vi "Autonomous Independent.vi"   [LabVIEW 2023]
doc: "This VI is called when autonomous begins, and will automatically be terminated when autonomous ends. You can carry out timed or sensor driven robot movement independently without needing to return to the caller."
uses:
  Swerve_Trajectory_Following/SWERVE_TRAJECTORY_GLOBALS.vi
  <vilib>/Rock Robotics/Network Tables/NT Read String.vi
  <vilib>/Rock Robotics/WPI/ThirdParty/JAS_Junk/TrajLib/Trajectory_Library.lvlib
  <vilib>/Rock Robotics/Network Tables/NT Write String.vi
  <vilib>/Rock Robotics/Network Tables/NT Read Number.vi
  <vilib>/Rock Robotics/Network Tables/NT Write Boolean.vi
  <vilib>/Rock Robotics/Network Tables/NT Read Boolean.vi
  <vilib>/Rock Robotics/Network Tables/NT Write Number.vi
  <vilib>/Rock Robotics/WPI/ThirdParty/JAS_Junk/TrajLib/TypeDef/TRANSLATION2D.ctl
  <vilib>/Rock Robotics/WPI/ThirdParty/JAS_Junk/TrajLib/TypeDef/ROTATION2D.ctl
  <vilib>/Rock Robotics/WPI/ThirdParty/JAS_Junk/TrajLib/TypeDef/POSE2D.ctl
  <vilib>/Rock Robotics/Network Tables/NT Read Numeric Array.vi
  <vilib>/Rock Robotics/Network Tables/NT Write Numeric Array.vi
  <vilib>/Rock Robotics/WPI/ThirdParty/MJansen/PathPlanner/ENum/PathPlanner_CommandUtilType_ENUM.ctl
  <vilib>/Rock Robotics/WPI/ThirdParty/MJansen/PathPlanner/PathPlanner24.lvlib
  <vilib>/Rock Robotics/WPI/ThirdParty/MJansen/PathPlanner/TypeDef/PathPlannerCommandUtil.ctl
  <vilib>/Rock Robotics/Network Tables/NT Write Integer.vi
  <vilib>/Rock Robotics/WPI/ThirdParty/Phoenix6/controls/DutyCycleOut SetControl.vi
  <vilib>/Rock Robotics/WPI/ThirdParty/Phoenix6/getters/GetPRO_PosAndVel_Velocity.vi
  <vilib>/Rock Robotics/WPI/ThirdParty/Phoenix6/getters/GetPRO_PosAndVel_Position.vi
panel:
  # "Be sure to right-click and choose Data Operations>>Make Current Value default if you want to save the array values with the VI"
types:
  T1 = typedef "WPI_JoystickDevRef.ctl" = cluster{"Device":T2}
  T2 = typedef "WPI_JoystickDeviceEnum.ctl" = enum16{"USB 0", "USB 1", "USB 2", "USB 3", "USB 4", "USB 5"}
  T3 = typedef "PathPlanner24.lvlib/PathPlannerCommandUtil.ctl" = cluster{"waitTime":dbl, "name":string, "pathName":string, "commands":cluster{"type":T4, "waitTime":dbl, "name":string, "pathName":string}[], "type":T4}
  T4 = typedef "PathPlanner24.lvlib/PathPlanner_CommandUtilType_ENUM.ctl" = enum16{"Unknown", "Wait", "Named", "Path", "Sequential", "Parallel", "Race", "Deadline"}
  T5 = cluster{"m_drive_volts":dbl, "m_log":u8[], "m_name":string}
  T6 = cluster{"MotorVoltage":dbl, "Position":dbl, "Velocity":dbl}
  T7 = typedef "Trajectory_Library.lvlib/POSE2D.ctl" = cluster{"TRANSLATION":T8, "ROTATION":T9}
  T8 = typedef "Trajectory_Library.lvlib/TRANSLATION2D.ctl" = cluster{"X":dbl, "Y":dbl}
  T9 = typedef "Trajectory_Library.lvlib/ROTATION2D.ctl" = cluster{"VALUE":dbl, "COS":dbl, "SIN":dbl}
  T10 = cluster{"type":T4, "waitTime":dbl, "name":string, "pathName":string}[]
  T11 = typedef "Trajectory_Library.lvlib/SWERVE_DRIVE_MODULE_POSITION.ctl" = cluster{"Distance":dbl, "Angle":T9, "P":bool}
  T12 = typedef "Trajectory_Library.lvlib/TRAJ_STATE.ctl" = cluster{"TimeSeconds":dbl, "Velocity":dbl, "Acceleration":dbl, "POSE":T7, "Curvature":dbl}
  T13 = cluster{"Error Pose":T7, "X Corr":dbl, "Y Corr":dbl}
  T14 = typedef "Trajectory_Library.lvlib/CHASSIS_SPEEDS.ctl" = cluster{"vX":dbl, "vY":dbl, "vOmega":dbl}
  T15 = typedef "Trajectory_Library.lvlib/TIMER.ctl" = cluster{"StartTime":dbl, "Accumulated TIme":dbl, "Running":bool, "semaphore":T16}
  T16 = typedef "Semaphore RefNum" = refnum<k1>
  T17 = cluster{"m_config":cluster{"m_timeout_Sec":dbl, "m_stepVoltage_Volt":dbl, "m_rampRate_V/S":dbl}, "m_mechanism":cluster{"m_drive_volts":dbl, "m_log":u8[], "m_name":string}, "m_outputVolts":dbl, "m_recordState":enum16{"kQuasistaticForward", "kQuasistaticReverse", "kDynamicForward", "kDynamicReverse", "kNone"}, "timer":T15}
  T18 = typedef "DeviceReference.ctl" = cluster{"CANbus Name":string, "Device Encoding":u32, "Device Name":string}
  T19 = cluster{"Value":dbl, "System Timestamp":dbl, "CANivore Timestamp":dbl, "ECU Timestamp":dbl}
  T20 = typedef "Trajectory_Library.lvlib/SWERVE_DRIVE_POSE_EST2.ctl" = cluster{"M_Vision_K":T21, "m_nominal_dT":dbl, "m_PrevTime_Sec":dbl, "Pose_Buffer":T22, "Swerve_Drive_Kinematics":T23, "Swerve_Drive_Odom":T25, "M_Q":T21, "NumModules":i32}
  T21 = typedef "NI_Matrix.lvlib/RealMatrix.ctl" = dbl[][]
  T22 = typedef "Trajectory_Library.lvlib/TIME_INTERPOLATABLE_VARIANT.ctl" = cluster{"TimeStamps":dbl[], "DataArray":variant[], "Min_TimeStamp":dbl, "Max_TimeStamp":dbl, "ItemCount":i32, "MaxBufferTime":dbl}
  T23 = typedef "Trajectory_Library.lvlib/SWERVE_DRIVE_KINEMATICS.ctl" = cluster{"NumModules":i32, "InverseKinematics":T21, "ForwardKinematics":T21, "Modules":T8[], "PrevCoR":T8, "SavedModuleStates":T24[]}
  T24 = typedef "Trajectory_Library.lvlib/SWERVE_DRIVE_MODULE_STATE.ctl" = cluster{"Speed":dbl, "Angle":T9}
  T25 = typedef "Trajectory_Library.lvlib/SWERVE_DRIVE_ODOMETRY.ctl" = cluster{"POSE":T7, "GyroOffset":T9, "PreviousAngle":T9, "PrevModulePositions":T11[], "NumModules":i32}
  T26 = typedef "Trajectory_Library.lvlib/PID_TUNING.ctl" = cluster{"Kp":dbl, "Ki":dbl, "Kd":dbl, "MaximumIntegral":dbl, "MinimumIntegral":dbl, "IntegralZone":dbl}
  T27 = typedef "Trajectory_Library.lvlib/PROFILED_PID_CONTROLLER.ctl" = cluster{"Controller":T28, "Goal":T29, "Setpoint":T29, "Constraint":T30}
  T28 = typedef "Trajectory_Library.lvlib/PID_CONTROLLER.ctl" = cluster{"Kp":dbl, "Ki":dbl, "Kd":dbl, "Period":dbl, "Max_Integral":dbl, "Min_Integral":dbl, "Max_Input":dbl, "Min_Input":dbl, "Continuous":bool, "PositionError":dbl, "VelocityError":dbl, "PrevError":dbl, "Total_Integral":dbl, "PositionTolerance":dbl, "VelocityTolerance":dbl, "SetPoint":dbl, "Kf":dbl, "Prev_Deriv":dbl, "Prev_Deriv 2":dbl, "DerivativeFilter":bool, "Min_Output":dbl, "Max_Output":dbl, "Prev_F_P":dbl, "Prev_F_P_2":dbl, "AntiWindupActive":bool, "Measurement":dbl, "IntegralZone":dbl}
  T29 = typedef "Trajectory_Library.lvlib/TRAPEZOID_PROFILE_STATE.ctl" = cluster{"Position":dbl, "Velocity":dbl}
  T30 = typedef "Trajectory_Library.lvlib/TRAPEZOID_PROFILE_CONSTRAINT.ctl" = cluster{"MaxVelocity":dbl, "MaxAcceleration":dbl}
  T31 = typedef "Trajectory_Library.lvlib/HOLONOMIC_PACK_TUNING.ctl" = cluster{"X PID Tuning":T26, "Y PID Tuning":T26, "thetaProfiledPID_CTRL":T27}
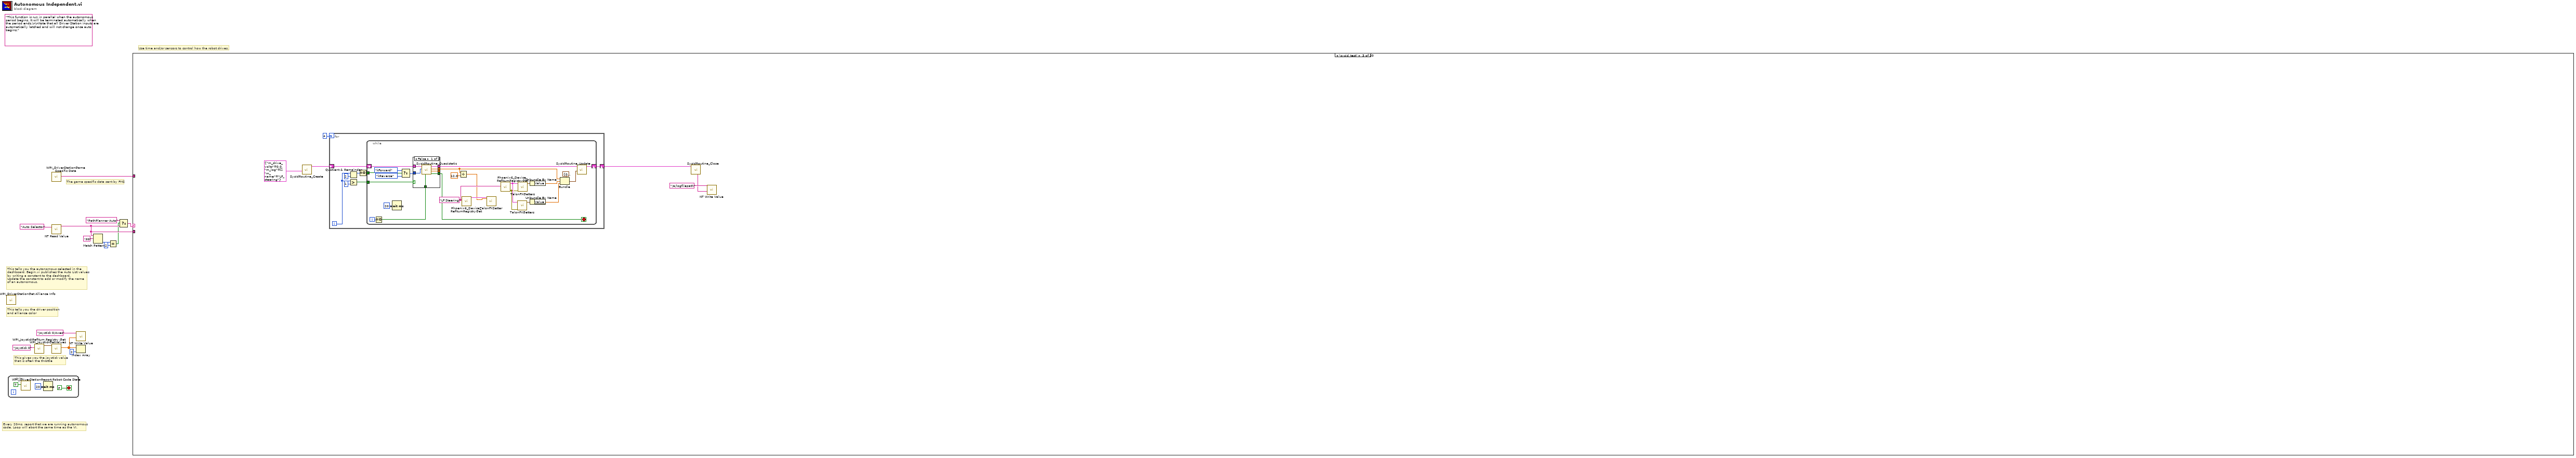
[diagram p0: block diagram]
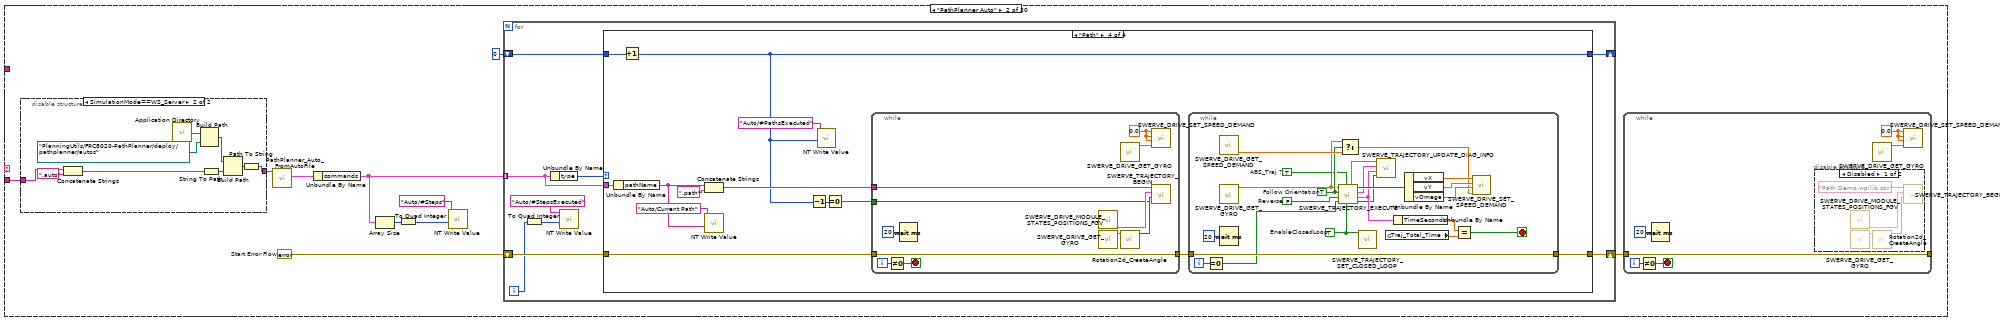
[diagram p3: hidden frame]
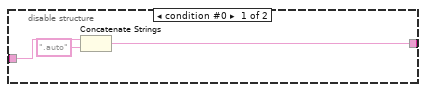
[diagram p4: hidden frame]
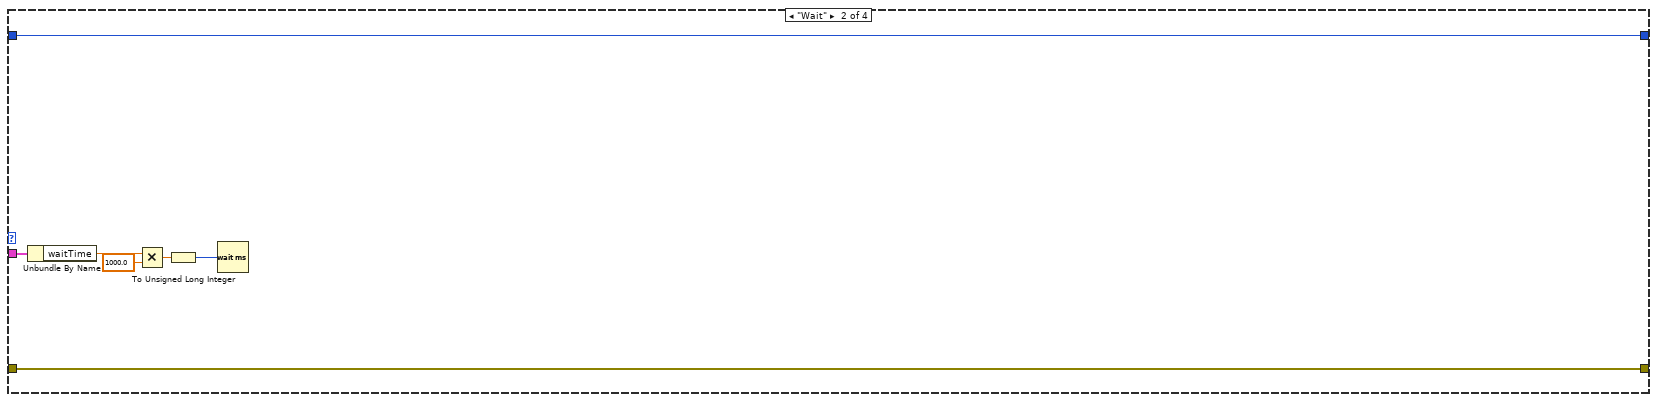
[diagram p7: hidden frame]
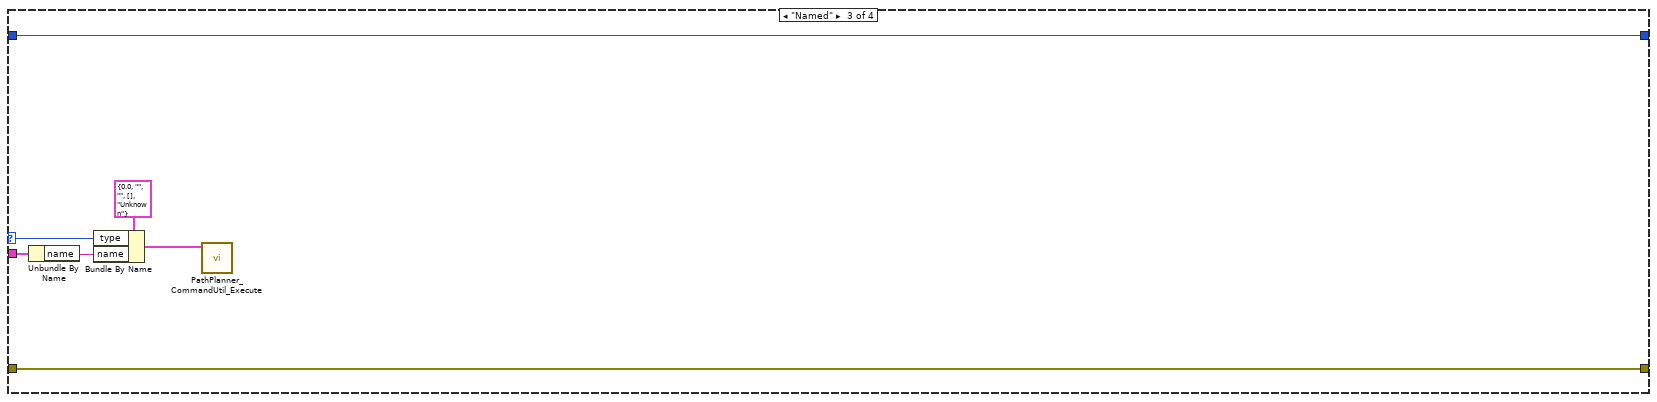
[diagram p8: hidden frame]
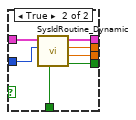
[diagram p9: hidden frame]
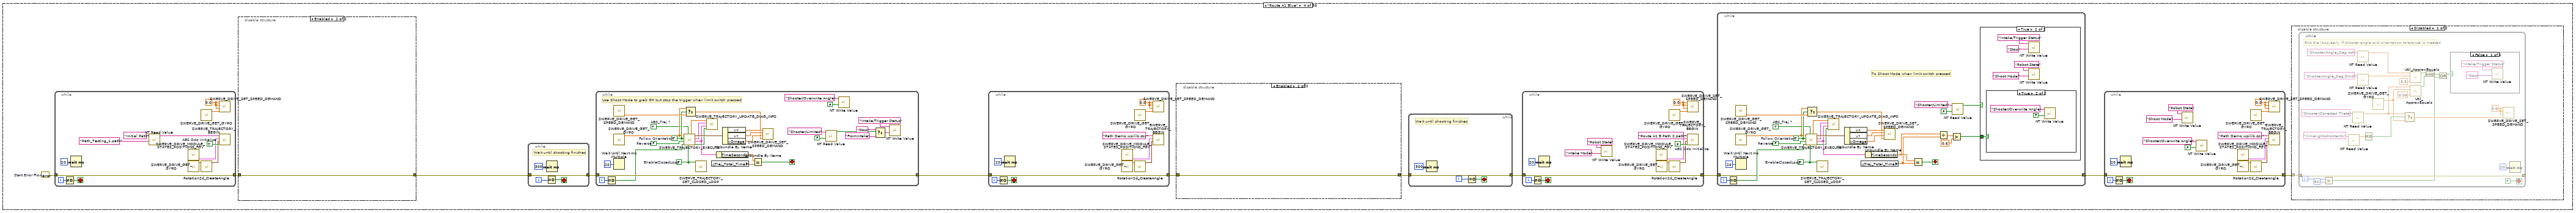
[diagram p10: hidden frame]
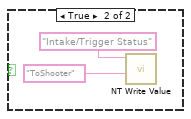
[diagram p11: hidden frame]
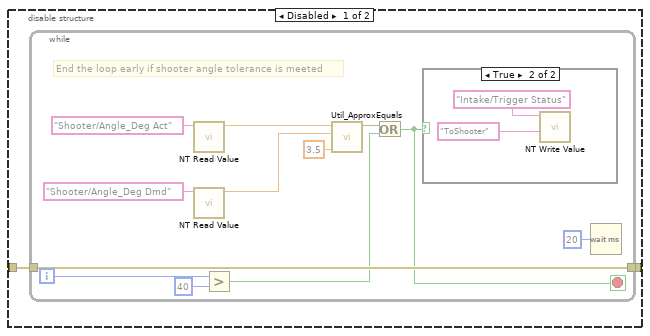
[diagram p13: hidden frame]
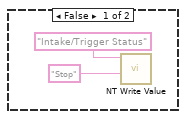
[diagram p14: hidden frame]
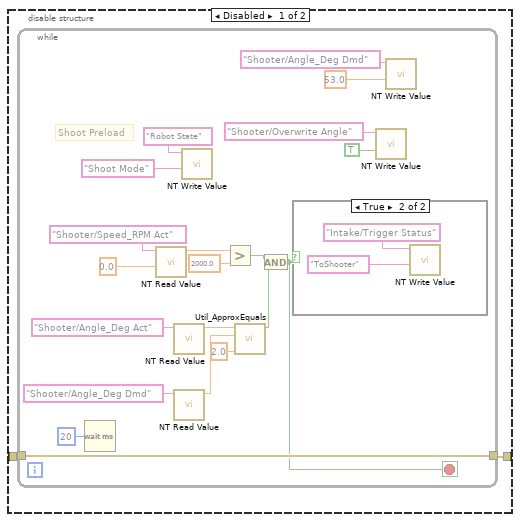
[diagram p15: hidden frame]
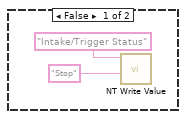
[diagram p16: hidden frame]
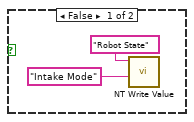
[diagram p17: hidden frame]
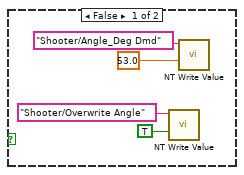
[diagram p18: hidden frame]
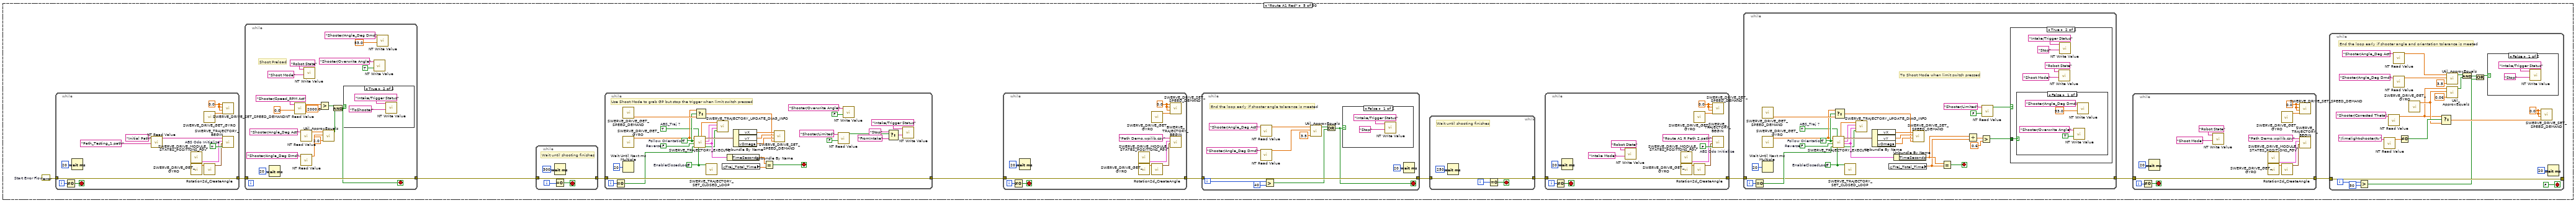
[diagram p19: hidden frame]
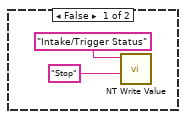
[diagram p20: hidden frame]
diagram:
  (unwired) "This function is run in parallel when the autonomous period begins. It will be terminated automatically when the period ends.\n\nNote that all Driver Station inputs are automatically latched and will not change once auto begins."
  # "The game specific data sent by FMS"
  # "This tells you the autonomous selected in the \ndashboard. Begin.vi publishes the Auto List values\nby writing a constant to the dashboard.\nUpdate the constant to add or modify the name\nof an autonomous."
  # "Every 20ms, report that we are running autonomous\ncode. Loop will abort the same time as the VI."
  # "This gives you the joystick value\nthat is often the throttle"
  # "Use time and/or sensors to control how the robot drives."
  # "This tells you the driver position\nand alliance color"
  n1 = call <vilib>:"WPI_DriverStationGet Alliance Info.vi"() -> ()  [unwired: 12 out]
  n2 = while {
    stop <- FALSE stop-if-true
    n3 = call <vilib>:"WPI_DriverStationReport Robot Code State.vi"("Autonomous"=TRUE) -> ()  [unwired: 10 in, 1 out]
    n4 = Wait (ms)(milliseconds to wait=u32 20) -> ()  [unwired: 1 out]
  }
  n5 = call <vilib>:"WPI_JoystickRefNum Registry Get.vi"("refnum name"="Joystick 0") -> ("JoystickDevRef"=w13:T1)  [unwired: 1 in, 9 out]
  n6 = call <vilib>:"WPI_JoystickGetValues.vi"("JoystickDevRef"=w13) -> ("Axes"=w10:dbl[])  [unwired: 6 in, 4 out]
  n7 = call <vilib>:"WPI_DriverStationGame Specific Data.vi"() -> ("Game Specific Data"=w8:string)  [unwired: 11 in]
  n8 = call-poly <vilib>:"NT Read Value.vi"("name"="Auto Selector" ("Name")) -> ("value"=w3:string)  [unwired: 8 in, 2 out]
  n9 = call-poly <vilib>:"NT Write Value.vi"("value"=w10, "name"="Joystick 0/Axes" ("Name")) -> ()  [unwired: 9 in, 1 out]
  n10 = Index Array(array=w10, index=2) -> ()  [unwired: 1 out]
  n11 = Match Pattern(string=w3, regular expression="PP") -> (offset past match=w6:i32)  [unwired: 1 in, 3 out]
  n12 = Equal?(x=w6, y=2) -> (x = y?=w1:bool)
  n13 = Select(t="PathPlanner Auto", s=w1, f=w3) -> (s? t:f=w4:string)
  n14 = case shown="\"sysid_test\"" w4 {
    tunnel: w8 -> [_ _ _ _ _ _ _ _ _ _ _ _ _ _ _ _ _ _ _ _ _ _ _ _ _ _ _ _ _ _]
    tunnel: w3 -> [_ w19 _ _ _ _ _ _ _ _ _ _ _ _ _ _ _ _ _ _ _ _ _ _ _ _ _ _ _ _]
    frame Default {
      # "You can put your main auto here, or you can right-click on the case and make any\nother frame be the default case."
      # "This is the frame that will execute if no selection is made, or if it is not recognized"
    }
    frame "PathPlanner Auto" {
      w21 = errorcluster {"status"=FALSE, "code"=0, "source"=""}  # Start Error Flow
      n15 = disable-structure shown="SimulationMode==WS_Server" {
        disable-tunnel: [w29 w31] -> w25
        disable-tunnel: w19 -> [w28 w38]
        frame condition #0 {
          n16 = Concatenate Strings(w28, ".auto" ("string")) -> (w29:string)
        }
        frame condition #1 (active) {
          n17 = Concatenate Strings(w38, ".auto" ("string")) -> (w35:string)
          n18 = call <vilib>:"Application Directory.vi"() -> ("Application Directory"=w37:path)
          n19 = Build Path(base path=w37, name or relative path=path "PlanningUtils/FRC8020-PathPlanner/deploy/pathplanner/autos") -> (appended path=w33:path)
          n20 = String To Path(string=w35) -> (path=w34:path)
          n21 = Build Path(base path=w33, name or relative path=w34) -> (appended path=w32:path)
          n22 = Path To String(path=w32) -> (string=w31:string)
        }
      }
      n23 = call "PathPlanner_Auto_FromAutoFile.vi"("FileName"=w25) -> ("Auto Command"=w27:T3)  [unwired: 8 in, 2 out]
      n24 = Unbundle By Name(w27) -> ("commands"=w26:T10)
      n25 = Array Size(array=w26) -> (size(s)=w23:i32)
      n26 = To Quad Integer(1:w23) -> (0:w22:i64)
      n27 = call-poly <vilib>:"NT Write Value.vi"("value"=w22, "name"="Auto/#Steps") -> ()  [unwired: 9 in, 1 out]
      n28 = for {
        tunnel: w26 -> [w57] mode=indexing
        shift-right: [w55] -> w20
        shift-left: w21 -> [w56]
        shift-right: [w50] -> _
        shift-left: 0 -> [w51]
        i -> [w53]
        n29 = To Quad Integer(1:w53) -> (0:w52:i64)
        n30 = Unbundle By Name(w57) -> ("type"=w58:T4)
        n31 = call-poly <vilib>:"NT Write Value.vi"("value"=w52, "name"="Auto/#StepsExecuted") -> ()  [unwired: 9 in, 1 out]
        n32 = case shown="\"Path\"" w58 {
          selector: w58 -> [_ _ w72 _]
          tunnel: w57 -> [_ w67 w74 w87]
          tunnel: w56 -> [w60 w62 w69 w82]
          tunnel: [w60 w62 w69 w81] -> w55
          tunnel: w51 -> [w59 w61 w68 w78]
          tunnel: [w59 w61 w68 w77] -> w50
          frame "Unknown", Default {
          }
          frame "Wait" {
            n33 = Unbundle By Name(w67) -> ("waitTime"=w66:dbl)
            n34 = Multiply(x=w66, y=1000.0) -> (x*y=w64:dbl)
            n35 = To Unsigned Long Integer(number=w64) -> (unsigned 32bit integer=w63:u32)
            n36 = Wait (ms)(milliseconds to wait=w63) -> ()  [unwired: 1 out]
          }
          frame "Named" {
            n37 = Unbundle By Name(w74) -> ("name"=w71:string)
            n38 = Bundle By Name(cluster=T3 {"waitTime"=0.0, "name"="", "pathName"="", "commands"=[], "type"=enum."Unknown"} ("CommandUtil"), "type"=w72, "name"=w71) -> (w70:T3)
            n39 = call <vilib>:"PathPlanner_CommandUtil_Execute.vi"("Command"=w70) -> ()  [unwired: 11 in]
          }
          frame "Path" {
            n40 = Unbundle By Name(w87) -> ("pathName"=w84:string)
            n41 = Increment(x=w78) -> (x+1=w77:i32)
            n42 = Concatenate Strings(w84, ".path" ("string")) -> (w80:string)
            n43 = call-poly <vilib>:"NT Write Value.vi"("value"=w84, "name"="Auto/Current Path") -> ()  [unwired: 9 in, 1 out]
            n44 = Decrement(x=w77) -> (x-1=w76:i32)
            n45 = call-poly <vilib>:"NT Write Value.vi"("value"=w77, "name"="Auto/#PathsExecuted") -> ()  [unwired: 9 in, 1 out]
            n46 = Equal To 0?(x=w76) -> (x = 0?=w75:bool)
            n47 = while {
              tunnel: w82 -> [w98]
              tunnel: [w98] -> w83
              tunnel: w80 -> [w89]
              tunnel: w75 -> [w88]
              i -> [w96]
              stop <- w95 stop-if-true
              w94 = 0.0 ("Drv X Vel Dmd")
              n48 = Not Equal To 0?(x=w96) -> (x != 0?=w95:bool)
              n49 = Wait (ms)(milliseconds to wait=u32 20) -> ()  [unwired: 1 out]
              n50 = call "SWERVE_DRIVE_MODULE_STATES_POSITIONS_FGV.vi"() -> ("out Current Module Positions"=w90:T11[])  [unwired: 10 in, 1 out]
              n51 = call "SWERVE_DRIVE_GET_GYRO.vi"() -> ("Gyro Heading Radians"=w92:dbl)  [unwired: 11 in]
              n52 = call "SWERVE_DRIVE_GET_GYRO.vi"() -> ("Gyro Heading Radians"=w93:dbl)  [unwired: 11 in]
              n53 = call <vilib>:"Rotation2d_CreateAngle.vi"("Angle"=w92) -> ("ROTATION"=w91:T9)  [unwired: 10 in]
              n54 = call "SWERVE_DRIVE_SET_SPEED_DEMAND.vi"("Drv Rotation Orentation Dmd"=w93, "Drv Angular Vel Dmd"=w94, "Drv Y Vel Dmd"=w94, "Drv X Vel Dmd"=w94) -> ()  [unwired: 8 in]
              n55 = call "SWERVE_TRAJECTORY_BEGIN.vi"("ABS Odo Initialize"=w88, "gyroAngle"=w91, "Module Positions"=w90, "Trajectory File Name"=w89) -> ()  [unwired: 8 in]
            }
            n56 = while {
              tunnel: w83 -> [w118]
              tunnel: [w118] -> w81
              i -> [w116]
              stop <- w115 stop-if-true
              w99 = TRUE  # ABS_Traj ?
              w107 = TRUE  # EnableClosedLoop
              w105 = FALSE  # Reverse
              w109 = TRUE  # Follow Orientation
              n57 = Equal To 0?(x=w116) -> (x = 0?=w106:bool)
              n58 = call "SWERVE_DRIVE_GET_SPEED_DEMAND.vi"() -> ("Drv Rotation Orentation Dmd"=w114:dbl)  [unwired: 8 in, 3 out]
              n59 = call "SWERVE_DRIVE_GET_GYRO.vi"() -> ("Gyro Heading Radians"=w104:dbl)  [unwired: 11 in]
              n60 = Wait (ms)(milliseconds to wait=u32 20) -> ()  [unwired: 1 out]
              n61 = call "SWERVE_TRAJECTORY_EXECUTE.vi"("EnableClosedLoop"=w107, "ABS_Traj ?"=w99, "Init"=w106, "Reverse"=w105, "Follow Orientation"=w109, "Gyro Heading\nRAD"=w104) -> ("AtReference"=w100:bool, "OutputTRAJ_STATE"=w101:T12, "Error and Corr"=w102:T13, "Chassis Velocity Target"=w108:T14, "Orientation Target"=w103:dbl)  [unwired: 1 in]
              n62 = Select(t=w104, s=w109, f=w114) -> (s? t:f=w110:dbl)
              n63 = call "SWERVE_TRAJECTORY_SET_CLOSED_LOOP.vi"("AUTO_CLOSED_LOOP"=w107) -> ()  [unwired: 11 in]
              n64 = call "SWERVE_TRAJECTORY_UPDATE_DIAG_INFO.vi"("AtReference"=w100, "OutputTRAJ_STATE"=w101, "Error and Corr"=w102, "Orientation Target"=w103) -> ()  [unwired: 8 in]
              n65 = global read "SWERVE_TRAJECTORY_GLOBALS.vi" "Traj_Total_Time"() -> (w119:dbl)
              n66 = Unbundle By Name(w101) -> ("TimeSeconds"=w117:dbl)
              n67 = Unbundle By Name(w108) -> ("vX"=w113:dbl, "vY"=w112:dbl, "vOmega"=w111:dbl)
              n68 = Equal?(x=w117, y=w119) -> (x = y?=w115:bool)
              n69 = call "SWERVE_DRIVE_SET_SPEED_DEMAND.vi"("Drv Rotation Orentation Dmd"=w110, "Drv Angular Vel Dmd"=w111, "Drv Y Vel Dmd"=w112, "Drv X Vel Dmd"=w113) -> ()  [unwired: 8 in]
            }
          }
        }
      }
      n70 = while {
        tunnel: w20 -> [w45]
        tunnel: [w45] -> _
        i -> [w43]
        stop <- w42 stop-if-true
        w41 = 0.0 ("Drv X Vel Dmd")
        n71 = Not Equal To 0?(x=w43) -> (x != 0?=w42:bool)
        n72 = Wait (ms)(milliseconds to wait=u32 20) -> ()  [unwired: 1 out]
        n73 = disable-structure shown="Disabled" {
          frame Disabled {
            n74 = call "SWERVE_DRIVE_MODULE_STATES_POSITIONS_FGV.vi"() -> ("out Current Module Positions"=w47:T11[])  [unwired: 10 in, 1 out]
            n75 = call "SWERVE_DRIVE_GET_GYRO.vi"() -> ("Gyro Heading Radians"=w49:dbl)  [unwired: 11 in]
            n76 = call <vilib>:"Rotation2d_CreateAngle.vi"("Angle"=w49) -> ("ROTATION"=w48:T9)  [unwired: 10 in]
            n77 = call "SWERVE_TRAJECTORY_BEGIN.vi"("gyroAngle"=w48, "Module Positions"=w47, "Trajectory File Name"="Path Demo.wpilib.csv") -> ()  [unwired: 9 in]
          }
          frame Enabled {
          }
        }
        n78 = call "SWERVE_DRIVE_GET_GYRO.vi"() -> ("Gyro Heading Radians"=w40:dbl)  [unwired: 11 in]
        n79 = call "SWERVE_DRIVE_SET_SPEED_DEMAND.vi"("Drv Rotation Orentation Dmd"=w40, "Drv Angular Vel Dmd"=w41, "Drv Y Vel Dmd"=w41, "Drv X Vel Dmd"=w41) -> ()  [unwired: 8 in]
      }
    }
    frame "sysid_test" {
      n80 = call "SysIdRoutine_Create.vi"("Mechanism"=T5 {"m_drive_volts"=0.0, "m_log"=[], "m_name"="LF_steering"}) -> ("SysIdRoutine"=w125:T17)  [unwired: 10 in]
      n81 = for {
        N: 4 -> [_]
        shift-right: [w133] -> w124
        shift-left: w125 -> [w134]
        i -> [w130]
        n82 = Greater?(x=w130, y=1) -> (0:w131:bool)
        n83 = Quotient & Remainder(x=w130, y=2) -> (x-y*floor(x/y)=w128:i32)  [unwired: 1 out]
        n84 = Equal To 0?(x=w128) -> (x = 0?=w127:bool)
        n85 = while {
          shift-right: [w157] -> w133
          shift-left: w134 -> [w159]
          tunnel: w131 -> [w150]
          tunnel: w127 -> [w148]
          i -> [w152]
          stop <- w149 stop-if-true
          w141 = "LF Steering" ("refnum name")
          n86 = Equal To 0?(x=w152) -> (x = 0?=w151:bool)
          n87 = Wait (ms)(milliseconds to wait=u32 20) -> ()  [unwired: 1 out]
          n88 = Select(t=enum16{"kForward", "kReverse"}."kForward" ("direction"), s=w148, f=enum16{"kForward", "kReverse"}."kReverse") -> (s? t:f=w154:enum16{"kForward", "kReverse"})
          n89 = case shown="False" w150 {
            tunnel: w159 -> [w166 w173]
            tunnel: [w165 w172] -> w158
            tunnel: w154 -> [w164 w170]
            tunnel: [w163 w169] -> w137
            tunnel: [w162 w168] -> _
            tunnel: [w161 w167] -> w149
            tunnel: w151 -> [w160 w171]
            frame False {
              n90 = call "SysIdRoutine_Quasistatic.vi"("reset?"=w160, "direction"=w164, "in SysIdRoutine"=w166) -> ("Expired"=w161:bool, "CurrentTimer"=w162:dbl, "outputVolts"=w163:dbl, "out SysIdRoutine"=w165:T17)  [unwired: 5 in]
            }
            frame True {
              n91 = call "SysIdRoutine_Dynamic.vi"("reset?"=w171, "direction"=w170, "in SysIdRoutine"=w173) -> ("Expired"=w167:bool, "CurrentTimer"=w168:dbl, "outputVolts"=w169:dbl, "out SysIdRoutine"=w172:T17)  [unwired: 5 in]
            }
          }
          n92 = Divide(x=w137, y=12.0) -> (x/y=w135:dbl)
          n93 = call <vilib>:"Phoenix6_Device_RefNumRegistryGet.vi"("refnum name"=w141) -> ("data"=w146:T18)  [unwired: 9 in, 1 out]
          n94 = call-poly <vilib>:"TalonFXSetter.vi"("DeviceReference"=w146, "Output"=w135) -> ()  [unwired: 24 in, 2 out]
          n95 = call <vilib>:"Phoenix6_Device_RefNumRegistryGet.vi"("refnum name"=w141) -> ("error out"=w144:errorcluster, "data"=w145:T18)  [unwired: 9 in]
          n96 = call-poly <vilib>:"TalonFXGetters.vi"("error in"=w144, "DeviceReference"=w145) -> ("Output"=w142:T19)  [unwired: 8 in, 1 out]
          n97 = call-poly <vilib>:"TalonFXGetters.vi"("error in"=w144, "DeviceReference"=w145) -> ("Output"=w143:T19)  [unwired: 8 in, 1 out]
          n98 = Unbundle By Name(w143) -> ("Value"=w139:dbl)
          n99 = Unbundle By Name(w142) -> ("Value"=w138:dbl)
          n100 = Bundle(cluster=T6 {"MotorVoltage"=0.0, "Position"=0.0, "Velocity"=0.0} ("MotorIO"), "MotorVoltage"=w137, "Position"=w139, "Velocity"=w138) -> (w136:T6)
          n101 = call "SysIdRoutine_Update.vi"("MotorIO"=w136, "in SysIdRoutine"=w158) -> ("out SysIdRoutine"=w157:T17)  [unwired: 9 in]
        }
      }
      n102 = call "SysIdRoutine_Close.vi"("in SysIdRoutine"=w124) -> ("Full Filename"=w121:string)  [unwired: 10 in]
      n103 = call-poly <vilib>:"NT Write Value.vi"("value"=w121, "name"="/a/logfilepath") -> ()  [unwired: 9 in, 1 out]
    }
    frame "Route A1 Blue" {
      w184 = errorcluster {"status"=FALSE, "code"=0, "source"=""}  # Start Error Flow
      n104 = while {
        tunnel: w184 -> [w358]
        tunnel: [w358] -> w176
        i -> [w356]
        stop <- w355 stop-if-true
        w352 = TRUE  # ABS Odo Initialize
        w354 = 0.0 ("Drv X Vel Dmd")
        n105 = Not Equal To 0?(x=w356) -> (x != 0?=w355:bool)
        n106 = Wait (ms)(milliseconds to wait=u32 20) -> ()  [unwired: 1 out]
        n107 = call-poly <vilib>:"NT Read Value.vi"("default value"="Path_Testing_1.path" ("Trajectory File Name"), "name"="Initial Path") -> ("value"=w349:string)  [unwired: 7 in, 2 out]
        n108 = call "SWERVE_DRIVE_MODULE_STATES_POSITIONS_FGV.vi"() -> ("out Current Module Positions"=w346:T11[])  [unwired: 10 in, 1 out]
        n109 = call "SWERVE_DRIVE_GET_GYRO.vi"() -> ("Gyro Heading Radians"=w348:dbl)  [unwired: 11 in]
        n110 = call "SWERVE_DRIVE_GET_GYRO.vi"() -> ("Gyro Heading Radians"=w353:dbl)  [unwired: 11 in]
        n111 = call <vilib>:"Rotation2d_CreateAngle.vi"("Angle"=w348) -> ("ROTATION"=w347:T9)  [unwired: 10 in]
        n112 = call "SWERVE_DRIVE_SET_SPEED_DEMAND.vi"("Drv Rotation Orentation Dmd"=w353, "Drv Angular Vel Dmd"=w354, "Drv Y Vel Dmd"=w354, "Drv X Vel Dmd"=w354) -> ()  [unwired: 8 in]
        n113 = call "SWERVE_TRAJECTORY_BEGIN.vi"("ABS Odo Initialize"=w352, "gyroAngle"=w347, "Module Positions"=w346, "Trajectory File Name"=w349) -> ()  [unwired: 8 in]
      }
      n114 = disable-structure shown="Enabled" {
        disable-tunnel: [w234 w259] -> w177
        disable-tunnel: w176 -> [w233 w259]
        frame Disabled {
          n115 = while {
            tunnel: w233 -> [w254]
            tunnel: [w254] -> w234
            stop <- w235 stop-if-true
            # "Shoot Preload"
            n116 = Wait (ms)(milliseconds to wait=u32 20) -> ()  [unwired: 1 out]
            n117 = call-poly <vilib>:"NT Read Value.vi"("default value"=0.0, "name"="Shooter/Speed_RPM Act") -> ("value"=w249:dbl)  [unwired: 7 in, 2 out]
            n118 = call-poly <vilib>:"NT Read Value.vi"("name"="Shooter/Angle_Deg Act") -> ("value"=w239:dbl)  [unwired: 8 in, 2 out]
            n119 = call-poly <vilib>:"NT Read Value.vi"("name"="Shooter/Angle_Deg Dmd") -> ("value"=w238:dbl)  [unwired: 8 in, 2 out]
            n120 = call-poly <vilib>:"NT Write Value.vi"("value"="Shoot Mode" ("default value"), "name"="Robot State") -> ()  [unwired: 9 in, 1 out]
            n121 = Greater?(x=w249, y=2000.0) -> (0:w237:bool)
            n122 = call <vilib>:"Util_ApproxEquals.vi"("Tolerance"=2.0, "Value 2"=w238, "Value 1"=w239) -> ("ApproxEquals"=w236:bool)  [unwired: 8 in]
            n123 = And(x=w237, y=w236) -> (x .and. y?=w235:bool)
            n124 = case shown="True" w235 {
              frame False {
                n125 = call-poly <vilib>:"NT Write Value.vi"("value"="Stop" ("default value"), "name"="Intake/Trigger Status") -> ()  [unwired: 9 in, 1 out]
              }
              frame True {
                n126 = call-poly <vilib>:"NT Write Value.vi"("value"="ToShooter" ("default value"), "name"="Intake/Trigger Status") -> ()  [unwired: 9 in, 1 out]
              }
            }
            n127 = call-poly <vilib>:"NT Write Value.vi"("value"=TRUE, "name"="Shooter/Overwrite Angle") -> ()  [unwired: 9 in, 1 out]
            n128 = call-poly <vilib>:"NT Write Value.vi"("value"=53.0, "name"="Shooter/Angle_Deg Dmd") -> ()  [unwired: 9 in, 1 out]
          }
        }
        frame Enabled {
        }
      }
      n129 = while {
        tunnel: w177 -> [w335]
        tunnel: [w335] -> w182
        i -> [w333]
        stop <- w332 stop-if-true
        # "Wait until shooting finishes"
        n130 = Wait (ms)(milliseconds to wait=u32 300) -> ()  [unwired: 1 out]
        n131 = Equal To 0?(x=w333) -> (x = 0?=w332:bool)
      }
      n132 = while {
        tunnel: w182 -> [w388]
        tunnel: [w388] -> w183
        i -> [w387]
        stop <- w370 stop-if-true
        w371 = TRUE  # ABS_Traj ?
        w379 = TRUE  # EnableClosedLoop
        w377 = FALSE  # Reverse
        w381 = TRUE  # Follow Orientation
        # "Use Shoot Mode to grab GP but stop the trigger when limit switch pressed"
        n133 = Equal To 0?(x=w387) -> (x = 0?=w378:bool)
        n134 = call "SWERVE_DRIVE_GET_SPEED_DEMAND.vi"() -> ("Drv Rotation Orentation Dmd"=w386:dbl)  [unwired: 8 in, 3 out]
        n135 = call "SWERVE_DRIVE_GET_GYRO.vi"() -> ("Gyro Heading Radians"=w376:dbl)  [unwired: 11 in]
        n136 = Wait Until Next ms Multiple(millisecond multiple=u32 20 ("milliseconds to wait")) -> ()  [unwired: 1 out]
        n137 = call "SWERVE_TRAJECTORY_EXECUTE.vi"("EnableClosedLoop"=w379, "ABS_Traj ?"=w371, "Init"=w378, "Reverse"=w377, "Follow Orientation"=w381, "Gyro Heading\nRAD"=w376) -> ("AtReference"=w372:bool, "OutputTRAJ_STATE"=w373:T12, "Error and Corr"=w374:T13, "Chassis Velocity Target"=w380:T14, "Orientation Target"=w375:dbl)  [unwired: 1 in]
        n138 = Select(t=w376, s=w381, f=w386) -> (s? t:f=w382:dbl)
        n139 = call "SWERVE_TRAJECTORY_SET_CLOSED_LOOP.vi"("AUTO_CLOSED_LOOP"=w379) -> ()  [unwired: 11 in]
        n140 = call "SWERVE_TRAJECTORY_UPDATE_DIAG_INFO.vi"("AtReference"=w372, "OutputTRAJ_STATE"=w373, "Error and Corr"=w374, "Orientation Target"=w375) -> ()  [unwired: 8 in]
        n141 = global read "SWERVE_TRAJECTORY_GLOBALS.vi" "Traj_Total_Time"() -> (w368:dbl)
        n142 = Unbundle By Name(w373) -> ("TimeSeconds"=w369:dbl)
        n143 = Unbundle By Name(w380) -> ("vX"=w385:dbl, "vY"=w384:dbl, "vOmega"=w383:dbl)
        n144 = Equal?(x=w369, y=w368) -> (x = y?=w370:bool)
        n145 = call "SWERVE_DRIVE_SET_SPEED_DEMAND.vi"("Drv Rotation Orentation Dmd"=w382, "Drv Angular Vel Dmd"=w383, "Drv Y Vel Dmd"=w384, "Drv X Vel Dmd"=w385) -> ()  [unwired: 8 in]
        n146 = call-poly <vilib>:"NT Read Value.vi"("default value"=FALSE ("value"), "name"="Shooter/Limited") -> ("value"=w365:bool)  [unwired: 7 in, 2 out]
        n147 = call-poly <vilib>:"NT Write Value.vi"("value"=FALSE, "name"="Shooter/Overwrite Angle") -> ()  [unwired: 9 in, 1 out]
        n148 = Select(t="Stop" ("default value"), s=w365, f="FromIntake") -> (s? t:f=w361:string)
        n149 = call-poly <vilib>:"NT Write Value.vi"("value"=w361, "name"="Intake/Trigger Status") -> ()  [unwired: 9 in, 1 out]
      }
      n150 = while {
        tunnel: w183 -> [w345]
        tunnel: [w345] -> w181
        i -> [w343]
        stop <- w342 stop-if-true
        w341 = 0.0 ("Drv X Vel Dmd")
        n151 = Not Equal To 0?(x=w343) -> (x != 0?=w342:bool)
        n152 = Wait (ms)(milliseconds to wait=u32 20) -> ()  [unwired: 1 out]
        n153 = call "SWERVE_DRIVE_MODULE_STATES_POSITIONS_FGV.vi"() -> ("out Current Module Positions"=w337:T11[])  [unwired: 10 in, 1 out]
        n154 = call "SWERVE_DRIVE_GET_GYRO.vi"() -> ("Gyro Heading Radians"=w339:dbl)  [unwired: 11 in]
        n155 = call "SWERVE_DRIVE_GET_GYRO.vi"() -> ("Gyro Heading Radians"=w340:dbl)  [unwired: 11 in]
        n156 = call <vilib>:"Rotation2d_CreateAngle.vi"("Angle"=w339) -> ("ROTATION"=w338:T9)  [unwired: 10 in]
        n157 = call "SWERVE_DRIVE_SET_SPEED_DEMAND.vi"("Drv Rotation Orentation Dmd"=w340, "Drv Angular Vel Dmd"=w341, "Drv Y Vel Dmd"=w341, "Drv X Vel Dmd"=w341) -> ()  [unwired: 8 in]
        n158 = call "SWERVE_TRAJECTORY_BEGIN.vi"("gyroAngle"=w338, "Module Positions"=w337, "Trajectory File Name"="Path Demo.wpilib.csv") -> ()  [unwired: 9 in]
      }
      n159 = disable-structure shown="Enabled" {
        disable-tunnel: w181 -> [w215 w232]
        disable-tunnel: [w214 w232] -> w179
        frame Disabled {
          n160 = while {
            tunnel: w215 -> [w227]
            tunnel: [w227] -> w214
            i -> [w219]
            stop <- w216 stop-if-true
            # "End the loop early if shooter angle tolerance is meeted"
            n161 = call-poly <vilib>:"NT Read Value.vi"("name"="Shooter/Angle_Deg Act") -> ("value"=w224:dbl)  [unwired: 8 in, 2 out]
            n162 = call-poly <vilib>:"NT Read Value.vi"("name"="Shooter/Angle_Deg Dmd") -> ("value"=w223:dbl)  [unwired: 8 in, 2 out]
            n163 = Greater?(x=w219, y=40) -> (0:w217:bool)
            n164 = call <vilib>:"Util_ApproxEquals.vi"("Tolerance"=3.5, "Value 2"=w223, "Value 1"=w224) -> ("ApproxEquals"=w220:bool)  [unwired: 8 in]
            n165 = Or(x=w220, y=w217) -> (x .or. y?=w216:bool)
            n166 = case shown="True" w216 {
              frame False {
                n167 = call-poly <vilib>:"NT Write Value.vi"("value"="Stop" ("default value"), "name"="Intake/Trigger Status") -> ()  [unwired: 9 in, 1 out]
              }
              frame True {
                n168 = call-poly <vilib>:"NT Write Value.vi"("value"="ToShooter" ("default value"), "name"="Intake/Trigger Status") -> ()  [unwired: 9 in, 1 out]
              }
            }
            n169 = Wait (ms)(milliseconds to wait=u32 20) -> ()  [unwired: 1 out]
          }
        }
        frame Enabled {
        }
      }
      n170 = while {
        tunnel: w179 -> [w304]
        tunnel: [w304] -> w178
        i -> [w302]
        stop <- w301 stop-if-true
        # "Wait until shooting finishes"
        n171 = Wait (ms)(milliseconds to wait=u32 300) -> ()  [unwired: 1 out]
        n172 = Equal To 0?(x=w302) -> (x = 0?=w301:bool)
      }
      n173 = while {
        tunnel: w178 -> [w331]
        tunnel: [w331] -> w174
        i -> [w329]
        stop <- w328 stop-if-true
        w325 = FALSE  # ABS Odo Initialize
        w327 = 0.0 ("Drv X Vel Dmd")
        n174 = Not Equal To 0?(x=w329) -> (x != 0?=w328:bool)
        n175 = Wait (ms)(milliseconds to wait=u32 20) -> ()  [unwired: 1 out]
        n176 = call-poly <vilib>:"NT Write Value.vi"("value"="Intake Mode" ("default value"), "name"="Robot State") -> ()  [unwired: 9 in, 1 out]
        n177 = call "SWERVE_DRIVE_MODULE_STATES_POSITIONS_FGV.vi"() -> ("out Current Module Positions"=w322:T11[])  [unwired: 10 in, 1 out]
        n178 = call "SWERVE_DRIVE_GET_GYRO.vi"() -> ("Gyro Heading Radians"=w324:dbl)  [unwired: 11 in]
        n179 = call "SWERVE_DRIVE_GET_GYRO.vi"() -> ("Gyro Heading Radians"=w326:dbl)  [unwired: 11 in]
        n180 = call <vilib>:"Rotation2d_CreateAngle.vi"("Angle"=w324) -> ("ROTATION"=w323:T9)  [unwired: 10 in]
        n181 = call "SWERVE_DRIVE_SET_SPEED_DEMAND.vi"("Drv Rotation Orentation Dmd"=w326, "Drv Angular Vel Dmd"=w327, "Drv Y Vel Dmd"=w327, "Drv X Vel Dmd"=w327) -> ()  [unwired: 8 in]
        n182 = call "SWERVE_TRAJECTORY_BEGIN.vi"("ABS Odo Initialize"=w325, "gyroAngle"=w323, "Module Positions"=w322, "Trajectory File Name"="Route A1 B Path 2.path") -> ()  [unwired: 8 in]
      }
      n183 = while {
        tunnel: w174 -> [w268]
        tunnel: [w268] -> w175
        i -> [w286]
        stop <- w269 stop-if-true
        w270 = TRUE  # ABS_Traj ?
        w278 = TRUE  # EnableClosedLoop
        w276 = FALSE  # Reverse
        w280 = TRUE  # Follow Orientation
        # "To Shoot Mode when limit switch pressed"
        n184 = Equal To 0?(x=w286) -> (x = 0?=w277:bool)
        n185 = call "SWERVE_DRIVE_GET_SPEED_DEMAND.vi"() -> ("Drv Rotation Orentation Dmd"=w285:dbl)  [unwired: 8 in, 3 out]
        n186 = call "SWERVE_DRIVE_GET_GYRO.vi"() -> ("Gyro Heading Radians"=w275:dbl)  [unwired: 11 in]
        n187 = Wait Until Next ms Multiple(millisecond multiple=u32 20 ("milliseconds to wait")) -> ()  [unwired: 1 out]
        n188 = call "SWERVE_TRAJECTORY_EXECUTE.vi"("EnableClosedLoop"=w278, "ABS_Traj ?"=w270, "Init"=w277, "Reverse"=w276, "Follow Orientation"=w280, "Gyro Heading\nRAD"=w275) -> ("AtReference"=w271:bool, "OutputTRAJ_STATE"=w272:T12, "Error and Corr"=w273:T13, "Chassis Velocity Target"=w279:T14, "Orientation Target"=w274:dbl)  [unwired: 1 in]
        n189 = Select(t=w275, s=w280, f=w285) -> (s? t:f=w281:dbl)
        n190 = call "SWERVE_TRAJECTORY_SET_CLOSED_LOOP.vi"("AUTO_CLOSED_LOOP"=w278) -> ()  [unwired: 11 in]
        n191 = call "SWERVE_TRAJECTORY_UPDATE_DIAG_INFO.vi"("AtReference"=w271, "OutputTRAJ_STATE"=w272, "Error and Corr"=w273, "Orientation Target"=w274) -> ()  [unwired: 8 in]
        n192 = Unbundle By Name(w279) -> ("vX"=w284:dbl, "vY"=w283:dbl, "vOmega"=w282:dbl)
        n193 = global read "SWERVE_TRAJECTORY_GLOBALS.vi" "Traj_Total_Time"() -> (w260:dbl)
        n194 = Unbundle By Name(w272) -> ("TimeSeconds"=w261:dbl)
        n195 = call "SWERVE_DRIVE_SET_SPEED_DEMAND.vi"("Drv Rotation Orentation Dmd"=w281, "Drv Angular Vel Dmd"=w282, "Drv Y Vel Dmd"=w283, "Drv X Vel Dmd"=w284) -> ()  [unwired: 8 in]
        n196 = Equal?(x=w261, y=w260) -> (x = y?=w269:bool)
        n197 = Divide(x=w261, y=w260) -> (x/y=w264:dbl)
        n198 = Greater?(x=w264, y=0.6) -> (0:w262:bool)
        n199 = call-poly <vilib>:"NT Read Value.vi"("default value"=FALSE ("value"), "name"="Shooter/Limited") -> ("value"=w266:bool)  [unwired: 7 in, 2 out]
        n200 = case shown="True" w266 {
          tunnel: w262 -> [_ w290]
          frame False {
            n201 = call-poly <vilib>:"NT Write Value.vi"("value"="Intake Mode" ("default value"), "name"="Robot State") -> ()  [unwired: 9 in, 1 out]
          }
          frame True {
            n202 = case shown="True" w290 {
              frame False {
                n203 = call-poly <vilib>:"NT Write Value.vi"("value"=TRUE, "name"="Shooter/Overwrite Angle") -> ()  [unwired: 9 in, 1 out]
                n204 = call-poly <vilib>:"NT Write Value.vi"("value"=53.0, "name"="Shooter/Angle_Deg Dmd") -> ()  [unwired: 9 in, 1 out]
              }
              frame True {
                n205 = call-poly <vilib>:"NT Write Value.vi"("value"=FALSE, "name"="Shooter/Overwrite Angle") -> ()  [unwired: 9 in, 1 out]
              }
            }
            n206 = call-poly <vilib>:"NT Write Value.vi"("value"="Shoot Mode" ("default value"), "name"="Robot State") -> ()  [unwired: 9 in, 1 out]
            n207 = call-poly <vilib>:"NT Write Value.vi"("value"="Stop" ("default value"), "name"="Intake/Trigger Status") -> ()  [unwired: 9 in, 1 out]
          }
        }
      }
      n208 = while {
        tunnel: w175 -> [w318]
        tunnel: [w318] -> w180
        i -> [w316]
        stop <- w315 stop-if-true
        w314 = 0.0 ("Drv X Vel Dmd")
        n209 = Not Equal To 0?(x=w316) -> (x != 0?=w315:bool)
        n210 = Wait (ms)(milliseconds to wait=u32 20) -> ()  [unwired: 1 out]
        n211 = call-poly <vilib>:"NT Write Value.vi"("value"="Shoot Mode" ("default value"), "name"="Robot State") -> ()  [unwired: 9 in, 1 out]
        n212 = call-poly <vilib>:"NT Write Value.vi"("value"=FALSE, "name"="Shooter/Overwrite Angle") -> ()  [unwired: 9 in, 1 out]
        n213 = call "SWERVE_DRIVE_MODULE_STATES_POSITIONS_FGV.vi"() -> ("out Current Module Positions"=w310:T11[])  [unwired: 10 in, 1 out]
        n214 = call "SWERVE_DRIVE_GET_GYRO.vi"() -> ("Gyro Heading Radians"=w312:dbl)  [unwired: 11 in]
        n215 = call "SWERVE_DRIVE_GET_GYRO.vi"() -> ("Gyro Heading Radians"=w313:dbl)  [unwired: 11 in]
        n216 = call <vilib>:"Rotation2d_CreateAngle.vi"("Angle"=w312) -> ("ROTATION"=w311:T9)  [unwired: 10 in]
        n217 = call "SWERVE_DRIVE_SET_SPEED_DEMAND.vi"("Drv Rotation Orentation Dmd"=w313, "Drv Angular Vel Dmd"=w314, "Drv Y Vel Dmd"=w314, "Drv X Vel Dmd"=w314) -> ()  [unwired: 8 in]
        n218 = call "SWERVE_TRAJECTORY_BEGIN.vi"("gyroAngle"=w311, "Module Positions"=w310, "Trajectory File Name"="Path Demo.wpilib.csv") -> ()  [unwired: 9 in]
      }
      n219 = disable-structure shown="Disabled" {
        disable-tunnel: w180 -> [w185 _]
        frame Disabled {
          n220 = while {
            tunnel: w185 -> [w209]
            tunnel: [w209] -> _
            i -> [w190]
            stop <- FALSE stop-if-true
            w197 = 0.0 ("Drv X Vel Dmd")
            # "End the loop early if shooter angle and orientation tolerance is meeted"
            n221 = Greater?(x=w190, y=50) -> (0:w186:bool)
            n222 = call-poly <vilib>:"NT Read Value.vi"("name"="/limelight-shooter/tv") -> ("value"=w200:dbl)  [unwired: 8 in, 2 out]
            n223 = call-poly <vilib>:"NT Read Value.vi"("name"="Shooter/Corrected Theta") -> ("value"=w194:dbl)  [unwired: 8 in, 2 out]
            n224 = call-poly <vilib>:"NT Read Value.vi"("name"="Shooter/Angle_Deg Act") -> ("value"=w206:dbl)  [unwired: 8 in, 2 out]
            n225 = call-poly <vilib>:"NT Read Value.vi"("name"="Shooter/Angle_Deg Dmd") -> ("value"=w205:dbl)  [unwired: 8 in, 2 out]
            n226 = Not Equal To 0?(x=w200) -> (x != 0?=w199:bool)
            n227 = call "SWERVE_DRIVE_GET_GYRO.vi"() -> ("Gyro Heading Radians"=w195:dbl)  [unwired: 11 in]
            n228 = Select(t=w194, s=w199, f=w195) -> (s? t:f=w198:dbl)
            n229 = call <vilib>:"Util_ApproxEquals.vi"("Tolerance"=3.5, "Value 2"=w205, "Value 1"=w206) -> ("ApproxEquals"=w196:bool)  [unwired: 8 in]
            n230 = call <vilib>:"Util_ApproxEquals.vi"("Tolerance"=0.06, "Value 2"=w195, "Value 1"=w194) -> ("ApproxEquals"=w192:bool)  [unwired: 8 in]
            n231 = And(x=w196, y=w192) -> (x .and. y?=w188:bool)
            n232 = Or(x=w188, y=w186) -> (x .or. y?=w187:bool)
            n233 = case shown="False" w187 {
              frame False {
                n234 = call-poly <vilib>:"NT Write Value.vi"("value"="Stop" ("default value"), "name"="Intake/Trigger Status") -> ()  [unwired: 9 in, 1 out]
              }
              frame True {
                n235 = call-poly <vilib>:"NT Write Value.vi"("value"="ToShooter" ("default value"), "name"="Intake/Trigger Status") -> ()  [unwired: 9 in, 1 out]
              }
            }
            n236 = call "SWERVE_DRIVE_SET_SPEED_DEMAND.vi"("Drv Rotation Orentation Dmd"=w198, "Drv Angular Vel Dmd"=w197, "Drv Y Vel Dmd"=w197, "Drv X Vel Dmd"=w197) -> ()  [unwired: 8 in]
            n237 = Wait (ms)(milliseconds to wait=u32 20) -> ()  [unwired: 1 out]
          }
        }
        frame Enabled {
        }
      }
    }
    frame "Route A1 Red" {
      w400 = errorcluster {"status"=FALSE, "code"=0, "source"=""}  # Start Error Flow
      n238 = while {
        tunnel: w400 -> [w565]
        tunnel: [w565] -> w391
        i -> [w563]
        stop <- w562 stop-if-true
        w559 = TRUE  # ABS Odo Initialize
        w561 = 0.0 ("Drv X Vel Dmd")
        n239 = Not Equal To 0?(x=w563) -> (x != 0?=w562:bool)
        n240 = Wait (ms)(milliseconds to wait=u32 20) -> ()  [unwired: 1 out]
        n241 = call-poly <vilib>:"NT Read Value.vi"("default value"="Path_Testing_1.path" ("Trajectory File Name"), "name"="Initial Path") -> ("value"=w556:string)  [unwired: 7 in, 2 out]
        n242 = call "SWERVE_DRIVE_MODULE_STATES_POSITIONS_FGV.vi"() -> ("out Current Module Positions"=w553:T11[])  [unwired: 10 in, 1 out]
        n243 = call "SWERVE_DRIVE_GET_GYRO.vi"() -> ("Gyro Heading Radians"=w555:dbl)  [unwired: 11 in]
        n244 = call "SWERVE_DRIVE_GET_GYRO.vi"() -> ("Gyro Heading Radians"=w560:dbl)  [unwired: 11 in]
        n245 = call <vilib>:"Rotation2d_CreateAngle.vi"("Angle"=w555) -> ("ROTATION"=w554:T9)  [unwired: 10 in]
        n246 = call "SWERVE_DRIVE_SET_SPEED_DEMAND.vi"("Drv Rotation Orentation Dmd"=w560, "Drv Angular Vel Dmd"=w561, "Drv Y Vel Dmd"=w561, "Drv X Vel Dmd"=w561) -> ()  [unwired: 8 in]
        n247 = call "SWERVE_TRAJECTORY_BEGIN.vi"("ABS Odo Initialize"=w559, "gyroAngle"=w554, "Module Positions"=w553, "Trajectory File Name"=w556) -> ()  [unwired: 8 in]
      }
      n248 = while {
        tunnel: w391 -> [w420]
        tunnel: [w420] -> w390
        stop <- w401 stop-if-true
        # "Shoot Preload"
        n249 = Wait (ms)(milliseconds to wait=u32 20) -> ()  [unwired: 1 out]
        n250 = call-poly <vilib>:"NT Read Value.vi"("default value"=0.0, "name"="Shooter/Speed_RPM Act") -> ("value"=w415:dbl)  [unwired: 7 in, 2 out]
        n251 = call-poly <vilib>:"NT Read Value.vi"("name"="Shooter/Angle_Deg Act") -> ("value"=w405:dbl)  [unwired: 8 in, 2 out]
        n252 = call-poly <vilib>:"NT Read Value.vi"("name"="Shooter/Angle_Deg Dmd") -> ("value"=w404:dbl)  [unwired: 8 in, 2 out]
        n253 = call-poly <vilib>:"NT Write Value.vi"("value"="Shoot Mode" ("default value"), "name"="Robot State") -> ()  [unwired: 9 in, 1 out]
        n254 = Greater?(x=w415, y=2000.0) -> (0:w403:bool)
        n255 = call <vilib>:"Util_ApproxEquals.vi"("Tolerance"=2.0, "Value 2"=w404, "Value 1"=w405) -> ("ApproxEquals"=w402:bool)  [unwired: 8 in]
        n256 = And(x=w403, y=w402) -> (x .and. y?=w401:bool)
        n257 = case shown="True" w401 {
          frame False {
            n258 = call-poly <vilib>:"NT Write Value.vi"("value"="Stop" ("default value"), "name"="Intake/Trigger Status") -> ()  [unwired: 9 in, 1 out]
          }
          frame True {
            n259 = call-poly <vilib>:"NT Write Value.vi"("value"="ToShooter" ("default value"), "name"="Intake/Trigger Status") -> ()  [unwired: 9 in, 1 out]
          }
        }
        n260 = call-poly <vilib>:"NT Write Value.vi"("value"=TRUE, "name"="Shooter/Overwrite Angle") -> ()  [unwired: 9 in, 1 out]
        n261 = call-poly <vilib>:"NT Write Value.vi"("value"=53.0, "name"="Shooter/Angle_Deg Dmd") -> ()  [unwired: 9 in, 1 out]
      }
      n262 = while {
        tunnel: w390 -> [w542]
        tunnel: [w542] -> w397
        i -> [w540]
        stop <- w539 stop-if-true
        # "Wait until shooting finishes"
        n263 = Wait (ms)(milliseconds to wait=u32 300) -> ()  [unwired: 1 out]
        n264 = Equal To 0?(x=w540) -> (x = 0?=w539:bool)
      }
      n265 = while {
        tunnel: w397 -> [w595]
        tunnel: [w595] -> w399
        i -> [w594]
        stop <- w577 stop-if-true
        w578 = TRUE  # ABS_Traj ?
        w586 = TRUE  # EnableClosedLoop
        w584 = FALSE  # Reverse
        w588 = TRUE  # Follow Orientation
        # "Use Shoot Mode to grab GP but stop the trigger when limit switch pressed"
        n266 = Equal To 0?(x=w594) -> (x = 0?=w585:bool)
        n267 = call "SWERVE_DRIVE_GET_SPEED_DEMAND.vi"() -> ("Drv Rotation Orentation Dmd"=w593:dbl)  [unwired: 8 in, 3 out]
        n268 = call "SWERVE_DRIVE_GET_GYRO.vi"() -> ("Gyro Heading Radians"=w583:dbl)  [unwired: 11 in]
        n269 = Wait Until Next ms Multiple(millisecond multiple=u32 20 ("milliseconds to wait")) -> ()  [unwired: 1 out]
        n270 = call "SWERVE_TRAJECTORY_EXECUTE.vi"("EnableClosedLoop"=w586, "ABS_Traj ?"=w578, "Init"=w585, "Reverse"=w584, "Follow Orientation"=w588, "Gyro Heading\nRAD"=w583) -> ("AtReference"=w579:bool, "OutputTRAJ_STATE"=w580:T12, "Error and Corr"=w581:T13, "Chassis Velocity Target"=w587:T14, "Orientation Target"=w582:dbl)  [unwired: 1 in]
        n271 = Select(t=w583, s=w588, f=w593) -> (s? t:f=w589:dbl)
        n272 = call "SWERVE_TRAJECTORY_SET_CLOSED_LOOP.vi"("AUTO_CLOSED_LOOP"=w586) -> ()  [unwired: 11 in]
        n273 = call "SWERVE_TRAJECTORY_UPDATE_DIAG_INFO.vi"("AtReference"=w579, "OutputTRAJ_STATE"=w580, "Error and Corr"=w581, "Orientation Target"=w582) -> ()  [unwired: 8 in]
        n274 = global read "SWERVE_TRAJECTORY_GLOBALS.vi" "Traj_Total_Time"() -> (w575:dbl)
        n275 = Unbundle By Name(w580) -> ("TimeSeconds"=w576:dbl)
        n276 = Unbundle By Name(w587) -> ("vX"=w592:dbl, "vY"=w591:dbl, "vOmega"=w590:dbl)
        n277 = Equal?(x=w576, y=w575) -> (x = y?=w577:bool)
        n278 = call "SWERVE_DRIVE_SET_SPEED_DEMAND.vi"("Drv Rotation Orentation Dmd"=w589, "Drv Angular Vel Dmd"=w590, "Drv Y Vel Dmd"=w591, "Drv X Vel Dmd"=w592) -> ()  [unwired: 8 in]
        n279 = call-poly <vilib>:"NT Read Value.vi"("default value"=FALSE ("value"), "name"="Shooter/Limited") -> ("value"=w572:bool)  [unwired: 7 in, 2 out]
        n280 = call-poly <vilib>:"NT Write Value.vi"("value"=FALSE, "name"="Shooter/Overwrite Angle") -> ()  [unwired: 9 in, 1 out]
        n281 = Select(t="Stop" ("default value"), s=w572, f="FromIntake") -> (s? t:f=w568:string)
        n282 = call-poly <vilib>:"NT Write Value.vi"("value"=w568, "name"="Intake/Trigger Status") -> ()  [unwired: 9 in, 1 out]
      }
      n283 = while {
        tunnel: w399 -> [w552]
        tunnel: [w552] -> w396
        i -> [w550]
        stop <- w549 stop-if-true
        w548 = 0.0 ("Drv X Vel Dmd")
        n284 = Not Equal To 0?(x=w550) -> (x != 0?=w549:bool)
        n285 = Wait (ms)(milliseconds to wait=u32 20) -> ()  [unwired: 1 out]
        n286 = call "SWERVE_DRIVE_MODULE_STATES_POSITIONS_FGV.vi"() -> ("out Current Module Positions"=w544:T11[])  [unwired: 10 in, 1 out]
        n287 = call "SWERVE_DRIVE_GET_GYRO.vi"() -> ("Gyro Heading Radians"=w546:dbl)  [unwired: 11 in]
        n288 = call "SWERVE_DRIVE_GET_GYRO.vi"() -> ("Gyro Heading Radians"=w547:dbl)  [unwired: 11 in]
        n289 = call <vilib>:"Rotation2d_CreateAngle.vi"("Angle"=w546) -> ("ROTATION"=w545:T9)  [unwired: 10 in]
        n290 = call "SWERVE_DRIVE_SET_SPEED_DEMAND.vi"("Drv Rotation Orentation Dmd"=w547, "Drv Angular Vel Dmd"=w548, "Drv Y Vel Dmd"=w548, "Drv X Vel Dmd"=w548) -> ()  [unwired: 8 in]
        n291 = call "SWERVE_TRAJECTORY_BEGIN.vi"("gyroAngle"=w545, "Module Positions"=w544, "Trajectory File Name"="Path Demo.wpilib.csv") -> ()  [unwired: 9 in]
      }
      n292 = while {
        tunnel: w396 -> [w509]
        tunnel: [w509] -> w393
        i -> [w501]
        stop <- w498 stop-if-true
        # "End the loop early if shooter angle tolerance is meeted"
        n293 = call-poly <vilib>:"NT Read Value.vi"("name"="Shooter/Angle_Deg Act") -> ("value"=w506:dbl)  [unwired: 8 in, 2 out]
        n294 = call-poly <vilib>:"NT Read Value.vi"("name"="Shooter/Angle_Deg Dmd") -> ("value"=w505:dbl)  [unwired: 8 in, 2 out]
        n295 = Greater?(x=w501, y=40) -> (0:w499:bool)
        n296 = call <vilib>:"Util_ApproxEquals.vi"("Tolerance"=3.5, "Value 2"=w505, "Value 1"=w506) -> ("ApproxEquals"=w502:bool)  [unwired: 8 in]
        n297 = Or(x=w502, y=w499) -> (x .or. y?=w498:bool)
        n298 = case shown="False" w498 {
          frame False {
            n299 = call-poly <vilib>:"NT Write Value.vi"("value"="Stop" ("default value"), "name"="Intake/Trigger Status") -> ()  [unwired: 9 in, 1 out]
          }
          frame True {
            n300 = call-poly <vilib>:"NT Write Value.vi"("value"="ToShooter" ("default value"), "name"="Intake/Trigger Status") -> ()  [unwired: 9 in, 1 out]
          }
        }
        n301 = Wait (ms)(milliseconds to wait=u32 20) -> ()  [unwired: 1 out]
      }
      n302 = while {
        tunnel: w393 -> [w428]
        tunnel: [w428] -> w392
        i -> [w426]
        stop <- w425 stop-if-true
        # "Wait until shooting finishes"
        n303 = Wait (ms)(milliseconds to wait=u32 250) -> ()  [unwired: 1 out]
        n304 = Equal To 0?(x=w426) -> (x = 0?=w425:bool)
      }
      n305 = while {
        tunnel: w392 -> [w538]
        tunnel: [w538] -> w398
        i -> [w536]
        stop <- w535 stop-if-true
        w532 = FALSE  # ABS Odo Initialize
        w534 = 0.0 ("Drv X Vel Dmd")
        n306 = Not Equal To 0?(x=w536) -> (x != 0?=w535:bool)
        n307 = Wait (ms)(milliseconds to wait=u32 20) -> ()  [unwired: 1 out]
        n308 = call-poly <vilib>:"NT Write Value.vi"("value"="Intake Mode" ("default value"), "name"="Robot State") -> ()  [unwired: 9 in, 1 out]
        n309 = call "SWERVE_DRIVE_MODULE_STATES_POSITIONS_FGV.vi"() -> ("out Current Module Positions"=w529:T11[])  [unwired: 10 in, 1 out]
        n310 = call "SWERVE_DRIVE_GET_GYRO.vi"() -> ("Gyro Heading Radians"=w531:dbl)  [unwired: 11 in]
        n311 = call "SWERVE_DRIVE_GET_GYRO.vi"() -> ("Gyro Heading Radians"=w533:dbl)  [unwired: 11 in]
        n312 = call <vilib>:"Rotation2d_CreateAngle.vi"("Angle"=w531) -> ("ROTATION"=w530:T9)  [unwired: 10 in]
        n313 = call "SWERVE_DRIVE_SET_SPEED_DEMAND.vi"("Drv Rotation Orentation Dmd"=w533, "Drv Angular Vel Dmd"=w534, "Drv Y Vel Dmd"=w534, "Drv X Vel Dmd"=w534) -> ()  [unwired: 8 in]
        n314 = call "SWERVE_TRAJECTORY_BEGIN.vi"("ABS Odo Initialize"=w532, "gyroAngle"=w530, "Module Positions"=w529, "Trajectory File Name"="Route A1 R Path 2.path") -> ()  [unwired: 8 in]
      }
      n315 = while {
        tunnel: w398 -> [w465]
        tunnel: [w465] -> w395
        i -> [w483]
        stop <- w466 stop-if-true
        w467 = TRUE  # ABS_Traj ?
        w475 = TRUE  # EnableClosedLoop
        w473 = FALSE  # Reverse
        w477 = TRUE  # Follow Orientation
        # "To Shoot Mode when limit switch pressed"
        n316 = Equal To 0?(x=w483) -> (x = 0?=w474:bool)
        n317 = call "SWERVE_DRIVE_GET_SPEED_DEMAND.vi"() -> ("Drv Rotation Orentation Dmd"=w482:dbl)  [unwired: 8 in, 3 out]
        n318 = call "SWERVE_DRIVE_GET_GYRO.vi"() -> ("Gyro Heading Radians"=w472:dbl)  [unwired: 11 in]
        n319 = Wait Until Next ms Multiple(millisecond multiple=u32 20 ("milliseconds to wait")) -> ()  [unwired: 1 out]
        n320 = call "SWERVE_TRAJECTORY_EXECUTE.vi"("EnableClosedLoop"=w475, "ABS_Traj ?"=w467, "Init"=w474, "Reverse"=w473, "Follow Orientation"=w477, "Gyro Heading\nRAD"=w472) -> ("AtReference"=w468:bool, "OutputTRAJ_STATE"=w469:T12, "Error and Corr"=w470:T13, "Chassis Velocity Target"=w476:T14, "Orientation Target"=w471:dbl)  [unwired: 1 in]
        n321 = Select(t=w472, s=w477, f=w482) -> (s? t:f=w478:dbl)
        n322 = call "SWERVE_TRAJECTORY_SET_CLOSED_LOOP.vi"("AUTO_CLOSED_LOOP"=w475) -> ()  [unwired: 11 in]
        n323 = call "SWERVE_TRAJECTORY_UPDATE_DIAG_INFO.vi"("AtReference"=w468, "OutputTRAJ_STATE"=w469, "Error and Corr"=w470, "Orientation Target"=w471) -> ()  [unwired: 8 in]
        n324 = Unbundle By Name(w476) -> ("vX"=w481:dbl, "vY"=w480:dbl, "vOmega"=w479:dbl)
        n325 = global read "SWERVE_TRAJECTORY_GLOBALS.vi" "Traj_Total_Time"() -> (w457:dbl)
        n326 = Unbundle By Name(w469) -> ("TimeSeconds"=w458:dbl)
        n327 = call "SWERVE_DRIVE_SET_SPEED_DEMAND.vi"("Drv Rotation Orentation Dmd"=w478, "Drv Angular Vel Dmd"=w479, "Drv Y Vel Dmd"=w480, "Drv X Vel Dmd"=w481) -> ()  [unwired: 8 in]
        n328 = Equal?(x=w458, y=w457) -> (x = y?=w466:bool)
        n329 = Divide(x=w458, y=w457) -> (x/y=w461:dbl)
        n330 = Greater?(x=w461, y=0.6) -> (0:w459:bool)
        n331 = call-poly <vilib>:"NT Read Value.vi"("default value"=FALSE ("value"), "name"="Shooter/Limited") -> ("value"=w463:bool)  [unwired: 7 in, 2 out]
        n332 = case shown="True" w463 {
          tunnel: w459 -> [_ w487]
          frame False {
            n333 = call-poly <vilib>:"NT Write Value.vi"("value"="Intake Mode" ("default value"), "name"="Robot State") -> ()  [unwired: 9 in, 1 out]
          }
          frame True {
            n334 = case shown="False" w487 {
              frame False {
                n335 = call-poly <vilib>:"NT Write Value.vi"("value"=TRUE, "name"="Shooter/Overwrite Angle") -> ()  [unwired: 9 in, 1 out]
                n336 = call-poly <vilib>:"NT Write Value.vi"("value"=53.0, "name"="Shooter/Angle_Deg Dmd") -> ()  [unwired: 9 in, 1 out]
              }
              frame True {
                n337 = call-poly <vilib>:"NT Write Value.vi"("value"=FALSE, "name"="Shooter/Overwrite Angle") -> ()  [unwired: 9 in, 1 out]
              }
            }
            n338 = call-poly <vilib>:"NT Write Value.vi"("value"="Shoot Mode" ("default value"), "name"="Robot State") -> ()  [unwired: 9 in, 1 out]
            n339 = call-poly <vilib>:"NT Write Value.vi"("value"="Stop" ("default value"), "name"="Intake/Trigger Status") -> ()  [unwired: 9 in, 1 out]
          }
        }
      }
      n340 = while {
        tunnel: w395 -> [w525]
        tunnel: [w525] -> w394
        i -> [w523]
        stop <- w522 stop-if-true
        w521 = 0.0 ("Drv X Vel Dmd")
        n341 = Not Equal To 0?(x=w523) -> (x != 0?=w522:bool)
        n342 = Wait (ms)(milliseconds to wait=u32 20) -> ()  [unwired: 1 out]
        n343 = call-poly <vilib>:"NT Write Value.vi"("value"="Shoot Mode" ("default value"), "name"="Robot State") -> ()  [unwired: 9 in, 1 out]
        n344 = call "SWERVE_DRIVE_MODULE_STATES_POSITIONS_FGV.vi"() -> ("out Current Module Positions"=w517:T11[])  [unwired: 10 in, 1 out]
        n345 = call "SWERVE_DRIVE_GET_GYRO.vi"() -> ("Gyro Heading Radians"=w519:dbl)  [unwired: 11 in]
        n346 = call "SWERVE_DRIVE_GET_GYRO.vi"() -> ("Gyro Heading Radians"=w520:dbl)  [unwired: 11 in]
        n347 = call <vilib>:"Rotation2d_CreateAngle.vi"("Angle"=w519) -> ("ROTATION"=w518:T9)  [unwired: 10 in]
        n348 = call "SWERVE_DRIVE_SET_SPEED_DEMAND.vi"("Drv Rotation Orentation Dmd"=w520, "Drv Angular Vel Dmd"=w521, "Drv Y Vel Dmd"=w521, "Drv X Vel Dmd"=w521) -> ()  [unwired: 8 in]
        n349 = call "SWERVE_TRAJECTORY_BEGIN.vi"("gyroAngle"=w518, "Module Positions"=w517, "Trajectory File Name"="Path Demo.wpilib.csv") -> ()  [unwired: 9 in]
      }
      n350 = while {
        tunnel: w394 -> [w452]
        tunnel: [w452] -> _
        i -> [w433]
        stop <- FALSE stop-if-true
        w440 = 0.0 ("Drv X Vel Dmd")
        # "End the loop early if shooter angle and orientation tolerance is meeted"
        n351 = Greater?(x=w433, y=50) -> (0:w429:bool)
        n352 = call-poly <vilib>:"NT Read Value.vi"("name"="/limelight-shooter/tv") -> ("value"=w443:dbl)  [unwired: 8 in, 2 out]
        n353 = call-poly <vilib>:"NT Read Value.vi"("name"="Shooter/Corrected Theta") -> ("value"=w437:dbl)  [unwired: 8 in, 2 out]
        n354 = call-poly <vilib>:"NT Read Value.vi"("name"="Shooter/Angle_Deg Act") -> ("value"=w449:dbl)  [unwired: 8 in, 2 out]
        n355 = call-poly <vilib>:"NT Read Value.vi"("name"="Shooter/Angle_Deg Dmd") -> ("value"=w448:dbl)  [unwired: 8 in, 2 out]
        n356 = Not Equal To 0?(x=w443) -> (x != 0?=w442:bool)
        n357 = call "SWERVE_DRIVE_GET_GYRO.vi"() -> ("Gyro Heading Radians"=w438:dbl)  [unwired: 11 in]
        n358 = Select(t=w437, s=w442, f=w438) -> (s? t:f=w441:dbl)
        n359 = call <vilib>:"Util_ApproxEquals.vi"("Tolerance"=3.5, "Value 2"=w448, "Value 1"=w449) -> ("ApproxEquals"=w439:bool)  [unwired: 8 in]
        n360 = call <vilib>:"Util_ApproxEquals.vi"("Tolerance"=0.06, "Value 2"=w438, "Value 1"=w437) -> ("ApproxEquals"=w435:bool)  [unwired: 8 in]
        n361 = And(x=w439, y=w435) -> (x .and. y?=w431:bool)
        n362 = Or(x=w431, y=w429) -> (x .or. y?=w430:bool)
        n363 = case shown="False" w430 {
          frame False {
            n364 = call-poly <vilib>:"NT Write Value.vi"("value"="Stop" ("default value"), "name"="Intake/Trigger Status") -> ()  [unwired: 9 in, 1 out]
          }
          frame True {
            n365 = call-poly <vilib>:"NT Write Value.vi"("value"="ToShooter" ("default value"), "name"="Intake/Trigger Status") -> ()  [unwired: 9 in, 1 out]
          }
        }
        n366 = call "SWERVE_DRIVE_SET_SPEED_DEMAND.vi"("Drv Rotation Orentation Dmd"=w441, "Drv Angular Vel Dmd"=w440, "Drv Y Vel Dmd"=w440, "Drv X Vel Dmd"=w440) -> ()  [unwired: 8 in]
        n367 = Wait (ms)(milliseconds to wait=u32 20) -> ()  [unwired: 1 out]
      }
    }
    frame "Preload A Blue" {
      w598 = errorcluster {"status"=FALSE, "code"=0, "source"=""}  # Start Error Flow
      n368 = while {
        tunnel: w598 -> [w637]
        tunnel: [w637] -> w597
        i -> [w635]
        stop <- w634 stop-if-true
        w631 = TRUE  # ABS Odo Initialize
        w633 = 0.0 ("Drv X Vel Dmd")
        n369 = Not Equal To 0?(x=w635) -> (x != 0?=w634:bool)
        n370 = Wait (ms)(milliseconds to wait=u32 20) -> ()  [unwired: 1 out]
        n371 = call-poly <vilib>:"NT Read Value.vi"("default value"="Path_Testing_1.path" ("Trajectory File Name"), "name"="Initial Path") -> ("value"=w628:string)  [unwired: 7 in, 2 out]
        n372 = call "SWERVE_DRIVE_MODULE_STATES_POSITIONS_FGV.vi"() -> ("out Current Module Positions"=w625:T11[])  [unwired: 10 in, 1 out]
        n373 = call "SWERVE_DRIVE_GET_GYRO.vi"() -> ("Gyro Heading Radians"=w627:dbl)  [unwired: 11 in]
        n374 = call "SWERVE_DRIVE_GET_GYRO.vi"() -> ("Gyro Heading Radians"=w632:dbl)  [unwired: 11 in]
        n375 = call <vilib>:"Rotation2d_CreateAngle.vi"("Angle"=w627) -> ("ROTATION"=w626:T9)  [unwired: 10 in]
        n376 = call "SWERVE_DRIVE_SET_SPEED_DEMAND.vi"("Drv Rotation Orentation Dmd"=w632, "Drv Angular Vel Dmd"=w633, "Drv Y Vel Dmd"=w633, "Drv X Vel Dmd"=w633) -> ()  [unwired: 8 in]
        n377 = call "SWERVE_TRAJECTORY_BEGIN.vi"("ABS Odo Initialize"=w631, "gyroAngle"=w626, "Module Positions"=w625, "Trajectory File Name"=w628) -> ()  [unwired: 8 in]
      }
      n378 = while {
        tunnel: w597 -> [w620]
        tunnel: [w620] -> _
        stop <- w602 stop-if-true
        # "Shoot Preload"
        n379 = Wait (ms)(milliseconds to wait=u32 20) -> ()  [unwired: 1 out]
        n380 = call-poly <vilib>:"NT Read Value.vi"("name"="PID Ctrl") -> ("value"=w600:dbl[])  [unwired: 8 in, 2 out]
        n381 = call-poly <vilib>:"NT Read Value.vi"("default value"=0.0, "name"="Shooter/Speed_RPM Act") -> ("value"=w615:dbl)  [unwired: 7 in, 2 out]
        n382 = Index Array(array=w600) -> (element #3=w599:dbl)  [unwired: 3 in, 2 out]
        n383 = call-poly <vilib>:"NT Read Value.vi"("name"="Shooter/Angle_Deg Act") -> ("value"=w606:dbl)  [unwired: 8 in, 2 out]
        n384 = call-poly <vilib>:"NT Read Value.vi"("name"="Shooter/Angle_Deg Dmd") -> ("value"=w605:dbl)  [unwired: 8 in, 2 out]
        n385 = call-poly <vilib>:"NT Write Value.vi"("value"="Shoot Mode" ("default value"), "name"="Robot State") -> ()  [unwired: 9 in, 1 out]
        n386 = Greater?(x=w615, y=2000.0) -> (0:w604:bool)
        n387 = call <vilib>:"Util_ApproxEquals.vi"("Tolerance"=2.0, "Value 2"=w605, "Value 1"=w606) -> ("ApproxEquals"=w603:bool)  [unwired: 8 in]
        n388 = And(x=w604, y=w603) -> (x .and. y?=w602:bool)
        n389 = case shown="True" w602 {
          frame False {
            n390 = call-poly <vilib>:"NT Write Value.vi"("value"="Stop" ("default value"), "name"="Intake/Trigger Status") -> ()  [unwired: 9 in, 1 out]
          }
          frame True {
            n391 = call-poly <vilib>:"NT Write Value.vi"("value"="ToShooter" ("default value"), "name"="Intake/Trigger Status") -> ()  [unwired: 9 in, 1 out]
          }
        }
        n392 = call-poly <vilib>:"NT Write Value.vi"("value"=TRUE, "name"="Shooter/Overwrite Angle") -> ()  [unwired: 9 in, 1 out]
        n393 = call-poly <vilib>:"NT Write Value.vi"("value"=w599, "name"="Shooter/Angle_Deg Dmd") -> ()  [unwired: 9 in, 1 out]
      }
    }
    frame "Preload A Red" {
      w639 = errorcluster {"status"=FALSE, "code"=0, "source"=""}  # Start Error Flow
      n394 = while {
        tunnel: w639 -> [w678]
        tunnel: [w678] -> w638
        i -> [w676]
        stop <- w675 stop-if-true
        w672 = TRUE  # ABS Odo Initialize
        w674 = 0.0 ("Drv X Vel Dmd")
        n395 = Not Equal To 0?(x=w676) -> (x != 0?=w675:bool)
        n396 = Wait (ms)(milliseconds to wait=u32 20) -> ()  [unwired: 1 out]
        n397 = call-poly <vilib>:"NT Read Value.vi"("default value"="Path_Testing_1.path" ("Trajectory File Name"), "name"="Initial Path") -> ("value"=w669:string)  [unwired: 7 in, 2 out]
        n398 = call "SWERVE_DRIVE_MODULE_STATES_POSITIONS_FGV.vi"() -> ("out Current Module Positions"=w666:T11[])  [unwired: 10 in, 1 out]
        n399 = call "SWERVE_DRIVE_GET_GYRO.vi"() -> ("Gyro Heading Radians"=w668:dbl)  [unwired: 11 in]
        n400 = call "SWERVE_DRIVE_GET_GYRO.vi"() -> ("Gyro Heading Radians"=w673:dbl)  [unwired: 11 in]
        n401 = call <vilib>:"Rotation2d_CreateAngle.vi"("Angle"=w668) -> ("ROTATION"=w667:T9)  [unwired: 10 in]
        n402 = call "SWERVE_DRIVE_SET_SPEED_DEMAND.vi"("Drv Rotation Orentation Dmd"=w673, "Drv Angular Vel Dmd"=w674, "Drv Y Vel Dmd"=w674, "Drv X Vel Dmd"=w674) -> ()  [unwired: 8 in]
        n403 = call "SWERVE_TRAJECTORY_BEGIN.vi"("ABS Odo Initialize"=w672, "gyroAngle"=w667, "Module Positions"=w666, "Trajectory File Name"=w669) -> ()  [unwired: 8 in]
      }
      n404 = while {
        tunnel: w638 -> [w661]
        tunnel: [w661] -> _
        stop <- w643 stop-if-true
        # "Shoot Preload"
        n405 = Wait (ms)(milliseconds to wait=u32 20) -> ()  [unwired: 1 out]
        n406 = call-poly <vilib>:"NT Read Value.vi"("name"="PID Ctrl") -> ("value"=w641:dbl[])  [unwired: 8 in, 2 out]
        n407 = call-poly <vilib>:"NT Read Value.vi"("default value"=0.0, "name"="Shooter/Speed_RPM Act") -> ("value"=w656:dbl)  [unwired: 7 in, 2 out]
        n408 = Index Array(array=w641) -> (element #3=w640:dbl)  [unwired: 3 in, 2 out]
        n409 = call-poly <vilib>:"NT Read Value.vi"("name"="Shooter/Angle_Deg Act") -> ("value"=w647:dbl)  [unwired: 8 in, 2 out]
        n410 = call-poly <vilib>:"NT Read Value.vi"("name"="Shooter/Angle_Deg Dmd") -> ("value"=w646:dbl)  [unwired: 8 in, 2 out]
        n411 = call-poly <vilib>:"NT Write Value.vi"("value"="Shoot Mode" ("default value"), "name"="Robot State") -> ()  [unwired: 9 in, 1 out]
        n412 = Greater?(x=w656, y=2000.0) -> (0:w645:bool)
        n413 = call <vilib>:"Util_ApproxEquals.vi"("Tolerance"=2.0, "Value 2"=w646, "Value 1"=w647) -> ("ApproxEquals"=w644:bool)  [unwired: 8 in]
        n414 = And(x=w645, y=w644) -> (x .and. y?=w643:bool)
        n415 = case shown="True" w643 {
          frame False {
            n416 = call-poly <vilib>:"NT Write Value.vi"("value"="Stop" ("default value"), "name"="Intake/Trigger Status") -> ()  [unwired: 9 in, 1 out]
          }
          frame True {
            n417 = call-poly <vilib>:"NT Write Value.vi"("value"="ToShooter" ("default value"), "name"="Intake/Trigger Status") -> ()  [unwired: 9 in, 1 out]
          }
        }
        n418 = call-poly <vilib>:"NT Write Value.vi"("value"=TRUE, "name"="Shooter/Overwrite Angle") -> ()  [unwired: 9 in, 1 out]
        n419 = call-poly <vilib>:"NT Write Value.vi"("value"=w640, "name"="Shooter/Angle_Deg Dmd") -> ()  [unwired: 9 in, 1 out]
      }
    }
    frame "Route B2 Blue" {
      w689 = errorcluster {"status"=FALSE, "code"=0, "source"=""}  # Start Error Flow
      n420 = while {
        tunnel: w689 -> [w818]
        tunnel: [w818] -> w685
        i -> [w816]
        stop <- w815 stop-if-true
        w812 = TRUE  # ABS Odo Initialize
        w814 = 0.0 ("Drv X Vel Dmd")
        n421 = Not Equal To 0?(x=w816) -> (x != 0?=w815:bool)
        n422 = Wait (ms)(milliseconds to wait=u32 20) -> ()  [unwired: 1 out]
        n423 = call-poly <vilib>:"NT Read Value.vi"("default value"="Path_Testing_1.path" ("Trajectory File Name"), "name"="Initial Path") -> ("value"=w809:string)  [unwired: 7 in, 2 out]
        n424 = call "SWERVE_DRIVE_MODULE_STATES_POSITIONS_FGV.vi"() -> ("out Current Module Positions"=w806:T11[])  [unwired: 10 in, 1 out]
        n425 = call "SWERVE_DRIVE_GET_GYRO.vi"() -> ("Gyro Heading Radians"=w808:dbl)  [unwired: 11 in]
        n426 = call "SWERVE_DRIVE_GET_GYRO.vi"() -> ("Gyro Heading Radians"=w813:dbl)  [unwired: 11 in]
        n427 = call <vilib>:"Rotation2d_CreateAngle.vi"("Angle"=w808) -> ("ROTATION"=w807:T9)  [unwired: 10 in]
        n428 = call "SWERVE_DRIVE_SET_SPEED_DEMAND.vi"("Drv Rotation Orentation Dmd"=w813, "Drv Angular Vel Dmd"=w814, "Drv Y Vel Dmd"=w814, "Drv X Vel Dmd"=w814) -> ()  [unwired: 8 in]
        n429 = call "SWERVE_TRAJECTORY_BEGIN.vi"("ABS Odo Initialize"=w812, "gyroAngle"=w807, "Module Positions"=w806, "Trajectory File Name"=w809) -> ()  [unwired: 8 in]
      }
      n430 = while {
        tunnel: w685 -> [w789]
        tunnel: [w789] -> w687
        stop <- w781 stop-if-true
        # "Shoot Preload"
        n431 = Wait (ms)(milliseconds to wait=u32 20) -> ()  [unwired: 1 out]
        n432 = call-poly <vilib>:"NT Read Value.vi"("default value"=0.0, "name"="Shooter/Speed_RPM Act") -> ("value"=w784:dbl)  [unwired: 7 in, 2 out]
        n433 = call-poly <vilib>:"NT Write Value.vi"("value"="Shoot Mode" ("default value"), "name"="Robot State") -> ()  [unwired: 9 in, 1 out]
        n434 = Greater?(x=w784, y=3000.0) -> (0:w781:bool)
        n435 = case shown="True" w781 {
          frame False {
            n436 = call-poly <vilib>:"NT Write Value.vi"("value"="Stop" ("default value"), "name"="Intake/Trigger Status") -> ()  [unwired: 9 in, 1 out]
          }
          frame True {
            n437 = call-poly <vilib>:"NT Write Value.vi"("value"="ToShooter" ("default value"), "name"="Intake/Trigger Status") -> ()  [unwired: 9 in, 1 out]
          }
        }
      }
      n438 = while {
        tunnel: w687 -> [w780]
        tunnel: [w780] -> w686
        i -> [w778]
        stop <- w777 stop-if-true
        # "Wait until shooting finishes"
        n439 = Equal To 0?(x=w778) -> (x = 0?=w777:bool)
        n440 = Wait (ms)(milliseconds to wait=u32 300) -> ()  [unwired: 1 out]
      }
      n441 = while {
        tunnel: w686 -> [w850]
        tunnel: [w850] -> w688
        i -> [w849]
        stop <- w832 stop-if-true
        w833 = TRUE  # ABS_Traj ?
        w841 = TRUE  # EnableClosedLoop
        w839 = FALSE  # Reverse
        w843 = TRUE  # Follow Orientation
        # "Use Shoot Mode to grab GP but stop the trigger when limit switch pressed"
        n442 = Equal To 0?(x=w849) -> (x = 0?=w840:bool)
        n443 = call "SWERVE_DRIVE_GET_SPEED_DEMAND.vi"() -> ("Drv Rotation Orentation Dmd"=w848:dbl)  [unwired: 8 in, 3 out]
        n444 = call "SWERVE_DRIVE_GET_GYRO.vi"() -> ("Gyro Heading Radians"=w838:dbl)  [unwired: 11 in]
        n445 = Wait Until Next ms Multiple(millisecond multiple=u32 20 ("milliseconds to wait")) -> ()  [unwired: 1 out]
        n446 = call "SWERVE_TRAJECTORY_EXECUTE.vi"("EnableClosedLoop"=w841, "ABS_Traj ?"=w833, "Init"=w840, "Reverse"=w839, "Follow Orientation"=w843, "Gyro Heading\nRAD"=w838) -> ("AtReference"=w834:bool, "OutputTRAJ_STATE"=w835:T12, "Error and Corr"=w836:T13, "Chassis Velocity Target"=w842:T14, "Orientation Target"=w837:dbl)  [unwired: 1 in]
        n447 = Select(t=w838, s=w843, f=w848) -> (s? t:f=w844:dbl)
        n448 = call "SWERVE_TRAJECTORY_SET_CLOSED_LOOP.vi"("AUTO_CLOSED_LOOP"=w841) -> ()  [unwired: 11 in]
        n449 = call "SWERVE_TRAJECTORY_UPDATE_DIAG_INFO.vi"("AtReference"=w834, "OutputTRAJ_STATE"=w835, "Error and Corr"=w836, "Orientation Target"=w837) -> ()  [unwired: 8 in]
        n450 = Unbundle By Name(w842) -> ("vX"=w847:dbl, "vY"=w846:dbl, "vOmega"=w845:dbl)
        n451 = global read "SWERVE_TRAJECTORY_GLOBALS.vi" "Traj_Total_Time"() -> (w831:dbl)
        n452 = Unbundle By Name(w835) -> ("TimeSeconds"=w830:dbl)
        n453 = call "SWERVE_DRIVE_SET_SPEED_DEMAND.vi"("Drv Rotation Orentation Dmd"=w844, "Drv Angular Vel Dmd"=w845, "Drv Y Vel Dmd"=w846, "Drv X Vel Dmd"=w847) -> ()  [unwired: 8 in]
        n454 = Equal?(x=w830, y=w831) -> (x = y?=w832:bool)
        n455 = call-poly <vilib>:"NT Write Value.vi"("value"=TRUE, "name"="Shooter/Overwrite Angle") -> ()  [unwired: 9 in, 1 out]
        n456 = call-poly <vilib>:"NT Read Value.vi"("default value"=FALSE ("value"), "name"="Shooter/Limited") -> ("value"=w827:bool)  [unwired: 7 in, 2 out]
        n457 = Select(t="Stop" ("default value"), s=w827, f="FromIntake") -> (s? t:f=w823:string)
        n458 = call-poly <vilib>:"NT Write Value.vi"("value"=w823, "name"="Intake/Trigger Status") -> ()  [unwired: 9 in, 1 out]
        n459 = call-poly <vilib>:"NT Write Value.vi"("value"=36.8, "name"="Shooter/Angle_Deg Dmd") -> ()  [unwired: 9 in, 1 out]
      }
      n460 = while {
        tunnel: w688 -> [w805]
        tunnel: [w805] -> w679
        i -> [w803]
        stop <- w802 stop-if-true
        w801 = 0.0 ("Drv X Vel Dmd")
        n461 = Not Equal To 0?(x=w803) -> (x != 0?=w802:bool)
        n462 = Wait (ms)(milliseconds to wait=u32 20) -> ()  [unwired: 1 out]
        n463 = call-poly <vilib>:"NT Write Value.vi"("value"="ToShooter" ("default value"), "name"="Intake/Trigger Status") -> ()  [unwired: 9 in, 1 out]
        n464 = call "SWERVE_DRIVE_MODULE_STATES_POSITIONS_FGV.vi"() -> ("out Current Module Positions"=w797:T11[])  [unwired: 10 in, 1 out]
        n465 = call "SWERVE_DRIVE_GET_GYRO.vi"() -> ("Gyro Heading Radians"=w799:dbl)  [unwired: 11 in]
        n466 = call "SWERVE_DRIVE_GET_GYRO.vi"() -> ("Gyro Heading Radians"=w800:dbl)  [unwired: 11 in]
        n467 = call <vilib>:"Rotation2d_CreateAngle.vi"("Angle"=w799) -> ("ROTATION"=w798:T9)  [unwired: 10 in]
        n468 = call "SWERVE_DRIVE_SET_SPEED_DEMAND.vi"("Drv Rotation Orentation Dmd"=w800, "Drv Angular Vel Dmd"=w801, "Drv Y Vel Dmd"=w801, "Drv X Vel Dmd"=w801) -> ()  [unwired: 8 in]
        n469 = call "SWERVE_TRAJECTORY_BEGIN.vi"("gyroAngle"=w798, "Module Positions"=w797, "Trajectory File Name"="Path Demo.wpilib.csv") -> ()  [unwired: 9 in]
      }
      n470 = while {
        tunnel: w679 -> [w765]
        tunnel: [w765] -> w684
        i -> [w763]
        stop <- w762 stop-if-true
        # "Wait until shooting finishes"
        n471 = Equal To 0?(x=w763) -> (x = 0?=w762:bool)
        n472 = Wait (ms)(milliseconds to wait=u32 300) -> ()  [unwired: 1 out]
      }
      n473 = while {
        tunnel: w684 -> [w776]
        tunnel: [w776] -> w683
        i -> [w774]
        stop <- w773 stop-if-true
        w770 = FALSE  # ABS Odo Initialize
        w772 = 0.0 ("Drv X Vel Dmd")
        n474 = Not Equal To 0?(x=w774) -> (x != 0?=w773:bool)
        n475 = Wait (ms)(milliseconds to wait=u32 20) -> ()  [unwired: 1 out]
        n476 = call "SWERVE_DRIVE_MODULE_STATES_POSITIONS_FGV.vi"() -> ("out Current Module Positions"=w767:T11[])  [unwired: 10 in, 1 out]
        n477 = call "SWERVE_DRIVE_GET_GYRO.vi"() -> ("Gyro Heading Radians"=w769:dbl)  [unwired: 11 in]
        n478 = call "SWERVE_DRIVE_GET_GYRO.vi"() -> ("Gyro Heading Radians"=w771:dbl)  [unwired: 11 in]
        n479 = call <vilib>:"Rotation2d_CreateAngle.vi"("Angle"=w769) -> ("ROTATION"=w768:T9)  [unwired: 10 in]
        n480 = call "SWERVE_DRIVE_SET_SPEED_DEMAND.vi"("Drv Rotation Orentation Dmd"=w771, "Drv Angular Vel Dmd"=w772, "Drv Y Vel Dmd"=w772, "Drv X Vel Dmd"=w772) -> ()  [unwired: 8 in]
        n481 = call "SWERVE_TRAJECTORY_BEGIN.vi"("ABS Odo Initialize"=w770, "gyroAngle"=w768, "Module Positions"=w767, "Trajectory File Name"="Route B2 B Path 2.path") -> ()  [unwired: 8 in]
      }
      n482 = while {
        tunnel: [w759] -> w681
        tunnel: w683 -> [w759]
        stop <- w755 stop-if-true
        # "Robot entering stage area\n=> don't move until shooter is retracted"
        n483 = call-poly <vilib>:"NT Write Value.vi"("value"="Intake Mode" ("default value"), "name"="Robot State") -> ()  [unwired: 9 in, 1 out]
        n484 = call-poly <vilib>:"NT Read Value.vi"("name"="Shooter/Angle_Deg Act") -> ("value"=w757:dbl)  [unwired: 8 in, 2 out]
        n485 = Less?(x=w757, y=19.0) -> (x < y?=w755:bool)
        n486 = Wait (ms)(milliseconds to wait=u32 20) -> ()  [unwired: 1 out]
        n487 = call-poly <vilib>:"NT Write Value.vi"("value"=FALSE, "name"="Shooter/Overwrite Angle") -> ()  [unwired: 9 in, 1 out]
      }
      n488 = while {
        tunnel: w681 -> [w738]
        tunnel: [w738] -> w682
        i -> [w718]
        stop <- w721 stop-if-true
        w722 = TRUE  # ABS_Traj ?
        w730 = TRUE  # EnableClosedLoop
        w728 = FALSE  # Reverse
        w732 = TRUE  # Follow Orientation
        n489 = call "SWERVE_DRIVE_GET_SPEED_DEMAND.vi"() -> ("Drv Rotation Orentation Dmd"=w737:dbl)  [unwired: 8 in, 3 out]
        n490 = call "SWERVE_DRIVE_GET_GYRO.vi"() -> ("Gyro Heading Radians"=w727:dbl)  [unwired: 11 in]
        n491 = Wait (ms)(milliseconds to wait=u32 20) -> ()  [unwired: 1 out]
        n492 = Equal To 0?(x=w718) -> (x = 0?=w729:bool)
        n493 = call "SWERVE_TRAJECTORY_EXECUTE.vi"("EnableClosedLoop"=w730, "ABS_Traj ?"=w722, "Init"=w729, "Reverse"=w728, "Follow Orientation"=w732, "Gyro Heading\nRAD"=w727) -> ("AtReference"=w723:bool, "OutputTRAJ_STATE"=w724:T12, "Error and Corr"=w725:T13, "Chassis Velocity Target"=w731:T14, "Orientation Target"=w726:dbl)  [unwired: 1 in]
        n494 = Select(t=w727, s=w732, f=w737) -> (s? t:f=w733:dbl)
        n495 = call "SWERVE_TRAJECTORY_SET_CLOSED_LOOP.vi"("AUTO_CLOSED_LOOP"=w730) -> ()  [unwired: 11 in]
        n496 = call "SWERVE_TRAJECTORY_UPDATE_DIAG_INFO.vi"("AtReference"=w723, "OutputTRAJ_STATE"=w724, "Error and Corr"=w725, "Orientation Target"=w726) -> ()  [unwired: 8 in]
        n497 = Unbundle By Name(w731) -> ("vX"=w736:dbl, "vY"=w735:dbl, "vOmega"=w734:dbl)
        n498 = global read "SWERVE_TRAJECTORY_GLOBALS.vi" "Traj_Total_Time"() -> (w719:dbl)
        n499 = Unbundle By Name(w724) -> ("TimeSeconds"=w720:dbl)
        n500 = call "SWERVE_DRIVE_SET_SPEED_DEMAND.vi"("Drv Rotation Orentation Dmd"=w733, "Drv Angular Vel Dmd"=w734, "Drv Y Vel Dmd"=w735, "Drv X Vel Dmd"=w736) -> ()  [unwired: 8 in]
        n501 = Equal?(x=w720, y=w719) -> (x = y?=w721:bool)
      }
      n502 = while {
        tunnel: w682 -> [w751]
        tunnel: [w751] -> w680
        i -> [w749]
        stop <- w748 stop-if-true
        w747 = 0.0 ("Drv X Vel Dmd")
        n503 = Not Equal To 0?(x=w749) -> (x != 0?=w748:bool)
        n504 = Wait (ms)(milliseconds to wait=u32 20) -> ()  [unwired: 1 out]
        n505 = call-poly <vilib>:"NT Write Value.vi"("value"="Shoot Mode" ("default value"), "name"="Robot State") -> ()  [unwired: 9 in, 1 out]
        n506 = call "SWERVE_DRIVE_MODULE_STATES_POSITIONS_FGV.vi"() -> ("out Current Module Positions"=w743:T11[])  [unwired: 10 in, 1 out]
        n507 = call "SWERVE_DRIVE_GET_GYRO.vi"() -> ("Gyro Heading Radians"=w745:dbl)  [unwired: 11 in]
        n508 = call "SWERVE_DRIVE_GET_GYRO.vi"() -> ("Gyro Heading Radians"=w746:dbl)  [unwired: 11 in]
        n509 = call <vilib>:"Rotation2d_CreateAngle.vi"("Angle"=w745) -> ("ROTATION"=w744:T9)  [unwired: 10 in]
        n510 = call "SWERVE_DRIVE_SET_SPEED_DEMAND.vi"("Drv Rotation Orentation Dmd"=w746, "Drv Angular Vel Dmd"=w747, "Drv Y Vel Dmd"=w747, "Drv X Vel Dmd"=w747) -> ()  [unwired: 8 in]
        n511 = call "SWERVE_TRAJECTORY_BEGIN.vi"("gyroAngle"=w744, "Module Positions"=w743, "Trajectory File Name"="Path Demo.wpilib.csv") -> ()  [unwired: 9 in]
      }
      n512 = while {
        tunnel: w680 -> [w713]
        tunnel: [w713] -> _
        i -> [w694]
        stop <- FALSE stop-if-true
        w701 = 0.0 ("Drv X Vel Dmd")
        n513 = Greater?(x=w694, y=25) -> (0:w690:bool)
        n514 = call-poly <vilib>:"NT Read Value.vi"("name"="/limelight-shooter/tv") -> ("value"=w704:dbl)  [unwired: 8 in, 2 out]
        n515 = call-poly <vilib>:"NT Read Value.vi"("name"="Shooter/Corrected Theta") -> ("value"=w698:dbl)  [unwired: 8 in, 2 out]
        n516 = call-poly <vilib>:"NT Read Value.vi"("name"="Shooter/Angle_Deg Act") -> ("value"=w710:dbl)  [unwired: 8 in, 2 out]
        n517 = call-poly <vilib>:"NT Read Value.vi"("name"="Shooter/Angle_Deg Dmd") -> ("value"=w709:dbl)  [unwired: 8 in, 2 out]
        n518 = Not Equal To 0?(x=w704) -> (x != 0?=w703:bool)
        n519 = call "SWERVE_DRIVE_GET_GYRO.vi"() -> ("Gyro Heading Radians"=w699:dbl)  [unwired: 11 in]
        n520 = Select(t=w698, s=w703, f=w699) -> (s? t:f=w702:dbl)
        n521 = call <vilib>:"Util_ApproxEquals.vi"("Tolerance"=3.5, "Value 2"=w709, "Value 1"=w710) -> ("ApproxEquals"=w700:bool)  [unwired: 8 in]
        n522 = call <vilib>:"Util_ApproxEquals.vi"("Tolerance"=0.1, "Value 2"=w699, "Value 1"=w698) -> ("ApproxEquals"=w696:bool)  [unwired: 8 in]
        n523 = And(x=w700, y=w696) -> (x .and. y?=w692:bool)
        n524 = Or(x=w692, y=w690) -> (x .or. y?=w691:bool)
        n525 = case shown="False" w691 {
          frame False {
            n526 = call-poly <vilib>:"NT Write Value.vi"("value"="Stop" ("default value"), "name"="Intake/Trigger Status") -> ()  [unwired: 9 in, 1 out]
          }
          frame True {
            n527 = call-poly <vilib>:"NT Write Value.vi"("value"="ToShooter" ("default value"), "name"="Intake/Trigger Status") -> ()  [unwired: 9 in, 1 out]
          }
        }
        n528 = call "SWERVE_DRIVE_SET_SPEED_DEMAND.vi"("Drv Rotation Orentation Dmd"=w702, "Drv Angular Vel Dmd"=w701, "Drv Y Vel Dmd"=w701, "Drv X Vel Dmd"=w701) -> ()  [unwired: 8 in]
        n529 = Wait (ms)(milliseconds to wait=u32 20) -> ()  [unwired: 1 out]
      }
    }
    frame "Route B2 Red" {
      w862 = errorcluster {"status"=FALSE, "code"=0, "source"=""}  # Start Error Flow
      n530 = while {
        tunnel: w862 -> [w998]
        tunnel: [w998] -> w858
        i -> [w996]
        stop <- w995 stop-if-true
        w992 = TRUE  # ABS Odo Initialize
        w994 = 0.0 ("Drv X Vel Dmd")
        n531 = Not Equal To 0?(x=w996) -> (x != 0?=w995:bool)
        n532 = Wait (ms)(milliseconds to wait=u32 20) -> ()  [unwired: 1 out]
        n533 = call-poly <vilib>:"NT Read Value.vi"("default value"="Path_Testing_1.path" ("Trajectory File Name"), "name"="Initial Path") -> ("value"=w989:string)  [unwired: 7 in, 2 out]
        n534 = call "SWERVE_DRIVE_MODULE_STATES_POSITIONS_FGV.vi"() -> ("out Current Module Positions"=w986:T11[])  [unwired: 10 in, 1 out]
        n535 = call "SWERVE_DRIVE_GET_GYRO.vi"() -> ("Gyro Heading Radians"=w988:dbl)  [unwired: 11 in]
        n536 = call "SWERVE_DRIVE_GET_GYRO.vi"() -> ("Gyro Heading Radians"=w993:dbl)  [unwired: 11 in]
        n537 = call <vilib>:"Rotation2d_CreateAngle.vi"("Angle"=w988) -> ("ROTATION"=w987:T9)  [unwired: 10 in]
        n538 = call "SWERVE_DRIVE_SET_SPEED_DEMAND.vi"("Drv Rotation Orentation Dmd"=w993, "Drv Angular Vel Dmd"=w994, "Drv Y Vel Dmd"=w994, "Drv X Vel Dmd"=w994) -> ()  [unwired: 8 in]
        n539 = call "SWERVE_TRAJECTORY_BEGIN.vi"("ABS Odo Initialize"=w992, "gyroAngle"=w987, "Module Positions"=w986, "Trajectory File Name"=w989) -> ()  [unwired: 8 in]
      }
      n540 = while {
        tunnel: w858 -> [w969]
        tunnel: [w969] -> w860
        stop <- w961 stop-if-true
        # "Shoot Preload"
        n541 = Wait (ms)(milliseconds to wait=u32 20) -> ()  [unwired: 1 out]
        n542 = call-poly <vilib>:"NT Read Value.vi"("default value"=0.0, "name"="Shooter/Speed_RPM Act") -> ("value"=w964:dbl)  [unwired: 7 in, 2 out]
        n543 = call-poly <vilib>:"NT Write Value.vi"("value"="Shoot Mode" ("default value"), "name"="Robot State") -> ()  [unwired: 9 in, 1 out]
        n544 = Greater?(x=w964, y=3000.0) -> (0:w961:bool)
        n545 = case shown="True" w961 {
          frame False {
            n546 = call-poly <vilib>:"NT Write Value.vi"("value"="Stop" ("default value"), "name"="Intake/Trigger Status") -> ()  [unwired: 9 in, 1 out]
          }
          frame True {
            n547 = call-poly <vilib>:"NT Write Value.vi"("value"="ToShooter" ("default value"), "name"="Intake/Trigger Status") -> ()  [unwired: 9 in, 1 out]
          }
        }
      }
      n548 = while {
        tunnel: w860 -> [w960]
        tunnel: [w960] -> w859
        i -> [w958]
        stop <- w957 stop-if-true
        # "Wait until shooting finishes"
        n549 = Equal To 0?(x=w958) -> (x = 0?=w957:bool)
        n550 = Wait (ms)(milliseconds to wait=u32 300) -> ()  [unwired: 1 out]
      }
      n551 = while {
        tunnel: w859 -> [w1030]
        tunnel: [w1030] -> w861
        i -> [w1029]
        stop <- w1012 stop-if-true
        w1013 = TRUE  # ABS_Traj ?
        w1021 = TRUE  # EnableClosedLoop
        w1019 = FALSE  # Reverse
        w1023 = TRUE  # Follow Orientation
        # "Use Shoot Mode to grab GP but stop the trigger when limit switch pressed"
        n552 = Equal To 0?(x=w1029) -> (x = 0?=w1020:bool)
        n553 = call "SWERVE_DRIVE_GET_SPEED_DEMAND.vi"() -> ("Drv Rotation Orentation Dmd"=w1028:dbl)  [unwired: 8 in, 3 out]
        n554 = call "SWERVE_DRIVE_GET_GYRO.vi"() -> ("Gyro Heading Radians"=w1018:dbl)  [unwired: 11 in]
        n555 = Wait Until Next ms Multiple(millisecond multiple=u32 20 ("milliseconds to wait")) -> ()  [unwired: 1 out]
        n556 = call "SWERVE_TRAJECTORY_EXECUTE.vi"("EnableClosedLoop"=w1021, "ABS_Traj ?"=w1013, "Init"=w1020, "Reverse"=w1019, "Follow Orientation"=w1023, "Gyro Heading\nRAD"=w1018) -> ("AtReference"=w1014:bool, "OutputTRAJ_STATE"=w1015:T12, "Error and Corr"=w1016:T13, "Chassis Velocity Target"=w1022:T14, "Orientation Target"=w1017:dbl)  [unwired: 1 in]
        n557 = Select(t=w1018, s=w1023, f=w1028) -> (s? t:f=w1024:dbl)
        n558 = call "SWERVE_TRAJECTORY_SET_CLOSED_LOOP.vi"("AUTO_CLOSED_LOOP"=w1021) -> ()  [unwired: 11 in]
        n559 = call "SWERVE_TRAJECTORY_UPDATE_DIAG_INFO.vi"("AtReference"=w1014, "OutputTRAJ_STATE"=w1015, "Error and Corr"=w1016, "Orientation Target"=w1017) -> ()  [unwired: 8 in]
        n560 = Unbundle By Name(w1022) -> ("vX"=w1027:dbl, "vY"=w1026:dbl, "vOmega"=w1025:dbl)
        n561 = global read "SWERVE_TRAJECTORY_GLOBALS.vi" "Traj_Total_Time"() -> (w1011:dbl)
        n562 = Unbundle By Name(w1015) -> ("TimeSeconds"=w1010:dbl)
        n563 = call "SWERVE_DRIVE_SET_SPEED_DEMAND.vi"("Drv Rotation Orentation Dmd"=w1024, "Drv Angular Vel Dmd"=w1025, "Drv Y Vel Dmd"=w1026, "Drv X Vel Dmd"=w1027) -> ()  [unwired: 8 in]
        n564 = Equal?(x=w1010, y=w1011) -> (x = y?=w1012:bool)
        n565 = call-poly <vilib>:"NT Write Value.vi"("value"=TRUE, "name"="Shooter/Overwrite Angle") -> ()  [unwired: 9 in, 1 out]
        n566 = call-poly <vilib>:"NT Read Value.vi"("default value"=FALSE ("value"), "name"="Shooter/Limited") -> ("value"=w1007:bool)  [unwired: 7 in, 2 out]
        n567 = Select(t="Stop" ("default value"), s=w1007, f="FromIntake") -> (s? t:f=w1003:string)
        n568 = call-poly <vilib>:"NT Write Value.vi"("value"=w1003, "name"="Intake/Trigger Status") -> ()  [unwired: 9 in, 1 out]
        n569 = call-poly <vilib>:"NT Write Value.vi"("value"=36.8, "name"="Shooter/Angle_Deg Dmd") -> ()  [unwired: 9 in, 1 out]
      }
      n570 = while {
        tunnel: w861 -> [w985]
        tunnel: [w985] -> w852
        i -> [w983]
        stop <- w982 stop-if-true
        w981 = 0.0 ("Drv X Vel Dmd")
        n571 = Not Equal To 0?(x=w983) -> (x != 0?=w982:bool)
        n572 = Wait (ms)(milliseconds to wait=u32 20) -> ()  [unwired: 1 out]
        n573 = call-poly <vilib>:"NT Write Value.vi"("value"="ToShooter" ("default value"), "name"="Intake/Trigger Status") -> ()  [unwired: 9 in, 1 out]
        n574 = call "SWERVE_DRIVE_MODULE_STATES_POSITIONS_FGV.vi"() -> ("out Current Module Positions"=w977:T11[])  [unwired: 10 in, 1 out]
        n575 = call "SWERVE_DRIVE_GET_GYRO.vi"() -> ("Gyro Heading Radians"=w979:dbl)  [unwired: 11 in]
        n576 = call "SWERVE_DRIVE_GET_GYRO.vi"() -> ("Gyro Heading Radians"=w980:dbl)  [unwired: 11 in]
        n577 = call <vilib>:"Rotation2d_CreateAngle.vi"("Angle"=w979) -> ("ROTATION"=w978:T9)  [unwired: 10 in]
        n578 = call "SWERVE_DRIVE_SET_SPEED_DEMAND.vi"("Drv Rotation Orentation Dmd"=w980, "Drv Angular Vel Dmd"=w981, "Drv Y Vel Dmd"=w981, "Drv X Vel Dmd"=w981) -> ()  [unwired: 8 in]
        n579 = call "SWERVE_TRAJECTORY_BEGIN.vi"("gyroAngle"=w978, "Module Positions"=w977, "Trajectory File Name"="Path Demo.wpilib.csv") -> ()  [unwired: 9 in]
      }
      n580 = while {
        tunnel: w852 -> [w945]
        tunnel: [w945] -> w857
        i -> [w943]
        stop <- w942 stop-if-true
        # "Wait until shooting finishes"
        n581 = Equal To 0?(x=w943) -> (x = 0?=w942:bool)
        n582 = Wait (ms)(milliseconds to wait=u32 300) -> ()  [unwired: 1 out]
      }
      n583 = while {
        tunnel: w857 -> [w956]
        tunnel: [w956] -> w856
        i -> [w954]
        stop <- w953 stop-if-true
        w950 = FALSE  # ABS Odo Initialize
        w952 = 0.0 ("Drv X Vel Dmd")
        n584 = Not Equal To 0?(x=w954) -> (x != 0?=w953:bool)
        n585 = Wait (ms)(milliseconds to wait=u32 20) -> ()  [unwired: 1 out]
        n586 = call "SWERVE_DRIVE_MODULE_STATES_POSITIONS_FGV.vi"() -> ("out Current Module Positions"=w947:T11[])  [unwired: 10 in, 1 out]
        n587 = call "SWERVE_DRIVE_GET_GYRO.vi"() -> ("Gyro Heading Radians"=w949:dbl)  [unwired: 11 in]
        n588 = call "SWERVE_DRIVE_GET_GYRO.vi"() -> ("Gyro Heading Radians"=w951:dbl)  [unwired: 11 in]
        n589 = call <vilib>:"Rotation2d_CreateAngle.vi"("Angle"=w949) -> ("ROTATION"=w948:T9)  [unwired: 10 in]
        n590 = call "SWERVE_DRIVE_SET_SPEED_DEMAND.vi"("Drv Rotation Orentation Dmd"=w951, "Drv Angular Vel Dmd"=w952, "Drv Y Vel Dmd"=w952, "Drv X Vel Dmd"=w952) -> ()  [unwired: 8 in]
        n591 = call "SWERVE_TRAJECTORY_BEGIN.vi"("ABS Odo Initialize"=w950, "gyroAngle"=w948, "Module Positions"=w947, "Trajectory File Name"="Route B2 R Path 2.path") -> ()  [unwired: 8 in]
      }
      n592 = while {
        tunnel: [w939] -> w854
        tunnel: w856 -> [w939]
        stop <- w935 stop-if-true
        # "Robot entering stage area\n=> don't move until shooter is retracted"
        n593 = call-poly <vilib>:"NT Write Value.vi"("value"="Intake Mode" ("default value"), "name"="Robot State") -> ()  [unwired: 9 in, 1 out]
        n594 = call-poly <vilib>:"NT Read Value.vi"("name"="Shooter/Angle_Deg Act") -> ("value"=w937:dbl)  [unwired: 8 in, 2 out]
        n595 = Less?(x=w937, y=19.0) -> (x < y?=w935:bool)
        n596 = Wait (ms)(milliseconds to wait=u32 20) -> ()  [unwired: 1 out]
        n597 = call-poly <vilib>:"NT Write Value.vi"("value"=FALSE, "name"="Shooter/Overwrite Angle") -> ()  [unwired: 9 in, 1 out]
      }
      n598 = while {
        tunnel: w854 -> [w918]
        tunnel: [w918] -> w855
        i -> [w898]
        stop <- w901 stop-if-true
        w902 = TRUE  # ABS_Traj ?
        w910 = TRUE  # EnableClosedLoop
        w908 = FALSE  # Reverse
        w912 = TRUE  # Follow Orientation
        n599 = call "SWERVE_DRIVE_GET_SPEED_DEMAND.vi"() -> ("Drv Rotation Orentation Dmd"=w917:dbl)  [unwired: 8 in, 3 out]
        n600 = call "SWERVE_DRIVE_GET_GYRO.vi"() -> ("Gyro Heading Radians"=w907:dbl)  [unwired: 11 in]
        n601 = Wait (ms)(milliseconds to wait=u32 20) -> ()  [unwired: 1 out]
        n602 = Equal To 0?(x=w898) -> (x = 0?=w909:bool)
        n603 = call "SWERVE_TRAJECTORY_EXECUTE.vi"("EnableClosedLoop"=w910, "ABS_Traj ?"=w902, "Init"=w909, "Reverse"=w908, "Follow Orientation"=w912, "Gyro Heading\nRAD"=w907) -> ("AtReference"=w903:bool, "OutputTRAJ_STATE"=w904:T12, "Error and Corr"=w905:T13, "Chassis Velocity Target"=w911:T14, "Orientation Target"=w906:dbl)  [unwired: 1 in]
        n604 = Select(t=w907, s=w912, f=w917) -> (s? t:f=w913:dbl)
        n605 = call "SWERVE_TRAJECTORY_SET_CLOSED_LOOP.vi"("AUTO_CLOSED_LOOP"=w910) -> ()  [unwired: 11 in]
        n606 = call "SWERVE_TRAJECTORY_UPDATE_DIAG_INFO.vi"("AtReference"=w903, "OutputTRAJ_STATE"=w904, "Error and Corr"=w905, "Orientation Target"=w906) -> ()  [unwired: 8 in]
        n607 = Unbundle By Name(w911) -> ("vX"=w916:dbl, "vY"=w915:dbl, "vOmega"=w914:dbl)
        n608 = global read "SWERVE_TRAJECTORY_GLOBALS.vi" "Traj_Total_Time"() -> (w899:dbl)
        n609 = Unbundle By Name(w904) -> ("TimeSeconds"=w900:dbl)
        n610 = call "SWERVE_DRIVE_SET_SPEED_DEMAND.vi"("Drv Rotation Orentation Dmd"=w913, "Drv Angular Vel Dmd"=w914, "Drv Y Vel Dmd"=w915, "Drv X Vel Dmd"=w916) -> ()  [unwired: 8 in]
        n611 = Equal?(x=w900, y=w899) -> (x = y?=w901:bool)
        n612 = call-poly <vilib>:"NT Read Value.vi"("default value"=FALSE ("value"), "name"="Shooter/Limited") -> ("value"=w895:bool)  [unwired: 7 in, 2 out]
        n613 = Select(t="Stop" ("default value"), s=w895, f="FromIntake") -> (s? t:f=w891:string)
        n614 = call-poly <vilib>:"NT Write Value.vi"("value"=w891, "name"="Intake/Trigger Status") -> ()  [unwired: 9 in, 1 out]
      }
      n615 = while {
        tunnel: w855 -> [w931]
        tunnel: [w931] -> w853
        i -> [w929]
        stop <- w928 stop-if-true
        w927 = 0.0 ("Drv X Vel Dmd")
        n616 = Not Equal To 0?(x=w929) -> (x != 0?=w928:bool)
        n617 = Wait (ms)(milliseconds to wait=u32 20) -> ()  [unwired: 1 out]
        n618 = call-poly <vilib>:"NT Write Value.vi"("value"="Shoot Mode" ("default value"), "name"="Robot State") -> ()  [unwired: 9 in, 1 out]
        n619 = call "SWERVE_DRIVE_MODULE_STATES_POSITIONS_FGV.vi"() -> ("out Current Module Positions"=w923:T11[])  [unwired: 10 in, 1 out]
        n620 = call "SWERVE_DRIVE_GET_GYRO.vi"() -> ("Gyro Heading Radians"=w925:dbl)  [unwired: 11 in]
        n621 = call "SWERVE_DRIVE_GET_GYRO.vi"() -> ("Gyro Heading Radians"=w926:dbl)  [unwired: 11 in]
        n622 = call <vilib>:"Rotation2d_CreateAngle.vi"("Angle"=w925) -> ("ROTATION"=w924:T9)  [unwired: 10 in]
        n623 = call "SWERVE_DRIVE_SET_SPEED_DEMAND.vi"("Drv Rotation Orentation Dmd"=w926, "Drv Angular Vel Dmd"=w927, "Drv Y Vel Dmd"=w927, "Drv X Vel Dmd"=w927) -> ()  [unwired: 8 in]
        n624 = call "SWERVE_TRAJECTORY_BEGIN.vi"("gyroAngle"=w924, "Module Positions"=w923, "Trajectory File Name"="Path Demo.wpilib.csv") -> ()  [unwired: 9 in]
      }
      n625 = while {
        tunnel: w853 -> [w886]
        tunnel: [w886] -> _
        i -> [w867]
        stop <- FALSE stop-if-true
        w874 = 0.0 ("Drv X Vel Dmd")
        n626 = Greater?(x=w867, y=25) -> (0:w863:bool)
        n627 = call-poly <vilib>:"NT Read Value.vi"("name"="/limelight-shooter/tv") -> ("value"=w877:dbl)  [unwired: 8 in, 2 out]
        n628 = call-poly <vilib>:"NT Read Value.vi"("name"="Shooter/Corrected Theta") -> ("value"=w871:dbl)  [unwired: 8 in, 2 out]
        n629 = call-poly <vilib>:"NT Read Value.vi"("name"="Shooter/Angle_Deg Act") -> ("value"=w883:dbl)  [unwired: 8 in, 2 out]
        n630 = call-poly <vilib>:"NT Read Value.vi"("name"="Shooter/Angle_Deg Dmd") -> ("value"=w882:dbl)  [unwired: 8 in, 2 out]
        n631 = Not Equal To 0?(x=w877) -> (x != 0?=w876:bool)
        n632 = call "SWERVE_DRIVE_GET_GYRO.vi"() -> ("Gyro Heading Radians"=w872:dbl)  [unwired: 11 in]
        n633 = Select(t=w871, s=w876, f=w872) -> (s? t:f=w875:dbl)
        n634 = call <vilib>:"Util_ApproxEquals.vi"("Tolerance"=3.5, "Value 2"=w882, "Value 1"=w883) -> ("ApproxEquals"=w873:bool)  [unwired: 8 in]
        n635 = call <vilib>:"Util_ApproxEquals.vi"("Tolerance"=0.1, "Value 2"=w872, "Value 1"=w871) -> ("ApproxEquals"=w869:bool)  [unwired: 8 in]
        n636 = And(x=w873, y=w869) -> (x .and. y?=w865:bool)
        n637 = Or(x=w865, y=w863) -> (x .or. y?=w864:bool)
        n638 = case shown="False" w864 {
          frame False {
            n639 = call-poly <vilib>:"NT Write Value.vi"("value"="Stop" ("default value"), "name"="Intake/Trigger Status") -> ()  [unwired: 9 in, 1 out]
          }
          frame True {
            n640 = call-poly <vilib>:"NT Write Value.vi"("value"="ToShooter" ("default value"), "name"="Intake/Trigger Status") -> ()  [unwired: 9 in, 1 out]
          }
        }
        n641 = call "SWERVE_DRIVE_SET_SPEED_DEMAND.vi"("Drv Rotation Orentation Dmd"=w875, "Drv Angular Vel Dmd"=w874, "Drv Y Vel Dmd"=w874, "Drv X Vel Dmd"=w874) -> ()  [unwired: 8 in]
        n642 = Wait (ms)(milliseconds to wait=u32 20) -> ()  [unwired: 1 out]
      }
    }
    frame "Preload B Blue" {
      w1033 = errorcluster {"status"=FALSE, "code"=0, "source"=""}  # Start Error Flow
      n643 = while {
        tunnel: w1033 -> [w1064]
        tunnel: [w1064] -> w1032
        i -> [w1062]
        stop <- w1061 stop-if-true
        w1058 = TRUE  # ABS Odo Initialize
        w1060 = 0.0 ("Drv X Vel Dmd")
        n644 = Not Equal To 0?(x=w1062) -> (x != 0?=w1061:bool)
        n645 = Wait (ms)(milliseconds to wait=u32 20) -> ()  [unwired: 1 out]
        n646 = call-poly <vilib>:"NT Read Value.vi"("default value"="Path_Testing_1.path" ("Trajectory File Name"), "name"="Initial Path") -> ("value"=w1055:string)  [unwired: 7 in, 2 out]
        n647 = call "SWERVE_DRIVE_MODULE_STATES_POSITIONS_FGV.vi"() -> ("out Current Module Positions"=w1052:T11[])  [unwired: 10 in, 1 out]
        n648 = call "SWERVE_DRIVE_GET_GYRO.vi"() -> ("Gyro Heading Radians"=w1054:dbl)  [unwired: 11 in]
        n649 = call "SWERVE_DRIVE_GET_GYRO.vi"() -> ("Gyro Heading Radians"=w1059:dbl)  [unwired: 11 in]
        n650 = call <vilib>:"Rotation2d_CreateAngle.vi"("Angle"=w1054) -> ("ROTATION"=w1053:T9)  [unwired: 10 in]
        n651 = call "SWERVE_DRIVE_SET_SPEED_DEMAND.vi"("Drv Rotation Orentation Dmd"=w1059, "Drv Angular Vel Dmd"=w1060, "Drv Y Vel Dmd"=w1060, "Drv X Vel Dmd"=w1060) -> ()  [unwired: 8 in]
        n652 = call "SWERVE_TRAJECTORY_BEGIN.vi"("ABS Odo Initialize"=w1058, "gyroAngle"=w1053, "Module Positions"=w1052, "Trajectory File Name"=w1055) -> ()  [unwired: 8 in]
      }
      n653 = while {
        tunnel: w1032 -> [w1047]
        tunnel: [w1047] -> _
        stop <- FALSE stop-if-true
        # "Shoot Preload"
        n654 = Wait (ms)(milliseconds to wait=u32 20) -> ()  [unwired: 1 out]
        n655 = call-poly <vilib>:"NT Read Value.vi"("default value"=0.0, "name"="Shooter/Speed_RPM Act") -> ("value"=w1042:dbl)  [unwired: 7 in, 2 out]
        n656 = call-poly <vilib>:"NT Write Value.vi"("value"="Shoot Mode" ("default value"), "name"="Robot State") -> ()  [unwired: 9 in, 1 out]
        n657 = Greater?(x=w1042, y=3500.0) -> (0:w1040:bool)
        n658 = case shown="True" w1040 {
          frame False {
            n659 = call-poly <vilib>:"NT Write Value.vi"("value"="Stop" ("default value"), "name"="Intake/Trigger Status") -> ()  [unwired: 9 in, 1 out]
          }
          frame True {
            n660 = call-poly <vilib>:"NT Write Value.vi"("value"="ToShooter" ("default value"), "name"="Intake/Trigger Status") -> ()  [unwired: 9 in, 1 out]
          }
        }
        n661 = call-poly <vilib>:"NT Write Value.vi"("value"=TRUE, "name"="Shooter/Overwrite Angle") -> ()  [unwired: 9 in, 1 out]
        n662 = call-poly <vilib>:"NT Write Value.vi"("value"=52.0, "name"="Shooter/Angle_Deg Dmd") -> ()  [unwired: 9 in, 1 out]
      }
    }
    frame "Preload B Red" {
      w1066 = errorcluster {"status"=FALSE, "code"=0, "source"=""}  # Start Error Flow
      n663 = while {
        tunnel: w1066 -> [w1097]
        tunnel: [w1097] -> w1065
        i -> [w1095]
        stop <- w1094 stop-if-true
        w1091 = TRUE  # ABS Odo Initialize
        w1093 = 0.0 ("Drv X Vel Dmd")
        n664 = Not Equal To 0?(x=w1095) -> (x != 0?=w1094:bool)
        n665 = Wait (ms)(milliseconds to wait=u32 20) -> ()  [unwired: 1 out]
        n666 = call-poly <vilib>:"NT Read Value.vi"("default value"="Path_Testing_1.path" ("Trajectory File Name"), "name"="Initial Path") -> ("value"=w1088:string)  [unwired: 7 in, 2 out]
        n667 = call "SWERVE_DRIVE_MODULE_STATES_POSITIONS_FGV.vi"() -> ("out Current Module Positions"=w1085:T11[])  [unwired: 10 in, 1 out]
        n668 = call "SWERVE_DRIVE_GET_GYRO.vi"() -> ("Gyro Heading Radians"=w1087:dbl)  [unwired: 11 in]
        n669 = call "SWERVE_DRIVE_GET_GYRO.vi"() -> ("Gyro Heading Radians"=w1092:dbl)  [unwired: 11 in]
        n670 = call <vilib>:"Rotation2d_CreateAngle.vi"("Angle"=w1087) -> ("ROTATION"=w1086:T9)  [unwired: 10 in]
        n671 = call "SWERVE_DRIVE_SET_SPEED_DEMAND.vi"("Drv Rotation Orentation Dmd"=w1092, "Drv Angular Vel Dmd"=w1093, "Drv Y Vel Dmd"=w1093, "Drv X Vel Dmd"=w1093) -> ()  [unwired: 8 in]
        n672 = call "SWERVE_TRAJECTORY_BEGIN.vi"("ABS Odo Initialize"=w1091, "gyroAngle"=w1086, "Module Positions"=w1085, "Trajectory File Name"=w1088) -> ()  [unwired: 8 in]
      }
      n673 = while {
        tunnel: w1065 -> [w1080]
        tunnel: [w1080] -> _
        stop <- FALSE stop-if-true
        # "Shoot Preload"
        n674 = Wait (ms)(milliseconds to wait=u32 20) -> ()  [unwired: 1 out]
        n675 = call-poly <vilib>:"NT Read Value.vi"("default value"=0.0, "name"="Shooter/Speed_RPM Act") -> ("value"=w1075:dbl)  [unwired: 7 in, 2 out]
        n676 = call-poly <vilib>:"NT Write Value.vi"("value"="Shoot Mode" ("default value"), "name"="Robot State") -> ()  [unwired: 9 in, 1 out]
        n677 = Greater?(x=w1075, y=3500.0) -> (0:w1073:bool)
        n678 = case shown="True" w1073 {
          frame False {
            n679 = call-poly <vilib>:"NT Write Value.vi"("value"="Stop" ("default value"), "name"="Intake/Trigger Status") -> ()  [unwired: 9 in, 1 out]
          }
          frame True {
            n680 = call-poly <vilib>:"NT Write Value.vi"("value"="ToShooter" ("default value"), "name"="Intake/Trigger Status") -> ()  [unwired: 9 in, 1 out]
          }
        }
        n681 = call-poly <vilib>:"NT Write Value.vi"("value"=TRUE, "name"="Shooter/Overwrite Angle") -> ()  [unwired: 9 in, 1 out]
        n682 = call-poly <vilib>:"NT Write Value.vi"("value"=52.0, "name"="Shooter/Angle_Deg Dmd") -> ()  [unwired: 9 in, 1 out]
      }
    }
    frame "Route C1 Blue" {
      w1107 = errorcluster {"status"=FALSE, "code"=0, "source"=""}  # Start Error Flow
      n683 = while {
        tunnel: w1107 -> [w1287]
        tunnel: [w1287] -> w1106
        i -> [w1285]
        stop <- w1284 stop-if-true
        w1281 = TRUE  # ABS Odo Initialize
        w1283 = 0.0 ("Drv X Vel Dmd")
        n684 = Not Equal To 0?(x=w1285) -> (x != 0?=w1284:bool)
        n685 = Wait (ms)(milliseconds to wait=u32 20) -> ()  [unwired: 1 out]
        n686 = call-poly <vilib>:"NT Read Value.vi"("default value"="Path_Testing_1.path" ("Trajectory File Name"), "name"="Initial Path") -> ("value"=w1278:string)  [unwired: 7 in, 2 out]
        n687 = call "SWERVE_DRIVE_MODULE_STATES_POSITIONS_FGV.vi"() -> ("out Current Module Positions"=w1275:T11[])  [unwired: 10 in, 1 out]
        n688 = call "SWERVE_DRIVE_GET_GYRO.vi"() -> ("Gyro Heading Radians"=w1277:dbl)  [unwired: 11 in]
        n689 = call "SWERVE_DRIVE_GET_GYRO.vi"() -> ("Gyro Heading Radians"=w1282:dbl)  [unwired: 11 in]
        n690 = call <vilib>:"Rotation2d_CreateAngle.vi"("Angle"=w1277) -> ("ROTATION"=w1276:T9)  [unwired: 10 in]
        n691 = call "SWERVE_DRIVE_SET_SPEED_DEMAND.vi"("Drv Rotation Orentation Dmd"=w1282, "Drv Angular Vel Dmd"=w1283, "Drv Y Vel Dmd"=w1283, "Drv X Vel Dmd"=w1283) -> ()  [unwired: 8 in]
        n692 = call "SWERVE_TRAJECTORY_BEGIN.vi"("ABS Odo Initialize"=w1281, "gyroAngle"=w1276, "Module Positions"=w1275, "Trajectory File Name"=w1278) -> ()  [unwired: 8 in]
      }
      n693 = while {
        tunnel: w1106 -> [w1270]
        tunnel: [w1270] -> w1099
        stop <- w1251 stop-if-true
        # "Shoot Preload"
        n694 = Wait (ms)(milliseconds to wait=u32 20) -> ()  [unwired: 1 out]
        n695 = call-poly <vilib>:"NT Read Value.vi"("default value"=0.0, "name"="Shooter/Speed_RPM Act") -> ("value"=w1265:dbl)  [unwired: 7 in, 2 out]
        n696 = call-poly <vilib>:"NT Read Value.vi"("name"="Shooter/Angle_Deg Act") -> ("value"=w1255:dbl)  [unwired: 8 in, 2 out]
        n697 = call-poly <vilib>:"NT Read Value.vi"("name"="Shooter/Angle_Deg Dmd") -> ("value"=w1254:dbl)  [unwired: 8 in, 2 out]
        n698 = call-poly <vilib>:"NT Write Value.vi"("value"="Shoot Mode" ("default value"), "name"="Robot State") -> ()  [unwired: 9 in, 1 out]
        n699 = call-poly <vilib>:"NT Write Value.vi"("value"=FALSE, "name"="Shooter/Overwrite RPM") -> ()  [unwired: 9 in, 1 out]
        n700 = Greater?(x=w1265, y=2000.0) -> (0:w1253:bool)
        n701 = call <vilib>:"Util_ApproxEquals.vi"("Tolerance"=3.0, "Value 2"=w1254, "Value 1"=w1255) -> ("ApproxEquals"=w1252:bool)  [unwired: 8 in]
        n702 = And(x=w1253, y=w1252) -> (x .and. y?=w1251:bool)
        n703 = case shown="True" w1251 {
          frame False {
            n704 = call-poly <vilib>:"NT Write Value.vi"("value"="Stop" ("default value"), "name"="Intake/Trigger Status") -> ()  [unwired: 9 in, 1 out]
          }
          frame True {
            n705 = call-poly <vilib>:"NT Write Value.vi"("value"="ToShooter" ("default value"), "name"="Intake/Trigger Status") -> ()  [unwired: 9 in, 1 out]
          }
        }
        n706 = call-poly <vilib>:"NT Write Value.vi"("value"=TRUE, "name"="Shooter/Overwrite Angle") -> ()  [unwired: 9 in, 1 out]
        n707 = call-poly <vilib>:"NT Write Value.vi"("value"=53.0, "name"="Shooter/Angle_Deg Dmd") -> ()  [unwired: 9 in, 1 out]
        n708 = call-poly <vilib>:"NT Write Value.vi"("value"=2500.0, "name"="Shooter/RPM Dmd") -> ()  [unwired: 9 in, 1 out]
      }
      n709 = while {
        tunnel: w1099 -> [w1111]
        tunnel: [w1111] -> w1100
        i -> [w1109]
        stop <- w1108 stop-if-true
        # "Wait until shooting finishes"
        n710 = Equal To 0?(x=w1109) -> (x = 0?=w1108:bool)
        n711 = Wait (ms)(milliseconds to wait=u32 300) -> ()  [unwired: 1 out]
      }
      n712 = while {
        tunnel: w1100 -> [w1153]
        tunnel: [w1153] -> w1101
        i -> [w1152]
        stop <- w1135 stop-if-true
        w1136 = TRUE  # ABS_Traj ?
        w1144 = TRUE  # EnableClosedLoop
        w1142 = FALSE  # Reverse
        w1146 = TRUE  # Follow Orientation
        n713 = Equal To 0?(x=w1152) -> (x = 0?=w1143:bool)
        n714 = call "SWERVE_DRIVE_GET_SPEED_DEMAND.vi"() -> ("Drv Rotation Orentation Dmd"=w1151:dbl)  [unwired: 8 in, 3 out]
        n715 = call "SWERVE_DRIVE_GET_GYRO.vi"() -> ("Gyro Heading Radians"=w1141:dbl)  [unwired: 11 in]
        n716 = Wait Until Next ms Multiple(millisecond multiple=u32 20 ("milliseconds to wait")) -> ()  [unwired: 1 out]
        n717 = call "SWERVE_TRAJECTORY_EXECUTE.vi"("EnableClosedLoop"=w1144, "ABS_Traj ?"=w1136, "Init"=w1143, "Reverse"=w1142, "Follow Orientation"=w1146, "Gyro Heading\nRAD"=w1141) -> ("AtReference"=w1137:bool, "OutputTRAJ_STATE"=w1138:T12, "Error and Corr"=w1139:T13, "Chassis Velocity Target"=w1145:T14, "Orientation Target"=w1140:dbl)  [unwired: 1 in]
        n718 = Select(t=w1141, s=w1146, f=w1151) -> (s? t:f=w1147:dbl)
        n719 = call "SWERVE_TRAJECTORY_SET_CLOSED_LOOP.vi"("AUTO_CLOSED_LOOP"=w1144) -> ()  [unwired: 11 in]
        n720 = call "SWERVE_TRAJECTORY_UPDATE_DIAG_INFO.vi"("AtReference"=w1137, "OutputTRAJ_STATE"=w1138, "Error and Corr"=w1139, "Orientation Target"=w1140) -> ()  [unwired: 8 in]
        n721 = Unbundle By Name(w1145) -> ("vX"=w1150:dbl, "vY"=w1149:dbl, "vOmega"=w1148:dbl)
        n722 = global read "SWERVE_TRAJECTORY_GLOBALS.vi" "Traj_Total_Time"() -> (w1133:dbl)
        n723 = Unbundle By Name(w1138) -> ("TimeSeconds"=w1134:dbl)
        n724 = call "SWERVE_DRIVE_SET_SPEED_DEMAND.vi"("Drv Rotation Orentation Dmd"=w1147, "Drv Angular Vel Dmd"=w1148, "Drv Y Vel Dmd"=w1149, "Drv X Vel Dmd"=w1150) -> ()  [unwired: 8 in]
        n725 = Equal?(x=w1134, y=w1133) -> (x = y?=w1135:bool)
        n726 = call-poly <vilib>:"NT Read Value.vi"("default value"=FALSE ("value"), "name"="Shooter/Limited") -> ("value"=w1131:bool)  [unwired: 7 in, 2 out]
        n727 = Select(t="Stop" ("default value"), s=w1131, f="FromIntake") -> (s? t:f=w1127:string)
        n728 = call-poly <vilib>:"NT Write Value.vi"("value"=FALSE, "name"="Shooter/Overwrite Angle") -> ()  [unwired: 9 in, 1 out]
        n729 = call-poly <vilib>:"NT Write Value.vi"("value"=w1127, "name"="Intake/Trigger Status") -> ()  [unwired: 9 in, 1 out]
      }
      n730 = while {
        tunnel: w1101 -> [w1123]
        tunnel: [w1123] -> w1098
        i -> [w1121]
        stop <- w1120 stop-if-true
        w1119 = 0.0 ("Drv X Vel Dmd")
        n731 = Not Equal To 0?(x=w1121) -> (x != 0?=w1120:bool)
        n732 = Wait (ms)(milliseconds to wait=u32 20) -> ()  [unwired: 1 out]
        n733 = call-poly <vilib>:"NT Write Value.vi"("value"="ToShooter" ("default value"), "name"="Intake/Trigger Status") -> ()  [unwired: 9 in, 1 out]
        n734 = call "SWERVE_DRIVE_MODULE_STATES_POSITIONS_FGV.vi"() -> ("out Current Module Positions"=w1115:T11[])  [unwired: 10 in, 1 out]
        n735 = call "SWERVE_DRIVE_GET_GYRO.vi"() -> ("Gyro Heading Radians"=w1117:dbl)  [unwired: 11 in]
        n736 = call "SWERVE_DRIVE_GET_GYRO.vi"() -> ("Gyro Heading Radians"=w1118:dbl)  [unwired: 11 in]
        n737 = call <vilib>:"Rotation2d_CreateAngle.vi"("Angle"=w1117) -> ("ROTATION"=w1116:T9)  [unwired: 10 in]
        n738 = call "SWERVE_DRIVE_SET_SPEED_DEMAND.vi"("Drv Rotation Orentation Dmd"=w1118, "Drv Angular Vel Dmd"=w1119, "Drv Y Vel Dmd"=w1119, "Drv X Vel Dmd"=w1119) -> ()  [unwired: 8 in]
        n739 = call "SWERVE_TRAJECTORY_BEGIN.vi"("gyroAngle"=w1116, "Module Positions"=w1115, "Trajectory File Name"="Path Demo.wpilib.csv") -> ()  [unwired: 9 in]
      }
      n740 = while {
        tunnel: w1098 -> [w1233]
        tunnel: [w1233] -> w1105
        i -> [w1231]
        stop <- w1230 stop-if-true
        # "Wait until shooting finishes"
        n741 = Equal To 0?(x=w1231) -> (x = 0?=w1230:bool)
        n742 = Wait (ms)(milliseconds to wait=u32 200) -> ()  [unwired: 1 out]
      }
      n743 = while {
        tunnel: w1105 -> [w1246]
        tunnel: [w1246] -> w1104
        i -> [w1244]
        stop <- w1243 stop-if-true
        w1240 = FALSE  # ABS Odo Initialize
        w1242 = 0.0 ("Drv X Vel Dmd")
        n744 = Not Equal To 0?(x=w1244) -> (x != 0?=w1243:bool)
        n745 = Wait (ms)(milliseconds to wait=u32 20) -> ()  [unwired: 1 out]
        n746 = call-poly <vilib>:"NT Write Value.vi"("value"="Intake Mode" ("default value"), "name"="Robot State") -> ()  [unwired: 9 in, 1 out]
        n747 = call "SWERVE_DRIVE_MODULE_STATES_POSITIONS_FGV.vi"() -> ("out Current Module Positions"=w1237:T11[])  [unwired: 10 in, 1 out]
        n748 = call "SWERVE_DRIVE_GET_GYRO.vi"() -> ("Gyro Heading Radians"=w1239:dbl)  [unwired: 11 in]
        n749 = call "SWERVE_DRIVE_GET_GYRO.vi"() -> ("Gyro Heading Radians"=w1241:dbl)  [unwired: 11 in]
        n750 = call <vilib>:"Rotation2d_CreateAngle.vi"("Angle"=w1239) -> ("ROTATION"=w1238:T9)  [unwired: 10 in]
        n751 = call "SWERVE_DRIVE_SET_SPEED_DEMAND.vi"("Drv Rotation Orentation Dmd"=w1241, "Drv Angular Vel Dmd"=w1242, "Drv Y Vel Dmd"=w1242, "Drv X Vel Dmd"=w1242) -> ()  [unwired: 8 in]
        n752 = call "SWERVE_TRAJECTORY_BEGIN.vi"("ABS Odo Initialize"=w1240, "gyroAngle"=w1238, "Module Positions"=w1237, "Trajectory File Name"="Route C1 B Path 2.path") -> ()  [unwired: 8 in]
      }
      n753 = while {
        tunnel: w1104 -> [w1209]
        tunnel: [w1209] -> w1103
        i -> [w1208]
        stop <- w1191 stop-if-true
        w1192 = TRUE  # ABS_Traj ?
        w1200 = TRUE  # EnableClosedLoop
        w1198 = FALSE  # Reverse
        w1202 = TRUE  # Follow Orientation
        # "During the second half of the path, switch to Shoot Mode but stop the trigger when limit switch pressed"
        n754 = Equal To 0?(x=w1208) -> (x = 0?=w1199:bool)
        n755 = call "SWERVE_DRIVE_GET_SPEED_DEMAND.vi"() -> ("Drv Rotation Orentation Dmd"=w1207:dbl)  [unwired: 8 in, 3 out]
        n756 = call "SWERVE_DRIVE_GET_GYRO.vi"() -> ("Gyro Heading Radians"=w1197:dbl)  [unwired: 11 in]
        n757 = Wait Until Next ms Multiple(millisecond multiple=u32 20 ("milliseconds to wait")) -> ()  [unwired: 1 out]
        n758 = call "SWERVE_TRAJECTORY_EXECUTE.vi"("EnableClosedLoop"=w1200, "ABS_Traj ?"=w1192, "Init"=w1199, "Reverse"=w1198, "Follow Orientation"=w1202, "Gyro Heading\nRAD"=w1197) -> ("AtReference"=w1193:bool, "OutputTRAJ_STATE"=w1194:T12, "Error and Corr"=w1195:T13, "Chassis Velocity Target"=w1201:T14, "Orientation Target"=w1196:dbl)  [unwired: 1 in]
        n759 = Select(t=w1197, s=w1202, f=w1207) -> (s? t:f=w1203:dbl)
        n760 = call "SWERVE_TRAJECTORY_SET_CLOSED_LOOP.vi"("AUTO_CLOSED_LOOP"=w1200) -> ()  [unwired: 11 in]
        n761 = call "SWERVE_TRAJECTORY_UPDATE_DIAG_INFO.vi"("AtReference"=w1193, "OutputTRAJ_STATE"=w1194, "Error and Corr"=w1195, "Orientation Target"=w1196) -> ()  [unwired: 8 in]
        n762 = Unbundle By Name(w1201) -> ("vX"=w1206:dbl, "vY"=w1205:dbl, "vOmega"=w1204:dbl)
        n763 = global read "SWERVE_TRAJECTORY_GLOBALS.vi" "Traj_Total_Time"() -> (w1183:dbl)
        n764 = Unbundle By Name(w1194) -> ("TimeSeconds"=w1184:dbl)
        n765 = call "SWERVE_DRIVE_SET_SPEED_DEMAND.vi"("Drv Rotation Orentation Dmd"=w1203, "Drv Angular Vel Dmd"=w1204, "Drv Y Vel Dmd"=w1205, "Drv X Vel Dmd"=w1206) -> ()  [unwired: 8 in]
        n766 = Equal?(x=w1184, y=w1183) -> (x = y?=w1191:bool)
        n767 = Divide(x=w1184, y=w1183) -> (x/y=w1187:dbl)
        n768 = Greater?(x=w1187, y=0.6) -> (0:w1185:bool)
        n769 = call-poly <vilib>:"NT Read Value.vi"("default value"=FALSE ("value"), "name"="Shooter/Limited") -> ("value"=w1189:bool)  [unwired: 7 in, 2 out]
        n770 = case shown="True" w1189 {
          tunnel: w1185 -> [_ w1213]
          frame False {
            n771 = call-poly <vilib>:"NT Write Value.vi"("value"="Intake Mode" ("default value"), "name"="Robot State") -> ()  [unwired: 9 in, 1 out]
          }
          frame True {
            n772 = case shown="True" w1213 {
              frame False {
              }
              frame True {
                n773 = call-poly <vilib>:"NT Write Value.vi"("value"="Shoot Mode" ("default value"), "name"="Robot State") -> ()  [unwired: 9 in, 1 out]
              }
            }
            n774 = call-poly <vilib>:"NT Write Value.vi"("value"="Stop" ("default value"), "name"="Intake/Trigger Status") -> ()  [unwired: 9 in, 1 out]
          }
        }
      }
      n775 = while {
        tunnel: w1103 -> [w1229]
        tunnel: [w1229] -> w1102
        i -> [w1227]
        stop <- w1226 stop-if-true
        w1225 = 0.0 ("Drv X Vel Dmd")
        n776 = Not Equal To 0?(x=w1227) -> (x != 0?=w1226:bool)
        n777 = Wait (ms)(milliseconds to wait=u32 20) -> ()  [unwired: 1 out]
        n778 = call-poly <vilib>:"NT Write Value.vi"("value"="Shoot Mode" ("default value"), "name"="Robot State") -> ()  [unwired: 9 in, 1 out]
        n779 = call "SWERVE_DRIVE_MODULE_STATES_POSITIONS_FGV.vi"() -> ("out Current Module Positions"=w1221:T11[])  [unwired: 10 in, 1 out]
        n780 = call "SWERVE_DRIVE_GET_GYRO.vi"() -> ("Gyro Heading Radians"=w1223:dbl)  [unwired: 11 in]
        n781 = call "SWERVE_DRIVE_GET_GYRO.vi"() -> ("Gyro Heading Radians"=w1224:dbl)  [unwired: 11 in]
        n782 = call <vilib>:"Rotation2d_CreateAngle.vi"("Angle"=w1223) -> ("ROTATION"=w1222:T9)  [unwired: 10 in]
        n783 = call "SWERVE_DRIVE_SET_SPEED_DEMAND.vi"("Drv Rotation Orentation Dmd"=w1224, "Drv Angular Vel Dmd"=w1225, "Drv Y Vel Dmd"=w1225, "Drv X Vel Dmd"=w1225) -> ()  [unwired: 8 in]
        n784 = call "SWERVE_TRAJECTORY_BEGIN.vi"("gyroAngle"=w1222, "Module Positions"=w1221, "Trajectory File Name"="Path Demo.wpilib.csv") -> ()  [unwired: 9 in]
      }
      n785 = while {
        tunnel: w1102 -> [w1178]
        tunnel: [w1178] -> _
        i -> [w1159]
        stop <- FALSE stop-if-true
        w1166 = 0.0 ("Drv X Vel Dmd")
        n786 = Greater?(x=w1159, y=40) -> (0:w1155:bool)
        n787 = call-poly <vilib>:"NT Read Value.vi"("name"="/limelight-shooter/tv") -> ("value"=w1169:dbl)  [unwired: 8 in, 2 out]
        n788 = call-poly <vilib>:"NT Read Value.vi"("name"="Shooter/Corrected Theta") -> ("value"=w1163:dbl)  [unwired: 8 in, 2 out]
        n789 = call-poly <vilib>:"NT Read Value.vi"("name"="Shooter/Angle_Deg Act") -> ("value"=w1175:dbl)  [unwired: 8 in, 2 out]
        n790 = call-poly <vilib>:"NT Read Value.vi"("name"="Shooter/Angle_Deg Dmd") -> ("value"=w1174:dbl)  [unwired: 8 in, 2 out]
        n791 = Not Equal To 0?(x=w1169) -> (x != 0?=w1168:bool)
        n792 = call "SWERVE_DRIVE_GET_GYRO.vi"() -> ("Gyro Heading Radians"=w1164:dbl)  [unwired: 11 in]
        n793 = Select(t=w1163, s=w1168, f=w1164) -> (s? t:f=w1167:dbl)
        n794 = call <vilib>:"Util_ApproxEquals.vi"("Tolerance"=3.5, "Value 2"=w1174, "Value 1"=w1175) -> ("ApproxEquals"=w1165:bool)  [unwired: 8 in]
        n795 = call <vilib>:"Util_ApproxEquals.vi"("Tolerance"=0.1, "Value 2"=w1164, "Value 1"=w1163) -> ("ApproxEquals"=w1161:bool)  [unwired: 8 in]
        n796 = And(x=w1165, y=w1161) -> (x .and. y?=w1157:bool)
        n797 = Or(x=w1157, y=w1155) -> (x .or. y?=w1156:bool)
        n798 = case shown="True" w1156 {
          frame False {
            n799 = call-poly <vilib>:"NT Write Value.vi"("value"="Stop" ("default value"), "name"="Intake/Trigger Status") -> ()  [unwired: 9 in, 1 out]
          }
          frame True {
            n800 = call-poly <vilib>:"NT Write Value.vi"("value"="ToShooter" ("default value"), "name"="Intake/Trigger Status") -> ()  [unwired: 9 in, 1 out]
          }
        }
        n801 = call "SWERVE_DRIVE_SET_SPEED_DEMAND.vi"("Drv Rotation Orentation Dmd"=w1167, "Drv Angular Vel Dmd"=w1166, "Drv Y Vel Dmd"=w1166, "Drv X Vel Dmd"=w1166) -> ()  [unwired: 8 in]
        n802 = Wait (ms)(milliseconds to wait=u32 20) -> ()  [unwired: 1 out]
      }
    }
    frame "Route C1 Red" {
      w1297 = errorcluster {"status"=FALSE, "code"=0, "source"=""}  # Start Error Flow
      n803 = while {
        tunnel: w1297 -> [w1481]
        tunnel: [w1481] -> w1289
        i -> [w1479]
        stop <- w1478 stop-if-true
        w1475 = TRUE  # ABS Odo Initialize
        w1477 = 0.0 ("Drv X Vel Dmd")
        n804 = Not Equal To 0?(x=w1479) -> (x != 0?=w1478:bool)
        n805 = Wait (ms)(milliseconds to wait=u32 20) -> ()  [unwired: 1 out]
        n806 = call-poly <vilib>:"NT Read Value.vi"("default value"="Path_Testing_1.path" ("Trajectory File Name"), "name"="Initial Path") -> ("value"=w1472:string)  [unwired: 7 in, 2 out]
        n807 = call "SWERVE_DRIVE_MODULE_STATES_POSITIONS_FGV.vi"() -> ("out Current Module Positions"=w1469:T11[])  [unwired: 10 in, 1 out]
        n808 = call "SWERVE_DRIVE_GET_GYRO.vi"() -> ("Gyro Heading Radians"=w1471:dbl)  [unwired: 11 in]
        n809 = call "SWERVE_DRIVE_GET_GYRO.vi"() -> ("Gyro Heading Radians"=w1476:dbl)  [unwired: 11 in]
        n810 = call <vilib>:"Rotation2d_CreateAngle.vi"("Angle"=w1471) -> ("ROTATION"=w1470:T9)  [unwired: 10 in]
        n811 = call "SWERVE_DRIVE_SET_SPEED_DEMAND.vi"("Drv Rotation Orentation Dmd"=w1476, "Drv Angular Vel Dmd"=w1477, "Drv Y Vel Dmd"=w1477, "Drv X Vel Dmd"=w1477) -> ()  [unwired: 8 in]
        n812 = call "SWERVE_TRAJECTORY_BEGIN.vi"("ABS Odo Initialize"=w1475, "gyroAngle"=w1470, "Module Positions"=w1469, "Trajectory File Name"=w1472) -> ()  [unwired: 8 in]
      }
      n813 = while {
        tunnel: w1289 -> [w1321]
        tunnel: [w1321] -> w1288
        stop <- w1302 stop-if-true
        # "Shoot Preload"
        n814 = Wait (ms)(milliseconds to wait=u32 20) -> ()  [unwired: 1 out]
        n815 = call-poly <vilib>:"NT Read Value.vi"("default value"=0.0, "name"="Shooter/Speed_RPM Act") -> ("value"=w1316:dbl)  [unwired: 7 in, 2 out]
        n816 = call-poly <vilib>:"NT Read Value.vi"("name"="Shooter/Angle_Deg Act") -> ("value"=w1306:dbl)  [unwired: 8 in, 2 out]
        n817 = call-poly <vilib>:"NT Read Value.vi"("name"="Shooter/Angle_Deg Dmd") -> ("value"=w1305:dbl)  [unwired: 8 in, 2 out]
        n818 = call-poly <vilib>:"NT Write Value.vi"("value"="Shoot Mode" ("default value"), "name"="Robot State") -> ()  [unwired: 9 in, 1 out]
        n819 = call-poly <vilib>:"NT Write Value.vi"("value"=FALSE, "name"="Shooter/Overwrite RPM") -> ()  [unwired: 9 in, 1 out]
        n820 = Greater?(x=w1316, y=2000.0) -> (0:w1304:bool)
        n821 = call <vilib>:"Util_ApproxEquals.vi"("Tolerance"=3.0, "Value 2"=w1305, "Value 1"=w1306) -> ("ApproxEquals"=w1303:bool)  [unwired: 8 in]
        n822 = And(x=w1304, y=w1303) -> (x .and. y?=w1302:bool)
        n823 = case shown="True" w1302 {
          frame False {
            n824 = call-poly <vilib>:"NT Write Value.vi"("value"="Stop" ("default value"), "name"="Intake/Trigger Status") -> ()  [unwired: 9 in, 1 out]
          }
          frame True {
            n825 = call-poly <vilib>:"NT Write Value.vi"("value"="ToShooter" ("default value"), "name"="Intake/Trigger Status") -> ()  [unwired: 9 in, 1 out]
          }
        }
        n826 = call-poly <vilib>:"NT Write Value.vi"("value"=TRUE, "name"="Shooter/Overwrite Angle") -> ()  [unwired: 9 in, 1 out]
        n827 = call-poly <vilib>:"NT Write Value.vi"("value"=53.0, "name"="Shooter/Angle_Deg Dmd") -> ()  [unwired: 9 in, 1 out]
        n828 = call-poly <vilib>:"NT Write Value.vi"("value"=2500.0, "name"="Shooter/RPM Dmd") -> ()  [unwired: 9 in, 1 out]
      }
      n829 = while {
        tunnel: [w1367] -> w1293
        tunnel: w1288 -> [w1367]
        i -> [w1369]
        stop <- w1368 stop-if-true
        # "Wait until shooting finishes"
        n830 = Equal To 0?(x=w1369) -> (x = 0?=w1368:bool)
        n831 = Wait (ms)(milliseconds to wait=u32 300) -> ()  [unwired: 1 out]
      }
      n832 = while {
        tunnel: w1293 -> [w1412]
        tunnel: [w1412] -> w1294
        i -> [w1411]
        stop <- w1394 stop-if-true
        w1395 = TRUE  # ABS_Traj ?
        w1403 = TRUE  # EnableClosedLoop
        w1401 = FALSE  # Reverse
        w1405 = TRUE  # Follow Orientation
        n833 = Equal To 0?(x=w1411) -> (x = 0?=w1402:bool)
        n834 = call "SWERVE_DRIVE_GET_SPEED_DEMAND.vi"() -> ("Drv Rotation Orentation Dmd"=w1410:dbl)  [unwired: 8 in, 3 out]
        n835 = call "SWERVE_DRIVE_GET_GYRO.vi"() -> ("Gyro Heading Radians"=w1400:dbl)  [unwired: 11 in]
        n836 = Wait Until Next ms Multiple(millisecond multiple=u32 20 ("milliseconds to wait")) -> ()  [unwired: 1 out]
        n837 = call "SWERVE_TRAJECTORY_EXECUTE.vi"("EnableClosedLoop"=w1403, "ABS_Traj ?"=w1395, "Init"=w1402, "Reverse"=w1401, "Follow Orientation"=w1405, "Gyro Heading\nRAD"=w1400) -> ("AtReference"=w1396:bool, "OutputTRAJ_STATE"=w1397:T12, "Error and Corr"=w1398:T13, "Chassis Velocity Target"=w1404:T14, "Orientation Target"=w1399:dbl)  [unwired: 1 in]
        n838 = Select(t=w1400, s=w1405, f=w1410) -> (s? t:f=w1406:dbl)
        n839 = call "SWERVE_TRAJECTORY_SET_CLOSED_LOOP.vi"("AUTO_CLOSED_LOOP"=w1403) -> ()  [unwired: 11 in]
        n840 = call "SWERVE_TRAJECTORY_UPDATE_DIAG_INFO.vi"("AtReference"=w1396, "OutputTRAJ_STATE"=w1397, "Error and Corr"=w1398, "Orientation Target"=w1399) -> ()  [unwired: 8 in]
        n841 = Unbundle By Name(w1404) -> ("vX"=w1409:dbl, "vY"=w1408:dbl, "vOmega"=w1407:dbl)
        n842 = global read "SWERVE_TRAJECTORY_GLOBALS.vi" "Traj_Total_Time"() -> (w1392:dbl)
        n843 = Unbundle By Name(w1397) -> ("TimeSeconds"=w1393:dbl)
        n844 = call "SWERVE_DRIVE_SET_SPEED_DEMAND.vi"("Drv Rotation Orentation Dmd"=w1406, "Drv Angular Vel Dmd"=w1407, "Drv Y Vel Dmd"=w1408, "Drv X Vel Dmd"=w1409) -> ()  [unwired: 8 in]
        n845 = Equal?(x=w1393, y=w1392) -> (x = y?=w1394:bool)
        n846 = call-poly <vilib>:"NT Read Value.vi"("default value"=FALSE ("value"), "name"="Shooter/Limited") -> ("value"=w1390:bool)  [unwired: 7 in, 2 out]
        n847 = Select(t="Stop" ("default value"), s=w1390, f="FromIntake") -> (s? t:f=w1386:string)
        n848 = call-poly <vilib>:"NT Write Value.vi"("value"=w1386, "name"="Intake/Trigger Status") -> ()  [unwired: 9 in, 1 out]
        n849 = call-poly <vilib>:"NT Write Value.vi"("value"=FALSE, "name"="Shooter/Overwrite Angle") -> ()  [unwired: 9 in, 1 out]
      }
      n850 = while {
        tunnel: w1294 -> [w1382]
        tunnel: [w1382] -> w1292
        i -> [w1380]
        stop <- w1379 stop-if-true
        w1378 = 0.0 ("Drv X Vel Dmd")
        n851 = Not Equal To 0?(x=w1380) -> (x != 0?=w1379:bool)
        n852 = Wait (ms)(milliseconds to wait=u32 20) -> ()  [unwired: 1 out]
        n853 = call-poly <vilib>:"NT Write Value.vi"("value"="ToShooter" ("default value"), "name"="Intake/Trigger Status") -> ()  [unwired: 9 in, 1 out]
        n854 = call "SWERVE_DRIVE_MODULE_STATES_POSITIONS_FGV.vi"() -> ("out Current Module Positions"=w1374:T11[])  [unwired: 10 in, 1 out]
        n855 = call "SWERVE_DRIVE_GET_GYRO.vi"() -> ("Gyro Heading Radians"=w1376:dbl)  [unwired: 11 in]
        n856 = call "SWERVE_DRIVE_GET_GYRO.vi"() -> ("Gyro Heading Radians"=w1377:dbl)  [unwired: 11 in]
        n857 = call <vilib>:"Rotation2d_CreateAngle.vi"("Angle"=w1376) -> ("ROTATION"=w1375:T9)  [unwired: 10 in]
        n858 = call "SWERVE_DRIVE_SET_SPEED_DEMAND.vi"("Drv Rotation Orentation Dmd"=w1377, "Drv Angular Vel Dmd"=w1378, "Drv Y Vel Dmd"=w1378, "Drv X Vel Dmd"=w1378) -> ()  [unwired: 8 in]
        n859 = call "SWERVE_TRAJECTORY_BEGIN.vi"("gyroAngle"=w1375, "Module Positions"=w1374, "Trajectory File Name"="Path Demo.wpilib.csv") -> ()  [unwired: 9 in]
      }
      n860 = while {
        tunnel: w1292 -> [w1455]
        tunnel: [w1455] -> w1296
        i -> [w1453]
        stop <- w1452 stop-if-true
        # "Wait until shooting finishes"
        n861 = Equal To 0?(x=w1453) -> (x = 0?=w1452:bool)
        n862 = Wait (ms)(milliseconds to wait=u32 200) -> ()  [unwired: 1 out]
      }
      n863 = while {
        tunnel: w1296 -> [w1468]
        tunnel: [w1468] -> w1291
        i -> [w1466]
        stop <- w1465 stop-if-true
        w1462 = FALSE  # ABS Odo Initialize
        w1464 = 0.0 ("Drv X Vel Dmd")
        n864 = Not Equal To 0?(x=w1466) -> (x != 0?=w1465:bool)
        n865 = Wait (ms)(milliseconds to wait=u32 20) -> ()  [unwired: 1 out]
        n866 = call-poly <vilib>:"NT Write Value.vi"("value"="Intake Mode" ("default value"), "name"="Robot State") -> ()  [unwired: 9 in, 1 out]
        n867 = call "SWERVE_DRIVE_MODULE_STATES_POSITIONS_FGV.vi"() -> ("out Current Module Positions"=w1459:T11[])  [unwired: 10 in, 1 out]
        n868 = call "SWERVE_DRIVE_GET_GYRO.vi"() -> ("Gyro Heading Radians"=w1461:dbl)  [unwired: 11 in]
        n869 = call "SWERVE_DRIVE_GET_GYRO.vi"() -> ("Gyro Heading Radians"=w1463:dbl)  [unwired: 11 in]
        n870 = call <vilib>:"Rotation2d_CreateAngle.vi"("Angle"=w1461) -> ("ROTATION"=w1460:T9)  [unwired: 10 in]
        n871 = call "SWERVE_DRIVE_SET_SPEED_DEMAND.vi"("Drv Rotation Orentation Dmd"=w1463, "Drv Angular Vel Dmd"=w1464, "Drv Y Vel Dmd"=w1464, "Drv X Vel Dmd"=w1464) -> ()  [unwired: 8 in]
        n872 = call "SWERVE_TRAJECTORY_BEGIN.vi"("ABS Odo Initialize"=w1462, "gyroAngle"=w1460, "Module Positions"=w1459, "Trajectory File Name"="Route C1 R Path 2.path") -> ()  [unwired: 8 in]
      }
      n873 = while {
        tunnel: w1291 -> [w1334]
        tunnel: [w1334] -> w1290
        i -> [w1352]
        stop <- w1335 stop-if-true
        w1336 = TRUE  # ABS_Traj ?
        w1344 = TRUE  # EnableClosedLoop
        w1342 = FALSE  # Reverse
        w1346 = TRUE  # Follow Orientation
        # "To Shoot Mode when limit switch pressed"
        n874 = Equal To 0?(x=w1352) -> (x = 0?=w1343:bool)
        n875 = call "SWERVE_DRIVE_GET_SPEED_DEMAND.vi"() -> ("Drv Rotation Orentation Dmd"=w1351:dbl)  [unwired: 8 in, 3 out]
        n876 = call "SWERVE_DRIVE_GET_GYRO.vi"() -> ("Gyro Heading Radians"=w1341:dbl)  [unwired: 11 in]
        n877 = Wait Until Next ms Multiple(millisecond multiple=u32 20 ("milliseconds to wait")) -> ()  [unwired: 1 out]
        n878 = call "SWERVE_TRAJECTORY_EXECUTE.vi"("EnableClosedLoop"=w1344, "ABS_Traj ?"=w1336, "Init"=w1343, "Reverse"=w1342, "Follow Orientation"=w1346, "Gyro Heading\nRAD"=w1341) -> ("AtReference"=w1337:bool, "OutputTRAJ_STATE"=w1338:T12, "Error and Corr"=w1339:T13, "Chassis Velocity Target"=w1345:T14, "Orientation Target"=w1340:dbl)  [unwired: 1 in]
        n879 = Select(t=w1341, s=w1346, f=w1351) -> (s? t:f=w1347:dbl)
        n880 = call "SWERVE_TRAJECTORY_SET_CLOSED_LOOP.vi"("AUTO_CLOSED_LOOP"=w1344) -> ()  [unwired: 11 in]
        n881 = call "SWERVE_TRAJECTORY_UPDATE_DIAG_INFO.vi"("AtReference"=w1337, "OutputTRAJ_STATE"=w1338, "Error and Corr"=w1339, "Orientation Target"=w1340) -> ()  [unwired: 8 in]
        n882 = Unbundle By Name(w1345) -> ("vX"=w1350:dbl, "vY"=w1349:dbl, "vOmega"=w1348:dbl)
        n883 = global read "SWERVE_TRAJECTORY_GLOBALS.vi" "Traj_Total_Time"() -> (w1326:dbl)
        n884 = Unbundle By Name(w1338) -> ("TimeSeconds"=w1327:dbl)
        n885 = call "SWERVE_DRIVE_SET_SPEED_DEMAND.vi"("Drv Rotation Orentation Dmd"=w1347, "Drv Angular Vel Dmd"=w1348, "Drv Y Vel Dmd"=w1349, "Drv X Vel Dmd"=w1350) -> ()  [unwired: 8 in]
        n886 = Equal?(x=w1327, y=w1326) -> (x = y?=w1335:bool)
        n887 = Divide(x=w1327, y=w1326) -> (x/y=w1330:dbl)
        n888 = Greater?(x=w1330, y=0.6) -> (0:w1328:bool)
        n889 = call-poly <vilib>:"NT Read Value.vi"("default value"=FALSE ("value"), "name"="Shooter/Limited") -> ("value"=w1332:bool)  [unwired: 7 in, 2 out]
        n890 = case shown="True" w1332 {
          tunnel: w1328 -> [_ w1356]
          frame False {
            n891 = call-poly <vilib>:"NT Write Value.vi"("value"="Intake Mode" ("default value"), "name"="Robot State") -> ()  [unwired: 9 in, 1 out]
          }
          frame True {
            n892 = case shown="True" w1356 {
              frame False {
                n893 = call-poly <vilib>:"NT Write Value.vi"("value"=TRUE, "name"="Shooter/Overwrite Angle") -> ()  [unwired: 9 in, 1 out]
                n894 = call-poly <vilib>:"NT Write Value.vi"("value"=53.0, "name"="Shooter/Angle_Deg Dmd") -> ()  [unwired: 9 in, 1 out]
              }
              frame True {
                n895 = call-poly <vilib>:"NT Write Value.vi"("value"=FALSE, "name"="Shooter/Overwrite Angle") -> ()  [unwired: 9 in, 1 out]
              }
            }
            n896 = call-poly <vilib>:"NT Write Value.vi"("value"="Shoot Mode" ("default value"), "name"="Robot State") -> ()  [unwired: 9 in, 1 out]
            n897 = call-poly <vilib>:"NT Write Value.vi"("value"="Stop" ("default value"), "name"="Intake/Trigger Status") -> ()  [unwired: 9 in, 1 out]
          }
        }
      }
      n898 = while {
        tunnel: w1290 -> [w1451]
        tunnel: [w1451] -> w1295
        i -> [w1449]
        stop <- w1448 stop-if-true
        w1447 = 0.0 ("Drv X Vel Dmd")
        n899 = Not Equal To 0?(x=w1449) -> (x != 0?=w1448:bool)
        n900 = Wait (ms)(milliseconds to wait=u32 20) -> ()  [unwired: 1 out]
        n901 = call "SWERVE_DRIVE_MODULE_STATES_POSITIONS_FGV.vi"() -> ("out Current Module Positions"=w1443:T11[])  [unwired: 10 in, 1 out]
        n902 = call "SWERVE_DRIVE_GET_GYRO.vi"() -> ("Gyro Heading Radians"=w1445:dbl)  [unwired: 11 in]
        n903 = call "SWERVE_DRIVE_GET_GYRO.vi"() -> ("Gyro Heading Radians"=w1446:dbl)  [unwired: 11 in]
        n904 = call <vilib>:"Rotation2d_CreateAngle.vi"("Angle"=w1445) -> ("ROTATION"=w1444:T9)  [unwired: 10 in]
        n905 = call "SWERVE_DRIVE_SET_SPEED_DEMAND.vi"("Drv Rotation Orentation Dmd"=w1446, "Drv Angular Vel Dmd"=w1447, "Drv Y Vel Dmd"=w1447, "Drv X Vel Dmd"=w1447) -> ()  [unwired: 8 in]
        n906 = call "SWERVE_TRAJECTORY_BEGIN.vi"("gyroAngle"=w1444, "Module Positions"=w1443, "Trajectory File Name"="Path Demo.wpilib.csv") -> ()  [unwired: 9 in]
      }
      n907 = while {
        tunnel: w1295 -> [w1437]
        tunnel: [w1437] -> _
        i -> [w1418]
        stop <- FALSE stop-if-true
        w1425 = 0.0 ("Drv X Vel Dmd")
        n908 = Greater?(x=w1418, y=40) -> (0:w1414:bool)
        n909 = call-poly <vilib>:"NT Read Value.vi"("name"="/limelight-shooter/tv") -> ("value"=w1428:dbl)  [unwired: 8 in, 2 out]
        n910 = call-poly <vilib>:"NT Read Value.vi"("name"="Shooter/Corrected Theta") -> ("value"=w1422:dbl)  [unwired: 8 in, 2 out]
        n911 = call-poly <vilib>:"NT Read Value.vi"("name"="Shooter/Angle_Deg Act") -> ("value"=w1434:dbl)  [unwired: 8 in, 2 out]
        n912 = call-poly <vilib>:"NT Read Value.vi"("name"="Shooter/Angle_Deg Dmd") -> ("value"=w1433:dbl)  [unwired: 8 in, 2 out]
        n913 = Not Equal To 0?(x=w1428) -> (x != 0?=w1427:bool)
        n914 = call "SWERVE_DRIVE_GET_GYRO.vi"() -> ("Gyro Heading Radians"=w1423:dbl)  [unwired: 11 in]
        n915 = Select(t=w1422, s=w1427, f=w1423) -> (s? t:f=w1426:dbl)
        n916 = call <vilib>:"Util_ApproxEquals.vi"("Tolerance"=3.5, "Value 2"=w1433, "Value 1"=w1434) -> ("ApproxEquals"=w1424:bool)  [unwired: 8 in]
        n917 = call <vilib>:"Util_ApproxEquals.vi"("Tolerance"=0.1, "Value 2"=w1423, "Value 1"=w1422) -> ("ApproxEquals"=w1420:bool)  [unwired: 8 in]
        n918 = And(x=w1424, y=w1420) -> (x .and. y?=w1416:bool)
        n919 = Or(x=w1416, y=w1414) -> (x .or. y?=w1415:bool)
        n920 = case shown="True" w1415 {
          frame False {
            n921 = call-poly <vilib>:"NT Write Value.vi"("value"="Stop" ("default value"), "name"="Intake/Trigger Status") -> ()  [unwired: 9 in, 1 out]
          }
          frame True {
            n922 = call-poly <vilib>:"NT Write Value.vi"("value"="ToShooter" ("default value"), "name"="Intake/Trigger Status") -> ()  [unwired: 9 in, 1 out]
          }
        }
        n923 = call "SWERVE_DRIVE_SET_SPEED_DEMAND.vi"("Drv Rotation Orentation Dmd"=w1426, "Drv Angular Vel Dmd"=w1425, "Drv Y Vel Dmd"=w1425, "Drv X Vel Dmd"=w1425) -> ()  [unwired: 8 in]
        n924 = Wait (ms)(milliseconds to wait=u32 20) -> ()  [unwired: 1 out]
      }
    }
    frame "Route C2 Blue" {
      w1487 = errorcluster {"status"=FALSE, "code"=0, "source"=""}  # Start Error Flow
      n925 = while {
        tunnel: w1487 -> [w1706]
        tunnel: [w1706] -> w1483
        i -> [w1704]
        stop <- w1703 stop-if-true
        w1700 = TRUE  # ABS Odo Initialize
        w1702 = 0.0 ("Drv X Vel Dmd")
        n926 = Not Equal To 0?(x=w1704) -> (x != 0?=w1703:bool)
        n927 = Wait (ms)(milliseconds to wait=u32 20) -> ()  [unwired: 1 out]
        n928 = call-poly <vilib>:"NT Read Value.vi"("default value"="Path_Testing_1.path" ("Trajectory File Name"), "name"="Initial Path") -> ("value"=w1697:string)  [unwired: 7 in, 2 out]
        n929 = call "SWERVE_DRIVE_MODULE_STATES_POSITIONS_FGV.vi"() -> ("out Current Module Positions"=w1694:T11[])  [unwired: 10 in, 1 out]
        n930 = call "SWERVE_DRIVE_GET_GYRO.vi"() -> ("Gyro Heading Radians"=w1696:dbl)  [unwired: 11 in]
        n931 = call "SWERVE_DRIVE_GET_GYRO.vi"() -> ("Gyro Heading Radians"=w1701:dbl)  [unwired: 11 in]
        n932 = call <vilib>:"Rotation2d_CreateAngle.vi"("Angle"=w1696) -> ("ROTATION"=w1695:T9)  [unwired: 10 in]
        n933 = call "SWERVE_DRIVE_SET_SPEED_DEMAND.vi"("Drv Rotation Orentation Dmd"=w1701, "Drv Angular Vel Dmd"=w1702, "Drv Y Vel Dmd"=w1702, "Drv X Vel Dmd"=w1702) -> ()  [unwired: 8 in]
        n934 = call "SWERVE_TRAJECTORY_BEGIN.vi"("ABS Odo Initialize"=w1700, "gyroAngle"=w1695, "Module Positions"=w1694, "Trajectory File Name"=w1697) -> ()  [unwired: 8 in]
      }
      n935 = while {
        tunnel: w1483 -> [w1507]
        tunnel: [w1507] -> w1482
        stop <- w1488 stop-if-true
        # "Shoot Preload"
        n936 = Wait (ms)(milliseconds to wait=u32 20) -> ()  [unwired: 1 out]
        n937 = call-poly <vilib>:"NT Read Value.vi"("default value"=0.0, "name"="Shooter/Speed_RPM Act") -> ("value"=w1502:dbl)  [unwired: 7 in, 2 out]
        n938 = call-poly <vilib>:"NT Read Value.vi"("name"="Shooter/Angle_Deg Act") -> ("value"=w1492:dbl)  [unwired: 8 in, 2 out]
        n939 = call-poly <vilib>:"NT Read Value.vi"("name"="Shooter/Angle_Deg Dmd") -> ("value"=w1491:dbl)  [unwired: 8 in, 2 out]
        n940 = call-poly <vilib>:"NT Write Value.vi"("value"="Shoot Mode" ("default value"), "name"="Robot State") -> ()  [unwired: 9 in, 1 out]
        n941 = Greater?(x=w1502, y=2000.0) -> (0:w1490:bool)
        n942 = call <vilib>:"Util_ApproxEquals.vi"("Tolerance"=2.0, "Value 2"=w1491, "Value 1"=w1492) -> ("ApproxEquals"=w1489:bool)  [unwired: 8 in]
        n943 = And(x=w1490, y=w1489) -> (x .and. y?=w1488:bool)
        n944 = case shown="True" w1488 {
          frame False {
            n945 = call-poly <vilib>:"NT Write Value.vi"("value"="Stop" ("default value"), "name"="Intake/Trigger Status") -> ()  [unwired: 9 in, 1 out]
          }
          frame True {
            n946 = call-poly <vilib>:"NT Write Value.vi"("value"="ToShooter" ("default value"), "name"="Intake/Trigger Status") -> ()  [unwired: 9 in, 1 out]
          }
        }
        n947 = call-poly <vilib>:"NT Write Value.vi"("value"=TRUE, "name"="Shooter/Overwrite Angle") -> ()  [unwired: 9 in, 1 out]
        n948 = call-poly <vilib>:"NT Write Value.vi"("value"=53.0, "name"="Shooter/Angle_Deg Dmd") -> ()  [unwired: 9 in, 1 out]
      }
      n949 = while {
        tunnel: w1482 -> [w1638]
        tunnel: [w1638] -> w1485
        i -> [w1636]
        stop <- w1635 stop-if-true
        # "Wait until shooting finishes"
        n950 = Equal To 0?(x=w1636) -> (x = 0?=w1635:bool)
        n951 = Wait (ms)(milliseconds to wait=u32 300) -> ()  [unwired: 1 out]
      }
      n952 = while {
        tunnel: w1485 -> [w1653]
        tunnel: [w1653] -> w1486
        i -> [w1679]
        stop <- w1662 stop-if-true
        w1663 = TRUE  # ABS_Traj ?
        w1671 = TRUE  # EnableClosedLoop
        w1669 = FALSE  # Reverse
        w1673 = TRUE  # Follow Orientation
        n953 = Equal To 0?(x=w1679) -> (x = 0?=w1670:bool)
        n954 = call "SWERVE_DRIVE_GET_SPEED_DEMAND.vi"() -> ("Drv Rotation Orentation Dmd"=w1678:dbl)  [unwired: 8 in, 3 out]
        n955 = call "SWERVE_DRIVE_GET_GYRO.vi"() -> ("Gyro Heading Radians"=w1668:dbl)  [unwired: 11 in]
        n956 = Wait Until Next ms Multiple(millisecond multiple=u32 20 ("milliseconds to wait")) -> ()  [unwired: 1 out]
        n957 = call "SWERVE_TRAJECTORY_EXECUTE.vi"("EnableClosedLoop"=w1671, "ABS_Traj ?"=w1663, "Init"=w1670, "Reverse"=w1669, "Follow Orientation"=w1673, "Gyro Heading\nRAD"=w1668) -> ("AtReference"=w1664:bool, "OutputTRAJ_STATE"=w1665:T12, "Error and Corr"=w1666:T13, "Chassis Velocity Target"=w1672:T14, "Orientation Target"=w1667:dbl)  [unwired: 1 in]
        n958 = Select(t=w1668, s=w1673, f=w1678) -> (s? t:f=w1674:dbl)
        n959 = call "SWERVE_TRAJECTORY_SET_CLOSED_LOOP.vi"("AUTO_CLOSED_LOOP"=w1671) -> ()  [unwired: 11 in]
        n960 = call "SWERVE_TRAJECTORY_UPDATE_DIAG_INFO.vi"("AtReference"=w1664, "OutputTRAJ_STATE"=w1665, "Error and Corr"=w1666, "Orientation Target"=w1667) -> ()  [unwired: 8 in]
        n961 = Unbundle By Name(w1672) -> ("vX"=w1677:dbl, "vY"=w1676:dbl, "vOmega"=w1675:dbl)
        n962 = global read "SWERVE_TRAJECTORY_GLOBALS.vi" "Traj_Total_Time"() -> (w1656:dbl)
        n963 = Unbundle By Name(w1665) -> ("TimeSeconds"=w1657:dbl)
        n964 = call "SWERVE_DRIVE_SET_SPEED_DEMAND.vi"("Drv Rotation Orentation Dmd"=w1674, "Drv Angular Vel Dmd"=w1675, "Drv Y Vel Dmd"=w1676, "Drv X Vel Dmd"=w1677) -> ()  [unwired: 8 in]
        n965 = Equal?(x=w1657, y=w1656) -> (x = y?=w1662:bool)
        n966 = Divide(x=w1657, y=w1656) -> (x/y=w1659:dbl)
        n967 = Greater?(x=w1659, y=0.7) -> (0:w1654:bool)
        n968 = call-poly <vilib>:"NT Read Value.vi"("default value"=FALSE ("value"), "name"="Shooter/Limited") -> ("value"=w1655:bool)  [unwired: 7 in, 2 out]
        n969 = case shown="True" w1655 {
          tunnel: w1654 -> [_ w1683]
          frame False {
            n970 = call-poly <vilib>:"NT Write Value.vi"("value"="Intake Mode" ("default value"), "name"="Robot State") -> ()  [unwired: 9 in, 1 out]
          }
          frame True {
            n971 = case shown="False" w1683 {
              frame False {
                n972 = call-poly <vilib>:"NT Write Value.vi"("value"=TRUE, "name"="Shooter/Overwrite Angle") -> ()  [unwired: 9 in, 1 out]
                n973 = call-poly <vilib>:"NT Write Value.vi"("value"=53.0, "name"="Shooter/Angle_Deg Dmd") -> ()  [unwired: 9 in, 1 out]
              }
              frame True {
                n974 = call-poly <vilib>:"NT Write Value.vi"("value"=FALSE, "name"="Shooter/Overwrite Angle") -> ()  [unwired: 9 in, 1 out]
              }
            }
            n975 = call-poly <vilib>:"NT Write Value.vi"("value"="Shoot Mode" ("default value"), "name"="Robot State") -> ()  [unwired: 9 in, 1 out]
            n976 = call-poly <vilib>:"NT Write Value.vi"("value"="Stop" ("default value"), "name"="Intake/Trigger Status") -> ()  [unwired: 9 in, 1 out]
          }
        }
      }
      n977 = while {
        tunnel: w1486 -> [w1652]
        tunnel: [w1652] -> w1484
        i -> [w1650]
        stop <- w1649 stop-if-true
        w1648 = 0.0 ("Drv X Vel Dmd")
        n978 = Not Equal To 0?(x=w1650) -> (x != 0?=w1649:bool)
        n979 = Wait (ms)(milliseconds to wait=u32 20) -> ()  [unwired: 1 out]
        n980 = call-poly <vilib>:"NT Write Value.vi"("value"="Shoot Mode" ("default value"), "name"="Robot State") -> ()  [unwired: 9 in, 1 out]
        n981 = call-poly <vilib>:"NT Write Value.vi"("value"=FALSE, "name"="Shooter/Overwrite Angle") -> ()  [unwired: 9 in, 1 out]
        n982 = call "SWERVE_DRIVE_MODULE_STATES_POSITIONS_FGV.vi"() -> ("out Current Module Positions"=w1644:T11[])  [unwired: 10 in, 1 out]
        n983 = call "SWERVE_DRIVE_GET_GYRO.vi"() -> ("Gyro Heading Radians"=w1646:dbl)  [unwired: 11 in]
        n984 = call "SWERVE_DRIVE_GET_GYRO.vi"() -> ("Gyro Heading Radians"=w1647:dbl)  [unwired: 11 in]
        n985 = call <vilib>:"Rotation2d_CreateAngle.vi"("Angle"=w1646) -> ("ROTATION"=w1645:T9)  [unwired: 10 in]
        n986 = call "SWERVE_DRIVE_SET_SPEED_DEMAND.vi"("Drv Rotation Orentation Dmd"=w1647, "Drv Angular Vel Dmd"=w1648, "Drv Y Vel Dmd"=w1648, "Drv X Vel Dmd"=w1648) -> ()  [unwired: 8 in]
        n987 = call "SWERVE_TRAJECTORY_BEGIN.vi"("gyroAngle"=w1645, "Module Positions"=w1644, "Trajectory File Name"="Path Demo.wpilib.csv") -> ()  [unwired: 9 in]
      }
      n988 = while {
        tunnel: w1484 -> [w1630]
        tunnel: [w1630] -> _
        i -> [w1612]
        stop <- FALSE stop-if-true
        w1618 = 0.0 ("Drv X Vel Dmd")
        # "End the loop early if shooter angle and orientation tolerance is meeted"
        n989 = Greater?(x=w1612, y=200) -> (0:w1608:bool)
        n990 = call-poly <vilib>:"NT Read Value.vi"("name"="/limelight-shooter/tv") -> ("value"=w1621:dbl)  [unwired: 8 in, 2 out]
        n991 = call-poly <vilib>:"NT Read Value.vi"("name"="Shooter/Corrected Theta") -> ("value"=w1615:dbl)  [unwired: 8 in, 2 out]
        n992 = call-poly <vilib>:"NT Read Value.vi"("name"="Shooter/Angle_Deg Act") -> ("value"=w1627:dbl)  [unwired: 8 in, 2 out]
        n993 = call-poly <vilib>:"NT Read Value.vi"("name"="Shooter/Angle_Deg Dmd") -> ("value"=w1626:dbl)  [unwired: 8 in, 2 out]
        n994 = Not Equal To 0?(x=w1621) -> (x != 0?=w1620:bool)
        n995 = call "SWERVE_DRIVE_GET_GYRO.vi"() -> ("Gyro Heading Radians"=w1616:dbl)  [unwired: 11 in]
        n996 = Select(t=w1615, s=w1620, f=w1616) -> (s? t:f=w1619:dbl)
        n997 = call <vilib>:"Util_ApproxEquals.vi"("Tolerance"=2.5, "Value 2"=w1626, "Value 1"=w1627) -> ("ApproxEquals"=w1617:bool)  [unwired: 8 in]
        n998 = call <vilib>:"Util_ApproxEquals.vi"("Tolerance"=0.07, "Value 2"=w1616, "Value 1"=w1615) -> ("ApproxEquals"=w1613:bool)  [unwired: 8 in]
        n999 = And(x=w1617, y=w1613) -> (x .and. y?=w1610:bool)
        n1000 = Or(x=w1610, y=w1608) -> (x .or. y?=w1609:bool)
        n1001 = case shown="False" w1609 {
          frame False {
            n1002 = call-poly <vilib>:"NT Write Value.vi"("value"="Stop" ("default value"), "name"="Intake/Trigger Status") -> ()  [unwired: 9 in, 1 out]
          }
          frame True {
            n1003 = call-poly <vilib>:"NT Write Value.vi"("value"="ToShooter" ("default value"), "name"="Intake/Trigger Status") -> ()  [unwired: 9 in, 1 out]
          }
        }
        n1004 = call "SWERVE_DRIVE_SET_SPEED_DEMAND.vi"("Drv Rotation Orentation Dmd"=w1619, "Drv Angular Vel Dmd"=w1618, "Drv Y Vel Dmd"=w1618, "Drv X Vel Dmd"=w1618) -> ()  [unwired: 8 in]
        n1005 = Wait (ms)(milliseconds to wait=u32 20) -> ()  [unwired: 1 out]
      }
      n1006 = disable-structure shown="Disabled" {
        frame Disabled {
          n1007 = while {
            tunnel: _ -> [w1592]
            tunnel: [w1592] -> w1515
            i -> [w1590]
            stop <- w1589 stop-if-true
            # "Wait until shooting finishes"
            n1008 = Equal To 0?(x=w1590) -> (x = 0?=w1589:bool)
            n1009 = Wait (ms)(milliseconds to wait=u32 400) -> ()  [unwired: 1 out]
          }
          n1010 = while {
            tunnel: w1515 -> [w1606]
            tunnel: [w1606] -> w1514
            i -> [w1604]
            stop <- w1603 stop-if-true
            (unwired) "Add Vision" ("name")
            w1600 = FALSE  # ABS Odo Initialize
            w1602 = 0.0 ("Drv X Vel Dmd")
            # "TBD"
            n1011 = Not Equal To 0?(x=w1604) -> (x != 0?=w1603:bool)
            n1012 = Wait (ms)(milliseconds to wait=u32 20) -> ()  [unwired: 1 out]
            n1013 = call-poly <vilib>:"NT Write Value.vi"("value"=FALSE ("default value")) -> ()  [unwired: 10 in, 1 out]
            n1014 = call-poly <vilib>:"NT Write Value.vi"("value"="Intake Mode" ("default value"), "name"="Robot State") -> ()  [unwired: 9 in, 1 out]
            n1015 = call "SWERVE_DRIVE_MODULE_STATES_POSITIONS_FGV.vi"() -> ("out Current Module Positions"=w1597:T11[])  [unwired: 10 in, 1 out]
            n1016 = call "SWERVE_DRIVE_GET_GYRO.vi"() -> ("Gyro Heading Radians"=w1599:dbl)  [unwired: 11 in]
            n1017 = call "SWERVE_DRIVE_GET_GYRO.vi"() -> ("Gyro Heading Radians"=w1601:dbl)  [unwired: 11 in]
            n1018 = call <vilib>:"Rotation2d_CreateAngle.vi"("Angle"=w1599) -> ("ROTATION"=w1598:T9)  [unwired: 10 in]
            n1019 = call "SWERVE_DRIVE_SET_SPEED_DEMAND.vi"("Drv Rotation Orentation Dmd"=w1601, "Drv Angular Vel Dmd"=w1602, "Drv Y Vel Dmd"=w1602, "Drv X Vel Dmd"=w1602) -> ()  [unwired: 8 in]
            n1020 = call "SWERVE_TRAJECTORY_BEGIN.vi"("ABS Odo Initialize"=w1600, "gyroAngle"=w1598, "Module Positions"=w1597, "Trajectory File Name"="Route C2 B Path 2.path") -> ()  [unwired: 8 in]
          }
          n1021 = while {
            tunnel: w1514 -> [w1570]
            tunnel: [w1570] -> w1513
            i -> [w1569]
            stop <- w1552 stop-if-true
            w1553 = TRUE  # ABS_Traj ?
            w1561 = TRUE  # EnableClosedLoop
            w1559 = FALSE  # Reverse
            w1563 = TRUE  # Follow Orientation
            # "During the second half of the path, switch to Shoot Mode but stop the trigger when limit switch pressed"
            n1022 = Equal To 0?(x=w1569) -> (x = 0?=w1560:bool)
            n1023 = call "SWERVE_DRIVE_GET_SPEED_DEMAND.vi"() -> ("Drv Rotation Orentation Dmd"=w1568:dbl)  [unwired: 8 in, 3 out]
            n1024 = call "SWERVE_DRIVE_GET_GYRO.vi"() -> ("Gyro Heading Radians"=w1558:dbl)  [unwired: 11 in]
            n1025 = Wait Until Next ms Multiple(millisecond multiple=u32 20 ("milliseconds to wait")) -> ()  [unwired: 1 out]
            n1026 = call "SWERVE_TRAJECTORY_EXECUTE.vi"("EnableClosedLoop"=w1561, "ABS_Traj ?"=w1553, "Init"=w1560, "Reverse"=w1559, "Follow Orientation"=w1563, "Gyro Heading\nRAD"=w1558) -> ("AtReference"=w1554:bool, "OutputTRAJ_STATE"=w1555:T12, "Error and Corr"=w1556:T13, "Chassis Velocity Target"=w1562:T14, "Orientation Target"=w1557:dbl)  [unwired: 1 in]
            n1027 = Select(t=w1558, s=w1563, f=w1568) -> (s? t:f=w1564:dbl)
            n1028 = call "SWERVE_TRAJECTORY_SET_CLOSED_LOOP.vi"("AUTO_CLOSED_LOOP"=w1561) -> ()  [unwired: 11 in]
            n1029 = call "SWERVE_TRAJECTORY_UPDATE_DIAG_INFO.vi"("AtReference"=w1554, "OutputTRAJ_STATE"=w1555, "Error and Corr"=w1556, "Orientation Target"=w1557) -> ()  [unwired: 8 in]
            n1030 = Unbundle By Name(w1562) -> ("vX"=w1567:dbl, "vY"=w1566:dbl, "vOmega"=w1565:dbl)
            n1031 = global read "SWERVE_TRAJECTORY_GLOBALS.vi" "Traj_Total_Time"() -> (w1547:dbl)
            n1032 = Unbundle By Name(w1555) -> ("TimeSeconds"=w1548:dbl)
            n1033 = call "SWERVE_DRIVE_SET_SPEED_DEMAND.vi"("Drv Rotation Orentation Dmd"=w1564, "Drv Angular Vel Dmd"=w1565, "Drv Y Vel Dmd"=w1566, "Drv X Vel Dmd"=w1567) -> ()  [unwired: 8 in]
            n1034 = Equal?(x=w1548, y=w1547) -> (x = y?=w1552:bool)
            n1035 = Divide(x=w1548, y=w1547) -> (x/y=w1546:dbl)
            n1036 = Greater?(x=w1546, y=0.6) -> (0:w1544:bool)
            n1037 = call-poly <vilib>:"NT Read Value.vi"("default value"=FALSE ("value"), "name"="Shooter/Limited") -> ("value"=w1550:bool)  [unwired: 7 in, 2 out]
            n1038 = case shown="True" w1550 {
              tunnel: w1544 -> [_ w1574]
              frame False {
                n1039 = call-poly <vilib>:"NT Write Value.vi"("value"="Intake Mode" ("default value"), "name"="Robot State") -> ()  [unwired: 9 in, 1 out]
              }
              frame True {
                n1040 = case shown="True" w1574 {
                  frame False {
                  }
                  frame True {
                    n1041 = call-poly <vilib>:"NT Write Value.vi"("value"="Shoot Mode" ("default value"), "name"="Robot State") -> ()  [unwired: 9 in, 1 out]
                  }
                }
                n1042 = call-poly <vilib>:"NT Write Value.vi"("value"="Stop" ("default value"), "name"="Intake/Trigger Status") -> ()  [unwired: 9 in, 1 out]
              }
            }
          }
          n1043 = while {
            tunnel: w1513 -> [w1588]
            tunnel: [w1588] -> w1512
            i -> [w1586]
            stop <- w1585 stop-if-true
            w1584 = 0.0 ("Drv X Vel Dmd")
            n1044 = Not Equal To 0?(x=w1586) -> (x != 0?=w1585:bool)
            n1045 = Wait (ms)(milliseconds to wait=u32 20) -> ()  [unwired: 1 out]
            n1046 = call "SWERVE_DRIVE_MODULE_STATES_POSITIONS_FGV.vi"() -> ("out Current Module Positions"=w1580:T11[])  [unwired: 10 in, 1 out]
            n1047 = call "SWERVE_DRIVE_GET_GYRO.vi"() -> ("Gyro Heading Radians"=w1582:dbl)  [unwired: 11 in]
            n1048 = call "SWERVE_DRIVE_GET_GYRO.vi"() -> ("Gyro Heading Radians"=w1583:dbl)  [unwired: 11 in]
            n1049 = call <vilib>:"Rotation2d_CreateAngle.vi"("Angle"=w1582) -> ("ROTATION"=w1581:T9)  [unwired: 10 in]
            n1050 = call "SWERVE_DRIVE_SET_SPEED_DEMAND.vi"("Drv Rotation Orentation Dmd"=w1583, "Drv Angular Vel Dmd"=w1584, "Drv Y Vel Dmd"=w1584, "Drv X Vel Dmd"=w1584) -> ()  [unwired: 8 in]
            n1051 = call "SWERVE_TRAJECTORY_BEGIN.vi"("gyroAngle"=w1581, "Module Positions"=w1580, "Trajectory File Name"="Path Demo.wpilib.csv") -> ()  [unwired: 9 in]
          }
          n1052 = while {
            tunnel: w1512 -> [w1539]
            tunnel: [w1539] -> _
            i -> [w1520]
            stop <- FALSE stop-if-true
            w1527 = 0.0 ("Drv X Vel Dmd")
            n1053 = Greater?(x=w1520, y=15) -> (0:w1516:bool)
            n1054 = call-poly <vilib>:"NT Read Value.vi"("name"="/limelight-shooter/tv") -> ("value"=w1530:dbl)  [unwired: 8 in, 2 out]
            n1055 = call-poly <vilib>:"NT Read Value.vi"("name"="Shooter/Corrected Theta") -> ("value"=w1524:dbl)  [unwired: 8 in, 2 out]
            n1056 = call-poly <vilib>:"NT Read Value.vi"("name"="Shooter/Angle_Deg Act") -> ("value"=w1536:dbl)  [unwired: 8 in, 2 out]
            n1057 = call-poly <vilib>:"NT Read Value.vi"("name"="Shooter/Angle_Deg Dmd") -> ("value"=w1535:dbl)  [unwired: 8 in, 2 out]
            n1058 = Not Equal To 0?(x=w1530) -> (x != 0?=w1529:bool)
            n1059 = call "SWERVE_DRIVE_GET_GYRO.vi"() -> ("Gyro Heading Radians"=w1525:dbl)  [unwired: 11 in]
            n1060 = Select(t=w1524, s=w1529, f=w1525) -> (s? t:f=w1528:dbl)
            n1061 = call <vilib>:"Util_ApproxEquals.vi"("Tolerance"=3.5, "Value 2"=w1535, "Value 1"=w1536) -> ("ApproxEquals"=w1526:bool)  [unwired: 8 in]
            n1062 = call <vilib>:"Util_ApproxEquals.vi"("Tolerance"=0.1, "Value 2"=w1525, "Value 1"=w1524) -> ("ApproxEquals"=w1522:bool)  [unwired: 8 in]
            n1063 = And(x=w1526, y=w1522) -> (x .and. y?=w1518:bool)
            n1064 = Or(x=w1518, y=w1516) -> (x .or. y?=w1517:bool)
            n1065 = case shown="True" w1517 {
              frame False {
                n1066 = call-poly <vilib>:"NT Write Value.vi"("value"="Stop" ("default value"), "name"="Intake/Trigger Status") -> ()  [unwired: 9 in, 1 out]
              }
              frame True {
                n1067 = call-poly <vilib>:"NT Write Value.vi"("value"="ToShooter" ("default value"), "name"="Intake/Trigger Status") -> ()  [unwired: 9 in, 1 out]
              }
            }
            n1068 = call "SWERVE_DRIVE_SET_SPEED_DEMAND.vi"("Drv Rotation Orentation Dmd"=w1528, "Drv Angular Vel Dmd"=w1527, "Drv Y Vel Dmd"=w1527, "Drv X Vel Dmd"=w1527) -> ()  [unwired: 8 in]
            n1069 = Wait (ms)(milliseconds to wait=u32 20) -> ()  [unwired: 1 out]
          }
        }
        frame Enabled {
        }
      }
    }
    frame "Route C2 Red" {
      w1713 = errorcluster {"status"=FALSE, "code"=0, "source"=""}  # Start Error Flow
      n1070 = while {
        tunnel: w1713 -> [w1929]
        tunnel: [w1929] -> w1710
        i -> [w1927]
        stop <- w1926 stop-if-true
        w1923 = TRUE  # ABS Odo Initialize
        w1925 = 0.0 ("Drv X Vel Dmd")
        n1071 = Not Equal To 0?(x=w1927) -> (x != 0?=w1926:bool)
        n1072 = Wait (ms)(milliseconds to wait=u32 20) -> ()  [unwired: 1 out]
        n1073 = call-poly <vilib>:"NT Read Value.vi"("default value"="Path_Testing_1.path" ("Trajectory File Name"), "name"="Initial Path") -> ("value"=w1920:string)  [unwired: 7 in, 2 out]
        n1074 = call "SWERVE_DRIVE_MODULE_STATES_POSITIONS_FGV.vi"() -> ("out Current Module Positions"=w1917:T11[])  [unwired: 10 in, 1 out]
        n1075 = call "SWERVE_DRIVE_GET_GYRO.vi"() -> ("Gyro Heading Radians"=w1919:dbl)  [unwired: 11 in]
        n1076 = call "SWERVE_DRIVE_GET_GYRO.vi"() -> ("Gyro Heading Radians"=w1924:dbl)  [unwired: 11 in]
        n1077 = call <vilib>:"Rotation2d_CreateAngle.vi"("Angle"=w1919) -> ("ROTATION"=w1918:T9)  [unwired: 10 in]
        n1078 = call "SWERVE_DRIVE_SET_SPEED_DEMAND.vi"("Drv Rotation Orentation Dmd"=w1924, "Drv Angular Vel Dmd"=w1925, "Drv Y Vel Dmd"=w1925, "Drv X Vel Dmd"=w1925) -> ()  [unwired: 8 in]
        n1079 = call "SWERVE_TRAJECTORY_BEGIN.vi"("ABS Odo Initialize"=w1923, "gyroAngle"=w1918, "Module Positions"=w1917, "Trajectory File Name"=w1920) -> ()  [unwired: 8 in]
      }
      n1080 = while {
        tunnel: w1710 -> [w1774]
        tunnel: [w1774] -> w1709
        stop <- w1755 stop-if-true
        # "Shoot Preload"
        n1081 = Wait (ms)(milliseconds to wait=u32 20) -> ()  [unwired: 1 out]
        n1082 = call-poly <vilib>:"NT Read Value.vi"("default value"=0.0, "name"="Shooter/Speed_RPM Act") -> ("value"=w1769:dbl)  [unwired: 7 in, 2 out]
        n1083 = call-poly <vilib>:"NT Read Value.vi"("name"="Shooter/Angle_Deg Act") -> ("value"=w1759:dbl)  [unwired: 8 in, 2 out]
        n1084 = call-poly <vilib>:"NT Read Value.vi"("name"="Shooter/Angle_Deg Dmd") -> ("value"=w1758:dbl)  [unwired: 8 in, 2 out]
        n1085 = call-poly <vilib>:"NT Write Value.vi"("value"="Shoot Mode" ("default value"), "name"="Robot State") -> ()  [unwired: 9 in, 1 out]
        n1086 = Greater?(x=w1769, y=2000.0) -> (0:w1757:bool)
        n1087 = call <vilib>:"Util_ApproxEquals.vi"("Tolerance"=2.0, "Value 2"=w1758, "Value 1"=w1759) -> ("ApproxEquals"=w1756:bool)  [unwired: 8 in]
        n1088 = And(x=w1757, y=w1756) -> (x .and. y?=w1755:bool)
        n1089 = case shown="True" w1755 {
          frame False {
            n1090 = call-poly <vilib>:"NT Write Value.vi"("value"="Stop" ("default value"), "name"="Intake/Trigger Status") -> ()  [unwired: 9 in, 1 out]
          }
          frame True {
            n1091 = call-poly <vilib>:"NT Write Value.vi"("value"="ToShooter" ("default value"), "name"="Intake/Trigger Status") -> ()  [unwired: 9 in, 1 out]
          }
        }
        n1092 = call-poly <vilib>:"NT Write Value.vi"("value"=TRUE, "name"="Shooter/Overwrite Angle") -> ()  [unwired: 9 in, 1 out]
        n1093 = call-poly <vilib>:"NT Write Value.vi"("value"=53.0, "name"="Shooter/Angle_Deg Dmd") -> ()  [unwired: 9 in, 1 out]
      }
      n1094 = while {
        tunnel: w1709 -> [w1906]
        tunnel: [w1906] -> w1708
        i -> [w1904]
        stop <- w1903 stop-if-true
        # "Wait until shooting finishes"
        n1095 = Equal To 0?(x=w1904) -> (x = 0?=w1903:bool)
        n1096 = Wait (ms)(milliseconds to wait=u32 300) -> ()  [unwired: 1 out]
      }
      n1097 = while {
        tunnel: w1708 -> [w1714]
        tunnel: [w1714] -> w1707
        i -> [w1740]
        stop <- w1723 stop-if-true
        w1724 = TRUE  # ABS_Traj ?
        w1732 = TRUE  # EnableClosedLoop
        w1730 = FALSE  # Reverse
        w1734 = TRUE  # Follow Orientation
        n1098 = Equal To 0?(x=w1740) -> (x = 0?=w1731:bool)
        n1099 = call "SWERVE_DRIVE_GET_SPEED_DEMAND.vi"() -> ("Drv Rotation Orentation Dmd"=w1739:dbl)  [unwired: 8 in, 3 out]
        n1100 = call "SWERVE_DRIVE_GET_GYRO.vi"() -> ("Gyro Heading Radians"=w1729:dbl)  [unwired: 11 in]
        n1101 = Wait Until Next ms Multiple(millisecond multiple=u32 20 ("milliseconds to wait")) -> ()  [unwired: 1 out]
        n1102 = call "SWERVE_TRAJECTORY_EXECUTE.vi"("EnableClosedLoop"=w1732, "ABS_Traj ?"=w1724, "Init"=w1731, "Reverse"=w1730, "Follow Orientation"=w1734, "Gyro Heading\nRAD"=w1729) -> ("AtReference"=w1725:bool, "OutputTRAJ_STATE"=w1726:T12, "Error and Corr"=w1727:T13, "Chassis Velocity Target"=w1733:T14, "Orientation Target"=w1728:dbl)  [unwired: 1 in]
        n1103 = Select(t=w1729, s=w1734, f=w1739) -> (s? t:f=w1735:dbl)
        n1104 = call "SWERVE_TRAJECTORY_SET_CLOSED_LOOP.vi"("AUTO_CLOSED_LOOP"=w1732) -> ()  [unwired: 11 in]
        n1105 = call "SWERVE_TRAJECTORY_UPDATE_DIAG_INFO.vi"("AtReference"=w1725, "OutputTRAJ_STATE"=w1726, "Error and Corr"=w1727, "Orientation Target"=w1728) -> ()  [unwired: 8 in]
        n1106 = Unbundle By Name(w1733) -> ("vX"=w1738:dbl, "vY"=w1737:dbl, "vOmega"=w1736:dbl)
        n1107 = global read "SWERVE_TRAJECTORY_GLOBALS.vi" "Traj_Total_Time"() -> (w1717:dbl)
        n1108 = Unbundle By Name(w1726) -> ("TimeSeconds"=w1718:dbl)
        n1109 = call "SWERVE_DRIVE_SET_SPEED_DEMAND.vi"("Drv Rotation Orentation Dmd"=w1735, "Drv Angular Vel Dmd"=w1736, "Drv Y Vel Dmd"=w1737, "Drv X Vel Dmd"=w1738) -> ()  [unwired: 8 in]
        n1110 = Equal?(x=w1718, y=w1717) -> (x = y?=w1723:bool)
        n1111 = Divide(x=w1718, y=w1717) -> (x/y=w1720:dbl)
        n1112 = Greater?(x=w1720, y=0.7) -> (0:w1715:bool)
        n1113 = call-poly <vilib>:"NT Read Value.vi"("default value"=FALSE ("value"), "name"="Shooter/Limited") -> ("value"=w1716:bool)  [unwired: 7 in, 2 out]
        n1114 = case shown="True" w1716 {
          tunnel: w1715 -> [_ w1744]
          frame False {
            n1115 = call-poly <vilib>:"NT Write Value.vi"("value"="Intake Mode" ("default value"), "name"="Robot State") -> ()  [unwired: 9 in, 1 out]
          }
          frame True {
            n1116 = case shown="False" w1744 {
              frame False {
                n1117 = call-poly <vilib>:"NT Write Value.vi"("value"=TRUE, "name"="Shooter/Overwrite Angle") -> ()  [unwired: 9 in, 1 out]
                n1118 = call-poly <vilib>:"NT Write Value.vi"("value"=53.0, "name"="Shooter/Angle_Deg Dmd") -> ()  [unwired: 9 in, 1 out]
              }
              frame True {
                n1119 = call-poly <vilib>:"NT Write Value.vi"("value"=FALSE, "name"="Shooter/Overwrite Angle") -> ()  [unwired: 9 in, 1 out]
              }
            }
            n1120 = call-poly <vilib>:"NT Write Value.vi"("value"="Shoot Mode" ("default value"), "name"="Robot State") -> ()  [unwired: 9 in, 1 out]
            n1121 = call-poly <vilib>:"NT Write Value.vi"("value"="Stop" ("default value"), "name"="Intake/Trigger Status") -> ()  [unwired: 9 in, 1 out]
          }
        }
      }
      n1122 = while {
        tunnel: w1707 -> [w1916]
        tunnel: [w1916] -> w1712
        i -> [w1914]
        stop <- w1913 stop-if-true
        w1912 = 0.0 ("Drv X Vel Dmd")
        # "TBD: use vision to correct robot position temporary"
        n1123 = Not Equal To 0?(x=w1914) -> (x != 0?=w1913:bool)
        n1124 = Wait (ms)(milliseconds to wait=u32 20) -> ()  [unwired: 1 out]
        n1125 = call "SWERVE_DRIVE_MODULE_STATES_POSITIONS_FGV.vi"() -> ("out Current Module Positions"=w1908:T11[])  [unwired: 10 in, 1 out]
        n1126 = call "SWERVE_DRIVE_GET_GYRO.vi"() -> ("Gyro Heading Radians"=w1910:dbl)  [unwired: 11 in]
        n1127 = call "SWERVE_DRIVE_GET_GYRO.vi"() -> ("Gyro Heading Radians"=w1911:dbl)  [unwired: 11 in]
        n1128 = call <vilib>:"Rotation2d_CreateAngle.vi"("Angle"=w1910) -> ("ROTATION"=w1909:T9)  [unwired: 10 in]
        n1129 = call "SWERVE_DRIVE_SET_SPEED_DEMAND.vi"("Drv Rotation Orentation Dmd"=w1911, "Drv Angular Vel Dmd"=w1912, "Drv Y Vel Dmd"=w1912, "Drv X Vel Dmd"=w1912) -> ()  [unwired: 8 in]
        n1130 = call "SWERVE_TRAJECTORY_BEGIN.vi"("gyroAngle"=w1909, "Module Positions"=w1908, "Trajectory File Name"="Path Demo.wpilib.csv") -> ()  [unwired: 9 in]
      }
      n1131 = while {
        tunnel: w1712 -> [w1898]
        tunnel: [w1898] -> w1711
        i -> [w1880]
        stop <- FALSE stop-if-true
        w1886 = 0.0 ("Drv X Vel Dmd")
        # "End the loop early if shooter angle and orientation tolerance is meeted"
        n1132 = Greater?(x=w1880, y=200) -> (0:w1876:bool)
        n1133 = call-poly <vilib>:"NT Read Value.vi"("name"="/limelight-shooter/tv") -> ("value"=w1889:dbl)  [unwired: 8 in, 2 out]
        n1134 = call-poly <vilib>:"NT Read Value.vi"("name"="Shooter/Corrected Theta") -> ("value"=w1883:dbl)  [unwired: 8 in, 2 out]
        n1135 = call-poly <vilib>:"NT Read Value.vi"("name"="Shooter/Angle_Deg Act") -> ("value"=w1895:dbl)  [unwired: 8 in, 2 out]
        n1136 = call-poly <vilib>:"NT Read Value.vi"("name"="Shooter/Angle_Deg Dmd") -> ("value"=w1894:dbl)  [unwired: 8 in, 2 out]
        n1137 = Not Equal To 0?(x=w1889) -> (x != 0?=w1888:bool)
        n1138 = call "SWERVE_DRIVE_GET_GYRO.vi"() -> ("Gyro Heading Radians"=w1884:dbl)  [unwired: 11 in]
        n1139 = Select(t=w1883, s=w1888, f=w1884) -> (s? t:f=w1887:dbl)
        n1140 = call <vilib>:"Util_ApproxEquals.vi"("Tolerance"=2.5, "Value 2"=w1894, "Value 1"=w1895) -> ("ApproxEquals"=w1885:bool)  [unwired: 8 in]
        n1141 = call <vilib>:"Util_ApproxEquals.vi"("Tolerance"=0.07, "Value 2"=w1884, "Value 1"=w1883) -> ("ApproxEquals"=w1881:bool)  [unwired: 8 in]
        n1142 = And(x=w1885, y=w1881) -> (x .and. y?=w1878:bool)
        n1143 = Or(x=w1878, y=w1876) -> (x .or. y?=w1877:bool)
        n1144 = case shown="False" w1877 {
          frame False {
            n1145 = call-poly <vilib>:"NT Write Value.vi"("value"="Stop" ("default value"), "name"="Intake/Trigger Status") -> ()  [unwired: 9 in, 1 out]
          }
          frame True {
            n1146 = call-poly <vilib>:"NT Write Value.vi"("value"="ToShooter" ("default value"), "name"="Intake/Trigger Status") -> ()  [unwired: 9 in, 1 out]
          }
        }
        n1147 = call "SWERVE_DRIVE_SET_SPEED_DEMAND.vi"("Drv Rotation Orentation Dmd"=w1887, "Drv Angular Vel Dmd"=w1886, "Drv Y Vel Dmd"=w1886, "Drv X Vel Dmd"=w1886) -> ()  [unwired: 8 in]
        n1148 = Wait (ms)(milliseconds to wait=u32 20) -> ()  [unwired: 1 out]
      }
      n1149 = disable-structure shown="Disabled" {
        disable-tunnel: w1711 -> [w1779 _]
        frame Disabled {
          n1150 = while {
            tunnel: w1779 -> [w1874]
            tunnel: [w1874] -> w1783
            i -> [w1872]
            stop <- w1871 stop-if-true
            # "Wait until shooting finishes"
            n1151 = Equal To 0?(x=w1872) -> (x = 0?=w1871:bool)
            n1152 = Wait (ms)(milliseconds to wait=u32 400) -> ()  [unwired: 1 out]
          }
          n1153 = while {
            tunnel: w1783 -> [w1870]
            tunnel: [w1870] -> w1782
            i -> [w1868]
            stop <- w1867 stop-if-true
            (unwired) "Add Vision" ("name")
            w1864 = FALSE  # ABS Odo Initialize
            w1866 = 0.0 ("Drv X Vel Dmd")
            # "TBD"
            n1154 = Not Equal To 0?(x=w1868) -> (x != 0?=w1867:bool)
            n1155 = Wait (ms)(milliseconds to wait=u32 20) -> ()  [unwired: 1 out]
            n1156 = call-poly <vilib>:"NT Write Value.vi"("value"=FALSE ("default value")) -> ()  [unwired: 10 in, 1 out]
            n1157 = call-poly <vilib>:"NT Write Value.vi"("value"="Intake Mode" ("default value"), "name"="Robot State") -> ()  [unwired: 9 in, 1 out]
            n1158 = call "SWERVE_DRIVE_MODULE_STATES_POSITIONS_FGV.vi"() -> ("out Current Module Positions"=w1861:T11[])  [unwired: 10 in, 1 out]
            n1159 = call "SWERVE_DRIVE_GET_GYRO.vi"() -> ("Gyro Heading Radians"=w1863:dbl)  [unwired: 11 in]
            n1160 = call "SWERVE_DRIVE_GET_GYRO.vi"() -> ("Gyro Heading Radians"=w1865:dbl)  [unwired: 11 in]
            n1161 = call <vilib>:"Rotation2d_CreateAngle.vi"("Angle"=w1863) -> ("ROTATION"=w1862:T9)  [unwired: 10 in]
            n1162 = call "SWERVE_DRIVE_SET_SPEED_DEMAND.vi"("Drv Rotation Orentation Dmd"=w1865, "Drv Angular Vel Dmd"=w1866, "Drv Y Vel Dmd"=w1866, "Drv X Vel Dmd"=w1866) -> ()  [unwired: 8 in]
            n1163 = call "SWERVE_TRAJECTORY_BEGIN.vi"("ABS Odo Initialize"=w1864, "gyroAngle"=w1862, "Module Positions"=w1861, "Trajectory File Name"="Route C2 R Path 2.path") -> ()  [unwired: 8 in]
          }
          n1164 = while {
            tunnel: w1782 -> [w1838]
            tunnel: [w1838] -> w1781
            i -> [w1837]
            stop <- w1820 stop-if-true
            w1821 = TRUE  # ABS_Traj ?
            w1829 = TRUE  # EnableClosedLoop
            w1827 = FALSE  # Reverse
            w1831 = TRUE  # Follow Orientation
            # "During the second half of the path, switch to Shoot Mode but stop the trigger when limit switch pressed"
            n1165 = Equal To 0?(x=w1837) -> (x = 0?=w1828:bool)
            n1166 = call "SWERVE_DRIVE_GET_SPEED_DEMAND.vi"() -> ("Drv Rotation Orentation Dmd"=w1836:dbl)  [unwired: 8 in, 3 out]
            n1167 = call "SWERVE_DRIVE_GET_GYRO.vi"() -> ("Gyro Heading Radians"=w1826:dbl)  [unwired: 11 in]
            n1168 = Wait Until Next ms Multiple(millisecond multiple=u32 20 ("milliseconds to wait")) -> ()  [unwired: 1 out]
            n1169 = call "SWERVE_TRAJECTORY_EXECUTE.vi"("EnableClosedLoop"=w1829, "ABS_Traj ?"=w1821, "Init"=w1828, "Reverse"=w1827, "Follow Orientation"=w1831, "Gyro Heading\nRAD"=w1826) -> ("AtReference"=w1822:bool, "OutputTRAJ_STATE"=w1823:T12, "Error and Corr"=w1824:T13, "Chassis Velocity Target"=w1830:T14, "Orientation Target"=w1825:dbl)  [unwired: 1 in]
            n1170 = Select(t=w1826, s=w1831, f=w1836) -> (s? t:f=w1832:dbl)
            n1171 = call "SWERVE_TRAJECTORY_SET_CLOSED_LOOP.vi"("AUTO_CLOSED_LOOP"=w1829) -> ()  [unwired: 11 in]
            n1172 = call "SWERVE_TRAJECTORY_UPDATE_DIAG_INFO.vi"("AtReference"=w1822, "OutputTRAJ_STATE"=w1823, "Error and Corr"=w1824, "Orientation Target"=w1825) -> ()  [unwired: 8 in]
            n1173 = Unbundle By Name(w1830) -> ("vX"=w1835:dbl, "vY"=w1834:dbl, "vOmega"=w1833:dbl)
            n1174 = global read "SWERVE_TRAJECTORY_GLOBALS.vi" "Traj_Total_Time"() -> (w1815:dbl)
            n1175 = Unbundle By Name(w1823) -> ("TimeSeconds"=w1816:dbl)
            n1176 = call "SWERVE_DRIVE_SET_SPEED_DEMAND.vi"("Drv Rotation Orentation Dmd"=w1832, "Drv Angular Vel Dmd"=w1833, "Drv Y Vel Dmd"=w1834, "Drv X Vel Dmd"=w1835) -> ()  [unwired: 8 in]
            n1177 = Equal?(x=w1816, y=w1815) -> (x = y?=w1820:bool)
            n1178 = Divide(x=w1816, y=w1815) -> (x/y=w1814:dbl)
            n1179 = Greater?(x=w1814, y=0.6) -> (0:w1812:bool)
            n1180 = call-poly <vilib>:"NT Read Value.vi"("default value"=FALSE ("value"), "name"="Shooter/Limited") -> ("value"=w1818:bool)  [unwired: 7 in, 2 out]
            n1181 = case shown="True" w1818 {
              tunnel: w1812 -> [_ w1842]
              frame False {
                n1182 = call-poly <vilib>:"NT Write Value.vi"("value"="Intake Mode" ("default value"), "name"="Robot State") -> ()  [unwired: 9 in, 1 out]
              }
              frame True {
                n1183 = case shown="True" w1842 {
                  frame False {
                  }
                  frame True {
                    n1184 = call-poly <vilib>:"NT Write Value.vi"("value"="Shoot Mode" ("default value"), "name"="Robot State") -> ()  [unwired: 9 in, 1 out]
                  }
                }
                n1185 = call-poly <vilib>:"NT Write Value.vi"("value"="Stop" ("default value"), "name"="Intake/Trigger Status") -> ()  [unwired: 9 in, 1 out]
              }
            }
          }
          n1186 = while {
            tunnel: w1781 -> [w1856]
            tunnel: [w1856] -> w1780
            i -> [w1854]
            stop <- w1853 stop-if-true
            w1852 = 0.0 ("Drv X Vel Dmd")
            n1187 = Not Equal To 0?(x=w1854) -> (x != 0?=w1853:bool)
            n1188 = Wait (ms)(milliseconds to wait=u32 20) -> ()  [unwired: 1 out]
            n1189 = call "SWERVE_DRIVE_MODULE_STATES_POSITIONS_FGV.vi"() -> ("out Current Module Positions"=w1848:T11[])  [unwired: 10 in, 1 out]
            n1190 = call "SWERVE_DRIVE_GET_GYRO.vi"() -> ("Gyro Heading Radians"=w1850:dbl)  [unwired: 11 in]
            n1191 = call "SWERVE_DRIVE_GET_GYRO.vi"() -> ("Gyro Heading Radians"=w1851:dbl)  [unwired: 11 in]
            n1192 = call <vilib>:"Rotation2d_CreateAngle.vi"("Angle"=w1850) -> ("ROTATION"=w1849:T9)  [unwired: 10 in]
            n1193 = call "SWERVE_DRIVE_SET_SPEED_DEMAND.vi"("Drv Rotation Orentation Dmd"=w1851, "Drv Angular Vel Dmd"=w1852, "Drv Y Vel Dmd"=w1852, "Drv X Vel Dmd"=w1852) -> ()  [unwired: 8 in]
            n1194 = call "SWERVE_TRAJECTORY_BEGIN.vi"("gyroAngle"=w1849, "Module Positions"=w1848, "Trajectory File Name"="Path Demo.wpilib.csv") -> ()  [unwired: 9 in]
          }
          n1195 = while {
            tunnel: w1780 -> [w1807]
            tunnel: [w1807] -> _
            i -> [w1788]
            stop <- FALSE stop-if-true
            w1795 = 0.0 ("Drv X Vel Dmd")
            n1196 = Greater?(x=w1788, y=15) -> (0:w1784:bool)
            n1197 = call-poly <vilib>:"NT Read Value.vi"("name"="/limelight-shooter/tv") -> ("value"=w1798:dbl)  [unwired: 8 in, 2 out]
            n1198 = call-poly <vilib>:"NT Read Value.vi"("name"="Shooter/Corrected Theta") -> ("value"=w1792:dbl)  [unwired: 8 in, 2 out]
            n1199 = call-poly <vilib>:"NT Read Value.vi"("name"="Shooter/Angle_Deg Act") -> ("value"=w1804:dbl)  [unwired: 8 in, 2 out]
            n1200 = call-poly <vilib>:"NT Read Value.vi"("name"="Shooter/Angle_Deg Dmd") -> ("value"=w1803:dbl)  [unwired: 8 in, 2 out]
            n1201 = Not Equal To 0?(x=w1798) -> (x != 0?=w1797:bool)
            n1202 = call "SWERVE_DRIVE_GET_GYRO.vi"() -> ("Gyro Heading Radians"=w1793:dbl)  [unwired: 11 in]
            n1203 = Select(t=w1792, s=w1797, f=w1793) -> (s? t:f=w1796:dbl)
            n1204 = call <vilib>:"Util_ApproxEquals.vi"("Tolerance"=3.5, "Value 2"=w1803, "Value 1"=w1804) -> ("ApproxEquals"=w1794:bool)  [unwired: 8 in]
            n1205 = call <vilib>:"Util_ApproxEquals.vi"("Tolerance"=0.1, "Value 2"=w1793, "Value 1"=w1792) -> ("ApproxEquals"=w1790:bool)  [unwired: 8 in]
            n1206 = And(x=w1794, y=w1790) -> (x .and. y?=w1786:bool)
            n1207 = Or(x=w1786, y=w1784) -> (x .or. y?=w1785:bool)
            n1208 = case shown="True" w1785 {
              frame False {
                n1209 = call-poly <vilib>:"NT Write Value.vi"("value"="Stop" ("default value"), "name"="Intake/Trigger Status") -> ()  [unwired: 9 in, 1 out]
              }
              frame True {
                n1210 = call-poly <vilib>:"NT Write Value.vi"("value"="ToShooter" ("default value"), "name"="Intake/Trigger Status") -> ()  [unwired: 9 in, 1 out]
              }
            }
            n1211 = call "SWERVE_DRIVE_SET_SPEED_DEMAND.vi"("Drv Rotation Orentation Dmd"=w1796, "Drv Angular Vel Dmd"=w1795, "Drv Y Vel Dmd"=w1795, "Drv X Vel Dmd"=w1795) -> ()  [unwired: 8 in]
            n1212 = Wait (ms)(milliseconds to wait=u32 20) -> ()  [unwired: 1 out]
          }
        }
        frame Enabled {
        }
      }
    }
    frame "Preload C Blue" {
      w1931 = errorcluster {"status"=FALSE, "code"=0, "source"=""}  # Start Error Flow
      n1213 = while {
        tunnel: w1931 -> [w1972]
        tunnel: [w1972] -> w1930
        i -> [w1970]
        stop <- w1969 stop-if-true
        w1966 = TRUE  # ABS Odo Initialize
        w1968 = 0.0 ("Drv X Vel Dmd")
        n1214 = Not Equal To 0?(x=w1970) -> (x != 0?=w1969:bool)
        n1215 = Wait (ms)(milliseconds to wait=u32 20) -> ()  [unwired: 1 out]
        n1216 = call-poly <vilib>:"NT Read Value.vi"("default value"="Path_Testing_1.path" ("Trajectory File Name"), "name"="Initial Path") -> ("value"=w1963:string)  [unwired: 7 in, 2 out]
        n1217 = call "SWERVE_DRIVE_MODULE_STATES_POSITIONS_FGV.vi"() -> ("out Current Module Positions"=w1960:T11[])  [unwired: 10 in, 1 out]
        n1218 = call "SWERVE_DRIVE_GET_GYRO.vi"() -> ("Gyro Heading Radians"=w1962:dbl)  [unwired: 11 in]
        n1219 = call "SWERVE_DRIVE_GET_GYRO.vi"() -> ("Gyro Heading Radians"=w1967:dbl)  [unwired: 11 in]
        n1220 = call <vilib>:"Rotation2d_CreateAngle.vi"("Angle"=w1962) -> ("ROTATION"=w1961:T9)  [unwired: 10 in]
        n1221 = call "SWERVE_DRIVE_SET_SPEED_DEMAND.vi"("Drv Rotation Orentation Dmd"=w1967, "Drv Angular Vel Dmd"=w1968, "Drv Y Vel Dmd"=w1968, "Drv X Vel Dmd"=w1968) -> ()  [unwired: 8 in]
        n1222 = call "SWERVE_TRAJECTORY_BEGIN.vi"("ABS Odo Initialize"=w1966, "gyroAngle"=w1961, "Module Positions"=w1960, "Trajectory File Name"=w1963) -> ()  [unwired: 8 in]
      }
      n1223 = while {
        tunnel: w1930 -> [w1932]
        tunnel: [w1932] -> _
        stop <- w1937 stop-if-true
        # "Shoot Preload"
        n1224 = Wait (ms)(milliseconds to wait=u32 20) -> ()  [unwired: 1 out]
        n1225 = call-poly <vilib>:"NT Read Value.vi"("default value"=0.0, "name"="Shooter/Speed_RPM Act") -> ("value"=w1951:dbl)  [unwired: 7 in, 2 out]
        n1226 = call-poly <vilib>:"NT Read Value.vi"("name"="Shooter/Angle_Deg Act") -> ("value"=w1941:dbl)  [unwired: 8 in, 2 out]
        n1227 = call-poly <vilib>:"NT Read Value.vi"("name"="Shooter/Angle_Deg Dmd") -> ("value"=w1940:dbl)  [unwired: 8 in, 2 out]
        n1228 = call-poly <vilib>:"NT Write Value.vi"("value"="Shoot Mode" ("default value"), "name"="Robot State") -> ()  [unwired: 9 in, 1 out]
        n1229 = call-poly <vilib>:"NT Write Value.vi"("value"=FALSE, "name"="Shooter/Overwrite RPM") -> ()  [unwired: 9 in, 1 out]
        n1230 = Greater?(x=w1951, y=2000.0) -> (0:w1939:bool)
        n1231 = call <vilib>:"Util_ApproxEquals.vi"("Tolerance"=3.0, "Value 2"=w1940, "Value 1"=w1941) -> ("ApproxEquals"=w1938:bool)  [unwired: 8 in]
        n1232 = And(x=w1939, y=w1938) -> (x .and. y?=w1937:bool)
        n1233 = case shown="True" w1937 {
          frame False {
            n1234 = call-poly <vilib>:"NT Write Value.vi"("value"="Stop" ("default value"), "name"="Intake/Trigger Status") -> ()  [unwired: 9 in, 1 out]
          }
          frame True {
            n1235 = call-poly <vilib>:"NT Write Value.vi"("value"="ToShooter" ("default value"), "name"="Intake/Trigger Status") -> ()  [unwired: 9 in, 1 out]
          }
        }
        n1236 = call-poly <vilib>:"NT Write Value.vi"("value"=TRUE, "name"="Shooter/Overwrite Angle") -> ()  [unwired: 9 in, 1 out]
        n1237 = call-poly <vilib>:"NT Write Value.vi"("value"=53.0, "name"="Shooter/Angle_Deg Dmd") -> ()  [unwired: 9 in, 1 out]
        n1238 = call-poly <vilib>:"NT Write Value.vi"("value"=2500.0, "name"="Shooter/RPM Dmd") -> ()  [unwired: 9 in, 1 out]
      }
    }
    frame "Preload C Red" {
      w1974 = errorcluster {"status"=FALSE, "code"=0, "source"=""}  # Start Error Flow
      n1239 = while {
        tunnel: w1974 -> [w2015]
        tunnel: [w2015] -> w1973
        i -> [w2013]
        stop <- w2012 stop-if-true
        w2009 = TRUE  # ABS Odo Initialize
        w2011 = 0.0 ("Drv X Vel Dmd")
        n1240 = Not Equal To 0?(x=w2013) -> (x != 0?=w2012:bool)
        n1241 = Wait (ms)(milliseconds to wait=u32 20) -> ()  [unwired: 1 out]
        n1242 = call-poly <vilib>:"NT Read Value.vi"("default value"="Path_Testing_1.path" ("Trajectory File Name"), "name"="Initial Path") -> ("value"=w2006:string)  [unwired: 7 in, 2 out]
        n1243 = call "SWERVE_DRIVE_MODULE_STATES_POSITIONS_FGV.vi"() -> ("out Current Module Positions"=w2003:T11[])  [unwired: 10 in, 1 out]
        n1244 = call "SWERVE_DRIVE_GET_GYRO.vi"() -> ("Gyro Heading Radians"=w2005:dbl)  [unwired: 11 in]
        n1245 = call "SWERVE_DRIVE_GET_GYRO.vi"() -> ("Gyro Heading Radians"=w2010:dbl)  [unwired: 11 in]
        n1246 = call <vilib>:"Rotation2d_CreateAngle.vi"("Angle"=w2005) -> ("ROTATION"=w2004:T9)  [unwired: 10 in]
        n1247 = call "SWERVE_DRIVE_SET_SPEED_DEMAND.vi"("Drv Rotation Orentation Dmd"=w2010, "Drv Angular Vel Dmd"=w2011, "Drv Y Vel Dmd"=w2011, "Drv X Vel Dmd"=w2011) -> ()  [unwired: 8 in]
        n1248 = call "SWERVE_TRAJECTORY_BEGIN.vi"("ABS Odo Initialize"=w2009, "gyroAngle"=w2004, "Module Positions"=w2003, "Trajectory File Name"=w2006) -> ()  [unwired: 8 in]
      }
      n1249 = while {
        tunnel: w1973 -> [w1975]
        tunnel: [w1975] -> _
        stop <- w1980 stop-if-true
        # "Shoot Preload"
        n1250 = Wait (ms)(milliseconds to wait=u32 20) -> ()  [unwired: 1 out]
        n1251 = call-poly <vilib>:"NT Read Value.vi"("default value"=0.0, "name"="Shooter/Speed_RPM Act") -> ("value"=w1994:dbl)  [unwired: 7 in, 2 out]
        n1252 = call-poly <vilib>:"NT Read Value.vi"("name"="Shooter/Angle_Deg Act") -> ("value"=w1984:dbl)  [unwired: 8 in, 2 out]
        n1253 = call-poly <vilib>:"NT Read Value.vi"("name"="Shooter/Angle_Deg Dmd") -> ("value"=w1983:dbl)  [unwired: 8 in, 2 out]
        n1254 = call-poly <vilib>:"NT Write Value.vi"("value"="Shoot Mode" ("default value"), "name"="Robot State") -> ()  [unwired: 9 in, 1 out]
        n1255 = call-poly <vilib>:"NT Write Value.vi"("value"=FALSE, "name"="Shooter/Overwrite RPM") -> ()  [unwired: 9 in, 1 out]
        n1256 = Greater?(x=w1994, y=2000.0) -> (0:w1982:bool)
        n1257 = call <vilib>:"Util_ApproxEquals.vi"("Tolerance"=3.0, "Value 2"=w1983, "Value 1"=w1984) -> ("ApproxEquals"=w1981:bool)  [unwired: 8 in]
        n1258 = And(x=w1982, y=w1981) -> (x .and. y?=w1980:bool)
        n1259 = case shown="True" w1980 {
          frame False {
            n1260 = call-poly <vilib>:"NT Write Value.vi"("value"="Stop" ("default value"), "name"="Intake/Trigger Status") -> ()  [unwired: 9 in, 1 out]
          }
          frame True {
            n1261 = call-poly <vilib>:"NT Write Value.vi"("value"="ToShooter" ("default value"), "name"="Intake/Trigger Status") -> ()  [unwired: 9 in, 1 out]
          }
        }
        n1262 = call-poly <vilib>:"NT Write Value.vi"("value"=TRUE, "name"="Shooter/Overwrite Angle") -> ()  [unwired: 9 in, 1 out]
        n1263 = call-poly <vilib>:"NT Write Value.vi"("value"=53.0, "name"="Shooter/Angle_Deg Dmd") -> ()  [unwired: 9 in, 1 out]
        n1264 = call-poly <vilib>:"NT Write Value.vi"("value"=2500.0, "name"="Shooter/RPM Dmd") -> ()  [unwired: 9 in, 1 out]
      }
    }
    frame "Trap" {
      n1265 = while {
        stop <- FALSE stop-if-true
        w2016 = 120.0 ("Heading_Deg")
        w2036 = 1.0  # Kn
        w2039 = 3.0  # Kp
        w2048 = 0.0  # Ki
        w2049 = 0.0  # Kd
        w2050 = 9.9e+30  # MaximumIntegral
        w2051 = -9.9e+30  # MinimumIntegral
        w2034 = 1.0  # Kn
        w2037 = 5.0  # Kp
        w2040 = 0.0  # Ki
        w2041 = 0.0  # Kd
        w2042 = 9.9e+30  # MaximumIntegral
        w2043 = -9.9e+30  # MinimumIntegral
        w2035 = 1.0  # Kn
        w2038 = 5.0  # Kp
        w2044 = 0.0  # Ki
        w2045 = 0.0  # Kd
        w2046 = 9.9e+30  # MaximumIntegral
        w2047 = -9.9e+30  # MinimumIntegral
        w2033 = 0.0  # Max Accel
        w2032 = 0.0  # Max Speed
        # "Holonomic Drive\nController"
        # "Theta Controller"
        # "Y Controller"
        # "X Controller"
        n1266 = call <vilib>:"Rotation2d_CreateAngleDegrees.vi"("Angle_Degrees"=120.0) -> ("ROTATION"=w2027:T9)  [unwired: 10 in]
        n1267 = call "SWERVE_ODOM_ABS_FGV.vi"() -> ("out SWERVE_DRIVE_POSE_EST2"=w2030:T20)  [unwired: 10 in, 1 out]
        n1268 = call <vilib>:"PIDController_Pack_Tuning.vi"("MinimumIntegral"=w2043, "MaximumIntegral"=w2042, "Kn"=w2034, "Kd"=w2041, "Ki"=w2040, "Kp"=w2037) -> ("PID Tuning"=w2053:T26)  [unwired: 5 in]
        n1269 = call <vilib>:"PIDController_Pack_Tuning.vi"("MinimumIntegral"=w2047, "MaximumIntegral"=w2046, "Kn"=w2035, "Kd"=w2045, "Ki"=w2044, "Kp"=w2038) -> ("PID Tuning"=w2055:T26)  [unwired: 5 in]
        n1270 = call <vilib>:"PIDController_Pack_Tuning.vi"("MinimumIntegral"=w2051, "MaximumIntegral"=w2050, "Kn"=w2036, "Kd"=w2049, "Ki"=w2048, "Kp"=w2039) -> ("PID Tuning"=w2031:T26)  [unwired: 5 in]
        n1271 = Unbundle By Name(w2030) -> ("Swerve_Drive_Odom.POSE"=w2029:T7)
        n1272 = call <vilib>:"HolDrvCtrl_PackProfPID.vi"("Max Accel"=w2033, "Max Speed"=w2032, "Theta PID Tuning"=w2031) -> ("Theta PID CONTROLLER"=w2054:T27)  [unwired: 8 in]
        n1273 = call <vilib>:"HolDrvCtrl_PackExecuteSP.vi"("LinearVel"=0.0, "Heading_Deg"=w2016, "Y"=5.081, "X"=4.37) -> ("HolExecuteSP"=w2052:cluster{"DesiredPose":T7, "LinearVel":dbl})  [unwired: 7 in]
        n1274 = call <vilib>:"HolDrvCtrl_PackControllers.vi"("thetaProfiledPID_CTRL"=w2054, "Y PID Tuning"=w2055, "X PID Tuning"=w2053) -> ("HOLONOMIC_CTRL_PACK_TUNING"=w2056:T31)  [unwired: 8 in]
        n1275 = call <vilib>:"HolDrvCtrl_Execute.vi"("HOLONOMIC_CTRL_PACK_TUNING"=w2056, "Enable"=TRUE, "angleRef"=w2027, "HolExecuteSP"=w2052, "currentPose"=w2029) -> ("calcChassisSpeed"=w2020:T14)  [unwired: 4 in, 2 out]
        n1276 = Unbundle By Name(w2020) -> ("vX"=w2019:dbl, "vY"=w2018:dbl, "vOmega"=w2017:dbl)
        n1277 = call "SWERVE_DRIVE_SET_SPEED_DEMAND.vi"("Drv Rotation Orentation Dmd"=w2016, "Drv Angular Vel Dmd"=w2017, "Drv Y Vel Dmd"=w2018, "Drv X Vel Dmd"=w2019) -> ()  [unwired: 8 in]
        n1278 = Wait (ms)(milliseconds to wait=u32 20) -> ()  [unwired: 1 out]
      }
    }
    frame "Preload Only" {
      w2057 = errorcluster {"status"=FALSE, "code"=0, "source"=""}  # Start Error Flow
      n1279 = while {
        tunnel: w2057 -> [w2067]
        tunnel: [w2067] -> _
        stop <- FALSE stop-if-true
        # "Shoot Preload"
        n1280 = Wait (ms)(milliseconds to wait=u32 20) -> ()  [unwired: 1 out]
        n1281 = call-poly <vilib>:"NT Read Value.vi"("default value"=0.0, "name"="Shooter/Speed_RPM Act") -> ("value"=w2062:dbl)  [unwired: 7 in, 2 out]
        n1282 = call-poly <vilib>:"NT Write Value.vi"("value"="Shoot Mode" ("default value"), "name"="Robot State") -> ()  [unwired: 9 in, 1 out]
        n1283 = Greater?(x=w2062, y=4000.0) -> (0:w2060:bool)
        n1284 = case shown="False" w2060 {
          frame False {
            n1285 = call-poly <vilib>:"NT Write Value.vi"("value"="Stop" ("default value"), "name"="Intake/Trigger Status") -> ()  [unwired: 9 in, 1 out]
          }
          frame True {
            n1286 = call-poly <vilib>:"NT Write Value.vi"("value"="ToShooter" ("default value"), "name"="Intake/Trigger Status") -> ()  [unwired: 9 in, 1 out]
          }
        }
      }
    }
    frame "ToSource" {
      w2073 = errorcluster {"status"=FALSE, "code"=0, "source"=""}  # Start Error Flow
      n1287 = while {
        tunnel: w2073 -> [w2118]
        tunnel: [w2118] -> w2072
        stop <- w2119 stop-if-true
        w2116 = -148.0 ("Angle_Degrees")
        w2136 = 1.0  # Kn
        w2139 = 1.0  # Kp
        w2148 = 0.0  # Ki
        w2149 = 0.0  # Kd
        w2150 = 9.9e+30  # MaximumIntegral
        w2151 = -9.9e+30  # MinimumIntegral
        w2134 = 1.0  # Kn
        w2137 = 5.0  # Kp
        w2140 = 0.0  # Ki
        w2141 = 0.0  # Kd
        w2142 = 9.9e+30  # MaximumIntegral
        w2143 = -9.9e+30  # MinimumIntegral
        w2135 = 1.0  # Kn
        w2138 = 5.0  # Kp
        w2144 = 0.0  # Ki
        w2145 = 0.0  # Kd
        w2146 = 9.9e+30  # MaximumIntegral
        w2147 = -9.9e+30  # MinimumIntegral
        # "Holonomic Drive\nController"
        # "Theta Controller"
        # "Y Controller"
        # "X Controller"
        n1288 = call "SWERVE_DRIVE_GET_MAX.vi"() -> ("Max Rotational Vel (Rad/Sec)"=w2115:dbl)  [unwired: 10 in, 1 out]
        n1289 = call <vilib>:"Rotation2d_CreateAngleDegrees.vi"("Angle_Degrees"=w2116) -> ("ROTATION"=w2130:T9)  [unwired: 10 in]
        n1290 = call "SWERVE_ODOM_ABS_FGV.vi"() -> ("out SWERVE_DRIVE_POSE_EST2"=w2132:T20)  [unwired: 10 in, 1 out]
        n1291 = call <vilib>:"PIDController_Pack_Tuning.vi"("MinimumIntegral"=w2143, "MaximumIntegral"=w2142, "Kn"=w2134, "Kd"=w2141, "Ki"=w2140, "Kp"=w2137) -> ("PID Tuning"=w2153:T26)  [unwired: 5 in]
        n1292 = call <vilib>:"PIDController_Pack_Tuning.vi"("MinimumIntegral"=w2147, "MaximumIntegral"=w2146, "Kn"=w2135, "Kd"=w2145, "Ki"=w2144, "Kp"=w2138) -> ("PID Tuning"=w2155:T26)  [unwired: 5 in]
        n1293 = call <vilib>:"PIDController_Pack_Tuning.vi"("MinimumIntegral"=w2151, "MaximumIntegral"=w2150, "Kn"=w2136, "Kd"=w2149, "Ki"=w2148, "Kp"=w2139) -> ("PID Tuning"=w2133:T26)  [unwired: 5 in]
        n1294 = Unbundle By Name(w2132) -> ("Swerve_Drive_Odom.POSE"=w2131:T7)
        n1295 = call <vilib>:"HolDrvCtrl_PackProfPID.vi"("Max Accel"=w2115, "Max Speed"=w2115, "Theta PID Tuning"=w2133) -> ("Theta PID CONTROLLER"=w2154:T27)  [unwired: 8 in]
        n1296 = call <vilib>:"HolDrvCtrl_PackExecuteSP.vi"("LinearVel"=0.0, "Heading_Deg"=0.0, "Y"=1.29, "X"=13.34) -> ("HolExecuteSP"=w2152:cluster{"DesiredPose":T7, "LinearVel":dbl})  [unwired: 7 in]
        n1297 = call <vilib>:"HolDrvCtrl_PackControllers.vi"("thetaProfiledPID_CTRL"=w2154, "Y PID Tuning"=w2155, "X PID Tuning"=w2153) -> ("HOLONOMIC_CTRL_PACK_TUNING"=w2156:T31)  [unwired: 8 in]
        n1298 = call <vilib>:"HolDrvCtrl_Execute.vi"("HOLONOMIC_CTRL_PACK_TUNING"=w2156, "Tolerance"=T7 {"TRANSLATION"={"X"=0.2, "Y"=0.2}, "ROTATION"={"VALUE"=34.0, "COS"=99.0, "SIN"=34.0}}, "Enable"=TRUE, "angleRef"=w2130, "HolExecuteSP"=w2152, "currentPose"=w2131) -> ("AtReference"=w2119:bool, "calcChassisSpeed"=w2124:T14)  [unwired: 3 in, 1 out]
        n1299 = Unbundle By Name(w2124) -> ("vX"=w2123:dbl, "vY"=w2122:dbl, "vOmega"=w2121:dbl)
        n1300 = call "SWERVE_DRIVE_SET_SPEED_DEMAND.vi"("Drv Rotation Orentation Dmd"=w2116, "Drv Angular Vel Dmd"=w2121, "Drv Y Vel Dmd"=w2122, "Drv X Vel Dmd"=w2123) -> ()  [unwired: 8 in]
        n1301 = Wait (ms)(milliseconds to wait=u32 20) -> ()  [unwired: 1 out]
      }
      n1302 = while {
        tunnel: [w2076] -> _
        tunnel: w2072 -> [w2076]
        stop <- w2077 stop-if-true
        w2075 = -148.0 ("Angle_Degrees")
        w2094 = 1.0  # Kn
        w2097 = 1.0  # Kp
        w2106 = 0.0  # Ki
        w2107 = 0.0  # Kd
        w2108 = 9.9e+30  # MaximumIntegral
        w2109 = -9.9e+30  # MinimumIntegral
        w2092 = 1.0  # Kn
        w2095 = 5.0  # Kp
        w2098 = 0.0  # Ki
        w2099 = 0.0  # Kd
        w2100 = 9.9e+30  # MaximumIntegral
        w2101 = -9.9e+30  # MinimumIntegral
        w2093 = 1.0  # Kn
        w2096 = 5.0  # Kp
        w2102 = 0.0  # Ki
        w2103 = 0.0  # Kd
        w2104 = 9.9e+30  # MaximumIntegral
        w2105 = -9.9e+30  # MinimumIntegral
        # "Holonomic Drive\nController"
        # "Theta Controller"
        # "Y Controller"
        # "X Controller"
        n1303 = call "SWERVE_DRIVE_GET_MAX.vi"() -> ("Max Rotational Vel (Rad/Sec)"=w2074:dbl)  [unwired: 10 in, 1 out]
        n1304 = call <vilib>:"Rotation2d_CreateAngleDegrees.vi"("Angle_Degrees"=w2075) -> ("ROTATION"=w2088:T9)  [unwired: 10 in]
        n1305 = call "SWERVE_ODOM_ABS_FGV.vi"() -> ("out SWERVE_DRIVE_POSE_EST2"=w2090:T20)  [unwired: 10 in, 1 out]
        n1306 = call <vilib>:"PIDController_Pack_Tuning.vi"("MinimumIntegral"=w2101, "MaximumIntegral"=w2100, "Kn"=w2092, "Kd"=w2099, "Ki"=w2098, "Kp"=w2095) -> ("PID Tuning"=w2111:T26)  [unwired: 5 in]
        n1307 = call <vilib>:"PIDController_Pack_Tuning.vi"("MinimumIntegral"=w2105, "MaximumIntegral"=w2104, "Kn"=w2093, "Kd"=w2103, "Ki"=w2102, "Kp"=w2096) -> ("PID Tuning"=w2113:T26)  [unwired: 5 in]
        n1308 = call <vilib>:"PIDController_Pack_Tuning.vi"("MinimumIntegral"=w2109, "MaximumIntegral"=w2108, "Kn"=w2094, "Kd"=w2107, "Ki"=w2106, "Kp"=w2097) -> ("PID Tuning"=w2091:T26)  [unwired: 5 in]
        n1309 = Unbundle By Name(w2090) -> ("Swerve_Drive_Odom.POSE"=w2089:T7)
        n1310 = call <vilib>:"HolDrvCtrl_PackProfPID.vi"("Max Accel"=w2074, "Max Speed"=w2074, "Theta PID Tuning"=w2091) -> ("Theta PID CONTROLLER"=w2112:T27)  [unwired: 8 in]
        n1311 = call <vilib>:"HolDrvCtrl_PackExecuteSP.vi"("LinearVel"=0.0, "Heading_Deg"=0.0, "Y"=1.0, "X"=3.0) -> ("HolExecuteSP"=w2110:cluster{"DesiredPose":T7, "LinearVel":dbl})  [unwired: 7 in]
        n1312 = call <vilib>:"HolDrvCtrl_PackControllers.vi"("thetaProfiledPID_CTRL"=w2112, "Y PID Tuning"=w2113, "X PID Tuning"=w2111) -> ("HOLONOMIC_CTRL_PACK_TUNING"=w2114:T31)  [unwired: 8 in]
        n1313 = call <vilib>:"HolDrvCtrl_Execute.vi"("HOLONOMIC_CTRL_PACK_TUNING"=w2114, "Enable"=TRUE, "angleRef"=w2088, "HolExecuteSP"=w2110, "currentPose"=w2089) -> ("AtReference"=w2077:bool, "calcChassisSpeed"=w2082:T14)  [unwired: 4 in, 1 out]
        n1314 = Unbundle By Name(w2082) -> ("vX"=w2081:dbl, "vY"=w2080:dbl, "vOmega"=w2079:dbl)
        n1315 = call "SWERVE_DRIVE_SET_SPEED_DEMAND.vi"("Drv Rotation Orentation Dmd"=w2075, "Drv Angular Vel Dmd"=w2079, "Drv Y Vel Dmd"=w2080, "Drv X Vel Dmd"=w2081) -> ()  [unwired: 8 in]
        n1316 = Wait (ms)(milliseconds to wait=u32 20) -> ()  [unwired: 1 out]
      }
    }
    frame "Route 1 B" {
      w2164 = errorcluster {"status"=FALSE, "code"=0, "source"=""}  # Start Error Flow
      # "Trigger events when robot pose approx equals event pose\n(The two while loops below ends when the path above is ended)"
      n1317 = while {
        tunnel: w2164 -> [w2266]
        tunnel: [w2266] -> w2161
        i -> [w2264]
        stop <- w2263 stop-if-true
        w2260 = TRUE  # ABS Odo Initialize
        w2262 = 0.0 ("Drv X Vel Dmd")
        n1318 = Not Equal To 0?(x=w2264) -> (x != 0?=w2263:bool)
        n1319 = Wait (ms)(milliseconds to wait=u32 20) -> ()  [unwired: 1 out]
        n1320 = call-poly <vilib>:"NT Read Value.vi"("default value"="Path_Testing_1.path" ("Trajectory File Name"), "name"="Initial Path") -> ("value"=w2257:string)  [unwired: 7 in, 2 out]
        n1321 = call "SWERVE_DRIVE_MODULE_STATES_POSITIONS_FGV.vi"() -> ("out Current Module Positions"=w2254:T11[])  [unwired: 10 in, 1 out]
        n1322 = call "SWERVE_DRIVE_GET_GYRO.vi"() -> ("Gyro Heading Radians"=w2256:dbl)  [unwired: 11 in]
        n1323 = call "SWERVE_DRIVE_GET_GYRO.vi"() -> ("Gyro Heading Radians"=w2261:dbl)  [unwired: 11 in]
        n1324 = call <vilib>:"Rotation2d_CreateAngle.vi"("Angle"=w2256) -> ("ROTATION"=w2255:T9)  [unwired: 10 in]
        n1325 = call "SWERVE_DRIVE_SET_SPEED_DEMAND.vi"("Drv Rotation Orentation Dmd"=w2261, "Drv Angular Vel Dmd"=w2262, "Drv Y Vel Dmd"=w2262, "Drv X Vel Dmd"=w2262) -> ()  [unwired: 8 in]
        n1326 = call "SWERVE_TRAJECTORY_BEGIN.vi"("ABS Odo Initialize"=w2260, "gyroAngle"=w2255, "Module Positions"=w2254, "Trajectory File Name"=w2257) -> ()  [unwired: 8 in]
      }
      n1327 = while {
        tunnel: w2161 -> [w2239]
        tunnel: [w2239] -> w2162
        stop <- w2231 stop-if-true
        # "Shoot Preload"
        n1328 = Wait (ms)(milliseconds to wait=u32 20) -> ()  [unwired: 1 out]
        n1329 = call-poly <vilib>:"NT Read Value.vi"("default value"=0.0, "name"="Shooter/Speed_RPM Act") -> ("value"=w2234:dbl)  [unwired: 7 in, 2 out]
        n1330 = call-poly <vilib>:"NT Write Value.vi"("value"="Shoot Mode" ("default value"), "name"="Robot State") -> ()  [unwired: 9 in, 1 out]
        n1331 = Greater?(x=w2234, y=4000.0) -> (0:w2231:bool)
        n1332 = case shown="False" w2231 {
          frame False {
            n1333 = call-poly <vilib>:"NT Write Value.vi"("value"="FromIntake" ("default value"), "name"="Intake/Trigger Status") -> ()  [unwired: 9 in, 1 out]
          }
          frame True {
            n1334 = call-poly <vilib>:"NT Write Value.vi"("value"="ToShooter" ("default value"), "name"="Intake/Trigger Status") -> ()  [unwired: 9 in, 1 out]
          }
        }
        n1335 = call-poly <vilib>:"NT Write Value.vi"("value"=59.0 ("Fixed 3.5 m_Deg"), "name"="Shooter/Angle_Deg Dmd") -> ()  [unwired: 9 in, 1 out]
      }
      n1336 = while {
        tunnel: w2162 -> [w2228]
        tunnel: [w2228] -> w2159
        i -> [w2226]
        stop <- w2225 stop-if-true
        # "Wait until shooting finishes"
        n1337 = Equal To 0?(x=w2226) -> (x = 0?=w2225:bool)
        n1338 = Wait (ms)(milliseconds to wait=u32 1500) -> ()  [unwired: 1 out]
      }
      n1339 = while {
        tunnel: w2159 -> [w2287]
        tunnel: [w2287] -> w2163
        i -> [w2285]
        stop <- w2267 stop-if-true
        w2269 = TRUE  # ABS_Traj ?
        w2277 = TRUE  # EnableClosedLoop
        w2275 = FALSE  # Reverse
        w2279 = TRUE  # Follow Orientation
        n1340 = Equal To 0?(x=w2285) -> (x = 0?=w2276:bool)
        n1341 = call "SWERVE_DRIVE_GET_SPEED_DEMAND.vi"() -> ("Drv Rotation Orentation Dmd"=w2284:dbl)  [unwired: 8 in, 3 out]
        n1342 = call "SWERVE_DRIVE_GET_GYRO.vi"() -> ("Gyro Heading Radians"=w2274:dbl)  [unwired: 11 in]
        n1343 = Wait Until Next ms Multiple(millisecond multiple=u32 20 ("milliseconds to wait")) -> ()  [unwired: 1 out]
        n1344 = call "SWERVE_TRAJECTORY_EXECUTE.vi"("EnableClosedLoop"=w2277, "ABS_Traj ?"=w2269, "Init"=w2276, "Reverse"=w2275, "Follow Orientation"=w2279, "Gyro Heading\nRAD"=w2274) -> ("AtReference"=w2270:bool, "OutputTRAJ_STATE"=w2271:T12, "Error and Corr"=w2272:T13, "Chassis Velocity Target"=w2278:T14, "Orientation Target"=w2273:dbl)  [unwired: 1 in]
        n1345 = Select(t=w2274, s=w2279, f=w2284) -> (s? t:f=w2280:dbl)
        n1346 = call "SWERVE_TRAJECTORY_SET_CLOSED_LOOP.vi"("AUTO_CLOSED_LOOP"=w2277) -> ()  [unwired: 11 in]
        n1347 = call "SWERVE_TRAJECTORY_UPDATE_DIAG_INFO.vi"("AtReference"=w2270, "OutputTRAJ_STATE"=w2271, "Error and Corr"=w2272, "Orientation Target"=w2273) -> ()  [unwired: 8 in]
        n1348 = global read "SWERVE_TRAJECTORY_GLOBALS.vi" "Traj_Total_Time"() -> (w2288:dbl)
        n1349 = Unbundle By Name(w2271) -> ("TimeSeconds"=w2286:dbl)
        n1350 = Unbundle By Name(w2278) -> ("vX"=w2283:dbl, "vY"=w2282:dbl, "vOmega"=w2281:dbl)
        n1351 = Equal?(x=w2286, y=w2288) -> (x = y?=w2267:bool)
        n1352 = call "SWERVE_DRIVE_SET_SPEED_DEMAND.vi"("Drv Rotation Orentation Dmd"=w2280, "Drv Angular Vel Dmd"=w2281, "Drv Y Vel Dmd"=w2282, "Drv X Vel Dmd"=w2283) -> ()  [unwired: 8 in]
        n1353 = call-poly <vilib>:"NT Write Value.vi"("value"=w2267, "name"="Auto/Path End") -> ()  [unwired: 9 in, 1 out]
      }
      n1354 = while {
        tunnel: w2159 -> [w2195]
        tunnel: [w2195] -> _
        tunnel: cluster{"X":dbl, "Y":dbl, "Event":string}[] [{"X"=1.55, "Y"=6.87, "Event"="Intake"}, {"X"=13.51, "Y"=7.06, "Event"="Shoot 1"}, {"X"=12.98, "Y"=7.13, "Event"="Trigger"}, {"X"=11.64, "Y"=7.32, "Event"="Intake"}, {"X"=9.17, "Y"=7.36, "Event"="Shoot 2"}] -> [w2191]
        stop <- w2189 stop-if-true
        n1355 = call "SWERVE_ODOM_ABS_FGV.vi"() -> ("out SWERVE_DRIVE_ODOMETRY"=w2187:T25)  [unwired: 10 in, 1 out]
        n1356 = Unbundle By Name(w2187) -> ("POSE.TRANSLATION.X"=w2194:dbl, "POSE.TRANSLATION.Y"=w2193:dbl)
        n1357 = call-poly <vilib>:"NT Read Value.vi"("default value"=FALSE, "name"="Auto/Path End") -> ("value"=w2189:bool)  [unwired: 7 in, 2 out]
        n1358 = Build Array(w2194, w2193) -> (w2192:dbl[])
        n1359 = for {
          tunnel: w2192 -> [w2203]
          tunnel: w2191 -> [w2202] mode=indexing
          n1360 = Unbundle(w2202) -> ("X"=w2201:dbl, "Y"=w2200:dbl, "Event"=w2196:string)
          n1361 = Build Array(w2201, w2200) -> (w2199:dbl[])
          n1362 = for {
            tunnel: w2203 -> [w2209] mode=indexing
            tunnel: [w2207] -> w2198 mode=indexing
            tunnel: w2199 -> [w2206] mode=indexing
            n1363 = call <vilib>:"Util_ApproxEquals.vi"("Tolerance"=0.15, "Value 2"=w2206, "Value 1"=w2209) -> ("ApproxEquals"=w2207:bool)  [unwired: 8 in]
          }
          n1364 = And Array Elements(Boolean array=w2198) -> (logical AND=w2197:bool)
          n1365 = case shown="True" w2197 {
            tunnel: w2196 -> [_ w2204]
            frame False {
            }
            frame True {
              n1366 = call-poly <vilib>:"NT Write Value.vi"("value"=w2204, "name"="Auto State") -> ()  [unwired: 9 in, 1 out]
            }
          }
        }
      }
      n1367 = while {
        tunnel: w2159 -> [w2213]
        tunnel: [w2213] -> _
        stop <- w2211 stop-if-true
        n1368 = call-poly <vilib>:"NT Read Value.vi"("default value"="None", "name"="Auto State") -> ("value"=w2215:string)  [unwired: 7 in, 2 out]
        n1369 = case shown="\"Trigger\"" w2215 {
          frame "None", Default {
          }
          frame "Shoot 1" {
            n1370 = call-poly <vilib>:"NT Write Value.vi"("value"="Shoot Mode" ("default value"), "name"="Robot State") -> ()  [unwired: 9 in, 1 out]
          }
          frame "Shoot 2" {
            n1371 = call-poly <vilib>:"NT Write Value.vi"("value"="Shoot Mode" ("default value"), "name"="Robot State") -> ()  [unwired: 9 in, 1 out]
          }
          frame "Intake" {
            n1372 = call-poly <vilib>:"NT Write Value.vi"("value"="Intake Mode" ("default value"), "name"="Robot State") -> ()  [unwired: 9 in, 1 out]
          }
          frame "Trigger" {
            n1373 = call-poly <vilib>:"NT Write Value.vi"("value"="ToShooter" ("default value"), "name"="Intake/Trigger Status") -> ()  [unwired: 9 in, 1 out]
          }
        }
        n1374 = call-poly <vilib>:"NT Read Value.vi"("default value"=FALSE, "name"="Auto/Path End") -> ("value"=w2211:bool)  [unwired: 7 in, 2 out]
      }
      n1375 = while {
        tunnel: w2163 -> [w2253]
        tunnel: [w2253] -> w2158
        i -> [w2251]
        stop <- w2250 stop-if-true
        w2249 = 0.0 ("Drv X Vel Dmd")
        n1376 = Not Equal To 0?(x=w2251) -> (x != 0?=w2250:bool)
        n1377 = Wait (ms)(milliseconds to wait=u32 20) -> ()  [unwired: 1 out]
        n1378 = call "SWERVE_DRIVE_MODULE_STATES_POSITIONS_FGV.vi"() -> ("out Current Module Positions"=w2245:T11[])  [unwired: 10 in, 1 out]
        n1379 = call "SWERVE_DRIVE_GET_GYRO.vi"() -> ("Gyro Heading Radians"=w2247:dbl)  [unwired: 11 in]
        n1380 = call "SWERVE_DRIVE_GET_GYRO.vi"() -> ("Gyro Heading Radians"=w2248:dbl)  [unwired: 11 in]
        n1381 = call <vilib>:"Rotation2d_CreateAngle.vi"("Angle"=w2247) -> ("ROTATION"=w2246:T9)  [unwired: 10 in]
        n1382 = call "SWERVE_DRIVE_SET_SPEED_DEMAND.vi"("Drv Rotation Orentation Dmd"=w2248, "Drv Angular Vel Dmd"=w2249, "Drv Y Vel Dmd"=w2249, "Drv X Vel Dmd"=w2249) -> ()  [unwired: 8 in]
        n1383 = call "SWERVE_TRAJECTORY_BEGIN.vi"("gyroAngle"=w2246, "Module Positions"=w2245, "Trajectory File Name"="Path Demo.wpilib.csv") -> ()  [unwired: 9 in]
      }
      n1384 = while {
        tunnel: [w2186] -> w2157
        tunnel: w2158 -> [w2186]
        i -> [w2182]
        stop <- w2181 stop-if-true
        # "TBD: GP 1 shooting angle dmd"
        # "Shooter angle to correct angle"
        n1385 = Equal To 0?(x=w2182) -> (x = 0?=w2181:bool)
        n1386 = Wait (ms)(milliseconds to wait=u32 20) -> ()  [unwired: 1 out]
        n1387 = call-poly <vilib>:"NT Write Value.vi"("value"=32.0 ("Fixed 3.5 m_Deg"), "name"="Shooter/Angle_Deg Dmd") -> ()  [unwired: 9 in, 1 out]
        n1388 = call-poly <vilib>:"NT Write Value.vi"("value"="Shoot Mode" ("default value"), "name"="Robot State") -> ()  [unwired: 9 in, 1 out]
      }
      n1389 = while {
        tunnel: w2157 -> [w2176]
        tunnel: [w2176] -> _
        stop <- FALSE stop-if-true
        w2172 = 2.0  # Tolerance
        w2166 = 0.0 ("vX")
        # "Turn robot to face speaker apriltag and shoot GP 1"
        n1390 = Wait (ms)(milliseconds to wait=u32 20) -> ()  [unwired: 1 out]
        n1391 = call-poly <vilib>:"NT Read Value.vi"("name"="/limelight/tx") -> ("value"=w2174:dbl)  [unwired: 8 in, 2 out]
        n1392 = call "SWERVE_DRIVE_GET_GYRO.vi"() -> ("Gyro Heading Radians"=w2167:dbl)  [unwired: 11 in]
        n1393 = call <vilib>:"Conv_Deg_Radians.vi"("Degress"=w2174) -> ("Radians"=w2173:dbl)  [unwired: 10 in]
        n1394 = Subtract(x=w2167, y=w2173) -> (x-y=w2165:dbl)
        n1395 = call <vilib>:"Util_ApproxEquals.vi"("Tolerance"=w2172, "Value 2"=w2173, "Value 1"=0.0) -> ("ApproxEquals"=w2170:bool)  [unwired: 8 in]
        n1396 = call "SWERVE_DRIVE_SET_SPEED_DEMAND.vi"("Drv Rotation Orentation Dmd"=w2165, "Drv Angular Vel Dmd"=w2166, "Drv Y Vel Dmd"=w2166, "Drv X Vel Dmd"=w2166) -> ()  [unwired: 8 in]
        n1397 = case shown="True" w2170 {
          frame False {
          }
          frame True {
            n1398 = call-poly <vilib>:"NT Write Value.vi"("value"="ToShooter" ("default value"), "name"="Intake/Trigger Status") -> ()  [unwired: 9 in, 1 out]
          }
        }
      }
    }
    frame "Route 1 R" {
      w2297 = errorcluster {"status"=FALSE, "code"=0, "source"=""}  # Start Error Flow
      # "Trigger events when robot pose approx equals event pose\n(The two while loops below ends when the path above is ended)"
      n1399 = while {
        tunnel: w2297 -> [w2403]
        tunnel: [w2403] -> w2294
        i -> [w2401]
        stop <- w2400 stop-if-true
        w2397 = TRUE  # ABS Odo Initialize
        w2399 = 0.0 ("Drv X Vel Dmd")
        n1400 = Not Equal To 0?(x=w2401) -> (x != 0?=w2400:bool)
        n1401 = Wait (ms)(milliseconds to wait=u32 20) -> ()  [unwired: 1 out]
        n1402 = call-poly <vilib>:"NT Read Value.vi"("default value"="Path_Testing_1.path" ("Trajectory File Name"), "name"="Initial Path") -> ("value"=w2394:string)  [unwired: 7 in, 2 out]
        n1403 = call "SWERVE_DRIVE_MODULE_STATES_POSITIONS_FGV.vi"() -> ("out Current Module Positions"=w2391:T11[])  [unwired: 10 in, 1 out]
        n1404 = call "SWERVE_DRIVE_GET_GYRO.vi"() -> ("Gyro Heading Radians"=w2393:dbl)  [unwired: 11 in]
        n1405 = call "SWERVE_DRIVE_GET_GYRO.vi"() -> ("Gyro Heading Radians"=w2398:dbl)  [unwired: 11 in]
        n1406 = call <vilib>:"Rotation2d_CreateAngle.vi"("Angle"=w2393) -> ("ROTATION"=w2392:T9)  [unwired: 10 in]
        n1407 = call "SWERVE_DRIVE_SET_SPEED_DEMAND.vi"("Drv Rotation Orentation Dmd"=w2398, "Drv Angular Vel Dmd"=w2399, "Drv Y Vel Dmd"=w2399, "Drv X Vel Dmd"=w2399) -> ()  [unwired: 8 in]
        n1408 = call "SWERVE_TRAJECTORY_BEGIN.vi"("ABS Odo Initialize"=w2397, "gyroAngle"=w2392, "Module Positions"=w2391, "Trajectory File Name"=w2394) -> ()  [unwired: 8 in]
      }
      n1409 = while {
        tunnel: w2294 -> [w2376]
        tunnel: [w2376] -> w2295
        stop <- w2368 stop-if-true
        # "Shoot Preload"
        n1410 = Wait (ms)(milliseconds to wait=u32 20) -> ()  [unwired: 1 out]
        n1411 = call-poly <vilib>:"NT Read Value.vi"("default value"=0.0, "name"="Shooter/Speed_RPM Act") -> ("value"=w2371:dbl)  [unwired: 7 in, 2 out]
        n1412 = call-poly <vilib>:"NT Write Value.vi"("value"="Shoot Mode" ("default value"), "name"="Robot State") -> ()  [unwired: 9 in, 1 out]
        n1413 = Greater?(x=w2371, y=4000.0) -> (0:w2368:bool)
        n1414 = case shown="False" w2368 {
          frame False {
            n1415 = call-poly <vilib>:"NT Write Value.vi"("value"="FromIntake" ("default value"), "name"="Intake/Trigger Status") -> ()  [unwired: 9 in, 1 out]
          }
          frame True {
            n1416 = call-poly <vilib>:"NT Write Value.vi"("value"="ToShooter" ("default value"), "name"="Intake/Trigger Status") -> ()  [unwired: 9 in, 1 out]
          }
        }
        n1417 = call-poly <vilib>:"NT Write Value.vi"("value"=59.0 ("Fixed 3.5 m_Deg"), "name"="Shooter/Angle_Deg Dmd") -> ()  [unwired: 9 in, 1 out]
      }
      n1418 = while {
        tunnel: w2295 -> [w2365]
        tunnel: [w2365] -> w2293
        i -> [w2363]
        stop <- w2362 stop-if-true
        # "Wait until shooting finishes"
        n1419 = Equal To 0?(x=w2363) -> (x = 0?=w2362:bool)
        n1420 = Wait (ms)(milliseconds to wait=u32 1500) -> ()  [unwired: 1 out]
      }
      n1421 = while {
        tunnel: w2293 -> [w2424]
        tunnel: [w2424] -> w2296
        i -> [w2422]
        stop <- w2404 stop-if-true
        w2406 = TRUE  # ABS_Traj ?
        w2414 = TRUE  # EnableClosedLoop
        w2412 = FALSE  # Reverse
        w2416 = TRUE  # Follow Orientation
        n1422 = Equal To 0?(x=w2422) -> (x = 0?=w2413:bool)
        n1423 = call "SWERVE_DRIVE_GET_SPEED_DEMAND.vi"() -> ("Drv Rotation Orentation Dmd"=w2421:dbl)  [unwired: 8 in, 3 out]
        n1424 = call "SWERVE_DRIVE_GET_GYRO.vi"() -> ("Gyro Heading Radians"=w2411:dbl)  [unwired: 11 in]
        n1425 = Wait Until Next ms Multiple(millisecond multiple=u32 20 ("milliseconds to wait")) -> ()  [unwired: 1 out]
        n1426 = call "SWERVE_TRAJECTORY_EXECUTE.vi"("EnableClosedLoop"=w2414, "ABS_Traj ?"=w2406, "Init"=w2413, "Reverse"=w2412, "Follow Orientation"=w2416, "Gyro Heading\nRAD"=w2411) -> ("AtReference"=w2407:bool, "OutputTRAJ_STATE"=w2408:T12, "Error and Corr"=w2409:T13, "Chassis Velocity Target"=w2415:T14, "Orientation Target"=w2410:dbl)  [unwired: 1 in]
        n1427 = Select(t=w2411, s=w2416, f=w2421) -> (s? t:f=w2417:dbl)
        n1428 = call "SWERVE_TRAJECTORY_SET_CLOSED_LOOP.vi"("AUTO_CLOSED_LOOP"=w2414) -> ()  [unwired: 11 in]
        n1429 = call "SWERVE_TRAJECTORY_UPDATE_DIAG_INFO.vi"("AtReference"=w2407, "OutputTRAJ_STATE"=w2408, "Error and Corr"=w2409, "Orientation Target"=w2410) -> ()  [unwired: 8 in]
        n1430 = global read "SWERVE_TRAJECTORY_GLOBALS.vi" "Traj_Total_Time"() -> (w2425:dbl)
        n1431 = Unbundle By Name(w2408) -> ("TimeSeconds"=w2423:dbl)
        n1432 = Unbundle By Name(w2415) -> ("vX"=w2420:dbl, "vY"=w2419:dbl, "vOmega"=w2418:dbl)
        n1433 = Equal?(x=w2423, y=w2425) -> (x = y?=w2404:bool)
        n1434 = call "SWERVE_DRIVE_SET_SPEED_DEMAND.vi"("Drv Rotation Orentation Dmd"=w2417, "Drv Angular Vel Dmd"=w2418, "Drv Y Vel Dmd"=w2419, "Drv X Vel Dmd"=w2420) -> ()  [unwired: 8 in]
        n1435 = call-poly <vilib>:"NT Write Value.vi"("value"=w2404, "name"="Auto/Path End") -> ()  [unwired: 9 in, 1 out]
      }
      n1436 = while {
        tunnel: w2293 -> [w2328]
        tunnel: [w2328] -> _
        tunnel: cluster{"X":dbl, "Y":dbl, "Event":string}[] [{"X"=14.99, "Y"=6.87, "Event"="Intake"}, {"X"=13.51, "Y"=7.06, "Event"="Shoot 1"}, {"X"=12.98, "Y"=7.13, "Event"="Trigger"}, {"X"=11.64, "Y"=7.32, "Event"="Intake"}, {"X"=9.17, "Y"=7.36, "Event"="Shoot 2"}] -> [w2324]
        stop <- w2322 stop-if-true
        n1437 = call "SWERVE_ODOM_ABS_FGV.vi"() -> ("out SWERVE_DRIVE_ODOMETRY"=w2320:T25)  [unwired: 10 in, 1 out]
        n1438 = Unbundle By Name(w2320) -> ("POSE.TRANSLATION.X"=w2327:dbl, "POSE.TRANSLATION.Y"=w2326:dbl)
        n1439 = call-poly <vilib>:"NT Read Value.vi"("default value"=FALSE, "name"="Auto/Path End") -> ("value"=w2322:bool)  [unwired: 7 in, 2 out]
        n1440 = Build Array(w2327, w2326) -> (w2325:dbl[])
        n1441 = for {
          tunnel: w2325 -> [w2336]
          tunnel: w2324 -> [w2335] mode=indexing
          n1442 = Unbundle(w2335) -> ("X"=w2334:dbl, "Y"=w2333:dbl, "Event"=w2329:string)
          n1443 = Build Array(w2334, w2333) -> (w2332:dbl[])
          n1444 = for {
            tunnel: w2336 -> [w2342] mode=indexing
            tunnel: [w2340] -> w2331 mode=indexing
            tunnel: w2332 -> [w2339] mode=indexing
            n1445 = call <vilib>:"Util_ApproxEquals.vi"("Tolerance"=0.1, "Value 2"=w2339, "Value 1"=w2342) -> ("ApproxEquals"=w2340:bool)  [unwired: 8 in]
          }
          n1446 = And Array Elements(Boolean array=w2331) -> (logical AND=w2330:bool)
          n1447 = case shown="True" w2330 {
            tunnel: w2329 -> [_ w2337]
            frame False {
            }
            frame True {
              n1448 = call-poly <vilib>:"NT Write Value.vi"("value"=w2337, "name"="Auto State") -> ()  [unwired: 9 in, 1 out]
            }
          }
        }
      }
      n1449 = while {
        tunnel: w2293 -> [w2346]
        tunnel: [w2346] -> _
        stop <- w2344 stop-if-true
        n1450 = call-poly <vilib>:"NT Read Value.vi"("default value"="None", "name"="Auto State") -> ("value"=w2348:string)  [unwired: 7 in, 2 out]
        n1451 = case shown="\"Intake\"" w2348 {
          frame "None", Default {
          }
          frame "Shoot 1" {
            n1452 = call-poly <vilib>:"NT Write Value.vi"("value"="Shoot Mode" ("default value"), "name"="Robot State") -> ()  [unwired: 9 in, 1 out]
            n1453 = call-poly <vilib>:"NT Write Value.vi"("value"=35.0 ("Fixed 3.5 m_Deg"), "name"="Shooter/Angle_Deg Dmd") -> ()  [unwired: 9 in, 1 out]
          }
          frame "Shoot 2" {
            n1454 = call-poly <vilib>:"NT Write Value.vi"("value"="Shoot Mode" ("default value"), "name"="Robot State") -> ()  [unwired: 9 in, 1 out]
            n1455 = call-poly <vilib>:"NT Write Value.vi"("value"=33.0 ("Fixed 3.5 m_Deg"), "name"="Shooter/Angle_Deg Dmd") -> ()  [unwired: 9 in, 1 out]
          }
          frame "Intake" {
            n1456 = call-poly <vilib>:"NT Write Value.vi"("value"="Intake Mode" ("default value"), "name"="Robot State") -> ()  [unwired: 9 in, 1 out]
          }
          frame "Trigger" {
            n1457 = call-poly <vilib>:"NT Write Value.vi"("value"="ToShooter" ("default value"), "name"="Intake/Trigger Status") -> ()  [unwired: 9 in, 1 out]
          }
        }
        n1458 = call-poly <vilib>:"NT Read Value.vi"("default value"=FALSE, "name"="Auto/Path End") -> ("value"=w2344:bool)  [unwired: 7 in, 2 out]
      }
      n1459 = while {
        tunnel: w2296 -> [w2390]
        tunnel: [w2390] -> w2292
        i -> [w2388]
        stop <- w2387 stop-if-true
        w2386 = 0.0 ("Drv X Vel Dmd")
        n1460 = Not Equal To 0?(x=w2388) -> (x != 0?=w2387:bool)
        n1461 = Wait (ms)(milliseconds to wait=u32 20) -> ()  [unwired: 1 out]
        n1462 = call "SWERVE_DRIVE_MODULE_STATES_POSITIONS_FGV.vi"() -> ("out Current Module Positions"=w2382:T11[])  [unwired: 10 in, 1 out]
        n1463 = call "SWERVE_DRIVE_GET_GYRO.vi"() -> ("Gyro Heading Radians"=w2384:dbl)  [unwired: 11 in]
        n1464 = call "SWERVE_DRIVE_GET_GYRO.vi"() -> ("Gyro Heading Radians"=w2385:dbl)  [unwired: 11 in]
        n1465 = call <vilib>:"Rotation2d_CreateAngle.vi"("Angle"=w2384) -> ("ROTATION"=w2383:T9)  [unwired: 10 in]
        n1466 = call "SWERVE_DRIVE_SET_SPEED_DEMAND.vi"("Drv Rotation Orentation Dmd"=w2385, "Drv Angular Vel Dmd"=w2386, "Drv Y Vel Dmd"=w2386, "Drv X Vel Dmd"=w2386) -> ()  [unwired: 8 in]
        n1467 = call "SWERVE_TRAJECTORY_BEGIN.vi"("gyroAngle"=w2383, "Module Positions"=w2382, "Trajectory File Name"="Path Demo.wpilib.csv") -> ()  [unwired: 9 in]
      }
      n1468 = while {
        tunnel: [w2319] -> w2291
        tunnel: w2292 -> [w2319]
        i -> [w2315]
        stop <- w2314 stop-if-true
        # "TBD: GP 1 shooting angle dmd"
        # "Shooter angle to correct angle"
        n1469 = Equal To 0?(x=w2315) -> (x = 0?=w2314:bool)
        n1470 = Wait (ms)(milliseconds to wait=u32 20) -> ()  [unwired: 1 out]
        n1471 = call-poly <vilib>:"NT Write Value.vi"("value"=32.0 ("Fixed 3.5 m_Deg"), "name"="Shooter/Angle_Deg Dmd") -> ()  [unwired: 9 in, 1 out]
        n1472 = call-poly <vilib>:"NT Write Value.vi"("value"="Shoot Mode" ("default value"), "name"="Robot State") -> ()  [unwired: 9 in, 1 out]
      }
      n1473 = while {
        tunnel: w2291 -> [w2309]
        tunnel: [w2309] -> _
        stop <- FALSE stop-if-true
        w2305 = 2.0  # Tolerance
        w2299 = 0.0 ("vX")
        # "Turn robot to face speaker apriltag and shoot GP 1"
        n1474 = Wait (ms)(milliseconds to wait=u32 20) -> ()  [unwired: 1 out]
        n1475 = call-poly <vilib>:"NT Read Value.vi"("name"="/limelight/tx") -> ("value"=w2307:dbl)  [unwired: 8 in, 2 out]
        n1476 = call "SWERVE_DRIVE_GET_GYRO.vi"() -> ("Gyro Heading Radians"=w2300:dbl)  [unwired: 11 in]
        n1477 = call <vilib>:"Conv_Deg_Radians.vi"("Degress"=w2307) -> ("Radians"=w2306:dbl)  [unwired: 10 in]
        n1478 = Subtract(x=w2300, y=w2306) -> (x-y=w2298:dbl)
        n1479 = call <vilib>:"Util_ApproxEquals.vi"("Tolerance"=w2305, "Value 2"=w2306, "Value 1"=0.0) -> ("ApproxEquals"=w2303:bool)  [unwired: 8 in]
        n1480 = call "SWERVE_DRIVE_SET_SPEED_DEMAND.vi"("Drv Rotation Orentation Dmd"=w2298, "Drv Angular Vel Dmd"=w2299, "Drv Y Vel Dmd"=w2299, "Drv X Vel Dmd"=w2299) -> ()  [unwired: 8 in]
        n1481 = case shown="True" w2303 {
          frame False {
          }
          frame True {
            n1482 = call-poly <vilib>:"NT Write Value.vi"("value"="ToShooter" ("default value"), "name"="Intake/Trigger Status") -> ()  [unwired: 9 in, 1 out]
          }
        }
      }
    }
    frame "Path Demo" {
      w2429 = errorcluster {"status"=FALSE, "code"=0, "source"=""}  # Start Error Flow
      n1483 = while {
        tunnel: w2429 -> [w2452]
        tunnel: [w2452] -> w2428
        i -> [w2450]
        stop <- w2449 stop-if-true
        w2446 = TRUE  # ABS Odo Initialize
        w2448 = 0.0 ("Drv X Vel Dmd")
        n1484 = Not Equal To 0?(x=w2450) -> (x != 0?=w2449:bool)
        n1485 = Wait (ms)(milliseconds to wait=u32 20) -> ()  [unwired: 1 out]
        n1486 = call-poly <vilib>:"NT Read Value.vi"("default value"="Path_Testing_1.path" ("Trajectory File Name"), "name"="Initial Path") -> ("value"=w2443:string)  [unwired: 7 in, 2 out]
        n1487 = call "SWERVE_DRIVE_MODULE_STATES_POSITIONS_FGV.vi"() -> ("out Current Module Positions"=w2440:T11[])  [unwired: 10 in, 1 out]
        n1488 = call "SWERVE_DRIVE_GET_GYRO.vi"() -> ("Gyro Heading Radians"=w2442:dbl)  [unwired: 11 in]
        n1489 = call "SWERVE_DRIVE_GET_GYRO.vi"() -> ("Gyro Heading Radians"=w2447:dbl)  [unwired: 11 in]
        n1490 = call <vilib>:"Rotation2d_CreateAngle.vi"("Angle"=w2442) -> ("ROTATION"=w2441:T9)  [unwired: 10 in]
        n1491 = call "SWERVE_DRIVE_SET_SPEED_DEMAND.vi"("Drv Rotation Orentation Dmd"=w2447, "Drv Angular Vel Dmd"=w2448, "Drv Y Vel Dmd"=w2448, "Drv X Vel Dmd"=w2448) -> ()  [unwired: 8 in]
        n1492 = call "SWERVE_TRAJECTORY_BEGIN.vi"("ABS Odo Initialize"=w2446, "gyroAngle"=w2441, "Module Positions"=w2440, "Trajectory File Name"=w2443) -> ()  [unwired: 8 in]
      }
      n1493 = while {
        tunnel: w2428 -> [w2472]
        tunnel: [w2472] -> w2427
        i -> [w2470]
        stop <- w2469 stop-if-true
        w2453 = TRUE  # ABS_Traj ?
        w2461 = TRUE  # EnableClosedLoop
        w2459 = FALSE  # Reverse
        w2463 = TRUE  # Follow Orientation
        n1494 = Equal To 0?(x=w2470) -> (x = 0?=w2460:bool)
        n1495 = call "SWERVE_DRIVE_GET_SPEED_DEMAND.vi"() -> ("Drv Rotation Orentation Dmd"=w2468:dbl)  [unwired: 8 in, 3 out]
        n1496 = call "SWERVE_DRIVE_GET_GYRO.vi"() -> ("Gyro Heading Radians"=w2458:dbl)  [unwired: 11 in]
        n1497 = Wait Until Next ms Multiple(millisecond multiple=u32 20 ("milliseconds to wait")) -> ()  [unwired: 1 out]
        n1498 = call "SWERVE_TRAJECTORY_EXECUTE.vi"("EnableClosedLoop"=w2461, "ABS_Traj ?"=w2453, "Init"=w2460, "Reverse"=w2459, "Follow Orientation"=w2463, "Gyro Heading\nRAD"=w2458) -> ("AtReference"=w2454:bool, "OutputTRAJ_STATE"=w2455:T12, "Error and Corr"=w2456:T13, "Chassis Velocity Target"=w2462:T14, "Orientation Target"=w2457:dbl)  [unwired: 1 in]
        n1499 = Select(t=w2458, s=w2463, f=w2468) -> (s? t:f=w2464:dbl)
        n1500 = call "SWERVE_TRAJECTORY_SET_CLOSED_LOOP.vi"("AUTO_CLOSED_LOOP"=w2461) -> ()  [unwired: 11 in]
        n1501 = call "SWERVE_TRAJECTORY_UPDATE_DIAG_INFO.vi"("AtReference"=w2454, "OutputTRAJ_STATE"=w2455, "Error and Corr"=w2456, "Orientation Target"=w2457) -> ()  [unwired: 8 in]
        n1502 = global read "SWERVE_TRAJECTORY_GLOBALS.vi" "Traj_Total_Time"() -> (w2473:dbl)
        n1503 = Unbundle By Name(w2455) -> ("TimeSeconds"=w2471:dbl)
        n1504 = Unbundle By Name(w2462) -> ("vX"=w2467:dbl, "vY"=w2466:dbl, "vOmega"=w2465:dbl)
        n1505 = Equal?(x=w2471, y=w2473) -> (x = y?=w2469:bool)
        n1506 = call "SWERVE_DRIVE_SET_SPEED_DEMAND.vi"("Drv Rotation Orentation Dmd"=w2464, "Drv Angular Vel Dmd"=w2465, "Drv Y Vel Dmd"=w2466, "Drv X Vel Dmd"=w2467) -> ()  [unwired: 8 in]
      }
      n1507 = while {
        tunnel: w2427 -> [w2439]
        tunnel: [w2439] -> _
        i -> [w2437]
        stop <- w2436 stop-if-true
        w2435 = 0.0 ("Drv X Vel Dmd")
        n1508 = Not Equal To 0?(x=w2437) -> (x != 0?=w2436:bool)
        n1509 = Wait (ms)(milliseconds to wait=u32 20) -> ()  [unwired: 1 out]
        n1510 = call "SWERVE_DRIVE_MODULE_STATES_POSITIONS_FGV.vi"() -> ("out Current Module Positions"=w2431:T11[])  [unwired: 10 in, 1 out]
        n1511 = call "SWERVE_DRIVE_GET_GYRO.vi"() -> ("Gyro Heading Radians"=w2433:dbl)  [unwired: 11 in]
        n1512 = call "SWERVE_DRIVE_GET_GYRO.vi"() -> ("Gyro Heading Radians"=w2434:dbl)  [unwired: 11 in]
        n1513 = call <vilib>:"Rotation2d_CreateAngle.vi"("Angle"=w2433) -> ("ROTATION"=w2432:T9)  [unwired: 10 in]
        n1514 = call "SWERVE_DRIVE_SET_SPEED_DEMAND.vi"("Drv Rotation Orentation Dmd"=w2434, "Drv Angular Vel Dmd"=w2435, "Drv Y Vel Dmd"=w2435, "Drv X Vel Dmd"=w2435) -> ()  [unwired: 8 in]
        n1515 = call "SWERVE_TRAJECTORY_BEGIN.vi"("gyroAngle"=w2432, "Module Positions"=w2431, "Trajectory File Name"="Path Demo.wpilib.csv") -> ()  [unwired: 9 in]
      }
    }
    frame "Route B2 R old" {
      w2487 = errorcluster {"status"=FALSE, "code"=0, "source"=""}  # Start Error Flow
      # "Shoot Preload"
      n1516 = while {
        tunnel: w2487 -> [w2629]
        tunnel: [w2629] -> w2483
        i -> [w2627]
        stop <- w2626 stop-if-true
        w2623 = TRUE  # ABS Odo Initialize
        w2625 = 0.0 ("Drv X Vel Dmd")
        n1517 = Not Equal To 0?(x=w2627) -> (x != 0?=w2626:bool)
        n1518 = Wait (ms)(milliseconds to wait=u32 20) -> ()  [unwired: 1 out]
        n1519 = call-poly <vilib>:"NT Read Value.vi"("default value"="Path_Testing_1.path" ("Trajectory File Name"), "name"="Initial Path") -> ("value"=w2620:string)  [unwired: 7 in, 2 out]
        n1520 = call "SWERVE_DRIVE_MODULE_STATES_POSITIONS_FGV.vi"() -> ("out Current Module Positions"=w2617:T11[])  [unwired: 10 in, 1 out]
        n1521 = call "SWERVE_DRIVE_GET_GYRO.vi"() -> ("Gyro Heading Radians"=w2619:dbl)  [unwired: 11 in]
        n1522 = call "SWERVE_DRIVE_GET_GYRO.vi"() -> ("Gyro Heading Radians"=w2624:dbl)  [unwired: 11 in]
        n1523 = call <vilib>:"Rotation2d_CreateAngle.vi"("Angle"=w2619) -> ("ROTATION"=w2618:T9)  [unwired: 10 in]
        n1524 = call "SWERVE_DRIVE_SET_SPEED_DEMAND.vi"("Drv Rotation Orentation Dmd"=w2624, "Drv Angular Vel Dmd"=w2625, "Drv Y Vel Dmd"=w2625, "Drv X Vel Dmd"=w2625) -> ()  [unwired: 8 in]
        n1525 = call "SWERVE_TRAJECTORY_BEGIN.vi"("ABS Odo Initialize"=w2623, "gyroAngle"=w2618, "Module Positions"=w2617, "Trajectory File Name"=w2620) -> ()  [unwired: 8 in]
      }
      n1526 = while {
        tunnel: w2483 -> [w2602]
        tunnel: [w2602] -> w2485
        stop <- w2594 stop-if-true
        n1527 = Wait (ms)(milliseconds to wait=u32 20) -> ()  [unwired: 1 out]
        n1528 = call-poly <vilib>:"NT Read Value.vi"("default value"=0.0, "name"="Shooter/Speed_RPM Act") -> ("value"=w2597:dbl)  [unwired: 7 in, 2 out]
        n1529 = call-poly <vilib>:"NT Write Value.vi"("value"="Shoot Mode" ("default value"), "name"="Robot State") -> ()  [unwired: 9 in, 1 out]
        n1530 = Greater?(x=w2597, y=3500.0) -> (0:w2594:bool)
        n1531 = case shown="False" w2594 {
          frame False {
            n1532 = call-poly <vilib>:"NT Write Value.vi"("value"="Stop" ("default value"), "name"="Intake/Trigger Status") -> ()  [unwired: 9 in, 1 out]
          }
          frame True {
            n1533 = call-poly <vilib>:"NT Write Value.vi"("value"="ToShooter" ("default value"), "name"="Intake/Trigger Status") -> ()  [unwired: 9 in, 1 out]
          }
        }
      }
      n1534 = while {
        tunnel: w2485 -> [w2593]
        tunnel: [w2593] -> w2484
        i -> [w2591]
        stop <- w2590 stop-if-true
        # "Wait until shooting finishes"
        n1535 = Equal To 0?(x=w2591) -> (x = 0?=w2590:bool)
        n1536 = Wait (ms)(milliseconds to wait=u32 100) -> ()  [unwired: 1 out]
      }
      n1537 = while {
        tunnel: [w2587] -> w2482
        tunnel: w2484 -> [w2587]
        i -> [w2586]
        stop <- w2585 stop-if-true
        n1538 = Equal To 0?(x=w2586) -> (x = 0?=w2585:bool)
        n1539 = call-poly <vilib>:"NT Write Value.vi"("value"="Intake Mode" ("default value"), "name"="Robot State") -> ()  [unwired: 9 in, 1 out]
        n1540 = call-poly <vilib>:"NT Write Value.vi"("value"=38.0, "name"="Shooter/Angle_Deg Dmd") -> ()  [unwired: 9 in, 1 out]
      }
      n1541 = while {
        tunnel: w2482 -> [w2651]
        tunnel: [w2651] -> w2486
        i -> [w2650]
        stop <- w2632 stop-if-true
        w2634 = TRUE  # ABS_Traj ?
        w2642 = TRUE  # EnableClosedLoop
        w2640 = FALSE  # Reverse
        w2644 = TRUE  # Follow Orientation
        n1542 = Equal To 0?(x=w2650) -> (x = 0?=w2641:bool)
        n1543 = call "SWERVE_DRIVE_GET_SPEED_DEMAND.vi"() -> ("Drv Rotation Orentation Dmd"=w2649:dbl)  [unwired: 8 in, 3 out]
        n1544 = call "SWERVE_DRIVE_GET_GYRO.vi"() -> ("Gyro Heading Radians"=w2639:dbl)  [unwired: 11 in]
        n1545 = Wait Until Next ms Multiple(millisecond multiple=u32 20 ("milliseconds to wait")) -> ()  [unwired: 1 out]
        n1546 = call "SWERVE_TRAJECTORY_EXECUTE.vi"("EnableClosedLoop"=w2642, "ABS_Traj ?"=w2634, "Init"=w2641, "Reverse"=w2640, "Follow Orientation"=w2644, "Gyro Heading\nRAD"=w2639) -> ("AtReference"=w2635:bool, "OutputTRAJ_STATE"=w2636:T12, "Error and Corr"=w2637:T13, "Chassis Velocity Target"=w2643:T14, "Orientation Target"=w2638:dbl)  [unwired: 1 in]
        n1547 = Select(t=w2639, s=w2644, f=w2649) -> (s? t:f=w2645:dbl)
        n1548 = call "SWERVE_TRAJECTORY_SET_CLOSED_LOOP.vi"("AUTO_CLOSED_LOOP"=w2642) -> ()  [unwired: 11 in]
        n1549 = call "SWERVE_TRAJECTORY_UPDATE_DIAG_INFO.vi"("AtReference"=w2635, "OutputTRAJ_STATE"=w2636, "Error and Corr"=w2637, "Orientation Target"=w2638) -> ()  [unwired: 8 in]
        n1550 = global read "SWERVE_TRAJECTORY_GLOBALS.vi" "Traj_Total_Time"() -> (w2630:dbl)
        n1551 = Unbundle By Name(w2636) -> ("TimeSeconds"=w2631:dbl)
        n1552 = Unbundle By Name(w2643) -> ("vX"=w2648:dbl, "vY"=w2647:dbl, "vOmega"=w2646:dbl)
        n1553 = Equal?(x=w2631, y=w2630) -> (x = y?=w2632:bool)
        n1554 = call "SWERVE_DRIVE_SET_SPEED_DEMAND.vi"("Drv Rotation Orentation Dmd"=w2645, "Drv Angular Vel Dmd"=w2646, "Drv Y Vel Dmd"=w2647, "Drv X Vel Dmd"=w2648) -> ()  [unwired: 8 in]
        n1555 = call-poly <vilib>:"NT Write Value.vi"("value"=w2632, "name"="Auto/Path End") -> ()  [unwired: 9 in, 1 out]
      }
      n1556 = while {
        tunnel: w2486 -> [w2616]
        tunnel: [w2616] -> w2481
        i -> [w2614]
        stop <- w2613 stop-if-true
        w2612 = 0.0 ("Drv X Vel Dmd")
        n1557 = Not Equal To 0?(x=w2614) -> (x != 0?=w2613:bool)
        n1558 = Wait (ms)(milliseconds to wait=u32 20) -> ()  [unwired: 1 out]
        n1559 = call "SWERVE_DRIVE_MODULE_STATES_POSITIONS_FGV.vi"() -> ("out Current Module Positions"=w2608:T11[])  [unwired: 10 in, 1 out]
        n1560 = call "SWERVE_DRIVE_GET_GYRO.vi"() -> ("Gyro Heading Radians"=w2610:dbl)  [unwired: 11 in]
        n1561 = call "SWERVE_DRIVE_GET_GYRO.vi"() -> ("Gyro Heading Radians"=w2611:dbl)  [unwired: 11 in]
        n1562 = call <vilib>:"Rotation2d_CreateAngle.vi"("Angle"=w2610) -> ("ROTATION"=w2609:T9)  [unwired: 10 in]
        n1563 = call "SWERVE_DRIVE_SET_SPEED_DEMAND.vi"("Drv Rotation Orentation Dmd"=w2611, "Drv Angular Vel Dmd"=w2612, "Drv Y Vel Dmd"=w2612, "Drv X Vel Dmd"=w2612) -> ()  [unwired: 8 in]
        n1564 = call "SWERVE_TRAJECTORY_BEGIN.vi"("gyroAngle"=w2609, "Module Positions"=w2608, "Trajectory File Name"="Path Demo.wpilib.csv") -> ()  [unwired: 9 in]
      }
      n1565 = while {
        tunnel: w2481 -> [w2578]
        tunnel: [w2578] -> w2480
        stop <- w2571 stop-if-true
        n1566 = call-poly <vilib>:"NT Write Value.vi"("value"="Shoot Mode" ("default value"), "name"="Robot State") -> ()  [unwired: 9 in, 1 out]
        n1567 = call-poly <vilib>:"NT Read Value.vi"("name"="Shooter/Angle_Deg Act") -> ("value"=w2575:dbl)  [unwired: 8 in, 2 out]
        n1568 = call-poly <vilib>:"NT Read Value.vi"("name"="Shooter/Angle_Deg Dmd") -> ("value"=w2574:dbl)  [unwired: 8 in, 2 out]
        n1569 = call <vilib>:"Util_ApproxEquals.vi"("Tolerance"=5.0, "Value 2"=w2574, "Value 1"=w2575) -> ("ApproxEquals"=w2571:bool)  [unwired: 8 in]
        n1570 = case shown="True" w2571 {
          frame False {
            n1571 = call-poly <vilib>:"NT Write Value.vi"("value"="Stop" ("default value"), "name"="Intake/Trigger Status") -> ()  [unwired: 9 in, 1 out]
          }
          frame True {
            n1572 = call-poly <vilib>:"NT Write Value.vi"("value"="ToShooter" ("default value"), "name"="Intake/Trigger Status") -> ()  [unwired: 9 in, 1 out]
          }
        }
        n1573 = Wait (ms)(milliseconds to wait=u32 20) -> ()  [unwired: 1 out]
      }
      n1574 = while {
        tunnel: w2480 -> [w2529]
        tunnel: [w2529] -> w2479
        i -> [w2527]
        stop <- w2526 stop-if-true
        # "Wait until shooting finishes"
        n1575 = Equal To 0?(x=w2527) -> (x = 0?=w2526:bool)
        n1576 = Wait (ms)(milliseconds to wait=u32 100) -> ()  [unwired: 1 out]
      }
      n1577 = while {
        tunnel: w2479 -> [w2568]
        tunnel: [w2568] -> w2478
        i -> [w2566]
        stop <- w2565 stop-if-true
        w2562 = FALSE  # ABS Odo Initialize
        w2564 = 0.0 ("Drv X Vel Dmd")
        n1578 = Not Equal To 0?(x=w2566) -> (x != 0?=w2565:bool)
        n1579 = Wait (ms)(milliseconds to wait=u32 20) -> ()  [unwired: 1 out]
        n1580 = call "SWERVE_DRIVE_MODULE_STATES_POSITIONS_FGV.vi"() -> ("out Current Module Positions"=w2559:T11[])  [unwired: 10 in, 1 out]
        n1581 = call "SWERVE_DRIVE_GET_GYRO.vi"() -> ("Gyro Heading Radians"=w2561:dbl)  [unwired: 11 in]
        n1582 = call "SWERVE_DRIVE_GET_GYRO.vi"() -> ("Gyro Heading Radians"=w2563:dbl)  [unwired: 11 in]
        n1583 = call <vilib>:"Rotation2d_CreateAngle.vi"("Angle"=w2561) -> ("ROTATION"=w2560:T9)  [unwired: 10 in]
        n1584 = call "SWERVE_DRIVE_SET_SPEED_DEMAND.vi"("Drv Rotation Orentation Dmd"=w2563, "Drv Angular Vel Dmd"=w2564, "Drv Y Vel Dmd"=w2564, "Drv X Vel Dmd"=w2564) -> ()  [unwired: 8 in]
        n1585 = call "SWERVE_TRAJECTORY_BEGIN.vi"("ABS Odo Initialize"=w2562, "gyroAngle"=w2560, "Module Positions"=w2559, "Trajectory File Name"="Route B2 R Path 2.path") -> ()  [unwired: 8 in]
      }
      n1586 = while {
        tunnel: [w2523] -> w2477
        tunnel: w2478 -> [w2523]
        i -> [w2522]
        stop <- w2521 stop-if-true
        n1587 = Equal To 0?(x=w2522) -> (x = 0?=w2521:bool)
        n1588 = call-poly <vilib>:"NT Write Value.vi"("value"="Intake Mode" ("default value"), "name"="Robot State") -> ()  [unwired: 9 in, 1 out]
      }
      n1589 = while {
        tunnel: w2477 -> [w2554]
        tunnel: [w2554] -> w2476
        i -> [w2553]
        stop <- w2535 stop-if-true
        w2537 = TRUE  # ABS_Traj ?
        w2545 = TRUE  # EnableClosedLoop
        w2543 = FALSE  # Reverse
        w2547 = TRUE  # Follow Orientation
        n1590 = Equal To 0?(x=w2553) -> (x = 0?=w2544:bool)
        n1591 = call "SWERVE_DRIVE_GET_SPEED_DEMAND.vi"() -> ("Drv Rotation Orentation Dmd"=w2552:dbl)  [unwired: 8 in, 3 out]
        n1592 = call "SWERVE_DRIVE_GET_GYRO.vi"() -> ("Gyro Heading Radians"=w2542:dbl)  [unwired: 11 in]
        n1593 = Wait Until Next ms Multiple(millisecond multiple=u32 20 ("milliseconds to wait")) -> ()  [unwired: 1 out]
        n1594 = call "SWERVE_TRAJECTORY_EXECUTE.vi"("EnableClosedLoop"=w2545, "ABS_Traj ?"=w2537, "Init"=w2544, "Reverse"=w2543, "Follow Orientation"=w2547, "Gyro Heading\nRAD"=w2542) -> ("AtReference"=w2538:bool, "OutputTRAJ_STATE"=w2539:T12, "Error and Corr"=w2540:T13, "Chassis Velocity Target"=w2546:T14, "Orientation Target"=w2541:dbl)  [unwired: 1 in]
        n1595 = Select(t=w2542, s=w2547, f=w2552) -> (s? t:f=w2548:dbl)
        n1596 = call "SWERVE_TRAJECTORY_SET_CLOSED_LOOP.vi"("AUTO_CLOSED_LOOP"=w2545) -> ()  [unwired: 11 in]
        n1597 = call "SWERVE_TRAJECTORY_UPDATE_DIAG_INFO.vi"("AtReference"=w2538, "OutputTRAJ_STATE"=w2539, "Error and Corr"=w2540, "Orientation Target"=w2541) -> ()  [unwired: 8 in]
        n1598 = global read "SWERVE_TRAJECTORY_GLOBALS.vi" "Traj_Total_Time"() -> (w2531:dbl)
        n1599 = Unbundle By Name(w2539) -> ("TimeSeconds"=w2532:dbl)
        n1600 = Unbundle By Name(w2546) -> ("vX"=w2551:dbl, "vY"=w2550:dbl, "vOmega"=w2549:dbl)
        n1601 = Divide(x=w2532, y=w2531) -> (x/y=w2534:dbl)
        n1602 = Equal?(x=w2532, y=w2531) -> (x = y?=w2535:bool)
        n1603 = Greater Or Equal?(x=w2534, y=0.7) -> (x >= y?=w2530:bool)
        n1604 = call "SWERVE_DRIVE_SET_SPEED_DEMAND.vi"("Drv Rotation Orentation Dmd"=w2548, "Drv Angular Vel Dmd"=w2549, "Drv Y Vel Dmd"=w2550, "Drv X Vel Dmd"=w2551) -> ()  [unwired: 8 in]
        n1605 = case shown="True" w2530 {
          frame False {
          }
          frame True {
            n1606 = call-poly <vilib>:"NT Write Value.vi"("value"="Shoot Mode" ("default value"), "name"="Robot State") -> ()  [unwired: 9 in, 1 out]
          }
        }
        n1607 = call-poly <vilib>:"NT Write Value.vi"("value"=w2535, "name"="Auto/Path End") -> ()  [unwired: 9 in, 1 out]
      }
      n1608 = while {
        tunnel: w2476 -> [w2520]
        tunnel: [w2520] -> w2475
        i -> [w2518]
        stop <- w2517 stop-if-true
        w2516 = 0.0 ("Drv X Vel Dmd")
        n1609 = Not Equal To 0?(x=w2518) -> (x != 0?=w2517:bool)
        n1610 = Wait (ms)(milliseconds to wait=u32 20) -> ()  [unwired: 1 out]
        n1611 = call "SWERVE_DRIVE_MODULE_STATES_POSITIONS_FGV.vi"() -> ("out Current Module Positions"=w2512:T11[])  [unwired: 10 in, 1 out]
        n1612 = call "SWERVE_DRIVE_GET_GYRO.vi"() -> ("Gyro Heading Radians"=w2514:dbl)  [unwired: 11 in]
        n1613 = call "SWERVE_DRIVE_GET_GYRO.vi"() -> ("Gyro Heading Radians"=w2515:dbl)  [unwired: 11 in]
        n1614 = call <vilib>:"Rotation2d_CreateAngle.vi"("Angle"=w2514) -> ("ROTATION"=w2513:T9)  [unwired: 10 in]
        n1615 = call "SWERVE_DRIVE_SET_SPEED_DEMAND.vi"("Drv Rotation Orentation Dmd"=w2515, "Drv Angular Vel Dmd"=w2516, "Drv Y Vel Dmd"=w2516, "Drv X Vel Dmd"=w2516) -> ()  [unwired: 8 in]
        n1616 = call "SWERVE_TRAJECTORY_BEGIN.vi"("gyroAngle"=w2513, "Module Positions"=w2512, "Trajectory File Name"="Path Demo.wpilib.csv") -> ()  [unwired: 9 in]
      }
      n1617 = while {
        tunnel: w2475 -> [w2506]
        tunnel: [w2506] -> _
        stop <- FALSE stop-if-true
        w2492 = 0.0 ("Drv X Vel Dmd")
        n1618 = call-poly <vilib>:"NT Write Value.vi"("value"="Shoot Mode" ("default value"), "name"="Robot State") -> ()  [unwired: 9 in, 1 out]
        n1619 = call-poly <vilib>:"NT Read Value.vi"("name"="Shooter/Angle_Deg Act") -> ("value"=w2503:dbl)  [unwired: 8 in, 2 out]
        n1620 = call-poly <vilib>:"NT Read Value.vi"("name"="Shooter/Angle_Deg Dmd") -> ("value"=w2502:dbl)  [unwired: 8 in, 2 out]
        n1621 = call-poly <vilib>:"NT Read Value.vi"("name"="Shooter/Corrected Theta") -> ("value"=w2494:dbl)  [unwired: 8 in, 2 out]
        n1622 = call-poly <vilib>:"NT Read Value.vi"("name"="/limelight/tv") -> ("value"=w2496:dbl)  [unwired: 8 in, 2 out]
        n1623 = Not Equal To 0?(x=w2496) -> (x != 0?=w2495:bool)
        n1624 = call "SWERVE_DRIVE_GET_GYRO.vi"() -> ("Gyro Heading Radians"=w2490:dbl)  [unwired: 11 in]
        n1625 = call <vilib>:"Util_ApproxEquals.vi"("Tolerance"=5.0, "Value 2"=w2502, "Value 1"=w2503) -> ("ApproxEquals"=w2489:bool)  [unwired: 8 in]
        n1626 = Select(t=w2494, s=w2495, f=w2490) -> (s? t:f=w2493:dbl)
        n1627 = case shown="False" w2489 {
          frame False {
            n1628 = call-poly <vilib>:"NT Write Value.vi"("value"="Stop" ("default value"), "name"="Intake/Trigger Status") -> ()  [unwired: 9 in, 1 out]
          }
          frame True {
            n1629 = call-poly <vilib>:"NT Write Value.vi"("value"="ToShooter" ("default value"), "name"="Intake/Trigger Status") -> ()  [unwired: 9 in, 1 out]
          }
        }
        n1630 = call "SWERVE_DRIVE_SET_SPEED_DEMAND.vi"("Drv Rotation Orentation Dmd"=w2493, "Drv Angular Vel Dmd"=w2492, "Drv Y Vel Dmd"=w2492, "Drv X Vel Dmd"=w2492) -> ()  [unwired: 8 in]
        n1631 = Wait (ms)(milliseconds to wait=u32 20) -> ()  [unwired: 1 out]
      }
    }
    frame "Route A1 R old" {
      w2660 = errorcluster {"status"=FALSE, "code"=0, "source"=""}  # Start Error Flow
      # "Trigger events when robot pose approx equals event pose\n(The two while loops below ends when the path above is ended)"
      # "Shoot Preload"
      n1632 = while {
        tunnel: w2660 -> [w2766]
        tunnel: [w2766] -> w2656
        i -> [w2764]
        stop <- w2763 stop-if-true
        w2760 = TRUE  # ABS Odo Initialize
        w2762 = 0.0 ("Drv X Vel Dmd")
        n1633 = Not Equal To 0?(x=w2764) -> (x != 0?=w2763:bool)
        n1634 = Wait (ms)(milliseconds to wait=u32 20) -> ()  [unwired: 1 out]
        n1635 = call-poly <vilib>:"NT Read Value.vi"("default value"="Path_Testing_1.path" ("Trajectory File Name"), "name"="Initial Path") -> ("value"=w2757:string)  [unwired: 7 in, 2 out]
        n1636 = call "SWERVE_DRIVE_MODULE_STATES_POSITIONS_FGV.vi"() -> ("out Current Module Positions"=w2754:T11[])  [unwired: 10 in, 1 out]
        n1637 = call "SWERVE_DRIVE_GET_GYRO.vi"() -> ("Gyro Heading Radians"=w2756:dbl)  [unwired: 11 in]
        n1638 = call "SWERVE_DRIVE_GET_GYRO.vi"() -> ("Gyro Heading Radians"=w2761:dbl)  [unwired: 11 in]
        n1639 = call <vilib>:"Rotation2d_CreateAngle.vi"("Angle"=w2756) -> ("ROTATION"=w2755:T9)  [unwired: 10 in]
        n1640 = call "SWERVE_DRIVE_SET_SPEED_DEMAND.vi"("Drv Rotation Orentation Dmd"=w2761, "Drv Angular Vel Dmd"=w2762, "Drv Y Vel Dmd"=w2762, "Drv X Vel Dmd"=w2762) -> ()  [unwired: 8 in]
        n1641 = call "SWERVE_TRAJECTORY_BEGIN.vi"("ABS Odo Initialize"=w2760, "gyroAngle"=w2755, "Module Positions"=w2754, "Trajectory File Name"=w2757) -> ()  [unwired: 8 in]
      }
      n1642 = while {
        tunnel: w2656 -> [w2739]
        tunnel: [w2739] -> w2658
        stop <- w2731 stop-if-true
        n1643 = Wait (ms)(milliseconds to wait=u32 20) -> ()  [unwired: 1 out]
        n1644 = call-poly <vilib>:"NT Read Value.vi"("default value"=0.0, "name"="Shooter/Speed_RPM Act") -> ("value"=w2734:dbl)  [unwired: 7 in, 2 out]
        n1645 = call-poly <vilib>:"NT Write Value.vi"("value"="Shoot Mode" ("default value"), "name"="Robot State") -> ()  [unwired: 9 in, 1 out]
        n1646 = Greater?(x=w2734, y=4000.0) -> (0:w2731:bool)
        n1647 = case shown="False" w2731 {
          frame False {
            n1648 = call-poly <vilib>:"NT Write Value.vi"("value"="Stop" ("default value"), "name"="Intake/Trigger Status") -> ()  [unwired: 9 in, 1 out]
          }
          frame True {
            n1649 = call-poly <vilib>:"NT Write Value.vi"("value"="ToShooter" ("default value"), "name"="Intake/Trigger Status") -> ()  [unwired: 9 in, 1 out]
          }
        }
      }
      n1650 = while {
        tunnel: w2658 -> [w2730]
        tunnel: [w2730] -> w2657
        i -> [w2728]
        stop <- w2727 stop-if-true
        # "Wait until shooting finishes"
        n1651 = Equal To 0?(x=w2728) -> (x = 0?=w2727:bool)
        n1652 = Wait (ms)(milliseconds to wait=u32 1000) -> ()  [unwired: 1 out]
      }
      n1653 = while {
        tunnel: [w2724] -> w2655
        tunnel: w2657 -> [w2724]
        i -> [w2723]
        stop <- w2722 stop-if-true
        n1654 = Equal To 0?(x=w2723) -> (x = 0?=w2722:bool)
        n1655 = call-poly <vilib>:"NT Write Value.vi"("value"="Intake Mode" ("default value"), "name"="Robot State") -> ()  [unwired: 9 in, 1 out]
      }
      n1656 = while {
        tunnel: w2655 -> [w2787]
        tunnel: [w2787] -> w2659
        i -> [w2785]
        stop <- w2767 stop-if-true
        w2769 = TRUE  # ABS_Traj ?
        w2777 = TRUE  # EnableClosedLoop
        w2775 = FALSE  # Reverse
        w2779 = TRUE  # Follow Orientation
        n1657 = Equal To 0?(x=w2785) -> (x = 0?=w2776:bool)
        n1658 = call "SWERVE_DRIVE_GET_SPEED_DEMAND.vi"() -> ("Drv Rotation Orentation Dmd"=w2784:dbl)  [unwired: 8 in, 3 out]
        n1659 = call "SWERVE_DRIVE_GET_GYRO.vi"() -> ("Gyro Heading Radians"=w2774:dbl)  [unwired: 11 in]
        n1660 = Wait Until Next ms Multiple(millisecond multiple=u32 20 ("milliseconds to wait")) -> ()  [unwired: 1 out]
        n1661 = call "SWERVE_TRAJECTORY_EXECUTE.vi"("EnableClosedLoop"=w2777, "ABS_Traj ?"=w2769, "Init"=w2776, "Reverse"=w2775, "Follow Orientation"=w2779, "Gyro Heading\nRAD"=w2774) -> ("AtReference"=w2770:bool, "OutputTRAJ_STATE"=w2771:T12, "Error and Corr"=w2772:T13, "Chassis Velocity Target"=w2778:T14, "Orientation Target"=w2773:dbl)  [unwired: 1 in]
        n1662 = Select(t=w2774, s=w2779, f=w2784) -> (s? t:f=w2780:dbl)
        n1663 = call "SWERVE_TRAJECTORY_SET_CLOSED_LOOP.vi"("AUTO_CLOSED_LOOP"=w2777) -> ()  [unwired: 11 in]
        n1664 = call "SWERVE_TRAJECTORY_UPDATE_DIAG_INFO.vi"("AtReference"=w2770, "OutputTRAJ_STATE"=w2771, "Error and Corr"=w2772, "Orientation Target"=w2773) -> ()  [unwired: 8 in]
        n1665 = global read "SWERVE_TRAJECTORY_GLOBALS.vi" "Traj_Total_Time"() -> (w2788:dbl)
        n1666 = Unbundle By Name(w2771) -> ("TimeSeconds"=w2786:dbl)
        n1667 = Unbundle By Name(w2778) -> ("vX"=w2783:dbl, "vY"=w2782:dbl, "vOmega"=w2781:dbl)
        n1668 = Equal?(x=w2786, y=w2788) -> (x = y?=w2767:bool)
        n1669 = call "SWERVE_DRIVE_SET_SPEED_DEMAND.vi"("Drv Rotation Orentation Dmd"=w2780, "Drv Angular Vel Dmd"=w2781, "Drv Y Vel Dmd"=w2782, "Drv X Vel Dmd"=w2783) -> ()  [unwired: 8 in]
        n1670 = call-poly <vilib>:"NT Write Value.vi"("value"=w2767, "name"="Auto/Path End") -> ()  [unwired: 9 in, 1 out]
      }
      n1671 = while {
        tunnel: w2655 -> [w2693]
        tunnel: [w2693] -> _
        tunnel: cluster{"X":dbl, "Y":dbl, "Event":string}[] [{"X"=13.197, "Y"=6.993, "Event"="Shoot"}, {"X"=12.84, "Y"=7.12, "Event"="Trigger"}, {"X"=11.585, "Y"=7.309, "Event"="Intake"}] -> [w2689]
        stop <- w2687 stop-if-true
        n1672 = call "SWERVE_ODOM_ABS_FGV.vi"() -> ("out SWERVE_DRIVE_ODOMETRY"=w2685:T25)  [unwired: 10 in, 1 out]
        n1673 = Unbundle By Name(w2685) -> ("POSE.TRANSLATION.X"=w2692:dbl, "POSE.TRANSLATION.Y"=w2691:dbl)
        n1674 = call-poly <vilib>:"NT Read Value.vi"("default value"=FALSE, "name"="Auto/Path End") -> ("value"=w2687:bool)  [unwired: 7 in, 2 out]
        n1675 = Wait (ms)(milliseconds to wait=u32 20) -> ()  [unwired: 1 out]
        n1676 = Build Array(w2692, w2691) -> (w2690:dbl[])
        n1677 = for {
          tunnel: w2690 -> [w2701]
          tunnel: w2689 -> [w2700] mode=indexing
          n1678 = Unbundle(w2700) -> ("X"=w2699:dbl, "Y"=w2698:dbl, "Event"=w2694:string)
          n1679 = Build Array(w2699, w2698) -> (w2697:dbl[])
          n1680 = for {
            tunnel: w2701 -> [w2707] mode=indexing
            tunnel: [w2705] -> w2696 mode=indexing
            tunnel: w2697 -> [w2704] mode=indexing
            n1681 = call <vilib>:"Util_ApproxEquals.vi"("Tolerance"=0.15, "Value 2"=w2704, "Value 1"=w2707) -> ("ApproxEquals"=w2705:bool)  [unwired: 8 in]
          }
          n1682 = And Array Elements(Boolean array=w2696) -> (logical AND=w2695:bool)
          n1683 = case shown="True" w2695 {
            tunnel: w2694 -> [_ w2702]
            frame False {
            }
            frame True {
              n1684 = call-poly <vilib>:"NT Write Value.vi"("value"=w2702, "name"="Auto State") -> ()  [unwired: 9 in, 1 out]
            }
          }
        }
      }
      n1685 = while {
        tunnel: w2655 -> [w2712]
        tunnel: [w2712] -> _
        stop <- w2710 stop-if-true
        n1686 = call-poly <vilib>:"NT Read Value.vi"("default value"="None", "name"="Auto State") -> ("value"=w2714:string)  [unwired: 7 in, 2 out]
        n1687 = call-poly <vilib>:"NT Read Value.vi"("default value"=FALSE, "name"="Auto/Path End") -> ("value"=w2710:bool)  [unwired: 7 in, 2 out]
        n1688 = Wait (ms)(milliseconds to wait=u32 20) -> ()  [unwired: 1 out]
        n1689 = case shown="\"Trigger\"" w2714 {
          frame "None", Default {
          }
          frame "Shoot" {
            n1690 = call-poly <vilib>:"NT Write Value.vi"("value"="Shoot Mode" ("default value"), "name"="Robot State") -> ()  [unwired: 9 in, 1 out]
          }
          frame "Intake" {
            n1691 = call-poly <vilib>:"NT Write Value.vi"("value"="Intake Mode" ("default value"), "name"="Robot State") -> ()  [unwired: 9 in, 1 out]
          }
          frame "Trigger" {
            n1692 = call-poly <vilib>:"NT Write Value.vi"("value"="ToShooter" ("default value"), "name"="Intake/Trigger Status") -> ()  [unwired: 9 in, 1 out]
          }
        }
      }
      n1693 = while {
        tunnel: w2659 -> [w2753]
        tunnel: [w2753] -> w2654
        i -> [w2751]
        stop <- w2750 stop-if-true
        w2749 = 0.0 ("Drv X Vel Dmd")
        n1694 = Not Equal To 0?(x=w2751) -> (x != 0?=w2750:bool)
        n1695 = Wait (ms)(milliseconds to wait=u32 20) -> ()  [unwired: 1 out]
        n1696 = call "SWERVE_DRIVE_MODULE_STATES_POSITIONS_FGV.vi"() -> ("out Current Module Positions"=w2745:T11[])  [unwired: 10 in, 1 out]
        n1697 = call "SWERVE_DRIVE_GET_GYRO.vi"() -> ("Gyro Heading Radians"=w2747:dbl)  [unwired: 11 in]
        n1698 = call "SWERVE_DRIVE_GET_GYRO.vi"() -> ("Gyro Heading Radians"=w2748:dbl)  [unwired: 11 in]
        n1699 = call <vilib>:"Rotation2d_CreateAngle.vi"("Angle"=w2747) -> ("ROTATION"=w2746:T9)  [unwired: 10 in]
        n1700 = call "SWERVE_DRIVE_SET_SPEED_DEMAND.vi"("Drv Rotation Orentation Dmd"=w2748, "Drv Angular Vel Dmd"=w2749, "Drv Y Vel Dmd"=w2749, "Drv X Vel Dmd"=w2749) -> ()  [unwired: 8 in]
        n1701 = call "SWERVE_TRAJECTORY_BEGIN.vi"("gyroAngle"=w2746, "Module Positions"=w2745, "Trajectory File Name"="Path Demo.wpilib.csv") -> ()  [unwired: 9 in]
      }
      n1702 = while {
        tunnel: w2654 -> [w2679]
        tunnel: [w2679] -> _
        stop <- FALSE stop-if-true
        w2663 = 0.0 ("Drv X Vel Dmd")
        n1703 = call-poly <vilib>:"NT Write Value.vi"("value"="Shoot Mode" ("default value"), "name"="Robot State") -> ()  [unwired: 9 in, 1 out]
        n1704 = call-poly <vilib>:"NT Read Value.vi"("name"="Shooter/Angle_Deg Act") -> ("value"=w2676:dbl)  [unwired: 8 in, 2 out]
        n1705 = call-poly <vilib>:"NT Read Value.vi"("name"="Shooter/Angle_Deg Dmd") -> ("value"=w2675:dbl)  [unwired: 8 in, 2 out]
        n1706 = call-poly <vilib>:"NT Read Value.vi"("name"="Shooter/Corrected Theta") -> ("value"=w2665:dbl)  [unwired: 8 in, 2 out]
        n1707 = call-poly <vilib>:"NT Read Value.vi"("name"="/limelight/tv") -> ("value"=w2667:dbl)  [unwired: 8 in, 2 out]
        n1708 = Not Equal To 0?(x=w2667) -> (x != 0?=w2666:bool)
        n1709 = call "SWERVE_DRIVE_GET_GYRO.vi"() -> ("Gyro Heading Radians"=w2661:dbl)  [unwired: 11 in]
        n1710 = call <vilib>:"Util_ApproxEquals.vi"("Tolerance"=2.0, "Value 2"=w2675, "Value 1"=w2676) -> ("ApproxEquals"=w2671:bool)  [unwired: 8 in]
        n1711 = Select(t=w2665, s=w2666, f=w2661) -> (s? t:f=w2664:dbl)
        n1712 = case shown="True" w2671 {
          frame False {
            n1713 = call-poly <vilib>:"NT Write Value.vi"("value"="Stop" ("default value"), "name"="Intake/Trigger Status") -> ()  [unwired: 9 in, 1 out]
          }
          frame True {
            n1714 = call-poly <vilib>:"NT Write Value.vi"("value"="ToShooter" ("default value"), "name"="Intake/Trigger Status") -> ()  [unwired: 9 in, 1 out]
          }
        }
        n1715 = call "SWERVE_DRIVE_SET_SPEED_DEMAND.vi"("Drv Rotation Orentation Dmd"=w2664, "Drv Angular Vel Dmd"=w2663, "Drv Y Vel Dmd"=w2663, "Drv X Vel Dmd"=w2663) -> ()  [unwired: 8 in]
        n1716 = Wait (ms)(milliseconds to wait=u32 20) -> ()  [unwired: 1 out]
      }
    }
    frame "Route A1 Red old" {
      w2801 = errorcluster {"status"=FALSE, "code"=0, "source"=""}  # Start Error Flow
      # "Shoot Preload"
      n1717 = while {
        tunnel: w2801 -> [w2940]
        tunnel: [w2940] -> w2798
        i -> [w2938]
        stop <- w2937 stop-if-true
        w2934 = TRUE  # ABS Odo Initialize
        w2936 = 0.0 ("Drv X Vel Dmd")
        n1718 = Not Equal To 0?(x=w2938) -> (x != 0?=w2937:bool)
        n1719 = Wait (ms)(milliseconds to wait=u32 20) -> ()  [unwired: 1 out]
        n1720 = call-poly <vilib>:"NT Read Value.vi"("default value"="Path_Testing_1.path" ("Trajectory File Name"), "name"="Initial Path") -> ("value"=w2931:string)  [unwired: 7 in, 2 out]
        n1721 = call "SWERVE_DRIVE_MODULE_STATES_POSITIONS_FGV.vi"() -> ("out Current Module Positions"=w2928:T11[])  [unwired: 10 in, 1 out]
        n1722 = call "SWERVE_DRIVE_GET_GYRO.vi"() -> ("Gyro Heading Radians"=w2930:dbl)  [unwired: 11 in]
        n1723 = call "SWERVE_DRIVE_GET_GYRO.vi"() -> ("Gyro Heading Radians"=w2935:dbl)  [unwired: 11 in]
        n1724 = call <vilib>:"Rotation2d_CreateAngle.vi"("Angle"=w2930) -> ("ROTATION"=w2929:T9)  [unwired: 10 in]
        n1725 = call "SWERVE_DRIVE_SET_SPEED_DEMAND.vi"("Drv Rotation Orentation Dmd"=w2935, "Drv Angular Vel Dmd"=w2936, "Drv Y Vel Dmd"=w2936, "Drv X Vel Dmd"=w2936) -> ()  [unwired: 8 in]
        n1726 = call "SWERVE_TRAJECTORY_BEGIN.vi"("ABS Odo Initialize"=w2934, "gyroAngle"=w2929, "Module Positions"=w2928, "Trajectory File Name"=w2931) -> ()  [unwired: 8 in]
      }
      n1727 = while {
        tunnel: w2798 -> [w2913]
        tunnel: [w2913] -> w2799
        stop <- w2905 stop-if-true
        n1728 = Wait (ms)(milliseconds to wait=u32 20) -> ()  [unwired: 1 out]
        n1729 = call-poly <vilib>:"NT Read Value.vi"("default value"=0.0, "name"="Shooter/Speed_RPM Act") -> ("value"=w2908:dbl)  [unwired: 7 in, 2 out]
        n1730 = call-poly <vilib>:"NT Write Value.vi"("value"="Shoot Mode" ("default value"), "name"="Robot State") -> ()  [unwired: 9 in, 1 out]
        n1731 = Greater?(x=w2908, y=3500.0) -> (0:w2905:bool)
        n1732 = case shown="True" w2905 {
          frame False {
            n1733 = call-poly <vilib>:"NT Write Value.vi"("value"="Stop" ("default value"), "name"="Intake/Trigger Status") -> ()  [unwired: 9 in, 1 out]
          }
          frame True {
            n1734 = call-poly <vilib>:"NT Write Value.vi"("value"="ToShooter" ("default value"), "name"="Intake/Trigger Status") -> ()  [unwired: 9 in, 1 out]
          }
        }
      }
      n1735 = while {
        tunnel: w2799 -> [w2904]
        tunnel: [w2904] -> w2792
        i -> [w2902]
        stop <- w2901 stop-if-true
        # "Wait until shooting finishes"
        n1736 = Equal To 0?(x=w2902) -> (x = 0?=w2901:bool)
        n1737 = Wait (ms)(milliseconds to wait=u32 300) -> ()  [unwired: 1 out]
      }
      n1738 = while {
        tunnel: w2792 -> [w2970]
        tunnel: [w2970] -> w2800
        i -> [w2969]
        stop <- w2952 stop-if-true
        w2953 = TRUE  # ABS_Traj ?
        w2961 = TRUE  # EnableClosedLoop
        w2959 = FALSE  # Reverse
        w2963 = TRUE  # Follow Orientation
        n1739 = Equal To 0?(x=w2969) -> (x = 0?=w2960:bool)
        n1740 = call "SWERVE_DRIVE_GET_SPEED_DEMAND.vi"() -> ("Drv Rotation Orentation Dmd"=w2968:dbl)  [unwired: 8 in, 3 out]
        n1741 = call "SWERVE_DRIVE_GET_GYRO.vi"() -> ("Gyro Heading Radians"=w2958:dbl)  [unwired: 11 in]
        n1742 = Wait Until Next ms Multiple(millisecond multiple=u32 20 ("milliseconds to wait")) -> ()  [unwired: 1 out]
        n1743 = call "SWERVE_TRAJECTORY_EXECUTE.vi"("EnableClosedLoop"=w2961, "ABS_Traj ?"=w2953, "Init"=w2960, "Reverse"=w2959, "Follow Orientation"=w2963, "Gyro Heading\nRAD"=w2958) -> ("AtReference"=w2954:bool, "OutputTRAJ_STATE"=w2955:T12, "Error and Corr"=w2956:T13, "Chassis Velocity Target"=w2962:T14, "Orientation Target"=w2957:dbl)  [unwired: 1 in]
        n1744 = Select(t=w2958, s=w2963, f=w2968) -> (s? t:f=w2964:dbl)
        n1745 = call "SWERVE_TRAJECTORY_SET_CLOSED_LOOP.vi"("AUTO_CLOSED_LOOP"=w2961) -> ()  [unwired: 11 in]
        n1746 = call "SWERVE_TRAJECTORY_UPDATE_DIAG_INFO.vi"("AtReference"=w2954, "OutputTRAJ_STATE"=w2955, "Error and Corr"=w2956, "Orientation Target"=w2957) -> ()  [unwired: 8 in]
        n1747 = global read "SWERVE_TRAJECTORY_GLOBALS.vi" "Traj_Total_Time"() -> (w2950:dbl)
        n1748 = Unbundle By Name(w2955) -> ("TimeSeconds"=w2951:dbl)
        n1749 = Unbundle By Name(w2962) -> ("vX"=w2967:dbl, "vY"=w2966:dbl, "vOmega"=w2965:dbl)
        n1750 = Equal?(x=w2951, y=w2950) -> (x = y?=w2952:bool)
        n1751 = call "SWERVE_DRIVE_SET_SPEED_DEMAND.vi"("Drv Rotation Orentation Dmd"=w2964, "Drv Angular Vel Dmd"=w2965, "Drv Y Vel Dmd"=w2966, "Drv X Vel Dmd"=w2967) -> ()  [unwired: 8 in]
        n1752 = call-poly <vilib>:"NT Read Value.vi"("name"="Shooter/Limit L") -> ("value"=w2948:bool)  [unwired: 8 in, 2 out]
        n1753 = call-poly <vilib>:"NT Read Value.vi"("name"="Shooter/Limit R") -> ("value"=w2949:bool)  [unwired: 8 in, 2 out]
        n1754 = Not Or(1:w2949, 2:w2948) -> (0:w2945:bool)
        n1755 = Select(t="FromIntake" ("default value"), s=w2945, f="Stop" ("default value")) -> (s? t:f=w2941:string)
        n1756 = call-poly <vilib>:"NT Write Value.vi"("value"=w2941, "name"="Intake/Trigger Status") -> ()  [unwired: 9 in, 1 out]
      }
      n1757 = while {
        tunnel: w2800 -> [w2927]
        tunnel: [w2927] -> w2791
        i -> [w2925]
        stop <- w2924 stop-if-true
        w2923 = 0.0 ("Drv X Vel Dmd")
        n1758 = Not Equal To 0?(x=w2925) -> (x != 0?=w2924:bool)
        n1759 = Wait (ms)(milliseconds to wait=u32 20) -> ()  [unwired: 1 out]
        n1760 = call "SWERVE_DRIVE_MODULE_STATES_POSITIONS_FGV.vi"() -> ("out Current Module Positions"=w2919:T11[])  [unwired: 10 in, 1 out]
        n1761 = call "SWERVE_DRIVE_GET_GYRO.vi"() -> ("Gyro Heading Radians"=w2921:dbl)  [unwired: 11 in]
        n1762 = call "SWERVE_DRIVE_GET_GYRO.vi"() -> ("Gyro Heading Radians"=w2922:dbl)  [unwired: 11 in]
        n1763 = call <vilib>:"Rotation2d_CreateAngle.vi"("Angle"=w2921) -> ("ROTATION"=w2920:T9)  [unwired: 10 in]
        n1764 = call "SWERVE_DRIVE_SET_SPEED_DEMAND.vi"("Drv Rotation Orentation Dmd"=w2922, "Drv Angular Vel Dmd"=w2923, "Drv Y Vel Dmd"=w2923, "Drv X Vel Dmd"=w2923) -> ()  [unwired: 8 in]
        n1765 = call "SWERVE_TRAJECTORY_BEGIN.vi"("gyroAngle"=w2920, "Module Positions"=w2919, "Trajectory File Name"="Path Demo.wpilib.csv") -> ()  [unwired: 9 in]
      }
      n1766 = while {
        tunnel: w2791 -> [w2813]
        tunnel: [w2813] -> w2790
        i -> [w2805]
        stop <- w2802 stop-if-true
        n1767 = call-poly <vilib>:"NT Read Value.vi"("name"="Shooter/Angle_Deg Act") -> ("value"=w2810:dbl)  [unwired: 8 in, 2 out]
        n1768 = call-poly <vilib>:"NT Read Value.vi"("name"="Shooter/Angle_Deg Dmd") -> ("value"=w2809:dbl)  [unwired: 8 in, 2 out]
        n1769 = Greater?(x=w2805, y=25) -> (0:w2803:bool)
        n1770 = call <vilib>:"Util_ApproxEquals.vi"("Tolerance"=5.0, "Value 2"=w2809, "Value 1"=w2810) -> ("ApproxEquals"=w2806:bool)  [unwired: 8 in]
        n1771 = Or(x=w2806, y=w2803) -> (x .or. y?=w2802:bool)
        n1772 = case shown="True" w2802 {
          frame False {
            n1773 = call-poly <vilib>:"NT Write Value.vi"("value"="Stop" ("default value"), "name"="Intake/Trigger Status") -> ()  [unwired: 9 in, 1 out]
          }
          frame True {
            n1774 = call-poly <vilib>:"NT Write Value.vi"("value"="ToShooter" ("default value"), "name"="Intake/Trigger Status") -> ()  [unwired: 9 in, 1 out]
          }
        }
        n1775 = Wait (ms)(milliseconds to wait=u32 20) -> ()  [unwired: 1 out]
      }
      n1776 = while {
        tunnel: w2790 -> [w2851]
        tunnel: [w2851] -> w2797
        i -> [w2849]
        stop <- w2848 stop-if-true
        # "Wait until shooting finishes"
        n1777 = Equal To 0?(x=w2849) -> (x = 0?=w2848:bool)
        n1778 = Wait (ms)(milliseconds to wait=u32 1000) -> ()  [unwired: 1 out]
      }
      n1779 = while {
        tunnel: w2797 -> [w2900]
        tunnel: [w2900] -> w2796
        i -> [w2898]
        stop <- w2897 stop-if-true
        w2894 = FALSE  # ABS Odo Initialize
        w2896 = 0.0 ("Drv X Vel Dmd")
        n1780 = Not Equal To 0?(x=w2898) -> (x != 0?=w2897:bool)
        n1781 = Wait (ms)(milliseconds to wait=u32 20) -> ()  [unwired: 1 out]
        n1782 = call "SWERVE_DRIVE_MODULE_STATES_POSITIONS_FGV.vi"() -> ("out Current Module Positions"=w2891:T11[])  [unwired: 10 in, 1 out]
        n1783 = call "SWERVE_DRIVE_GET_GYRO.vi"() -> ("Gyro Heading Radians"=w2893:dbl)  [unwired: 11 in]
        n1784 = call "SWERVE_DRIVE_GET_GYRO.vi"() -> ("Gyro Heading Radians"=w2895:dbl)  [unwired: 11 in]
        n1785 = call <vilib>:"Rotation2d_CreateAngle.vi"("Angle"=w2893) -> ("ROTATION"=w2892:T9)  [unwired: 10 in]
        n1786 = call "SWERVE_DRIVE_SET_SPEED_DEMAND.vi"("Drv Rotation Orentation Dmd"=w2895, "Drv Angular Vel Dmd"=w2896, "Drv Y Vel Dmd"=w2896, "Drv X Vel Dmd"=w2896) -> ()  [unwired: 8 in]
        n1787 = call "SWERVE_TRAJECTORY_BEGIN.vi"("ABS Odo Initialize"=w2894, "gyroAngle"=w2892, "Module Positions"=w2891, "Trajectory File Name"="Route A1 R Path 2.path") -> ()  [unwired: 8 in]
      }
      n1788 = while {
        tunnel: [w2845] -> w2795
        tunnel: w2796 -> [w2845]
        i -> [w2844]
        stop <- w2843 stop-if-true
        n1789 = Equal To 0?(x=w2844) -> (x = 0?=w2843:bool)
        n1790 = call-poly <vilib>:"NT Write Value.vi"("value"="Intake Mode" ("default value"), "name"="Robot State") -> ()  [unwired: 9 in, 1 out]
      }
      n1791 = while {
        tunnel: w2795 -> [w2881]
        tunnel: [w2881] -> w2794
        i -> [w2880]
        stop <- w2862 stop-if-true
        w2864 = TRUE  # ABS_Traj ?
        w2872 = TRUE  # EnableClosedLoop
        w2870 = FALSE  # Reverse
        w2874 = TRUE  # Follow Orientation
        n1792 = Equal To 0?(x=w2880) -> (x = 0?=w2871:bool)
        n1793 = call "SWERVE_DRIVE_GET_SPEED_DEMAND.vi"() -> ("Drv Rotation Orentation Dmd"=w2879:dbl)  [unwired: 8 in, 3 out]
        n1794 = call "SWERVE_DRIVE_GET_GYRO.vi"() -> ("Gyro Heading Radians"=w2869:dbl)  [unwired: 11 in]
        n1795 = Wait Until Next ms Multiple(millisecond multiple=u32 20 ("milliseconds to wait")) -> ()  [unwired: 1 out]
        n1796 = call "SWERVE_TRAJECTORY_EXECUTE.vi"("EnableClosedLoop"=w2872, "ABS_Traj ?"=w2864, "Init"=w2871, "Reverse"=w2870, "Follow Orientation"=w2874, "Gyro Heading\nRAD"=w2869) -> ("AtReference"=w2865:bool, "OutputTRAJ_STATE"=w2866:T12, "Error and Corr"=w2867:T13, "Chassis Velocity Target"=w2873:T14, "Orientation Target"=w2868:dbl)  [unwired: 1 in]
        n1797 = Select(t=w2869, s=w2874, f=w2879) -> (s? t:f=w2875:dbl)
        n1798 = call "SWERVE_TRAJECTORY_SET_CLOSED_LOOP.vi"("AUTO_CLOSED_LOOP"=w2872) -> ()  [unwired: 11 in]
        n1799 = call "SWERVE_TRAJECTORY_UPDATE_DIAG_INFO.vi"("AtReference"=w2865, "OutputTRAJ_STATE"=w2866, "Error and Corr"=w2867, "Orientation Target"=w2868) -> ()  [unwired: 8 in]
        n1800 = global read "SWERVE_TRAJECTORY_GLOBALS.vi" "Traj_Total_Time"() -> (w2852:dbl)
        n1801 = Unbundle By Name(w2866) -> ("TimeSeconds"=w2853:dbl)
        n1802 = Unbundle By Name(w2873) -> ("vX"=w2878:dbl, "vY"=w2877:dbl, "vOmega"=w2876:dbl)
        n1803 = Equal?(x=w2853, y=w2852) -> (x = y?=w2862:bool)
        n1804 = Divide(x=w2853, y=w2852) -> (x/y=w2861:dbl)
        n1805 = call "SWERVE_DRIVE_SET_SPEED_DEMAND.vi"("Drv Rotation Orentation Dmd"=w2875, "Drv Angular Vel Dmd"=w2876, "Drv Y Vel Dmd"=w2877, "Drv X Vel Dmd"=w2878) -> ()  [unwired: 8 in]
        n1806 = Greater Or Equal?(x=w2861, y=0.5) -> (x >= y?=w2859:bool)
        n1807 = call-poly <vilib>:"NT Read Value.vi"("name"="Shooter/Limit L") -> ("value"=w2857:bool)  [unwired: 8 in, 2 out]
        n1808 = call-poly <vilib>:"NT Read Value.vi"("name"="Shooter/Limit R") -> ("value"=w2858:bool)  [unwired: 8 in, 2 out]
        n1809 = Not Or(1:w2858, 2:w2857) -> (0:w2854:bool)
        n1810 = case shown="True" w2859 {
          tunnel: w2854 -> [_ w2884]
          frame False {
          }
          frame True {
            n1811 = Select(t="FromIntake" ("default value"), s=w2884, f="Stop" ("default value")) -> (s? t:f=w2883:string)
            n1812 = call-poly <vilib>:"NT Write Value.vi"("value"=w2883, "name"="Intake/Trigger Status") -> ()  [unwired: 9 in, 1 out]
            n1813 = call-poly <vilib>:"NT Write Value.vi"("value"="Shoot Mode" ("default value"), "name"="Robot State") -> ()  [unwired: 9 in, 1 out]
          }
        }
        n1814 = call-poly <vilib>:"NT Write Value.vi"("value"=w2862, "name"="Auto/Path End") -> ()  [unwired: 9 in, 1 out]
      }
      n1815 = while {
        tunnel: w2794 -> [w2842]
        tunnel: [w2842] -> w2793
        i -> [w2840]
        stop <- w2839 stop-if-true
        w2838 = 0.0 ("Drv X Vel Dmd")
        n1816 = Not Equal To 0?(x=w2840) -> (x != 0?=w2839:bool)
        n1817 = Wait (ms)(milliseconds to wait=u32 20) -> ()  [unwired: 1 out]
        n1818 = call "SWERVE_DRIVE_MODULE_STATES_POSITIONS_FGV.vi"() -> ("out Current Module Positions"=w2834:T11[])  [unwired: 10 in, 1 out]
        n1819 = call "SWERVE_DRIVE_GET_GYRO.vi"() -> ("Gyro Heading Radians"=w2836:dbl)  [unwired: 11 in]
        n1820 = call "SWERVE_DRIVE_GET_GYRO.vi"() -> ("Gyro Heading Radians"=w2837:dbl)  [unwired: 11 in]
        n1821 = call <vilib>:"Rotation2d_CreateAngle.vi"("Angle"=w2836) -> ("ROTATION"=w2835:T9)  [unwired: 10 in]
        n1822 = call "SWERVE_DRIVE_SET_SPEED_DEMAND.vi"("Drv Rotation Orentation Dmd"=w2837, "Drv Angular Vel Dmd"=w2838, "Drv Y Vel Dmd"=w2838, "Drv X Vel Dmd"=w2838) -> ()  [unwired: 8 in]
        n1823 = call "SWERVE_TRAJECTORY_BEGIN.vi"("gyroAngle"=w2835, "Module Positions"=w2834, "Trajectory File Name"="Path Demo.wpilib.csv") -> ()  [unwired: 9 in]
      }
      n1824 = while {
        tunnel: w2793 -> [w2828]
        tunnel: [w2828] -> _
        stop <- FALSE stop-if-true
        n1825 = call-poly <vilib>:"NT Read Value.vi"("name"="Shooter/Angle_Deg Act") -> ("value"=w2825:dbl)  [unwired: 8 in, 2 out]
        n1826 = call-poly <vilib>:"NT Read Value.vi"("name"="Shooter/Angle_Deg Dmd") -> ("value"=w2824:dbl)  [unwired: 8 in, 2 out]
        n1827 = call-poly <vilib>:"NT Write Value.vi"("value"="Shoot Mode" ("default value"), "name"="Robot State") -> ()  [unwired: 9 in, 1 out]
        n1828 = call <vilib>:"Util_ApproxEquals.vi"("Tolerance"=5.0, "Value 2"=w2824, "Value 1"=w2825) -> ("ApproxEquals"=w2818:bool)  [unwired: 8 in]
        n1829 = case shown="True" w2818 {
          frame False {
            n1830 = call-poly <vilib>:"NT Write Value.vi"("value"="Stop" ("default value"), "name"="Intake/Trigger Status") -> ()  [unwired: 9 in, 1 out]
          }
          frame True {
            n1831 = call-poly <vilib>:"NT Write Value.vi"("value"="ToShooter" ("default value"), "name"="Intake/Trigger Status") -> ()  [unwired: 9 in, 1 out]
          }
        }
        n1832 = Wait (ms)(milliseconds to wait=u32 20) -> ()  [unwired: 1 out]
      }
    }
    frame "Route A1 Red Alter" {
      w2984 = errorcluster {"status"=FALSE, "code"=0, "source"=""}  # Start Error Flow
      # "Shoot Preload"
      n1833 = while {
        tunnel: w2984 -> [w3150]
        tunnel: [w3150] -> w2980
        i -> [w3148]
        stop <- w3147 stop-if-true
        w3144 = TRUE  # ABS Odo Initialize
        w3146 = 0.0 ("Drv X Vel Dmd")
        n1834 = Not Equal To 0?(x=w3148) -> (x != 0?=w3147:bool)
        n1835 = Wait (ms)(milliseconds to wait=u32 20) -> ()  [unwired: 1 out]
        n1836 = call-poly <vilib>:"NT Read Value.vi"("default value"="Path_Testing_1.path" ("Trajectory File Name"), "name"="Initial Path") -> ("value"=w3141:string)  [unwired: 7 in, 2 out]
        n1837 = call "SWERVE_DRIVE_MODULE_STATES_POSITIONS_FGV.vi"() -> ("out Current Module Positions"=w3138:T11[])  [unwired: 10 in, 1 out]
        n1838 = call "SWERVE_DRIVE_GET_GYRO.vi"() -> ("Gyro Heading Radians"=w3140:dbl)  [unwired: 11 in]
        n1839 = call "SWERVE_DRIVE_GET_GYRO.vi"() -> ("Gyro Heading Radians"=w3145:dbl)  [unwired: 11 in]
        n1840 = call <vilib>:"Rotation2d_CreateAngle.vi"("Angle"=w3140) -> ("ROTATION"=w3139:T9)  [unwired: 10 in]
        n1841 = call "SWERVE_DRIVE_SET_SPEED_DEMAND.vi"("Drv Rotation Orentation Dmd"=w3145, "Drv Angular Vel Dmd"=w3146, "Drv Y Vel Dmd"=w3146, "Drv X Vel Dmd"=w3146) -> ()  [unwired: 8 in]
        n1842 = call "SWERVE_TRAJECTORY_BEGIN.vi"("ABS Odo Initialize"=w3144, "gyroAngle"=w3139, "Module Positions"=w3138, "Trajectory File Name"=w3141) -> ()  [unwired: 8 in]
      }
      n1843 = while {
        tunnel: w2980 -> [w3123]
        tunnel: [w3123] -> w2982
        stop <- w3115 stop-if-true
        n1844 = Wait (ms)(milliseconds to wait=u32 20) -> ()  [unwired: 1 out]
        n1845 = call-poly <vilib>:"NT Read Value.vi"("default value"=0.0, "name"="Shooter/Speed_RPM Act") -> ("value"=w3118:dbl)  [unwired: 7 in, 2 out]
        n1846 = call-poly <vilib>:"NT Write Value.vi"("value"="Shoot Mode" ("default value"), "name"="Robot State") -> ()  [unwired: 9 in, 1 out]
        n1847 = Greater?(x=w3118, y=4000.0) -> (0:w3115:bool)
        n1848 = case shown="True" w3115 {
          frame False {
            n1849 = call-poly <vilib>:"NT Write Value.vi"("value"="Stop" ("default value"), "name"="Intake/Trigger Status") -> ()  [unwired: 9 in, 1 out]
          }
          frame True {
            n1850 = call-poly <vilib>:"NT Write Value.vi"("value"="ToShooter" ("default value"), "name"="Intake/Trigger Status") -> ()  [unwired: 9 in, 1 out]
          }
        }
      }
      n1851 = while {
        tunnel: w2982 -> [w3114]
        tunnel: [w3114] -> w2981
        i -> [w3112]
        stop <- w3111 stop-if-true
        # "Wait until shooting finishes"
        n1852 = Equal To 0?(x=w3112) -> (x = 0?=w3111:bool)
        n1853 = Wait (ms)(milliseconds to wait=u32 100) -> ()  [unwired: 1 out]
      }
      n1854 = while {
        tunnel: [w3108] -> w2979
        tunnel: w2981 -> [w3108]
        i -> [w3107]
        stop <- w3106 stop-if-true
        n1855 = Equal To 0?(x=w3107) -> (x = 0?=w3106:bool)
        n1856 = call-poly <vilib>:"NT Write Value.vi"("value"="Intake Mode" ("default value"), "name"="Robot State") -> ()  [unwired: 9 in, 1 out]
        n1857 = call-poly <vilib>:"NT Write Value.vi"("value"=29.0, "name"="Shooter/Angle_Deg Dmd") -> ()  [unwired: 9 in, 1 out]
      }
      n1858 = while {
        tunnel: w2979 -> [w3179]
        tunnel: [w3179] -> w2983
        i -> [w3178]
        stop <- w3161 stop-if-true
        w3162 = TRUE  # ABS_Traj ?
        w3170 = TRUE  # EnableClosedLoop
        w3168 = FALSE  # Reverse
        w3172 = TRUE  # Follow Orientation
        n1859 = Equal To 0?(x=w3178) -> (x = 0?=w3169:bool)
        n1860 = call "SWERVE_DRIVE_GET_SPEED_DEMAND.vi"() -> ("Drv Rotation Orentation Dmd"=w3177:dbl)  [unwired: 8 in, 3 out]
        n1861 = call "SWERVE_DRIVE_GET_GYRO.vi"() -> ("Gyro Heading Radians"=w3167:dbl)  [unwired: 11 in]
        n1862 = Wait Until Next ms Multiple(millisecond multiple=u32 20 ("milliseconds to wait")) -> ()  [unwired: 1 out]
        n1863 = call "SWERVE_TRAJECTORY_EXECUTE.vi"("EnableClosedLoop"=w3170, "ABS_Traj ?"=w3162, "Init"=w3169, "Reverse"=w3168, "Follow Orientation"=w3172, "Gyro Heading\nRAD"=w3167) -> ("AtReference"=w3163:bool, "OutputTRAJ_STATE"=w3164:T12, "Error and Corr"=w3165:T13, "Chassis Velocity Target"=w3171:T14, "Orientation Target"=w3166:dbl)  [unwired: 1 in]
        n1864 = Select(t=w3167, s=w3172, f=w3177) -> (s? t:f=w3173:dbl)
        n1865 = call "SWERVE_TRAJECTORY_SET_CLOSED_LOOP.vi"("AUTO_CLOSED_LOOP"=w3170) -> ()  [unwired: 11 in]
        n1866 = call "SWERVE_TRAJECTORY_UPDATE_DIAG_INFO.vi"("AtReference"=w3163, "OutputTRAJ_STATE"=w3164, "Error and Corr"=w3165, "Orientation Target"=w3166) -> ()  [unwired: 8 in]
        n1867 = global read "SWERVE_TRAJECTORY_GLOBALS.vi" "Traj_Total_Time"() -> (w3151:dbl)
        n1868 = Unbundle By Name(w3164) -> ("TimeSeconds"=w3152:dbl)
        n1869 = Unbundle By Name(w3171) -> ("vX"=w3176:dbl, "vY"=w3175:dbl, "vOmega"=w3174:dbl)
        n1870 = Equal?(x=w3152, y=w3151) -> (x = y?=w3161:bool)
        n1871 = Divide(x=w3152, y=w3151) -> (x/y=w3160:dbl)
        n1872 = call "SWERVE_DRIVE_SET_SPEED_DEMAND.vi"("Drv Rotation Orentation Dmd"=w3173, "Drv Angular Vel Dmd"=w3174, "Drv Y Vel Dmd"=w3175, "Drv X Vel Dmd"=w3176) -> ()  [unwired: 8 in]
        n1873 = Greater Or Equal?(x=w3160, y=0.5) -> (x >= y?=w3158:bool)
        n1874 = call-poly <vilib>:"NT Read Value.vi"("name"="Shooter/Limit L") -> ("value"=w3156:bool)  [unwired: 8 in, 2 out]
        n1875 = call-poly <vilib>:"NT Read Value.vi"("name"="Shooter/Limit R") -> ("value"=w3157:bool)  [unwired: 8 in, 2 out]
        n1876 = And(x=w3156, y=w3157) -> (x .and. y?=w3153:bool)
        n1877 = case shown="True" w3158 {
          tunnel: w3153 -> [_ w3182]
          frame False {
          }
          frame True {
            n1878 = Select(t="FromIntake" ("default value"), s=w3182, f="Stop" ("default value")) -> (s? t:f=w3181:string)
            n1879 = call-poly <vilib>:"NT Write Value.vi"("value"=w3181, "name"="Intake/Trigger Status") -> ()  [unwired: 9 in, 1 out]
            n1880 = call-poly <vilib>:"NT Write Value.vi"("value"="Shoot Mode" ("default value"), "name"="Robot State") -> ()  [unwired: 9 in, 1 out]
          }
        }
      }
      n1881 = while {
        tunnel: w2983 -> [w3137]
        tunnel: [w3137] -> w2978
        i -> [w3135]
        stop <- w3134 stop-if-true
        w3133 = 0.0 ("Drv X Vel Dmd")
        n1882 = Not Equal To 0?(x=w3135) -> (x != 0?=w3134:bool)
        n1883 = Wait (ms)(milliseconds to wait=u32 20) -> ()  [unwired: 1 out]
        n1884 = call "SWERVE_DRIVE_MODULE_STATES_POSITIONS_FGV.vi"() -> ("out Current Module Positions"=w3129:T11[])  [unwired: 10 in, 1 out]
        n1885 = call "SWERVE_DRIVE_GET_GYRO.vi"() -> ("Gyro Heading Radians"=w3131:dbl)  [unwired: 11 in]
        n1886 = call "SWERVE_DRIVE_GET_GYRO.vi"() -> ("Gyro Heading Radians"=w3132:dbl)  [unwired: 11 in]
        n1887 = call <vilib>:"Rotation2d_CreateAngle.vi"("Angle"=w3131) -> ("ROTATION"=w3130:T9)  [unwired: 10 in]
        n1888 = call "SWERVE_DRIVE_SET_SPEED_DEMAND.vi"("Drv Rotation Orentation Dmd"=w3132, "Drv Angular Vel Dmd"=w3133, "Drv Y Vel Dmd"=w3133, "Drv X Vel Dmd"=w3133) -> ()  [unwired: 8 in]
        n1889 = call "SWERVE_TRAJECTORY_BEGIN.vi"("gyroAngle"=w3130, "Module Positions"=w3129, "Trajectory File Name"="Path Demo.wpilib.csv") -> ()  [unwired: 9 in]
      }
      n1890 = while {
        tunnel: w2978 -> [w3099]
        tunnel: [w3099] -> w2977
        stop <- w3080 stop-if-true
        w3086 = 0.0 ("Drv X Vel Dmd")
        n1891 = call-poly <vilib>:"NT Read Value.vi"("name"="/limelight/tv") -> ("value"=w3089:dbl)  [unwired: 8 in, 2 out]
        n1892 = call-poly <vilib>:"NT Read Value.vi"("name"="Shooter/Corrected Theta") -> ("value"=w3083:dbl)  [unwired: 8 in, 2 out]
        n1893 = call-poly <vilib>:"NT Read Value.vi"("name"="Shooter/Angle_Deg Act") -> ("value"=w3096:dbl)  [unwired: 8 in, 2 out]
        n1894 = call-poly <vilib>:"NT Read Value.vi"("name"="Shooter/Angle_Deg Dmd") -> ("value"=w3095:dbl)  [unwired: 8 in, 2 out]
        n1895 = call-poly <vilib>:"NT Write Value.vi"("value"="Shoot Mode" ("default value"), "name"="Robot State") -> ()  [unwired: 9 in, 1 out]
        n1896 = Not Equal To 0?(x=w3089) -> (x != 0?=w3088:bool)
        n1897 = call "SWERVE_DRIVE_GET_GYRO.vi"() -> ("Gyro Heading Radians"=w3084:dbl)  [unwired: 11 in]
        n1898 = Select(t=w3083, s=w3088, f=w3084) -> (s? t:f=w3087:dbl)
        n1899 = call <vilib>:"Util_ApproxEquals.vi"("Tolerance"=2.0, "Value 2"=w3095, "Value 1"=w3096) -> ("ApproxEquals"=w3085:bool)  [unwired: 8 in]
        n1900 = call <vilib>:"Util_ApproxEquals.vi"("Tolerance"=0.05, "Value 2"=w3084, "Value 1"=w3083) -> ("ApproxEquals"=w3081:bool)  [unwired: 8 in]
        n1901 = And(x=w3085, y=w3081) -> (x .and. y?=w3080:bool)
        n1902 = case shown="True" w3080 {
          frame False {
            n1903 = call-poly <vilib>:"NT Write Value.vi"("value"="Stop" ("default value"), "name"="Intake/Trigger Status") -> ()  [unwired: 9 in, 1 out]
          }
          frame True {
            n1904 = call-poly <vilib>:"NT Write Value.vi"("value"="ToShooter" ("default value"), "name"="Intake/Trigger Status") -> ()  [unwired: 9 in, 1 out]
          }
        }
        n1905 = call "SWERVE_DRIVE_SET_SPEED_DEMAND.vi"("Drv Rotation Orentation Dmd"=w3087, "Drv Angular Vel Dmd"=w3086, "Drv Y Vel Dmd"=w3086, "Drv X Vel Dmd"=w3086) -> ()  [unwired: 8 in]
        n1906 = Wait (ms)(milliseconds to wait=u32 20) -> ()  [unwired: 1 out]
      }
      n1907 = while {
        tunnel: w2977 -> [w3029]
        tunnel: [w3029] -> w2976
        i -> [w3027]
        stop <- w3026 stop-if-true
        # "Wait until shooting finishes"
        n1908 = Equal To 0?(x=w3027) -> (x = 0?=w3026:bool)
        n1909 = Wait (ms)(milliseconds to wait=u32 1000) -> ()  [unwired: 1 out]
      }
      n1910 = while {
        tunnel: w2976 -> [w3078]
        tunnel: [w3078] -> w2975
        i -> [w3076]
        stop <- w3075 stop-if-true
        w3072 = FALSE  # ABS Odo Initialize
        w3074 = 0.0 ("Drv X Vel Dmd")
        n1911 = Not Equal To 0?(x=w3076) -> (x != 0?=w3075:bool)
        n1912 = Wait (ms)(milliseconds to wait=u32 20) -> ()  [unwired: 1 out]
        n1913 = call "SWERVE_DRIVE_MODULE_STATES_POSITIONS_FGV.vi"() -> ("out Current Module Positions"=w3069:T11[])  [unwired: 10 in, 1 out]
        n1914 = call "SWERVE_DRIVE_GET_GYRO.vi"() -> ("Gyro Heading Radians"=w3071:dbl)  [unwired: 11 in]
        n1915 = call "SWERVE_DRIVE_GET_GYRO.vi"() -> ("Gyro Heading Radians"=w3073:dbl)  [unwired: 11 in]
        n1916 = call <vilib>:"Rotation2d_CreateAngle.vi"("Angle"=w3071) -> ("ROTATION"=w3070:T9)  [unwired: 10 in]
        n1917 = call "SWERVE_DRIVE_SET_SPEED_DEMAND.vi"("Drv Rotation Orentation Dmd"=w3073, "Drv Angular Vel Dmd"=w3074, "Drv Y Vel Dmd"=w3074, "Drv X Vel Dmd"=w3074) -> ()  [unwired: 8 in]
        n1918 = call "SWERVE_TRAJECTORY_BEGIN.vi"("ABS Odo Initialize"=w3072, "gyroAngle"=w3070, "Module Positions"=w3069, "Trajectory File Name"="Route A1 R Path 2.path") -> ()  [unwired: 8 in]
      }
      n1919 = while {
        tunnel: [w3023] -> w2974
        tunnel: w2975 -> [w3023]
        i -> [w3022]
        stop <- w3021 stop-if-true
        n1920 = Equal To 0?(x=w3022) -> (x = 0?=w3021:bool)
        n1921 = call-poly <vilib>:"NT Write Value.vi"("value"="Intake Mode" ("default value"), "name"="Robot State") -> ()  [unwired: 9 in, 1 out]
      }
      n1922 = while {
        tunnel: w2974 -> [w3059]
        tunnel: [w3059] -> w2973
        i -> [w3058]
        stop <- w3040 stop-if-true
        w3042 = TRUE  # ABS_Traj ?
        w3050 = TRUE  # EnableClosedLoop
        w3048 = FALSE  # Reverse
        w3052 = TRUE  # Follow Orientation
        n1923 = Equal To 0?(x=w3058) -> (x = 0?=w3049:bool)
        n1924 = call "SWERVE_DRIVE_GET_SPEED_DEMAND.vi"() -> ("Drv Rotation Orentation Dmd"=w3057:dbl)  [unwired: 8 in, 3 out]
        n1925 = call "SWERVE_DRIVE_GET_GYRO.vi"() -> ("Gyro Heading Radians"=w3047:dbl)  [unwired: 11 in]
        n1926 = Wait Until Next ms Multiple(millisecond multiple=u32 20 ("milliseconds to wait")) -> ()  [unwired: 1 out]
        n1927 = call "SWERVE_TRAJECTORY_EXECUTE.vi"("EnableClosedLoop"=w3050, "ABS_Traj ?"=w3042, "Init"=w3049, "Reverse"=w3048, "Follow Orientation"=w3052, "Gyro Heading\nRAD"=w3047) -> ("AtReference"=w3043:bool, "OutputTRAJ_STATE"=w3044:T12, "Error and Corr"=w3045:T13, "Chassis Velocity Target"=w3051:T14, "Orientation Target"=w3046:dbl)  [unwired: 1 in]
        n1928 = Select(t=w3047, s=w3052, f=w3057) -> (s? t:f=w3053:dbl)
        n1929 = call "SWERVE_TRAJECTORY_SET_CLOSED_LOOP.vi"("AUTO_CLOSED_LOOP"=w3050) -> ()  [unwired: 11 in]
        n1930 = call "SWERVE_TRAJECTORY_UPDATE_DIAG_INFO.vi"("AtReference"=w3043, "OutputTRAJ_STATE"=w3044, "Error and Corr"=w3045, "Orientation Target"=w3046) -> ()  [unwired: 8 in]
        n1931 = global read "SWERVE_TRAJECTORY_GLOBALS.vi" "Traj_Total_Time"() -> (w3030:dbl)
        n1932 = Unbundle By Name(w3044) -> ("TimeSeconds"=w3031:dbl)
        n1933 = Unbundle By Name(w3051) -> ("vX"=w3056:dbl, "vY"=w3055:dbl, "vOmega"=w3054:dbl)
        n1934 = Equal?(x=w3031, y=w3030) -> (x = y?=w3040:bool)
        n1935 = Divide(x=w3031, y=w3030) -> (x/y=w3039:dbl)
        n1936 = call "SWERVE_DRIVE_SET_SPEED_DEMAND.vi"("Drv Rotation Orentation Dmd"=w3053, "Drv Angular Vel Dmd"=w3054, "Drv Y Vel Dmd"=w3055, "Drv X Vel Dmd"=w3056) -> ()  [unwired: 8 in]
        n1937 = Greater Or Equal?(x=w3039, y=0.5) -> (x >= y?=w3037:bool)
        n1938 = call-poly <vilib>:"NT Read Value.vi"("name"="Shooter/Limit L") -> ("value"=w3035:bool)  [unwired: 8 in, 2 out]
        n1939 = call-poly <vilib>:"NT Read Value.vi"("name"="Shooter/Limit R") -> ("value"=w3036:bool)  [unwired: 8 in, 2 out]
        n1940 = And(x=w3035, y=w3036) -> (x .and. y?=w3032:bool)
        n1941 = case shown="True" w3037 {
          tunnel: w3032 -> [_ w3062]
          frame False {
          }
          frame True {
            n1942 = Select(t="FromIntake" ("default value"), s=w3062, f="Stop" ("default value")) -> (s? t:f=w3061:string)
            n1943 = call-poly <vilib>:"NT Write Value.vi"("value"=w3061, "name"="Intake/Trigger Status") -> ()  [unwired: 9 in, 1 out]
            n1944 = call-poly <vilib>:"NT Write Value.vi"("value"="Shoot Mode" ("default value"), "name"="Robot State") -> ()  [unwired: 9 in, 1 out]
          }
        }
        n1945 = call-poly <vilib>:"NT Write Value.vi"("value"=w3040, "name"="Auto/Path End") -> ()  [unwired: 9 in, 1 out]
      }
      n1946 = while {
        tunnel: w2973 -> [w3020]
        tunnel: [w3020] -> w2972
        i -> [w3018]
        stop <- w3017 stop-if-true
        w3016 = 0.0 ("Drv X Vel Dmd")
        n1947 = Not Equal To 0?(x=w3018) -> (x != 0?=w3017:bool)
        n1948 = Wait (ms)(milliseconds to wait=u32 20) -> ()  [unwired: 1 out]
        n1949 = call "SWERVE_DRIVE_MODULE_STATES_POSITIONS_FGV.vi"() -> ("out Current Module Positions"=w3012:T11[])  [unwired: 10 in, 1 out]
        n1950 = call "SWERVE_DRIVE_GET_GYRO.vi"() -> ("Gyro Heading Radians"=w3014:dbl)  [unwired: 11 in]
        n1951 = call "SWERVE_DRIVE_GET_GYRO.vi"() -> ("Gyro Heading Radians"=w3015:dbl)  [unwired: 11 in]
        n1952 = call <vilib>:"Rotation2d_CreateAngle.vi"("Angle"=w3014) -> ("ROTATION"=w3013:T9)  [unwired: 10 in]
        n1953 = call "SWERVE_DRIVE_SET_SPEED_DEMAND.vi"("Drv Rotation Orentation Dmd"=w3015, "Drv Angular Vel Dmd"=w3016, "Drv Y Vel Dmd"=w3016, "Drv X Vel Dmd"=w3016) -> ()  [unwired: 8 in]
        n1954 = call "SWERVE_TRAJECTORY_BEGIN.vi"("gyroAngle"=w3013, "Module Positions"=w3012, "Trajectory File Name"="Path Demo.wpilib.csv") -> ()  [unwired: 9 in]
      }
      n1955 = while {
        tunnel: w2972 -> [w3006]
        tunnel: [w3006] -> _
        stop <- FALSE stop-if-true
        w2993 = 0.0 ("Drv X Vel Dmd")
        n1956 = call-poly <vilib>:"NT Read Value.vi"("name"="/limelight/tv") -> ("value"=w2996:dbl)  [unwired: 8 in, 2 out]
        n1957 = call-poly <vilib>:"NT Read Value.vi"("name"="Shooter/Corrected Theta") -> ("value"=w2990:dbl)  [unwired: 8 in, 2 out]
        n1958 = call-poly <vilib>:"NT Read Value.vi"("name"="Shooter/Angle_Deg Act") -> ("value"=w3003:dbl)  [unwired: 8 in, 2 out]
        n1959 = call-poly <vilib>:"NT Read Value.vi"("name"="Shooter/Angle_Deg Dmd") -> ("value"=w3002:dbl)  [unwired: 8 in, 2 out]
        n1960 = call-poly <vilib>:"NT Write Value.vi"("value"="Shoot Mode" ("default value"), "name"="Robot State") -> ()  [unwired: 9 in, 1 out]
        n1961 = Not Equal To 0?(x=w2996) -> (x != 0?=w2995:bool)
        n1962 = call "SWERVE_DRIVE_GET_GYRO.vi"() -> ("Gyro Heading Radians"=w2991:dbl)  [unwired: 11 in]
        n1963 = Select(t=w2990, s=w2995, f=w2991) -> (s? t:f=w2994:dbl)
        n1964 = call <vilib>:"Util_ApproxEquals.vi"("Tolerance"=2.0, "Value 2"=w3002, "Value 1"=w3003) -> ("ApproxEquals"=w2992:bool)  [unwired: 8 in]
        n1965 = call <vilib>:"Util_ApproxEquals.vi"("Tolerance"=0.05, "Value 2"=w2991, "Value 1"=w2990) -> ("ApproxEquals"=w2988:bool)  [unwired: 8 in]
        n1966 = And(x=w2992, y=w2988) -> (x .and. y?=w2987:bool)
        n1967 = case shown="True" w2987 {
          frame False {
            n1968 = call-poly <vilib>:"NT Write Value.vi"("value"="Stop" ("default value"), "name"="Intake/Trigger Status") -> ()  [unwired: 9 in, 1 out]
          }
          frame True {
            n1969 = call-poly <vilib>:"NT Write Value.vi"("value"="ToShooter" ("default value"), "name"="Intake/Trigger Status") -> ()  [unwired: 9 in, 1 out]
          }
        }
        n1970 = call "SWERVE_DRIVE_SET_SPEED_DEMAND.vi"("Drv Rotation Orentation Dmd"=w2994, "Drv Angular Vel Dmd"=w2993, "Drv Y Vel Dmd"=w2993, "Drv X Vel Dmd"=w2993) -> ()  [unwired: 8 in]
        n1971 = Wait (ms)(milliseconds to wait=u32 20) -> ()  [unwired: 1 out]
      }
    }
    frame "Route B2 Red old" {
      w3199 = errorcluster {"status"=FALSE, "code"=0, "source"=""}  # Start Error Flow
      n1972 = while {
        tunnel: w3199 -> [w3338]
        tunnel: [w3338] -> w3195
        i -> [w3336]
        stop <- w3335 stop-if-true
        w3332 = TRUE  # ABS Odo Initialize
        w3334 = 0.0 ("Drv X Vel Dmd")
        n1973 = Not Equal To 0?(x=w3336) -> (x != 0?=w3335:bool)
        n1974 = Wait (ms)(milliseconds to wait=u32 20) -> ()  [unwired: 1 out]
        n1975 = call-poly <vilib>:"NT Read Value.vi"("default value"="Path_Testing_1.path" ("Trajectory File Name"), "name"="Initial Path") -> ("value"=w3329:string)  [unwired: 7 in, 2 out]
        n1976 = call "SWERVE_DRIVE_MODULE_STATES_POSITIONS_FGV.vi"() -> ("out Current Module Positions"=w3326:T11[])  [unwired: 10 in, 1 out]
        n1977 = call "SWERVE_DRIVE_GET_GYRO.vi"() -> ("Gyro Heading Radians"=w3328:dbl)  [unwired: 11 in]
        n1978 = call "SWERVE_DRIVE_GET_GYRO.vi"() -> ("Gyro Heading Radians"=w3333:dbl)  [unwired: 11 in]
        n1979 = call <vilib>:"Rotation2d_CreateAngle.vi"("Angle"=w3328) -> ("ROTATION"=w3327:T9)  [unwired: 10 in]
        n1980 = call "SWERVE_DRIVE_SET_SPEED_DEMAND.vi"("Drv Rotation Orentation Dmd"=w3333, "Drv Angular Vel Dmd"=w3334, "Drv Y Vel Dmd"=w3334, "Drv X Vel Dmd"=w3334) -> ()  [unwired: 8 in]
        n1981 = call "SWERVE_TRAJECTORY_BEGIN.vi"("ABS Odo Initialize"=w3332, "gyroAngle"=w3327, "Module Positions"=w3326, "Trajectory File Name"=w3329) -> ()  [unwired: 8 in]
      }
      n1982 = while {
        tunnel: w3195 -> [w3311]
        tunnel: [w3311] -> w3197
        stop <- w3303 stop-if-true
        # "Shoot Preload"
        n1983 = Wait (ms)(milliseconds to wait=u32 20) -> ()  [unwired: 1 out]
        n1984 = call-poly <vilib>:"NT Read Value.vi"("default value"=0.0, "name"="Shooter/Speed_RPM Act") -> ("value"=w3306:dbl)  [unwired: 7 in, 2 out]
        n1985 = call-poly <vilib>:"NT Write Value.vi"("value"="Shoot Mode" ("default value"), "name"="Robot State") -> ()  [unwired: 9 in, 1 out]
        n1986 = Greater?(x=w3306, y=2500.0) -> (0:w3303:bool)
        n1987 = case shown="True" w3303 {
          frame False {
            n1988 = call-poly <vilib>:"NT Write Value.vi"("value"="Stop" ("default value"), "name"="Intake/Trigger Status") -> ()  [unwired: 9 in, 1 out]
          }
          frame True {
            n1989 = call-poly <vilib>:"NT Write Value.vi"("value"="ToShooter" ("default value"), "name"="Intake/Trigger Status") -> ()  [unwired: 9 in, 1 out]
          }
        }
      }
      n1990 = while {
        tunnel: w3197 -> [w3302]
        tunnel: [w3302] -> w3196
        i -> [w3300]
        stop <- w3299 stop-if-true
        # "Wait until shooting finishes"
        n1991 = Equal To 0?(x=w3300) -> (x = 0?=w3299:bool)
        n1992 = Wait (ms)(milliseconds to wait=u32 300) -> ()  [unwired: 1 out]
      }
      n1993 = while {
        tunnel: w3196 -> [w3368]
        tunnel: [w3368] -> w3198
        i -> [w3367]
        stop <- w3350 stop-if-true
        w3351 = TRUE  # ABS_Traj ?
        w3359 = TRUE  # EnableClosedLoop
        w3357 = FALSE  # Reverse
        w3361 = TRUE  # Follow Orientation
        n1994 = Equal To 0?(x=w3367) -> (x = 0?=w3358:bool)
        n1995 = call "SWERVE_DRIVE_GET_SPEED_DEMAND.vi"() -> ("Drv Rotation Orentation Dmd"=w3366:dbl)  [unwired: 8 in, 3 out]
        n1996 = call "SWERVE_DRIVE_GET_GYRO.vi"() -> ("Gyro Heading Radians"=w3356:dbl)  [unwired: 11 in]
        n1997 = Wait Until Next ms Multiple(millisecond multiple=u32 20 ("milliseconds to wait")) -> ()  [unwired: 1 out]
        n1998 = call "SWERVE_TRAJECTORY_EXECUTE.vi"("EnableClosedLoop"=w3359, "ABS_Traj ?"=w3351, "Init"=w3358, "Reverse"=w3357, "Follow Orientation"=w3361, "Gyro Heading\nRAD"=w3356) -> ("AtReference"=w3352:bool, "OutputTRAJ_STATE"=w3353:T12, "Error and Corr"=w3354:T13, "Chassis Velocity Target"=w3360:T14, "Orientation Target"=w3355:dbl)  [unwired: 1 in]
        n1999 = Select(t=w3356, s=w3361, f=w3366) -> (s? t:f=w3362:dbl)
        n2000 = call "SWERVE_TRAJECTORY_SET_CLOSED_LOOP.vi"("AUTO_CLOSED_LOOP"=w3359) -> ()  [unwired: 11 in]
        n2001 = call "SWERVE_TRAJECTORY_UPDATE_DIAG_INFO.vi"("AtReference"=w3352, "OutputTRAJ_STATE"=w3353, "Error and Corr"=w3354, "Orientation Target"=w3355) -> ()  [unwired: 8 in]
        n2002 = Unbundle By Name(w3360) -> ("vX"=w3365:dbl, "vY"=w3364:dbl, "vOmega"=w3363:dbl)
        n2003 = global read "SWERVE_TRAJECTORY_GLOBALS.vi" "Traj_Total_Time"() -> (w3344:dbl)
        n2004 = Unbundle By Name(w3353) -> ("TimeSeconds"=w3343:dbl)
        n2005 = call "SWERVE_DRIVE_SET_SPEED_DEMAND.vi"("Drv Rotation Orentation Dmd"=w3362, "Drv Angular Vel Dmd"=w3363, "Drv Y Vel Dmd"=w3364, "Drv X Vel Dmd"=w3365) -> ()  [unwired: 8 in]
        n2006 = Equal?(x=w3343, y=w3344) -> (x = y?=w3350:bool)
        n2007 = call-poly <vilib>:"NT Read Value.vi"("name"="Shooter/Limit R") -> ("value"=w3349:bool)  [unwired: 8 in, 2 out]
        n2008 = call-poly <vilib>:"NT Read Value.vi"("name"="Shooter/Limit L") -> ("value"=w3348:bool)  [unwired: 8 in, 2 out]
        n2009 = Not Or(1:w3349, 2:w3348) -> (0:w3345:bool)
        n2010 = Select(t="FromIntake" ("default value"), s=w3345, f="Stop" ("default value")) -> (s? t:f=w3339:string)
        n2011 = call-poly <vilib>:"NT Write Value.vi"("value"=w3339, "name"="Intake/Trigger Status") -> ()  [unwired: 9 in, 1 out]
      }
      n2012 = while {
        tunnel: w3198 -> [w3325]
        tunnel: [w3325] -> w3194
        i -> [w3323]
        stop <- w3322 stop-if-true
        w3321 = 0.0 ("Drv X Vel Dmd")
        n2013 = Not Equal To 0?(x=w3323) -> (x != 0?=w3322:bool)
        n2014 = Wait (ms)(milliseconds to wait=u32 20) -> ()  [unwired: 1 out]
        n2015 = call "SWERVE_DRIVE_MODULE_STATES_POSITIONS_FGV.vi"() -> ("out Current Module Positions"=w3317:T11[])  [unwired: 10 in, 1 out]
        n2016 = call "SWERVE_DRIVE_GET_GYRO.vi"() -> ("Gyro Heading Radians"=w3319:dbl)  [unwired: 11 in]
        n2017 = call "SWERVE_DRIVE_GET_GYRO.vi"() -> ("Gyro Heading Radians"=w3320:dbl)  [unwired: 11 in]
        n2018 = call <vilib>:"Rotation2d_CreateAngle.vi"("Angle"=w3319) -> ("ROTATION"=w3318:T9)  [unwired: 10 in]
        n2019 = call "SWERVE_DRIVE_SET_SPEED_DEMAND.vi"("Drv Rotation Orentation Dmd"=w3320, "Drv Angular Vel Dmd"=w3321, "Drv Y Vel Dmd"=w3321, "Drv X Vel Dmd"=w3321) -> ()  [unwired: 8 in]
        n2020 = call "SWERVE_TRAJECTORY_BEGIN.vi"("gyroAngle"=w3318, "Module Positions"=w3317, "Trajectory File Name"="Path Demo.wpilib.csv") -> ()  [unwired: 9 in]
      }
      n2021 = while {
        tunnel: w3194 -> [w3294]
        tunnel: [w3294] -> w3193
        i -> [w3286]
        stop <- w3283 stop-if-true
        n2022 = call-poly <vilib>:"NT Read Value.vi"("name"="Shooter/Angle_Deg Act") -> ("value"=w3291:dbl)  [unwired: 8 in, 2 out]
        n2023 = call-poly <vilib>:"NT Read Value.vi"("name"="Shooter/Angle_Deg Dmd") -> ("value"=w3290:dbl)  [unwired: 8 in, 2 out]
        n2024 = Greater?(x=w3286, y=25) -> (0:w3284:bool)
        n2025 = call <vilib>:"Util_ApproxEquals.vi"("Tolerance"=4.5, "Value 2"=w3290, "Value 1"=w3291) -> ("ApproxEquals"=w3287:bool)  [unwired: 8 in]
        n2026 = Or(x=w3287, y=w3284) -> (x .or. y?=w3283:bool)
        n2027 = case shown="True" w3283 {
          frame False {
            n2028 = call-poly <vilib>:"NT Write Value.vi"("value"="Stop" ("default value"), "name"="Intake/Trigger Status") -> ()  [unwired: 9 in, 1 out]
          }
          frame True {
            n2029 = call-poly <vilib>:"NT Write Value.vi"("value"="ToShooter" ("default value"), "name"="Intake/Trigger Status") -> ()  [unwired: 9 in, 1 out]
          }
        }
        n2030 = Wait (ms)(milliseconds to wait=u32 20) -> ()  [unwired: 1 out]
      }
      n2031 = while {
        tunnel: w3193 -> [w3271]
        tunnel: [w3271] -> w3192
        i -> [w3269]
        stop <- w3268 stop-if-true
        # "Wait until shooting finishes"
        n2032 = Equal To 0?(x=w3269) -> (x = 0?=w3268:bool)
        n2033 = Wait (ms)(milliseconds to wait=u32 1000) -> ()  [unwired: 1 out]
        n2034 = call-poly <vilib>:"NT Write Value.vi"("value"="ToShooter" ("default value"), "name"="Intake/Trigger Status") -> ()  [unwired: 9 in, 1 out]
      }
      n2035 = while {
        tunnel: w3192 -> [w3282]
        tunnel: [w3282] -> w3191
        i -> [w3280]
        stop <- w3279 stop-if-true
        w3276 = FALSE  # ABS Odo Initialize
        w3278 = 0.0 ("Drv X Vel Dmd")
        n2036 = Not Equal To 0?(x=w3280) -> (x != 0?=w3279:bool)
        n2037 = Wait (ms)(milliseconds to wait=u32 20) -> ()  [unwired: 1 out]
        n2038 = call "SWERVE_DRIVE_MODULE_STATES_POSITIONS_FGV.vi"() -> ("out Current Module Positions"=w3273:T11[])  [unwired: 10 in, 1 out]
        n2039 = call "SWERVE_DRIVE_GET_GYRO.vi"() -> ("Gyro Heading Radians"=w3275:dbl)  [unwired: 11 in]
        n2040 = call "SWERVE_DRIVE_GET_GYRO.vi"() -> ("Gyro Heading Radians"=w3277:dbl)  [unwired: 11 in]
        n2041 = call <vilib>:"Rotation2d_CreateAngle.vi"("Angle"=w3275) -> ("ROTATION"=w3274:T9)  [unwired: 10 in]
        n2042 = call "SWERVE_DRIVE_SET_SPEED_DEMAND.vi"("Drv Rotation Orentation Dmd"=w3277, "Drv Angular Vel Dmd"=w3278, "Drv Y Vel Dmd"=w3278, "Drv X Vel Dmd"=w3278) -> ()  [unwired: 8 in]
        n2043 = call "SWERVE_TRAJECTORY_BEGIN.vi"("ABS Odo Initialize"=w3276, "gyroAngle"=w3274, "Module Positions"=w3273, "Trajectory File Name"="Route B2 R Path 2.path") -> ()  [unwired: 8 in]
      }
      n2044 = while {
        tunnel: [w3263] -> w3189
        tunnel: w3191 -> [w3263]
        i -> [w3262]
        stop <- w3261 stop-if-true
        n2045 = Equal To 0?(x=w3262) -> (x = 0?=w3261:bool)
        n2046 = call-poly <vilib>:"NT Write Value.vi"("value"="Reset" ("default value"), "name"="Robot State") -> ()  [unwired: 9 in, 1 out]
      }
      n2047 = while {
        tunnel: w3189 -> [w3243]
        tunnel: [w3243] -> w3190
        i -> [w3217]
        stop <- w3226 stop-if-true
        w3227 = TRUE  # ABS_Traj ?
        w3235 = TRUE  # EnableClosedLoop
        w3233 = FALSE  # Reverse
        w3237 = TRUE  # Follow Orientation
        n2048 = call "SWERVE_DRIVE_GET_SPEED_DEMAND.vi"() -> ("Drv Rotation Orentation Dmd"=w3242:dbl)  [unwired: 8 in, 3 out]
        n2049 = call "SWERVE_DRIVE_GET_GYRO.vi"() -> ("Gyro Heading Radians"=w3232:dbl)  [unwired: 11 in]
        n2050 = Wait (ms)(milliseconds to wait=u32 20) -> ()  [unwired: 1 out]
        n2051 = Equal?(x=w3217, y=105) -> (x = y?=w3222:bool)
        n2052 = Equal To 0?(x=w3217) -> (x = 0?=w3234:bool)
        n2053 = case shown="True" w3222 {
          frame False {
          }
          frame True {
            n2054 = call-poly <vilib>:"NT Write Value.vi"("value"="Intake Mode" ("default value"), "name"="Robot State") -> ()  [unwired: 9 in, 1 out]
          }
        }
        n2055 = call "SWERVE_TRAJECTORY_EXECUTE.vi"("EnableClosedLoop"=w3235, "ABS_Traj ?"=w3227, "Init"=w3234, "Reverse"=w3233, "Follow Orientation"=w3237, "Gyro Heading\nRAD"=w3232) -> ("AtReference"=w3228:bool, "OutputTRAJ_STATE"=w3229:T12, "Error and Corr"=w3230:T13, "Chassis Velocity Target"=w3236:T14, "Orientation Target"=w3231:dbl)  [unwired: 1 in]
        n2056 = Select(t=w3232, s=w3237, f=w3242) -> (s? t:f=w3238:dbl)
        n2057 = call "SWERVE_TRAJECTORY_SET_CLOSED_LOOP.vi"("AUTO_CLOSED_LOOP"=w3235) -> ()  [unwired: 11 in]
        n2058 = call "SWERVE_TRAJECTORY_UPDATE_DIAG_INFO.vi"("AtReference"=w3228, "OutputTRAJ_STATE"=w3229, "Error and Corr"=w3230, "Orientation Target"=w3231) -> ()  [unwired: 8 in]
        n2059 = Equal?(x=w3217, y=260) -> (x = y?=w3220:bool)
        n2060 = Unbundle By Name(w3236) -> ("vX"=w3241:dbl, "vY"=w3240:dbl, "vOmega"=w3239:dbl)
        n2061 = case shown="True" w3220 {
          frame False {
          }
          frame True {
            n2062 = call-poly <vilib>:"NT Write Value.vi"("value"="Reset" ("default value"), "name"="Robot State") -> ()  [unwired: 9 in, 1 out]
          }
        }
        n2063 = global read "SWERVE_TRAJECTORY_GLOBALS.vi" "Traj_Total_Time"() -> (w3224:dbl)
        n2064 = Unbundle By Name(w3229) -> ("TimeSeconds"=w3225:dbl)
        n2065 = call "SWERVE_DRIVE_SET_SPEED_DEMAND.vi"("Drv Rotation Orentation Dmd"=w3238, "Drv Angular Vel Dmd"=w3239, "Drv Y Vel Dmd"=w3240, "Drv X Vel Dmd"=w3241) -> ()  [unwired: 8 in]
        n2066 = Equal?(x=w3225, y=w3224) -> (x = y?=w3226:bool)
        n2067 = Equal?(x=w3217, y=320) -> (x = y?=w3218:bool)
        n2068 = case shown="True" w3218 {
          frame False {
          }
          frame True {
            n2069 = call-poly <vilib>:"NT Write Value.vi"("value"="Shoot Mode" ("default value"), "name"="Robot State") -> ()  [unwired: 9 in, 1 out]
          }
        }
      }
      n2070 = while {
        tunnel: w3190 -> [w3260]
        tunnel: [w3260] -> w3188
        i -> [w3258]
        stop <- w3257 stop-if-true
        w3256 = 0.0 ("Drv X Vel Dmd")
        n2071 = Not Equal To 0?(x=w3258) -> (x != 0?=w3257:bool)
        n2072 = Wait (ms)(milliseconds to wait=u32 20) -> ()  [unwired: 1 out]
        n2073 = call "SWERVE_DRIVE_MODULE_STATES_POSITIONS_FGV.vi"() -> ("out Current Module Positions"=w3252:T11[])  [unwired: 10 in, 1 out]
        n2074 = call "SWERVE_DRIVE_GET_GYRO.vi"() -> ("Gyro Heading Radians"=w3254:dbl)  [unwired: 11 in]
        n2075 = call "SWERVE_DRIVE_GET_GYRO.vi"() -> ("Gyro Heading Radians"=w3255:dbl)  [unwired: 11 in]
        n2076 = call <vilib>:"Rotation2d_CreateAngle.vi"("Angle"=w3254) -> ("ROTATION"=w3253:T9)  [unwired: 10 in]
        n2077 = call "SWERVE_DRIVE_SET_SPEED_DEMAND.vi"("Drv Rotation Orentation Dmd"=w3255, "Drv Angular Vel Dmd"=w3256, "Drv Y Vel Dmd"=w3256, "Drv X Vel Dmd"=w3256) -> ()  [unwired: 8 in]
        n2078 = call "SWERVE_TRAJECTORY_BEGIN.vi"("gyroAngle"=w3253, "Module Positions"=w3252, "Trajectory File Name"="Path Demo.wpilib.csv") -> ()  [unwired: 9 in]
      }
      n2079 = while {
        tunnel: w3188 -> [w3200]
        tunnel: [w3200] -> _
        i -> [w3205]
        stop <- FALSE stop-if-true
        # "Shoot early if shooter angle tolerance is meeted"
        n2080 = Greater?(x=w3205, y=50) -> (0:w3203:bool)
        n2081 = Wait (ms)(milliseconds to wait=u32 20) -> ()  [unwired: 1 out]
        n2082 = call-poly <vilib>:"NT Read Value.vi"("name"="Shooter/Angle_Deg Act") -> ("value"=w3206:dbl)  [unwired: 8 in, 2 out]
        n2083 = call-poly <vilib>:"NT Read Value.vi"("name"="Shooter/Angle_Deg Dmd") -> ("value"=w3210:dbl)  [unwired: 8 in, 2 out]
        n2084 = call <vilib>:"Util_ApproxEquals.vi"("Tolerance"=5.5, "Value 2"=w3210, "Value 1"=w3206) -> ("ApproxEquals"=w3208:bool)  [unwired: 8 in]
        n2085 = Compound Arithmetic op=OR(w3208, w3203) -> (w3202:bool)
        n2086 = case shown="True" w3202 {
          frame False {
            n2087 = call-poly <vilib>:"NT Write Value.vi"("value"="Stop" ("default value"), "name"="Intake/Trigger Status") -> ()  [unwired: 9 in, 1 out]
          }
          frame True {
            n2088 = call-poly <vilib>:"NT Write Value.vi"("value"="ToShooter" ("default value"), "name"="Intake/Trigger Status") -> ()  [unwired: 9 in, 1 out]
          }
        }
      }
    }
    frame "Route B1 Blue" {
      w3377 = errorcluster {"status"=FALSE, "code"=0, "source"=""}  # Start Error Flow
      # "Trigger events when robot pose approx equals event pose\n(The two while loops below ends when the path above is ended)"
      # "Shoot Preload"
      n2089 = while {
        tunnel: w3377 -> [w3483]
        tunnel: [w3483] -> w3373
        i -> [w3481]
        stop <- w3480 stop-if-true
        w3477 = TRUE  # ABS Odo Initialize
        w3479 = 0.0 ("Drv X Vel Dmd")
        n2090 = Not Equal To 0?(x=w3481) -> (x != 0?=w3480:bool)
        n2091 = Wait (ms)(milliseconds to wait=u32 20) -> ()  [unwired: 1 out]
        n2092 = call-poly <vilib>:"NT Read Value.vi"("default value"="Path_Testing_1.path" ("Trajectory File Name"), "name"="Initial Path") -> ("value"=w3474:string)  [unwired: 7 in, 2 out]
        n2093 = call "SWERVE_DRIVE_MODULE_STATES_POSITIONS_FGV.vi"() -> ("out Current Module Positions"=w3471:T11[])  [unwired: 10 in, 1 out]
        n2094 = call "SWERVE_DRIVE_GET_GYRO.vi"() -> ("Gyro Heading Radians"=w3473:dbl)  [unwired: 11 in]
        n2095 = call "SWERVE_DRIVE_GET_GYRO.vi"() -> ("Gyro Heading Radians"=w3478:dbl)  [unwired: 11 in]
        n2096 = call <vilib>:"Rotation2d_CreateAngle.vi"("Angle"=w3473) -> ("ROTATION"=w3472:T9)  [unwired: 10 in]
        n2097 = call "SWERVE_DRIVE_SET_SPEED_DEMAND.vi"("Drv Rotation Orentation Dmd"=w3478, "Drv Angular Vel Dmd"=w3479, "Drv Y Vel Dmd"=w3479, "Drv X Vel Dmd"=w3479) -> ()  [unwired: 8 in]
        n2098 = call "SWERVE_TRAJECTORY_BEGIN.vi"("ABS Odo Initialize"=w3477, "gyroAngle"=w3472, "Module Positions"=w3471, "Trajectory File Name"=w3474) -> ()  [unwired: 8 in]
      }
      n2099 = while {
        tunnel: w3373 -> [w3456]
        tunnel: [w3456] -> w3375
        stop <- w3448 stop-if-true
        n2100 = Wait (ms)(milliseconds to wait=u32 20) -> ()  [unwired: 1 out]
        n2101 = call-poly <vilib>:"NT Read Value.vi"("default value"=0.0, "name"="Shooter/Speed_RPM Act") -> ("value"=w3451:dbl)  [unwired: 7 in, 2 out]
        n2102 = call-poly <vilib>:"NT Write Value.vi"("value"="Shoot Mode" ("default value"), "name"="Robot State") -> ()  [unwired: 9 in, 1 out]
        n2103 = Greater?(x=w3451, y=4000.0) -> (0:w3448:bool)
        n2104 = case shown="False" w3448 {
          frame False {
            n2105 = call-poly <vilib>:"NT Write Value.vi"("value"="Stop" ("default value"), "name"="Intake/Trigger Status") -> ()  [unwired: 9 in, 1 out]
          }
          frame True {
            n2106 = call-poly <vilib>:"NT Write Value.vi"("value"="ToShooter" ("default value"), "name"="Intake/Trigger Status") -> ()  [unwired: 9 in, 1 out]
          }
        }
      }
      n2107 = while {
        tunnel: w3375 -> [w3447]
        tunnel: [w3447] -> w3374
        i -> [w3445]
        stop <- w3444 stop-if-true
        # "Wait until shooting finishes"
        n2108 = Equal To 0?(x=w3445) -> (x = 0?=w3444:bool)
        n2109 = Wait (ms)(milliseconds to wait=u32 1000) -> ()  [unwired: 1 out]
      }
      n2110 = while {
        tunnel: [w3441] -> w3372
        tunnel: w3374 -> [w3441]
        i -> [w3440]
        stop <- w3439 stop-if-true
        n2111 = Equal To 0?(x=w3440) -> (x = 0?=w3439:bool)
        n2112 = call-poly <vilib>:"NT Write Value.vi"("value"="Intake Mode" ("default value"), "name"="Robot State") -> ()  [unwired: 9 in, 1 out]
      }
      n2113 = while {
        tunnel: w3372 -> [w3504]
        tunnel: [w3504] -> w3376
        i -> [w3502]
        stop <- w3484 stop-if-true
        w3486 = TRUE  # ABS_Traj ?
        w3494 = TRUE  # EnableClosedLoop
        w3492 = FALSE  # Reverse
        w3496 = TRUE  # Follow Orientation
        n2114 = Equal To 0?(x=w3502) -> (x = 0?=w3493:bool)
        n2115 = call "SWERVE_DRIVE_GET_SPEED_DEMAND.vi"() -> ("Drv Rotation Orentation Dmd"=w3501:dbl)  [unwired: 8 in, 3 out]
        n2116 = call "SWERVE_DRIVE_GET_GYRO.vi"() -> ("Gyro Heading Radians"=w3491:dbl)  [unwired: 11 in]
        n2117 = Wait Until Next ms Multiple(millisecond multiple=u32 20 ("milliseconds to wait")) -> ()  [unwired: 1 out]
        n2118 = call "SWERVE_TRAJECTORY_EXECUTE.vi"("EnableClosedLoop"=w3494, "ABS_Traj ?"=w3486, "Init"=w3493, "Reverse"=w3492, "Follow Orientation"=w3496, "Gyro Heading\nRAD"=w3491) -> ("AtReference"=w3487:bool, "OutputTRAJ_STATE"=w3488:T12, "Error and Corr"=w3489:T13, "Chassis Velocity Target"=w3495:T14, "Orientation Target"=w3490:dbl)  [unwired: 1 in]
        n2119 = Select(t=w3491, s=w3496, f=w3501) -> (s? t:f=w3497:dbl)
        n2120 = call "SWERVE_TRAJECTORY_SET_CLOSED_LOOP.vi"("AUTO_CLOSED_LOOP"=w3494) -> ()  [unwired: 11 in]
        n2121 = call "SWERVE_TRAJECTORY_UPDATE_DIAG_INFO.vi"("AtReference"=w3487, "OutputTRAJ_STATE"=w3488, "Error and Corr"=w3489, "Orientation Target"=w3490) -> ()  [unwired: 8 in]
        n2122 = global read "SWERVE_TRAJECTORY_GLOBALS.vi" "Traj_Total_Time"() -> (w3505:dbl)
        n2123 = Unbundle By Name(w3488) -> ("TimeSeconds"=w3503:dbl)
        n2124 = Unbundle By Name(w3495) -> ("vX"=w3500:dbl, "vY"=w3499:dbl, "vOmega"=w3498:dbl)
        n2125 = Equal?(x=w3503, y=w3505) -> (x = y?=w3484:bool)
        n2126 = call "SWERVE_DRIVE_SET_SPEED_DEMAND.vi"("Drv Rotation Orentation Dmd"=w3497, "Drv Angular Vel Dmd"=w3498, "Drv Y Vel Dmd"=w3499, "Drv X Vel Dmd"=w3500) -> ()  [unwired: 8 in]
        n2127 = call-poly <vilib>:"NT Write Value.vi"("value"=w3484, "name"="Auto/Path End") -> ()  [unwired: 9 in, 1 out]
      }
      n2128 = while {
        tunnel: w3372 -> [w3410]
        tunnel: [w3410] -> _
        tunnel: cluster{"X":dbl, "Y":dbl, "Event":string}[] [{"X"=2.507, "Y"=5.551, "Event"="Shoot"}, {"X"=2.507, "Y"=5.551, "Event"="Trigger"}, {"X"=4.674, "Y"=6.244, "Event"="Intake"}] -> [w3406]
        stop <- w3404 stop-if-true
        n2129 = call "SWERVE_ODOM_ABS_FGV.vi"() -> ("out SWERVE_DRIVE_ODOMETRY"=w3402:T25)  [unwired: 10 in, 1 out]
        n2130 = Unbundle By Name(w3402) -> ("POSE.TRANSLATION.X"=w3409:dbl, "POSE.TRANSLATION.Y"=w3408:dbl)
        n2131 = call-poly <vilib>:"NT Read Value.vi"("default value"=FALSE, "name"="Auto/Path End") -> ("value"=w3404:bool)  [unwired: 7 in, 2 out]
        n2132 = Wait (ms)(milliseconds to wait=u32 20) -> ()  [unwired: 1 out]
        n2133 = Build Array(w3409, w3408) -> (w3407:dbl[])
        n2134 = for {
          tunnel: w3407 -> [w3418]
          tunnel: w3406 -> [w3417] mode=indexing
          n2135 = Unbundle(w3417) -> ("X"=w3416:dbl, "Y"=w3415:dbl, "Event"=w3411:string)
          n2136 = Build Array(w3416, w3415) -> (w3414:dbl[])
          n2137 = for {
            tunnel: w3418 -> [w3424] mode=indexing
            tunnel: [w3422] -> w3413 mode=indexing
            tunnel: w3414 -> [w3421] mode=indexing
            n2138 = call <vilib>:"Util_ApproxEquals.vi"("Tolerance"=0.15, "Value 2"=w3421, "Value 1"=w3424) -> ("ApproxEquals"=w3422:bool)  [unwired: 8 in]
          }
          n2139 = And Array Elements(Boolean array=w3413) -> (logical AND=w3412:bool)
          n2140 = case shown="True" w3412 {
            tunnel: w3411 -> [_ w3419]
            frame False {
            }
            frame True {
              n2141 = call-poly <vilib>:"NT Write Value.vi"("value"=w3419, "name"="Auto State") -> ()  [unwired: 9 in, 1 out]
            }
          }
        }
      }
      n2142 = while {
        tunnel: w3372 -> [w3429]
        tunnel: [w3429] -> _
        stop <- w3427 stop-if-true
        n2143 = call-poly <vilib>:"NT Read Value.vi"("default value"="None", "name"="Auto State") -> ("value"=w3431:string)  [unwired: 7 in, 2 out]
        n2144 = call-poly <vilib>:"NT Read Value.vi"("default value"=FALSE, "name"="Auto/Path End") -> ("value"=w3427:bool)  [unwired: 7 in, 2 out]
        n2145 = Wait (ms)(milliseconds to wait=u32 20) -> ()  [unwired: 1 out]
        n2146 = case shown="\"Trigger\"" w3431 {
          frame "None", Default {
          }
          frame "Shoot" {
            n2147 = call-poly <vilib>:"NT Write Value.vi"("value"="Shoot Mode" ("default value"), "name"="Robot State") -> ()  [unwired: 9 in, 1 out]
          }
          frame "Intake" {
            n2148 = call-poly <vilib>:"NT Write Value.vi"("value"="Intake Mode" ("default value"), "name"="Robot State") -> ()  [unwired: 9 in, 1 out]
          }
          frame "Trigger" {
            n2149 = call-poly <vilib>:"NT Write Value.vi"("value"="ToShooter" ("default value"), "name"="Intake/Trigger Status") -> ()  [unwired: 9 in, 1 out]
          }
        }
      }
      n2150 = while {
        tunnel: w3376 -> [w3470]
        tunnel: [w3470] -> w3371
        i -> [w3468]
        stop <- w3467 stop-if-true
        w3466 = 0.0 ("Drv X Vel Dmd")
        n2151 = Not Equal To 0?(x=w3468) -> (x != 0?=w3467:bool)
        n2152 = Wait (ms)(milliseconds to wait=u32 20) -> ()  [unwired: 1 out]
        n2153 = call "SWERVE_DRIVE_MODULE_STATES_POSITIONS_FGV.vi"() -> ("out Current Module Positions"=w3462:T11[])  [unwired: 10 in, 1 out]
        n2154 = call "SWERVE_DRIVE_GET_GYRO.vi"() -> ("Gyro Heading Radians"=w3464:dbl)  [unwired: 11 in]
        n2155 = call "SWERVE_DRIVE_GET_GYRO.vi"() -> ("Gyro Heading Radians"=w3465:dbl)  [unwired: 11 in]
        n2156 = call <vilib>:"Rotation2d_CreateAngle.vi"("Angle"=w3464) -> ("ROTATION"=w3463:T9)  [unwired: 10 in]
        n2157 = call "SWERVE_DRIVE_SET_SPEED_DEMAND.vi"("Drv Rotation Orentation Dmd"=w3465, "Drv Angular Vel Dmd"=w3466, "Drv Y Vel Dmd"=w3466, "Drv X Vel Dmd"=w3466) -> ()  [unwired: 8 in]
        n2158 = call "SWERVE_TRAJECTORY_BEGIN.vi"("gyroAngle"=w3463, "Module Positions"=w3462, "Trajectory File Name"="Path Demo.wpilib.csv") -> ()  [unwired: 9 in]
      }
      n2159 = while {
        tunnel: w3371 -> [w3396]
        tunnel: [w3396] -> _
        stop <- FALSE stop-if-true
        w3380 = 0.0 ("Drv X Vel Dmd")
        n2160 = call-poly <vilib>:"NT Write Value.vi"("value"="Shoot Mode" ("default value"), "name"="Robot State") -> ()  [unwired: 9 in, 1 out]
        n2161 = call-poly <vilib>:"NT Read Value.vi"("name"="Shooter/Angle_Deg Act") -> ("value"=w3393:dbl)  [unwired: 8 in, 2 out]
        n2162 = call-poly <vilib>:"NT Read Value.vi"("name"="Shooter/Angle_Deg Dmd") -> ("value"=w3392:dbl)  [unwired: 8 in, 2 out]
        n2163 = call-poly <vilib>:"NT Read Value.vi"("name"="Shooter/Corrected Theta") -> ("value"=w3382:dbl)  [unwired: 8 in, 2 out]
        n2164 = call-poly <vilib>:"NT Read Value.vi"("name"="/limelight/tv") -> ("value"=w3384:dbl)  [unwired: 8 in, 2 out]
        n2165 = Not Equal To 0?(x=w3384) -> (x != 0?=w3383:bool)
        n2166 = call "SWERVE_DRIVE_GET_GYRO.vi"() -> ("Gyro Heading Radians"=w3378:dbl)  [unwired: 11 in]
        n2167 = call <vilib>:"Util_ApproxEquals.vi"("Tolerance"=2.0, "Value 2"=w3392, "Value 1"=w3393) -> ("ApproxEquals"=w3388:bool)  [unwired: 8 in]
        n2168 = Select(t=w3382, s=w3383, f=w3378) -> (s? t:f=w3381:dbl)
        n2169 = case shown="True" w3388 {
          frame False {
            n2170 = call-poly <vilib>:"NT Write Value.vi"("value"="Stop" ("default value"), "name"="Intake/Trigger Status") -> ()  [unwired: 9 in, 1 out]
          }
          frame True {
            n2171 = call-poly <vilib>:"NT Write Value.vi"("value"="ToShooter" ("default value"), "name"="Intake/Trigger Status") -> ()  [unwired: 9 in, 1 out]
          }
        }
        n2172 = call "SWERVE_DRIVE_SET_SPEED_DEMAND.vi"("Drv Rotation Orentation Dmd"=w3381, "Drv Angular Vel Dmd"=w3380, "Drv Y Vel Dmd"=w3380, "Drv X Vel Dmd"=w3380) -> ()  [unwired: 8 in]
        n2173 = Wait (ms)(milliseconds to wait=u32 20) -> ()  [unwired: 1 out]
      }
    }
    frame "Route B1 Red" {
      w3514 = errorcluster {"status"=FALSE, "code"=0, "source"=""}  # Start Error Flow
      # "Trigger events when robot pose approx equals event pose\n(The two while loops below ends when the path above is ended)"
      # "Shoot Preload"
      n2174 = while {
        tunnel: w3514 -> [w3620]
        tunnel: [w3620] -> w3510
        i -> [w3618]
        stop <- w3617 stop-if-true
        w3614 = TRUE  # ABS Odo Initialize
        w3616 = 0.0 ("Drv X Vel Dmd")
        n2175 = Not Equal To 0?(x=w3618) -> (x != 0?=w3617:bool)
        n2176 = Wait (ms)(milliseconds to wait=u32 20) -> ()  [unwired: 1 out]
        n2177 = call-poly <vilib>:"NT Read Value.vi"("default value"="Path_Testing_1.path" ("Trajectory File Name"), "name"="Initial Path") -> ("value"=w3611:string)  [unwired: 7 in, 2 out]
        n2178 = call "SWERVE_DRIVE_MODULE_STATES_POSITIONS_FGV.vi"() -> ("out Current Module Positions"=w3608:T11[])  [unwired: 10 in, 1 out]
        n2179 = call "SWERVE_DRIVE_GET_GYRO.vi"() -> ("Gyro Heading Radians"=w3610:dbl)  [unwired: 11 in]
        n2180 = call "SWERVE_DRIVE_GET_GYRO.vi"() -> ("Gyro Heading Radians"=w3615:dbl)  [unwired: 11 in]
        n2181 = call <vilib>:"Rotation2d_CreateAngle.vi"("Angle"=w3610) -> ("ROTATION"=w3609:T9)  [unwired: 10 in]
        n2182 = call "SWERVE_DRIVE_SET_SPEED_DEMAND.vi"("Drv Rotation Orentation Dmd"=w3615, "Drv Angular Vel Dmd"=w3616, "Drv Y Vel Dmd"=w3616, "Drv X Vel Dmd"=w3616) -> ()  [unwired: 8 in]
        n2183 = call "SWERVE_TRAJECTORY_BEGIN.vi"("ABS Odo Initialize"=w3614, "gyroAngle"=w3609, "Module Positions"=w3608, "Trajectory File Name"=w3611) -> ()  [unwired: 8 in]
      }
      n2184 = while {
        tunnel: w3510 -> [w3593]
        tunnel: [w3593] -> w3512
        stop <- w3585 stop-if-true
        n2185 = Wait (ms)(milliseconds to wait=u32 20) -> ()  [unwired: 1 out]
        n2186 = call-poly <vilib>:"NT Read Value.vi"("default value"=0.0, "name"="Shooter/Speed_RPM Act") -> ("value"=w3588:dbl)  [unwired: 7 in, 2 out]
        n2187 = call-poly <vilib>:"NT Write Value.vi"("value"="Shoot Mode" ("default value"), "name"="Robot State") -> ()  [unwired: 9 in, 1 out]
        n2188 = Greater?(x=w3588, y=4000.0) -> (0:w3585:bool)
        n2189 = case shown="False" w3585 {
          frame False {
            n2190 = call-poly <vilib>:"NT Write Value.vi"("value"="Stop" ("default value"), "name"="Intake/Trigger Status") -> ()  [unwired: 9 in, 1 out]
          }
          frame True {
            n2191 = call-poly <vilib>:"NT Write Value.vi"("value"="ToShooter" ("default value"), "name"="Intake/Trigger Status") -> ()  [unwired: 9 in, 1 out]
          }
        }
      }
      n2192 = while {
        tunnel: w3512 -> [w3584]
        tunnel: [w3584] -> w3511
        i -> [w3582]
        stop <- w3581 stop-if-true
        # "Wait until shooting finishes"
        n2193 = Equal To 0?(x=w3582) -> (x = 0?=w3581:bool)
        n2194 = Wait (ms)(milliseconds to wait=u32 1000) -> ()  [unwired: 1 out]
      }
      n2195 = while {
        tunnel: [w3578] -> w3509
        tunnel: w3511 -> [w3578]
        i -> [w3577]
        stop <- w3576 stop-if-true
        n2196 = Equal To 0?(x=w3577) -> (x = 0?=w3576:bool)
        n2197 = call-poly <vilib>:"NT Write Value.vi"("value"="Intake Mode" ("default value"), "name"="Robot State") -> ()  [unwired: 9 in, 1 out]
      }
      n2198 = while {
        tunnel: w3509 -> [w3641]
        tunnel: [w3641] -> w3513
        i -> [w3639]
        stop <- w3621 stop-if-true
        w3623 = TRUE  # ABS_Traj ?
        w3631 = TRUE  # EnableClosedLoop
        w3629 = FALSE  # Reverse
        w3633 = TRUE  # Follow Orientation
        n2199 = Equal To 0?(x=w3639) -> (x = 0?=w3630:bool)
        n2200 = call "SWERVE_DRIVE_GET_SPEED_DEMAND.vi"() -> ("Drv Rotation Orentation Dmd"=w3638:dbl)  [unwired: 8 in, 3 out]
        n2201 = call "SWERVE_DRIVE_GET_GYRO.vi"() -> ("Gyro Heading Radians"=w3628:dbl)  [unwired: 11 in]
        n2202 = Wait Until Next ms Multiple(millisecond multiple=u32 20 ("milliseconds to wait")) -> ()  [unwired: 1 out]
        n2203 = call "SWERVE_TRAJECTORY_EXECUTE.vi"("EnableClosedLoop"=w3631, "ABS_Traj ?"=w3623, "Init"=w3630, "Reverse"=w3629, "Follow Orientation"=w3633, "Gyro Heading\nRAD"=w3628) -> ("AtReference"=w3624:bool, "OutputTRAJ_STATE"=w3625:T12, "Error and Corr"=w3626:T13, "Chassis Velocity Target"=w3632:T14, "Orientation Target"=w3627:dbl)  [unwired: 1 in]
        n2204 = Select(t=w3628, s=w3633, f=w3638) -> (s? t:f=w3634:dbl)
        n2205 = call "SWERVE_TRAJECTORY_SET_CLOSED_LOOP.vi"("AUTO_CLOSED_LOOP"=w3631) -> ()  [unwired: 11 in]
        n2206 = call "SWERVE_TRAJECTORY_UPDATE_DIAG_INFO.vi"("AtReference"=w3624, "OutputTRAJ_STATE"=w3625, "Error and Corr"=w3626, "Orientation Target"=w3627) -> ()  [unwired: 8 in]
        n2207 = global read "SWERVE_TRAJECTORY_GLOBALS.vi" "Traj_Total_Time"() -> (w3642:dbl)
        n2208 = Unbundle By Name(w3625) -> ("TimeSeconds"=w3640:dbl)
        n2209 = Unbundle By Name(w3632) -> ("vX"=w3637:dbl, "vY"=w3636:dbl, "vOmega"=w3635:dbl)
        n2210 = Equal?(x=w3640, y=w3642) -> (x = y?=w3621:bool)
        n2211 = call "SWERVE_DRIVE_SET_SPEED_DEMAND.vi"("Drv Rotation Orentation Dmd"=w3634, "Drv Angular Vel Dmd"=w3635, "Drv Y Vel Dmd"=w3636, "Drv X Vel Dmd"=w3637) -> ()  [unwired: 8 in]
        n2212 = call-poly <vilib>:"NT Write Value.vi"("value"=w3621, "name"="Auto/Path End") -> ()  [unwired: 9 in, 1 out]
      }
      n2213 = while {
        tunnel: w3509 -> [w3547]
        tunnel: [w3547] -> _
        tunnel: cluster{"X":dbl, "Y":dbl, "Event":string}[] [{"X"=14.033, "Y"=5.551, "Event"="Shoot"}, {"X"=14.033, "Y"=5.551, "Event"="Trigger"}, {"X"=11.866, "Y"=6.244, "Event"="Intake"}] -> [w3543]
        stop <- w3541 stop-if-true
        n2214 = call "SWERVE_ODOM_ABS_FGV.vi"() -> ("out SWERVE_DRIVE_ODOMETRY"=w3539:T25)  [unwired: 10 in, 1 out]
        n2215 = Unbundle By Name(w3539) -> ("POSE.TRANSLATION.X"=w3546:dbl, "POSE.TRANSLATION.Y"=w3545:dbl)
        n2216 = call-poly <vilib>:"NT Read Value.vi"("default value"=FALSE, "name"="Auto/Path End") -> ("value"=w3541:bool)  [unwired: 7 in, 2 out]
        n2217 = Wait (ms)(milliseconds to wait=u32 20) -> ()  [unwired: 1 out]
        n2218 = Build Array(w3546, w3545) -> (w3544:dbl[])
        n2219 = for {
          tunnel: w3544 -> [w3555]
          tunnel: w3543 -> [w3554] mode=indexing
          n2220 = Unbundle(w3554) -> ("X"=w3553:dbl, "Y"=w3552:dbl, "Event"=w3548:string)
          n2221 = Build Array(w3553, w3552) -> (w3551:dbl[])
          n2222 = for {
            tunnel: w3555 -> [w3561] mode=indexing
            tunnel: [w3559] -> w3550 mode=indexing
            tunnel: w3551 -> [w3558] mode=indexing
            n2223 = call <vilib>:"Util_ApproxEquals.vi"("Tolerance"=0.15, "Value 2"=w3558, "Value 1"=w3561) -> ("ApproxEquals"=w3559:bool)  [unwired: 8 in]
          }
          n2224 = And Array Elements(Boolean array=w3550) -> (logical AND=w3549:bool)
          n2225 = case shown="True" w3549 {
            tunnel: w3548 -> [_ w3556]
            frame False {
            }
            frame True {
              n2226 = call-poly <vilib>:"NT Write Value.vi"("value"=w3556, "name"="Auto State") -> ()  [unwired: 9 in, 1 out]
            }
          }
        }
      }
      n2227 = while {
        tunnel: w3509 -> [w3566]
        tunnel: [w3566] -> _
        stop <- w3564 stop-if-true
        n2228 = call-poly <vilib>:"NT Read Value.vi"("default value"="None", "name"="Auto State") -> ("value"=w3568:string)  [unwired: 7 in, 2 out]
        n2229 = call-poly <vilib>:"NT Read Value.vi"("default value"=FALSE, "name"="Auto/Path End") -> ("value"=w3564:bool)  [unwired: 7 in, 2 out]
        n2230 = Wait (ms)(milliseconds to wait=u32 20) -> ()  [unwired: 1 out]
        n2231 = case shown="\"Trigger\"" w3568 {
          frame "None", Default {
          }
          frame "Shoot" {
            n2232 = call-poly <vilib>:"NT Write Value.vi"("value"="Shoot Mode" ("default value"), "name"="Robot State") -> ()  [unwired: 9 in, 1 out]
          }
          frame "Intake" {
            n2233 = call-poly <vilib>:"NT Write Value.vi"("value"="Intake Mode" ("default value"), "name"="Robot State") -> ()  [unwired: 9 in, 1 out]
          }
          frame "Trigger" {
            n2234 = call-poly <vilib>:"NT Write Value.vi"("value"="ToShooter" ("default value"), "name"="Intake/Trigger Status") -> ()  [unwired: 9 in, 1 out]
          }
        }
      }
      n2235 = while {
        tunnel: w3513 -> [w3607]
        tunnel: [w3607] -> w3508
        i -> [w3605]
        stop <- w3604 stop-if-true
        w3603 = 0.0 ("Drv X Vel Dmd")
        n2236 = Not Equal To 0?(x=w3605) -> (x != 0?=w3604:bool)
        n2237 = Wait (ms)(milliseconds to wait=u32 20) -> ()  [unwired: 1 out]
        n2238 = call "SWERVE_DRIVE_MODULE_STATES_POSITIONS_FGV.vi"() -> ("out Current Module Positions"=w3599:T11[])  [unwired: 10 in, 1 out]
        n2239 = call "SWERVE_DRIVE_GET_GYRO.vi"() -> ("Gyro Heading Radians"=w3601:dbl)  [unwired: 11 in]
        n2240 = call "SWERVE_DRIVE_GET_GYRO.vi"() -> ("Gyro Heading Radians"=w3602:dbl)  [unwired: 11 in]
        n2241 = call <vilib>:"Rotation2d_CreateAngle.vi"("Angle"=w3601) -> ("ROTATION"=w3600:T9)  [unwired: 10 in]
        n2242 = call "SWERVE_DRIVE_SET_SPEED_DEMAND.vi"("Drv Rotation Orentation Dmd"=w3602, "Drv Angular Vel Dmd"=w3603, "Drv Y Vel Dmd"=w3603, "Drv X Vel Dmd"=w3603) -> ()  [unwired: 8 in]
        n2243 = call "SWERVE_TRAJECTORY_BEGIN.vi"("gyroAngle"=w3600, "Module Positions"=w3599, "Trajectory File Name"="Path Demo.wpilib.csv") -> ()  [unwired: 9 in]
      }
      n2244 = while {
        tunnel: w3508 -> [w3533]
        tunnel: [w3533] -> _
        stop <- FALSE stop-if-true
        w3517 = 0.0 ("Drv X Vel Dmd")
        n2245 = call-poly <vilib>:"NT Write Value.vi"("value"="Shoot Mode" ("default value"), "name"="Robot State") -> ()  [unwired: 9 in, 1 out]
        n2246 = call-poly <vilib>:"NT Read Value.vi"("name"="Shooter/Angle_Deg Act") -> ("value"=w3530:dbl)  [unwired: 8 in, 2 out]
        n2247 = call-poly <vilib>:"NT Read Value.vi"("name"="Shooter/Angle_Deg Dmd") -> ("value"=w3529:dbl)  [unwired: 8 in, 2 out]
        n2248 = call-poly <vilib>:"NT Read Value.vi"("name"="Shooter/Corrected Theta") -> ("value"=w3519:dbl)  [unwired: 8 in, 2 out]
        n2249 = call-poly <vilib>:"NT Read Value.vi"("name"="/limelight/tv") -> ("value"=w3521:dbl)  [unwired: 8 in, 2 out]
        n2250 = Not Equal To 0?(x=w3521) -> (x != 0?=w3520:bool)
        n2251 = call "SWERVE_DRIVE_GET_GYRO.vi"() -> ("Gyro Heading Radians"=w3515:dbl)  [unwired: 11 in]
        n2252 = call <vilib>:"Util_ApproxEquals.vi"("Tolerance"=2.0, "Value 2"=w3529, "Value 1"=w3530) -> ("ApproxEquals"=w3525:bool)  [unwired: 8 in]
        n2253 = Select(t=w3519, s=w3520, f=w3515) -> (s? t:f=w3518:dbl)
        n2254 = case shown="True" w3525 {
          frame False {
            n2255 = call-poly <vilib>:"NT Write Value.vi"("value"="Stop" ("default value"), "name"="Intake/Trigger Status") -> ()  [unwired: 9 in, 1 out]
          }
          frame True {
            n2256 = call-poly <vilib>:"NT Write Value.vi"("value"="ToShooter" ("default value"), "name"="Intake/Trigger Status") -> ()  [unwired: 9 in, 1 out]
          }
        }
        n2257 = call "SWERVE_DRIVE_SET_SPEED_DEMAND.vi"("Drv Rotation Orentation Dmd"=w3518, "Drv Angular Vel Dmd"=w3517, "Drv Y Vel Dmd"=w3517, "Drv X Vel Dmd"=w3517) -> ()  [unwired: 8 in]
        n2258 = Wait (ms)(milliseconds to wait=u32 20) -> ()  [unwired: 1 out]
      }
    }
  }
